vi "Test 401 Generic IO.vi"(11 "Test Case In":refnum<class "Test Profile Verification.lvclass">) -> (0 "error out":errorcluster, 3 "Test Case Out":refnum<class "Test Profile Verification.lvclass">)   [LabVIEW 2020, in "Test Profile Verification.lvclass"]
uses:
  Test Profile Verification.lvclass
  Test Profile Verification.lvclass/Test Profile Verification.ctl
  4993e8ee-a06a-463a-9684-69129f64d5ce.vi
  Profiles/401 Generic IO/CiA401 Generic IO Profile.lvclass
  Profiles/401 Generic IO/IO Capabilities.ctl
  EDS-File-Viewer/source/Electronic Datasheet/Electronic Datasheet.lvclass
  source/Typedefs/OD Entry Spec.ctl
  source/CANopen.lvlib
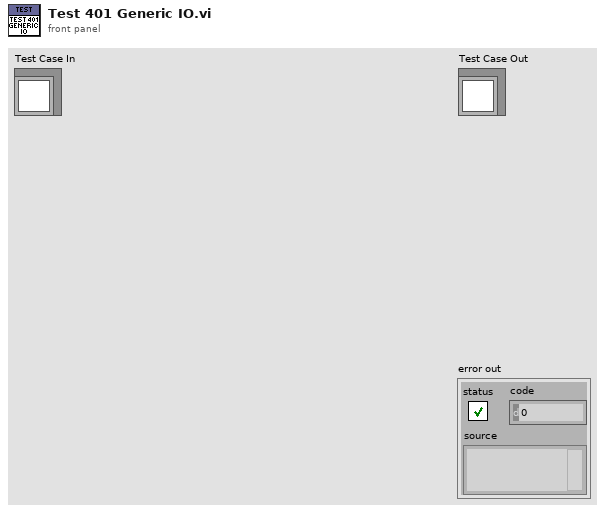
[diagram p1: front panel]
types:
  T1 = typedef "CANopen.lvlib/OD Entry Spec.ctl" = cluster{"Index":u16, "Name":string}
  T2 = typedef "CiA401 Generic IO Profile.lvclass/IO Capabilities.ctl" = cluster{"hasDigitialInputs":bool, "hasDigitalOutputs":bool, "hasAnalogInputs":bool, "hasAnalogOutputs":bool}
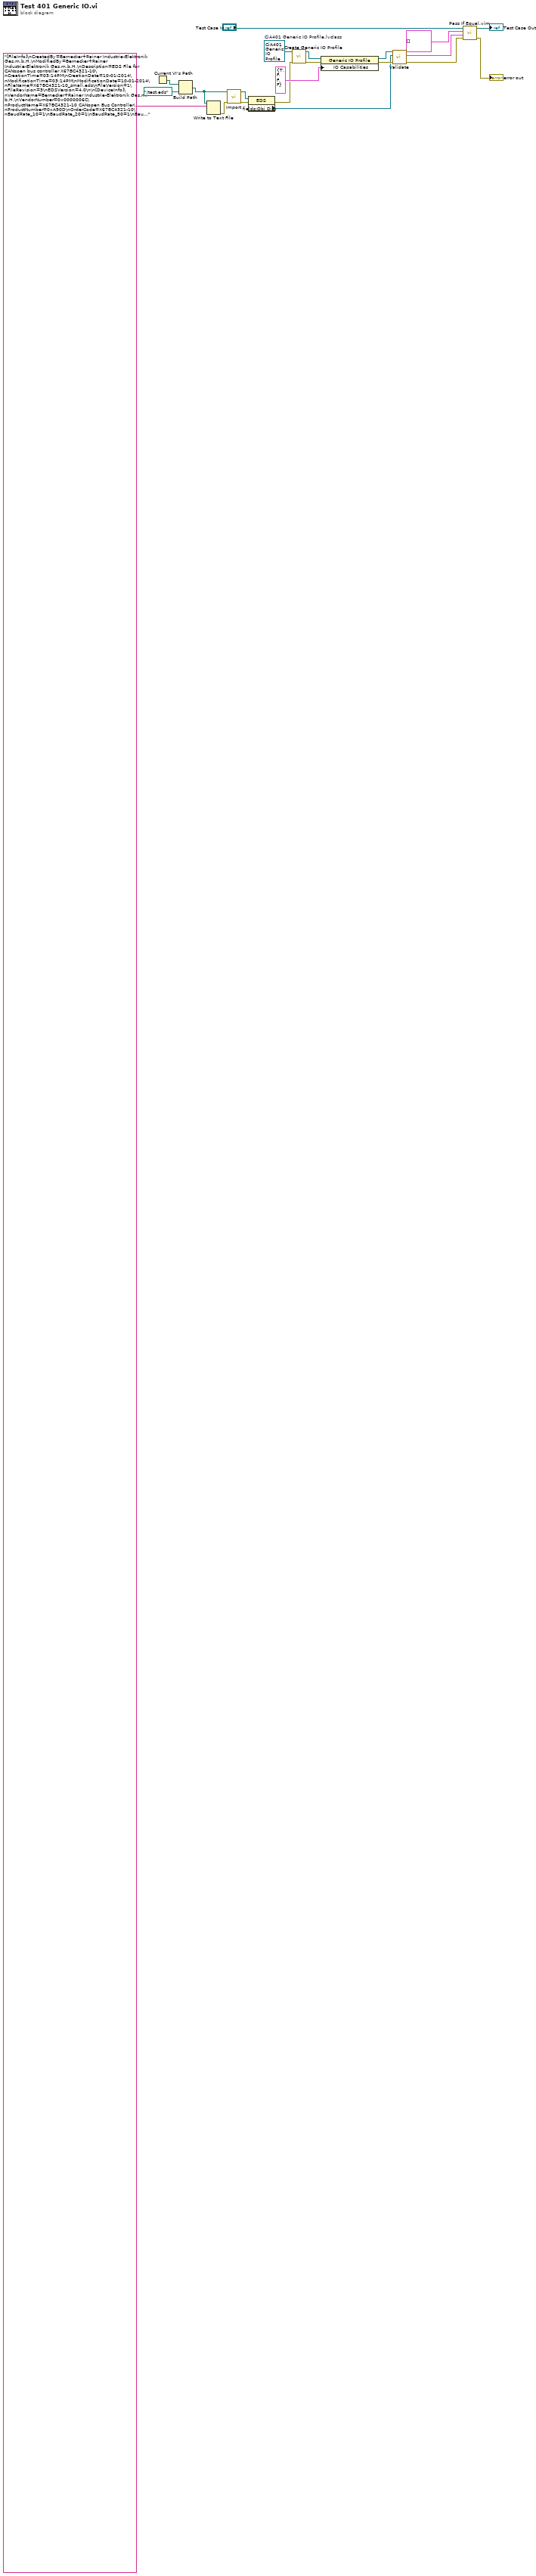
[diagram p0: block diagram]
diagram:
  w18 = refnum<class "CiA401 Generic IO Profile.lvclass"> refnum  # CiA401 Generic IO Profile.lvclass
  n1 = Current VI's Path() -> (path=w3:path)
  n2 = Build Path(base path=w3, name or relative path=path "../test.eds" ("file (use dialog)")) -> (appended path=w4:path)
  n3 = Write to Text File(file (use dialog)=w4, text="[FileInfo]\nCreatedBy=Bernecker+Rainer Industrie-Elektronik Ges.m.b.H.\nModifiedBy=Bernecker+Rainer Industrie-Elektronik Ges.m.b.H.\nDescription=EDS File for CANopen bus controller X67BC4321-10\nCreationTime=03:14PM\nCreationDate=10-01-2014\nModificationTime=03:14PM\nModificationDate=10-01-2014\nFileName=X67BC4321-10_small.eds\nFileVersion=1\nFileRevision=3\nEDSVersion=4.0\n\n[DeviceInfo]\nVendorName=Bernecker+Rainer Industrie-Elektronik Ges.m.b.H.\nVendorNumber=0x0000006C\nProductName=X67BC4321-10 CANopen Bus Controller\nProductNumber=0xA90D\nOrderCode=X67BC4321-10\nBaudRate_10=1\nBaudRate_20=1\nBaudRate_50=1\nBaudRate_125=1\nBaudRate_250=1\nBaudRate_500=1\nBaudRate_800=1\nBaudRate_1000=1\nSimpleBootUpMaster=0\nSimpleBootUpSlave=1\nGranularity=1\nDynamicChannelsSupported=0\nCompactPDO=0\nGroupMessaging=0\nNrOfRXPDO=32\nNrOfTXPDO=32\nLSS_Supported=0\n\n[DummyUsage]\nDummy0001=1\nDummy0002=1\nDummy0003=1\nDummy0004=1\nDummy0005=1\nDummy0006=1\nDummy0007=1\n\n[Comments]\nLines=0\n\n[MandatoryObjects]\nSupportedObjects=3\n1=0x1000\n2=0x1001\n3=0x1018\n\n[1000]\nParameterName=Device type\nObjectType=0x7\nDataType=0x0007\nAccessType=const\nDefaultValue=0x000F0191\nPDOMapping=0\nLowLimit=0x00000000\nHighLimit=0xFFFFFFFF\n\n[1001]\nParameterName=Error Register\nObjectType=0x7\nDataType=0x0005\nAccessType=ro\nDefaultValue=0x00\nPDOMapping=0\nLowLimit=0x00\nHighLimit=0xFF\n\n[1018]\nParameterName=Identity Object\nObjectType=0x9\nSubNumber=5\n\n[1018sub0]\nParameterName=Number of Entries\nObjectType=0x7\nDataType=0x0005\nAccessType=ro\nDefaultValue=0x4\nLowLimit=0x1\nHighLimit=0x4\n\n[1018sub1]\nParameterName=Vendor Id\nObjectType=0x7\nDataType=0x0007\nAccessType=ro\nDefaultValue=0x0000006C\nLowLimit=0x0\nHighLimit=0xFFFFFFFF\n\n[1018sub2]\nParameterName=Product Code\nObjectType=0x7\nDataType=0x0007\nAccessType=ro\nDefaultValue=0xA90D\nLowLimit=0x00000000\nHighLimit=0xFFFFFFFF\n\n[1018sub3]\nParameterName=Revision number\nObjectType=0x7\nDataType=0x0007\nAccessType=ro\nLowLimit=0x00000000\nHighLimit=0xFFFFFFFF\n\n[1018sub4]\nParameterName=Serial number\nObjectType=0x7\nDataType=0x0007\nAccessType=ro\nLowLimit=0x0\nHighLimit=0xFFFFFFFF\n\n[OptionalObjects]\nSupportedObjects=85\n1=0x1003\n2=0x1005\n3=0x1008\n4=0x1009\n5=0x100A\n6=0x100C\n7=0x100D\n8=0x1010\n9=0x1011\n10=0x1014\n11=0x1015\n12=0x1016\n13=0x1017\n14=0x1020\n15=0x1027\n16=0x1029\n17=0x1200\n18=0x1201\n19=0x1400\n20=0x1401\n21=0x1402\n22=0x1403\n23=0x1404\n24=0x1405\n25=0x1406\n26=0x1407\n27=0x1408\n28=0x1409\n29=0x1600\n30=0x1601\n31=0x1602\n32=0x1603\n33=0x1604\n34=0x1605\n35=0x1606\n36=0x1607\n37=0x1608\n38=0x1609\n39=0x1800\n40=0x1801\n41=0x1802\n42=0x1803\n43=0x1804\n44=0x1805\n45=0x1806\n46=0x1807\n47=0x1808\n48=0x1809\n49=0x1A00\n50=0x1A01\n51=0x1A02\n52=0x1A03\n53=0x1A04\n54=0x1A05\n55=0x1A06\n56=0x1A07\n57=0x1A08\n58=0x1A09\n59=0x1F50\n60=0x1F51\n61=0x1F52\n62=0x1F56\n63=0x1F57\n64=0x1F80\n65=0x6000\n66=0x6005\n67=0x6006\n68=0x6007\n69=0x6008\n70=0x6200\n71=0x6206\n72=0x6207\n73=0x6400\n74=0x6401\n75=0x6402\n76=0x6410\n77=0x6411\n78=0x6412\n79=0x6421\n80=0x6423\n81=0x6424\n82=0x6425\n83=0x6426\n84=0x6443\n85=0x6444\n\n[1003]\nParameterName=Pre-defined Error Field\nObjectType=0x8\nSubNumber=33\n\n[1003sub0]\nParameterName=Number of Errors\nObjectType=0x7\nDataType=0x0005\nAccessType=rw\nDefaultValue=0x0\nLowLimit=0x0\nHighLimit=0x20\n\n[1003sub1]\nParameterName=Standard Error Field 1\nObjectType=0x7\nDataType=0x0007\nAccessType=ro\nDefaultValue=0x0\nLowLimit=0x0\nHighLimit=0xFFFFFFFF\n\n[1003sub2]\nParameterName=Standard Error Field 2\nObjectType=0x7\nDataType=0x0007\nAccessType=ro\nDefaultValue=0x0\nLowLimit=0x0\nHighLimit=0xFFFFFFFF\n\n[1003sub3]\nParameterName=Standard Error Field 3\nObjectType=0x7\nDataType=0x0007\nAccessType=ro\nDefaultValue=0x0\nLowLimit=0x0\nHighLimit=0xFFFFFFFF\n\n[1003sub4]\nParameterName=Standard Error Field 4\nObjectType=0x7\nDataType=0x0007\nAccessType=ro\nDefaultValue=0x0\nLowLimit=0x0\nHighLimit=0xFFFFFFFF\n\n[1003sub5]\nParameterName=Standard Error Field 5\nObjectType=0x7\nDataType=0x0007\nAccessType=ro\nDefaultValue=0x0\nLowLimit=0x0\nHighLimit=0xFFFFFFFF\n\n[1003sub6]\nParameterName=Standard Error Field 6\nObjectType=0x7\nDataType=0x0007\nAccessType=ro\nDefaultValue=0x0\nLowLimit=0x0\nHighLimit=0xFFFFFFFF\n\n[1003sub7]\nParameterName=Standard Error Field 7\nObjectType=0x7\nDataType=0x0007\nAccessType=ro\nDefaultValue=0x0\nLowLimit=0x0\nHighLimit=0xFFFFFFFF\n\n[1003sub8]\nParameterName=Standard Error Field 8\nObjectType=0x7\nDataType=0x0007\nAccessType=ro\nDefaultValue=0x0\nLowLimit=0x0\nHighLimit=0xFFFFFFFF\n\n[1003sub9]\nParameterName=Standard Error Field 9\nObjectType=0x7\nDataType=0x0007\nAccessType=ro\nDefaultValue=0x0\nLowLimit=0x0\nHighLimit=0xFFFFFFFF\n\n[1003subA]\nParameterName=Standard Error Field 10\nObjectType=0x7\nDataType=0x0007\nAccessType=ro\nDefaultValue=0x0\nLowLimit=0x0\nHighLimit=0xFFFFFFFF\n\n[1003subB]\nParameterName=Standard Error Field 11\nObjectType=0x7\nDataType=0x0007\nAccessType=ro\nDefaultValue=0x0\nLowLimit=0x0\nHighLimit=0xFFFFFFFF\n\n[1003subC]\nParameterName=Standard Error Field 12\nObjectType=0x7\nDataType=0x0007\nAccessType=ro\nDefaultValue=0x0\nLowLimit=0x0\nHighLimit=0xFFFFFFFF\n\n[1003subD]\nParameterName=Standard Error Field 13\nObjectType=0x7\nDataType=0x0007\nAccessType=ro\nDefaultValue=0x0\nLowLimit=0x0\nHighLimit=0xFFFFFFFF\n\n[1003subE]\nParameterName=Standard Error Field 14\nObjectType=0x7\nDataType=0x0007\nAccessType=ro\nDefaultValue=0x0\nLowLimit=0x0\nHighLimit=0xFFFFFFFF\n\n[1003subF]\nParameterName=Standard Error Field 15\nObjectType=0x7\nDataType=0x0007\nAccessType=ro\nDefaultValue=0x0\nLowLimit=0x0\nHighLimit=0xFFFFFFFF\n\n[1003sub10]\nParameterName=Standard Error Field 16\nObjectType=0x7\nDataType=0x0007\nAccessType=ro\nDefaultValue=0x0\nLowLimit=0x0\nHighLimit=0xFFFFFFFF\n\n[1003sub11]\nParameterName=Standard Error Field 17\nObjectType=0x7\nDataType=0x0007\nAccessType=ro\nDefaultValue=0x0\nLowLimit=0x0\nHighLimit=0xFFFFFFFF\n\n[1003sub12]\nParameterName=Standard Error Field 18\nObjectType=0x7\nDataType=0x0007\nAccessType=ro\nDefaultValue=0x0\nLowLimit=0x0\nHighLimit=0xFFFFFFFF\n\n[1003sub13]\nParameterName=Standard Error Field 19\nObjectType=0x7\nDataType=0x0007\nAccessType=ro\nDefaultValue=0x0\nLowLimit=0x0\nHighLimit=0xFFFFFFFF\n\n[1003sub14]\nParameterName=Standard Error Field 20\nObjectType=0x7\nDataType=0x0007\nAccessType=ro\nDefaultValue=0x0\nLowLimit=0x0\nHighLimit=0xFFFFFFFF\n\n[1003sub15]\nParameterName=Standard Error Field 21\nObjectType=0x7\nDataType=0x0007\nAccessType=ro\nDefaultValue=0x0\nLowLimit=0x0\nHighLimit=0xFFFFFFFF\n\n[1003sub16]\nParameterName=Standard Error Field 22\nObjectType=0x7\nDataType=0x0007\nAccessType=ro\nDefaultValue=0x0\nLowLimit=0x0\nHighLimit=0xFFFFFFFF\n\n[1003sub17]\nParameterName=Standard Error Field 23\nObjectType=0x7\nDataType=0x0007\nAccessType=ro\nDefaultValue=0x0\nLowLimit=0x0\nHighLimit=0xFFFFFFFF\n\n[1003sub18]\nParameterName=Standard Error Field 24\nObjectType=0x7\nDataType=0x0007\nAccessType=ro\nDefaultValue=0x0\nLowLimit=0x0\nHighLimit=0xFFFFFFFF\n\n[1003sub19]\nParameterName=Standard Error Field 25\nObjectType=0x7\nDataType=0x0007\nAccessType=ro\nDefaultValue=0x0\nLowLimit=0x0\nHighLimit=0xFFFFFFFF\n\n[1003sub1A]\nParameterName=Standard Error Field 26\nObjectType=0x7\nDataType=0x0007\nAccessType=ro\nDefaultValue=0x0\nLowLimit=0x0\nHighLimit=0xFFFFFFFF\n\n[1003sub1B]\nParameterName=Standard Error Field 27\nObjectType=0x7\nDataType=0x0007\nAccessType=ro\nDefaultValue=0x0\nLowLimit=0x0\nHighLimit=0xFFFFFFFF\n\n[1003sub1C]\nParameterName=Standard Error Field 28\nObjectType=0x7\nDataType=0x0007\nAccessType=ro\nDefaultValue=0x0\nLowLimit=0x0\nHighLimit=0xFFFFFFFF\n\n[1003sub1D]\nParameterName=Standard Error Field 29\nObjectType=0x7\nDataType=0x0007\nAccessType=ro\nDefaultValue=0x0\nLowLimit=0x0\nHighLimit=0xFFFFFFFF\n\n[1003sub1E]\nParameterName=Standard Error Field 30\nObjectType=0x7\nDataType=0x0007\nAccessType=ro\nDefaultValue=0x0\nLowLimit=0x0\nHighLimit=0xFFFFFFFF\n\n[1003sub1F]\nParameterName=Standard Error Field 31\nObjectType=0x7\nDataType=0x0007\nAccessType=ro\nDefaultValue=0x0\nLowLimit=0x0\nHighLimit=0xFFFFFFFF\n\n[1003sub20]\nParameterName=Standard Error Field 32\nObjectType=0x7\nDataType=0x0007\nAccessType=ro\nDefaultValue=0x0\nLowLimit=0x0\nHighLimit=0xFFFFFFFF\n\n[1005]\nParameterName=COB-ID SYNC\nObjectType=0x7\nDataType=0x0007\nAccessType=rw\nDefaultValue=0x00000080\nPDOMapping=0\nLowLimit=0x00000001\nHighLimit=0xFFFFFFFF\n\n[1008]\nParameterName=Manufacturer Device Name\nObjectType=0x7\nDataType=0x0009\nAccessType=const\nDefaultValue=X67BC4321-10\nPDOMapping=0\n\n[1009]\nParameterName=Manufacturer Hardware Version\nObjectType=0x7\nDataType=0x0009\nAccessType=const\nPDOMapping=0\n\n[100A]\nParameterName=Manufacturer Software Version\nObjectType=0x7\nDataType=0x0009\nAccessType=const\nPDOMapping=0\n\n[100C]\nParameterName=Guard Time\nObjectType=0x7\nDataType=0x0006\nAccessType=rw\nDefaultValue=0\nPDOMapping=0\nLowLimit=0\nHighLimit=65535\n\n[100D]\nParameterName=Life Time Factor\nObjectType=0x7\nDataType=0x0005\nAccessType=rw\nDefaultValue=0x00\nPDOMapping=0\nLowLimit=0x0\nHighLimit=0xFF\n\n[1010]\nParameterName=Store Parameter Field\nObjectType=0x8\nSubNumber=5\n\n[1010sub0]\nParameterName=Number of Entries\nObjectType=0x7\nDataType=0x0005\nAccessType=ro\nDefaultValue=0x04\nLowLimit=0x0\nHighLimit=0x7F\n\n[1010sub1]\nParameterName=Save all Parameters\nObjectType=0x7\nDataType=0x0007\nAccessType=rw\n\n[1010sub2]\nParameterName=Save Communication Parameters\nObjectType=0x7\nDataType=0x0007\nAccessType=rw\n\n[1010sub3]\nParameterName=Save Application Parameters\nObjectType=0x7\nDataType=0x0007\nAccessType=rw\n\n[1010sub4]\nParameterName=Save Manufacturer Parameters\nObjectType=0x7\nDataType=0x0007\nAccessType=rw\n\n[1011]\nParameterName=Restore Default Parameters\nObjectType=0x8\nSubNumber=5\n\n[1011sub0]\nParameterName=Number of Entries\nObjectType=0x7\nDataType=0x0005\nAccessType=ro\nDefaultValue=0x04\nLowLimit=0x0\nHighLimit=0x7F\n\n[1011sub1]\nParameterName=Restore all Default Parameters\nObjectType=0x7\nDataType=0x0007\nAccessType=rw\n\n[1011sub2]\nParameterName=Restore Communication Default Parameters\nObjectType=0x7\nDataType=0x0007\nAccessType=rw\n\n[1011sub3]\nParameterName=Restore Application Default Parameters\nObjectType=0x7\nDataType=0x0007\nAccessType=rw\n\n[1011sub4]\nParameterName=Restore Manufacturer Default Parameters\nObjectType=0x7\nDataType=0x0007\nAccessType=rw\n\n[1014]\nParameterName=COB-ID EMCY\nObjectType=0x7\nDataType=0x0007\nAccessType=rw\nDefaultValue=$NODEID+0x080\nPDOMapping=0\nLowLimit=0x00000001\nHighLimit=0xFFFFFFFF\n\n[1015]\nParameterName=Inhibit Time Emergency\nObjectType=0x7\nDataType=0x0006\nAccessType=rw\nDefaultValue=0x0\nPDOMapping=0\nLowLimit=0x0\nHighLimit=0xFFFF\n\n[1016]\nParameterName=Consumer Heartbeat Time\nObjectType=0x8\nSubNumber=2\n\n[1016sub0]\nParameterName=Number of Entries\nObjectType=0x7\nDataType=0x0005\nAccessType=ro\nDefaultValue=0x1\nLowLimit=0x1\nHighLimit=0x7F\n\n[1016sub1]\nParameterName=Consumer Heartbeat Time\nObjectType=0x7\nDataType=0x0007\nAccessType=rw\nDefaultValue=0\nLowLimit=0x00000000\nHighLimit=0x007FFFFF\n\n[1017]\nParameterName=Producer Heartbeat Time\nObjectType=0x7\nDataType=0x0006\nAccessType=rw\nDefaultValue=0\nPDOMapping=0\nLowLimit=0\nHighLimit=65535\n\n[1020]\nParameterName=Verify Configuration\nObjectType=0x8\nSubNumber=3\n\n[1020sub0]\nParameterName=Number of entries\nObjectType=0x7\nDataType=0x0005\nAccessType=ro\nDefaultValue=2\n\n[1020sub1]\nParameterName=Configuration date\nObjectType=0x7\nDataType=0x0007\nAccessType=rw\n\n[1020sub2]\nParameterName=Configuration time\nObjectType=0x7\nDataType=0x0007\nAccessType=rw\n\n[1027]\nParameterName=Module List\nObjectType=0x8\nSubNumber=65\n\n[1027sub0]\nParameterName=Nr of connected modules\nObjectType=0x7\nDataType=0x0005\nAccessType=ro\nLowLimit=0x00\nHighLimit=0x40\n\n[1027sub1]\nParameterName=Module 1\nObjectType=0x7\nDataType=0x0006\nAccessType=ro\nDefaultValue=0xB528\nLowLimit=0x0000\nHighLimit=0xFFFF\n\n[1027sub2]\nParameterName=Module 2\nObjectType=0x7\nDataType=0x0006\nAccessType=ro\nDefaultValue=0x0000\nLowLimit=0x0000\nHighLimit=0xFFFF\n\n[1027sub3]\nParameterName=Module 3\nObjectType=0x7\nDataType=0x0006\nAccessType=ro\nDefaultValue=0x0000\nLowLimit=0x0000\nHighLimit=0xFFFF\n\n[1027sub4]\nParameterName=Module 4\nObjectType=0x7\nDataType=0x0006\nAccessType=ro\nDefaultValue=0x0000\nLowLimit=0x0000\nHighLimit=0xFFFF\n\n[1027sub5]\nParameterName=Module 5\nObjectType=0x7\nDataType=0x0006\nAccessType=ro\nDefaultValue=0x0000\nLowLimit=0x0000\nHighLimit=0xFFFF\n\n[1027sub6]\nParameterName=Module 6\nObjectType=0x7\nDataType=0x0006\nAccessType=ro\nDefaultValue=0x0000\nLowLimit=0x0000\nHighLimit=0xFFFF\n\n[1027sub7]\nParameterName=Module 7\nObjectType=0x7\nDataType=0x0006\nAccessType=ro\nDefaultValue=0x0000\nLowLimit=0x0000\nHighLimit=0xFFFF\n\n[1027sub8]\nParameterName=Module 8\nObjectType=0x7\nDataType=0x0006\nAccessType=ro\nDefaultValue=0x0000\nLowLimit=0x0000\nHighLimit=0xFFFF\n\n[1027sub9]\nParameterName=Module 9\nObjectType=0x7\nDataType=0x0006\nAccessType=ro\nDefaultValue=0x0000\nLowLimit=0x0000\nHighLimit=0xFFFF\n\n[1027subA]\nParameterName=Module 10\nObjectType=0x7\nDataType=0x0006\nAccessType=ro\nDefaultValue=0x0000\nLowLimit=0x0000\nHighLimit=0xFFFF\n\n[1027subB]\nParameterName=Module 11\nObjectType=0x7\nDataType=0x0006\nAccessType=ro\nDefaultValue=0x0000\nLowLimit=0x0000\nHighLimit=0xFFFF\n\n[1027subC]\nParameterName=Module 12\nObjectType=0x7\nDataType=0x0006\nAccessType=ro\nDefaultValue=0x0000\nLowLimit=0x0000\nHighLimit=0xFFFF\n\n[1027subD]\nParameterName=Module 13\nObjectType=0x7\nDataType=0x0006\nAccessType=ro\nDefaultValue=0x0000\nLowLimit=0x0000\nHighLimit=0xFFFF\n\n[1027subE]\nParameterName=Module 14\nObjectType=0x7\nDataType=0x0006\nAccessType=ro\nDefaultValue=0x0000\nLowLimit=0x0000\nHighLimit=0xFFFF\n\n[1027subF]\nParameterName=Module 15\nObjectType=0x7\nDataType=0x0006\nAccessType=ro\nDefaultValue=0x0000\nLowLimit=0x0000\nHighLimit=0xFFFF\n\n[1027sub10]\nParameterName=Module 16\nObjectType=0x7\nDataType=0x0006\nAccessType=ro\nDefaultValue=0x0000\nLowLimit=0x0000\nHighLimit=0xFFFF\n\n[1027sub11]\nParameterName=Module 17\nObjectType=0x7\nDataType=0x0006\nAccessType=ro\nDefaultValue=0x0000\nLowLimit=0x0000\nHighLimit=0xFFFF\n\n[1027sub12]\nParameterName=Module 18\nObjectType=0x7\nDataType=0x0006\nAccessType=ro\nDefaultValue=0x0000\nLowLimit=0x0000\nHighLimit=0xFFFF\n\n[1027sub13]\nParameterName=Module 19\nObjectType=0x7\nDataType=0x0006\nAccessType=ro\nDefaultValue=0x0000\nLowLimit=0x0000\nHighLimit=0xFFFF\n\n[1027sub14]\nParameterName=Module 20\nObjectType=0x7\nDataType=0x0006\nAccessType=ro\nDefaultValue=0x0000\nLowLimit=0x0000\nHighLimit=0xFFFF\n\n[1027sub15]\nParameterName=Module 21\nObjectType=0x7\nDataType=0x0006\nAccessType=ro\nDefaultValue=0x0000\nLowLimit=0x0000\nHighLimit=0xFFFF\n\n[1027sub16]\nParameterName=Module 22\nObjectType=0x7\nDataType=0x0006\nAccessType=ro\nDefaultValue=0x0000\nLowLimit=0x0000\nHighLimit=0xFFFF\n\n[1027sub17]\nParameterName=Module 23\nObjectType=0x7\nDataType=0x0006\nAccessType=ro\nDefaultValue=0x0000\nLowLimit=0x0000\nHighLimit=0xFFFF\n\n[1027sub18]\nParameterName=Module 24\nObjectType=0x7\nDataType=0x0006\nAccessType=ro\nDefaultValue=0x0000\nLowLimit=0x0000\nHighLimit=0xFFFF\n\n[1027sub19]\nParameterName=Module 25\nObjectType=0x7\nDataType=0x0006\nAccessType=ro\nDefaultValue=0x0000\nLowLimit=0x0000\nHighLimit=0xFFFF\n\n[1027sub1A]\nParameterName=Module 26\nObjectType=0x7\nDataType=0x0006\nAccessType=ro\nDefaultValue=0x0000\nLowLimit=0x0000\nHighLimit=0xFFFF\n\n[1027sub1B]\nParameterName=Module 27\nObjectType=0x7\nDataType=0x0006\nAccessType=ro\nDefaultValue=0x0000\nLowLimit=0x0000\nHighLimit=0xFFFF\n\n[1027sub1C]\nParameterName=Module 28\nObjectType=0x7\nDataType=0x0006\nAccessType=ro\nDefaultValue=0x0000\nLowLimit=0x0000\nHighLimit=0xFFFF\n\n[1027sub1D]\nParameterName=Module 29\nObjectType=0x7\nDataType=0x0006\nAccessType=ro\nDefaultValue=0x0000\nLowLimit=0x0000\nHighLimit=0xFFFF\n\n[1027sub1E]\nParameterName=Module 30\nObjectType=0x7\nDataType=0x0006\nAccessType=ro\nDefaultValue=0x0000\nLowLimit=0x0000\nHighLimit=0xFFFF\n\n[1027sub1F]\nParameterName=Module 31\nObjectType=0x7\nDataType=0x0006\nAccessType=ro\nDefaultValue=0x0000\nLowLimit=0x0000\nHighLimit=0xFFFF\n\n[1027sub20]\nParameterName=Module 32\nObjectType=0x7\nDataType=0x0006\nAccessType=ro\nDefaultValue=0x0000\nLowLimit=0x0000\nHighLimit=0xFFFF\n\n[1027sub21]\nParameterName=Module 33\nObjectType=0x7\nDataType=0x0006\nAccessType=ro\nDefaultValue=0x0000\nLowLimit=0x0000\nHighLimit=0xFFFF\n\n[1027sub22]\nParameterName=Module 34\nObjectType=0x7\nDataType=0x0006\nAccessType=ro\nDefaultValue=0x0000\nLowLimit=0x0000\nHighLimit=0xFFFF\n\n[1027sub23]\nParameterName=Module 35\nObjectType=0x7\nDataType=0x0006\nAccessType=ro\nDefaultValue=0x0000\nLowLimit=0x0000\nHighLimit=0xFFFF\n\n[1027sub24]\nParameterName=Module 36\nObjectType=0x7\nDataType=0x0006\nAccessType=ro\nDefaultValue=0x0000\nLowLimit=0x0000\nHighLimit=0xFFFF\n\n[1027sub25]\nParameterName=Module 37\nObjectType=0x7\nDataType=0x0006\nAccessType=ro\nDefaultValue=0x0000\nLowLimit=0x0000\nHighLimit=0xFFFF\n\n[1027sub26]\nParameterName=Module 38\nObjectType=0x7\nDataType=0x0006\nAccessType=ro\nDefaultValue=0x0000\nLowLimit=0x0000\nHighLimit=0xFFFF\n\n[1027sub27]\nParameterName=Module 39\nObjectType=0x7\nDataType=0x0006\nAccessType=ro\nDefaultValue=0x0000\nLowLimit=0x0000\nHighLimit=0xFFFF\n\n[1027sub28]\nParameterName=Module 40\nObjectType=0x7\nDataType=0x0006\nAccessType=ro\nDefaultValue=0x0000\nLowLimit=0x0000\nHighLimit=0xFFFF\n\n[1027sub29]\nParameterName=Module 41\nObjectType=0x7\nDataType=0x0006\nAccessType=ro\nDefaultValue=0x0000\nLowLimit=0x0000\nHighLimit=0xFFFF\n\n[1027sub2A]\nParameterName=Module 42\nObjectType=0x7\nDataType=0x0006\nAccessType=ro\nDefaultValue=0x0000\nLowLimit=0x0000\nHighLimit=0xFFFF\n\n[1027sub2B]\nParameterName=Module 43\nObjectType=0x7\nDataType=0x0006\nAccessType=ro\nDefaultValue=0x0000\nLowLimit=0x0000\nHighLimit=0xFFFF\n\n[1027sub2C]\nParameterName=Module 44\nObjectType=0x7\nDataType=0x0006\nAccessType=ro\nDefaultValue=0x0000\nLowLimit=0x0000\nHighLimit=0xFFFF\n\n[1027sub2D]\nParameterName=Module 45\nObjectType=0x7\nDataType=0x0006\nAccessType=ro\nDefaultValue=0x0000\nLowLimit=0x0000\nHighLimit=0xFFFF\n\n[1027sub2E]\nParameterName=Module 46\nObjectType=0x7\nDataType=0x0006\nAccessType=ro\nDefaultValue=0x0000\nLowLimit=0x0000\nHighLimit=0xFFFF\n\n[1027sub2F]\nParameterName=Module 47\nObjectType=0x7\nDataType=0x0006\nAccessType=ro\nDefaultValue=0x0000\nLowLimit=0x0000\nHighLimit=0xFFFF\n\n[1027sub30]\nParameterName=Module 48\nObjectType=0x7\nDataType=0x0006\nAccessType=ro\nDefaultValue=0x0000\nLowLimit=0x0000\nHighLimit=0xFFFF\n\n[1027sub31]\nParameterName=Module 49\nObjectType=0x7\nDataType=0x0006\nAccessType=ro\nDefaultValue=0x0000\nLowLimit=0x0000\nHighLimit=0xFFFF\n\n[1027sub32]\nParameterName=Module 50\nObjectType=0x7\nDataType=0x0006\nAccessType=ro\nDefaultValue=0x0000\nLowLimit=0x0000\nHighLimit=0xFFFF\n\n[1027sub33]\nParameterName=Module 51\nObjectType=0x7\nDataType=0x0006\nAccessType=ro\nDefaultValue=0x0000\nLowLimit=0x0000\nHighLimit=0xFFFF\n\n[1027sub34]\nParameterName=Module 52\nObjectType=0x7\nDataType=0x0006\nAccessType=ro\nDefaultValue=0x0000\nLowLimit=0x0000\nHighLimit=0xFFFF\n\n[1027sub35]\nParameterName=Module 53\nObjectType=0x7\nDataType=0x0006\nAccessType=ro\nDefaultValue=0x0000\nLowLimit=0x0000\nHighLimit=0xFFFF\n\n[1027sub36]\nParameterName=Module 54\nObjectType=0x7\nDataType=0x0006\nAccessType=ro\nDefaultValue=0x0000\nLowLimit=0x0000\nHighLimit=0xFFFF\n\n[1027sub37]\nParameterName=Module 55\nObjectType=0x7\nDataType=0x0006\nAccessType=ro\nDefaultValue=0x0000\nLowLimit=0x0000\nHighLimit=0xFFFF\n\n[1027sub38]\nParameterName=Module 56\nObjectType=0x7\nDataType=0x0006\nAccessType=ro\nDefaultValue=0x0000\nLowLimit=0x0000\nHighLimit=0xFFFF\n\n[1027sub39]\nParameterName=Module 57\nObjectType=0x7\nDataType=0x0006\nAccessType=ro\nDefaultValue=0x0000\nLowLimit=0x0000\nHighLimit=0xFFFF\n\n[1027sub3A]\nParameterName=Module 58\nObjectType=0x7\nDataType=0x0006\nAccessType=ro\nDefaultValue=0x0000\nLowLimit=0x0000\nHighLimit=0xFFFF\n\n[1027sub3B]\nParameterName=Module 59\nObjectType=0x7\nDataType=0x0006\nAccessType=ro\nDefaultValue=0x0000\nLowLimit=0x0000\nHighLimit=0xFFFF\n\n[1027sub3C]\nParameterName=Module 60\nObjectType=0x7\nDataType=0x0006\nAccessType=ro\nDefaultValue=0x0000\nLowLimit=0x0000\nHighLimit=0xFFFF\n\n[1027sub3D]\nParameterName=Module 61\nObjectType=0x7\nDataType=0x0006\nAccessType=ro\nDefaultValue=0x0000\nLowLimit=0x0000\nHighLimit=0xFFFF\n\n[1027sub3E]\nParameterName=Module 62\nObjectType=0x7\nDataType=0x0006\nAccessType=ro\nDefaultValue=0x0000\nLowLimit=0x0000\nHighLimit=0xFFFF\n\n[1027sub3F]\nParameterName=Module 63\nObjectType=0x7\nDataType=0x0006\nAccessType=ro\nDefaultValue=0x0000\nLowLimit=0x0000\nHighLimit=0xFFFF\n\n[1027sub40]\nParameterName=Module 64\nObjectType=0x7\nDataType=0x0006\nAccessType=ro\nDefaultValue=0x0000\nLowLimit=0x0000\nHighLimit=0xFFFF\n\n[1029]\nParameterName=Error behaviour\nObjectType=0x8\nSubNumber=3\n\n[1029sub0]\nParameterName=Nr of Error Classes\nObjectType=0x7\nDataType=0x0005\nAccessType=ro\nDefaultValue=128\n\n[1029sub1]\nParameterName=Communication Error\nObjectType=0x7\nDataType=0x0005\nAccessType=rw\nDefaultValue=0\n\n[1029sub80]\nParameterName=Advanced mapping\nObjectType=0x7\nDataType=0x0005\nAccessType=rw\nDefaultValue=0x81\n\n[1200]\nParameterName=Server SDO Parameter\nObjectType=0x9\nSubNumber=3\n\n[1200sub0]\nParameterName=Number of Entries\nObjectType=0x7\nDataType=0x0005\nAccessType=ro\nDefaultValue=0x02\nLowLimit=0x02\nHighLimit=0x02\n\n[1200sub1]\nParameterName=COB-ID Client -> Server\nObjectType=0x7\nDataType=0x0007\nAccessType=ro\nDefaultValue=$NODEID+0x600\nLowLimit=$NODEID+0x600\nHighLimit=$NODEID+0x600\n\n[1200sub2]\nParameterName=COB-ID Server -> Client\nObjectType=0x7\nDataType=0x0007\nAccessType=ro\nDefaultValue=$NODEID+0x580\nLowLimit=$NODEID+0x580\nHighLimit=$NODEID+0x580\n\n[1201]\nParameterName=Server SDO Parameter\nObjectType=0x9\nSubNumber=4\n\n[1201sub0]\nParameterName=Number of Entries\nObjectType=0x7\nDataType=0x0005\nAccessType=ro\nDefaultValue=0x3\nLowLimit=0x2\nHighLimit=0x3\n\n[1201sub1]\nParameterName=COB-ID Client -> Server\nObjectType=0x7\nDataType=0x0007\nAccessType=rw\nDefaultValue=0x80000000\nPDOMapping=0\nLowLimit=0x01\nHighLimit=0xFFFFFFFF\n\n[1201sub2]\nParameterName=COB-ID Server -> Client\nObjectType=0x7\nDataType=0x0007\nAccessType=rw\nDefaultValue=0x80000000\nPDOMapping=0\nLowLimit=0x01\nHighLimit=0xFFFFFFFF\n\n[1201sub3]\nParameterName=Node ID of the SDO Client\nObjectType=0x7\nDataType=0x0005\nAccessType=rw\nPDOMapping=0\nLowLimit=1\nHighLimit=127\n\n[1400]\nParameterName=Receive PDO 1 Communication Parameter\nObjectType=0x9\nSubNumber=5\n\n[1400sub0]\nParameterName=Number of Entries\nObjectType=0x7\nDataType=0x0005\nAccessType=ro\nDefaultValue=0x05\nLowLimit=0x02\nHighLimit=0x05\n\n[1400sub1]\nParameterName=COB-ID\nObjectType=0x7\nDataType=0x0007\nAccessType=rw\nDefaultValue=$NODEID+0x00000200\nLowLimit=0x00000001\nHighLimit=0xFFFFFFFF\n\n[1400sub2]\nParameterName=Transmission Type\nObjectType=0x7\nDataType=0x0005\nAccessType=rw\nDefaultValue=0xFF\nLowLimit=0x00\nHighLimit=0xFF\n\n[1400sub3]\nParameterName=Inhibit Time\nObjectType=0x7\nDataType=0x0006\nAccessType=rw\nDefaultValue=0x0000\nLowLimit=0x0000\nHighLimit=0xFFFF\n\n[1400sub5]\nParameterName=Event Timer\nObjectType=0x7\nDataType=0x0006\nAccessType=rw\nDefaultValue=0x0\nLowLimit=0x0\nHighLimit=0xFFFF\n\n[1401]\nParameterName=Receive PDO 2 Communication Parameter\nObjectType=0x9\nSubNumber=5\n\n[1401sub0]\nParameterName=Number of Entries\nObjectType=0x7\nDataType=0x0005\nAccessType=ro\nDefaultValue=0x05\nLowLimit=0x02\nHighLimit=0x05\n\n[1401sub1]\nParameterName=COB-ID\nObjectType=0x7\nDataType=0x0007\nAccessType=rw\nDefaultValue=$NODEID+0x00000300\nLowLimit=0x00000001\nHighLimit=0xFFFFFFFF\n\n[1401sub2]\nParameterName=Transmission Type\nObjectType=0x7\nDataType=0x0005\nAccessType=rw\nDefaultValue=0xFF\nLowLimit=0x00\nHighLimit=0xFF\n\n[1401sub3]\nParameterName=Inhibit Time\nObjectType=0x7\nDataType=0x0006\nAccessType=rw\nDefaultValue=0x0000\nLowLimit=0x0000\nHighLimit=0xFFFF\n\n[1401sub5]\nParameterName=Event Timer\nObjectType=0x7\nDataType=0x0006\nAccessType=rw\nDefaultValue=0x0\nLowLimit=0x0\nHighLimit=0xFFFF\n\n[1402]\nParameterName=Receive PDO 3 Communication Parameter\nObjectType=0x9\nSubNumber=5\n\n[1402sub0]\nParameterName=Number of Entries\nObjectType=0x7\nDataType=0x0005\nAccessType=ro\nDefaultValue=0x05\nLowLimit=0x02\nHighLimit=0x05\n\n[1402sub1]\nParameterName=COB-ID\nObjectType=0x7\nDataType=0x0007\nAccessType=rw\nDefaultValue=$NODEID+0x00000400\nLowLimit=0x00000001\nHighLimit=0xFFFFFFFF\n\n[1402sub2]\nParameterName=Transmission Type\nObjectType=0x7\nDataType=0x0005\nAccessType=rw\nDefaultValue=0xFF\nLowLimit=0x00\nHighLimit=0xFF\n\n[1402sub3]\nParameterName=Inhibit Time\nObjectType=0x7\nDataType=0x0006\nAccessType=rw\nDefaultValue=0x0000\nLowLimit=0x0000\nHighLimit=0xFFFF\n\n[1402sub5]\nParameterName=Event Timer\nObjectType=0x7\nDataType=0x0006\nAccessType=rw\nDefaultValue=0x0\nLowLimit=0x0\nHighLimit=0xFFFF\n\n[1403]\nParameterName=Receive PDO 4 Communication Parameter\nObjectType=0x9\nSubNumber=5\n\n[1403sub0]\nParameterName=Number of Entries\nObjectType=0x7\nDataType=0x0005\nAccessType=ro\nDefaultValue=0x05\nLowLimit=0x02\nHighLimit=0x05\n\n[1403sub1]\nParameterName=COB-ID\nObjectType=0x7\nDataType=0x0007\nAccessType=rw\nDefaultValue=$NODEID+0x00000500\nLowLimit=0x00000001\nHighLimit=0xFFFFFFFF\n\n[1403sub2]\nParameterName=Transmission Type\nObjectType=0x7\nDataType=0x0005\nAccessType=rw\nDefaultValue=0xFF\nLowLimit=0x00\nHighLimit=0xFF\n\n[1403sub3]\nParameterName=Inhibit Time\nObjectType=0x7\nDataType=0x0006\nAccessType=rw\nDefaultValue=0x0000\nLowLimit=0x0000\nHighLimit=0xFFFF\n\n[1403sub5]\nParameterName=Event Timer\nObjectType=0x7\nDataType=0x0006\nAccessType=rw\nDefaultValue=0x0\nLowLimit=0x0\nHighLimit=0xFFFF\n\n[1404]\nParameterName=Receive PDO 5 Communication Parameter\nObjectType=0x9\nSubNumber=5\n\n[1404sub0]\nParameterName=Number of Entries\nObjectType=0x7\nDataType=0x0005\nAccessType=ro\nDefaultValue=0x05\nLowLimit=0x02\nHighLimit=0x05\n\n[1404sub1]\nParameterName=COB-ID\nObjectType=0x7\nDataType=0x0007\nAccessType=rw\nDefaultValue=$NODEID+0x80000240\nLowLimit=0x00000001\nHighLimit=0xFFFFFFFF\n\n[1404sub2]\nParameterName=Transmission Type\nObjectType=0x7\nDataType=0x0005\nAccessType=rw\nDefaultValue=255\nLowLimit=0\nHighLimit=255\n\n[1404sub3]\nParameterName=Inhibit Time\nObjectType=0x7\nDataType=0x0006\nAccessType=rw\nDefaultValue=0x0000\nLowLimit=0x0000\nHighLimit=0xFFFF\n\n[1404sub5]\nParameterName=Event Timer\nObjectType=0x7\nDataType=0x0006\nAccessType=rw\nDefaultValue=0x0\nLowLimit=0x0\nHighLimit=0xFFFF\n\n[1405]\nParameterName=Receive PDO 6 Communication Parameter\nObjectType=0x9\nSubNumber=5\n\n[1405sub0]\nParameterName=Number of Entries\nObjectType=0x7\nDataType=0x0005\nAccessType=ro\nDefaultValue=0x05\nLowLimit=0x02\nHighLimit=0x05\n\n[1405sub1]\nParameterName=COB-ID\nObjectType=0x7\nDataType=0x0007\nAccessType=rw\nDefaultValue=$NODEID+0x80000340\nLowLimit=0x00000001\nHighLimit=0xFFFFFFFF\n\n[1405sub2]\nParameterName=Transmission Type\nObjectType=0x7\nDataType=0x0005\nAccessType=rw\nDefaultValue=255\nLowLimit=0\nHighLimit=255\n\n[1405sub3]\nParameterName=Inhibit Time\nObjectType=0x7\nDataType=0x0006\nAccessType=rw\nDefaultValue=0x0000\nLowLimit=0x0000\nHighLimit=0xFFFF\n\n[1405sub5]\nParameterName=Event Timer\nObjectType=0x7\nDataType=0x0006\nAccessType=rw\nDefaultValue=0x0\nLowLimit=0x0\nHighLimit=0xFFFF\n\n[1406]\nParameterName=Receive PDO 7 Communication Parameter\nObjectType=0x9\nSubNumber=5\n\n[1406sub0]\nParameterName=Number of Entries\nObjectType=0x7\nDataType=0x0005\nAccessType=ro\nDefaultValue=0x05\nLowLimit=0x02\nHighLimit=0x05\n\n[1406sub1]\nParameterName=COB-ID\nObjectType=0x7\nDataType=0x0007\nAccessType=rw\nDefaultValue=$NODEID+0x80000440\nLowLimit=0x00000001\nHighLimit=0xFFFFFFFF\n\n[1406sub2]\nParameterName=Transmission Type\nObjectType=0x7\nDataType=0x0005\nAccessType=rw\nDefaultValue=0xFF\nLowLimit=0x00\nHighLimit=0xFF\n\n[1406sub3]\nParameterName=Inhibit Time\nObjectType=0x7\nDataType=0x0006\nAccessType=rw\nDefaultValue=0x0000\nLowLimit=0x0000\nHighLimit=0xFFFF\n\n[1406sub5]\nParameterName=Event Timer\nObjectType=0x7\nDataType=0x0006\nAccessType=rw\nDefaultValue=0x0\nLowLimit=0x0\nHighLimit=0xFFFF\n\n[1407]\nParameterName=Receive PDO 8 Communication Parameter\nObjectType=0x9\nSubNumber=5\n\n[1407sub0]\nParameterName=Number of Entries\nObjectType=0x7\nDataType=0x0005\nAccessType=ro\nDefaultValue=0x05\nLowLimit=0x02\nHighLimit=0x05\n\n[1407sub1]\nParameterName=COB-ID\nObjectType=0x7\nDataType=0x0007\nAccessType=rw\nDefaultValue=$NODEID+0x80000540\nLowLimit=0x00000001\nHighLimit=0xFFFFFFFF\n\n[1407sub2]\nParameterName=Transmission Type\nObjectType=0x7\nDataType=0x0005\nAccessType=rw\nDefaultValue=0xFF\nLowLimit=0x00\nHighLimit=0xFF\n\n[1407sub3]\nParameterName=Inhibit Time\nObjectType=0x7\nDataType=0x0006\nAccessType=rw\nDefaultValue=0x0000\nLowLimit=0x0000\nHighLimit=0xFFFF\n\n[1407sub5]\nParameterName=Event Timer\nObjectType=0x7\nDataType=0x0006\nAccessType=rw\nDefaultValue=0x0\nLowLimit=0x0\nHighLimit=0xFFFF\n\n[1408]\nParameterName=Receive PDO 9 Communication Parameter\nObjectType=0x9\nSubNumber=5\n\n[1408sub0]\nParameterName=Number of Entries\nObjectType=0x7\nDataType=0x0005\nAccessType=ro\nDefaultValue=0x05\nLowLimit=0x02\nHighLimit=0x05\n\n[1408sub1]\nParameterName=COB-ID\nObjectType=0x7\nDataType=0x0007\nAccessType=rw\nDefaultValue=$NODEID+0x80000220\nLowLimit=0x00000001\nHighLimit=0xFFFFFFFF\n\n[1408sub2]\nParameterName=Transmission Type\nObjectType=0x7\nDataType=0x0005\nAccessType=rw\nDefaultValue=0xFF\nLowLimit=0x00\nHighLimit=0xFF\n\n[1408sub3]\nParameterName=Inhibit Time\nObjectType=0x7\nDataType=0x0006\nAccessType=rw\nDefaultValue=0x0000\nLowLimit=0x0000\nHighLimit=0xFFFF\n\n[1408sub5]\nParameterName=Event Timer\nObjectType=0x7\nDataType=0x0006\nAccessType=rw\nDefaultValue=0x0\nLowLimit=0x0\nHighLimit=0xFFFF\n\n[1409]\nParameterName=Receive PDO 10 Communication Parameter\nObjectType=0x9\nSubNumber=5\n\n[1409sub0]\nParameterName=Number of Entries\nObjectType=0x7\nDataType=0x0005\nAccessType=ro\nDefaultValue=0x05\nLowLimit=0x02\nHighLimit=0x05\n\n[1409sub1]\nParameterName=COB-ID\nObjectType=0x7\nDataType=0x0007\nAccessType=rw\nDefaultValue=$NODEID+0x80000320\nLowLimit=0x00000001\nHighLimit=0xFFFFFFFF\n\n[1409sub2]\nParameterName=Transmission Type\nObjectType=0x7\nDataType=0x0005\nAccessType=rw\nDefaultValue=0xFF\nLowLimit=0x00\nHighLimit=0xFF\n\n[1409sub3]\nParameterName=Inhibit Time\nObjectType=0x7\nDataType=0x0006\nAccessType=rw\nDefaultValue=0x0000\nLowLimit=0x0000\nHighLimit=0xFFFF\n\n[1409sub5]\nParameterName=Event Timer\nObjectType=0x7\nDataType=0x0006\nAccessType=rw\nDefaultValue=0x0\nLowLimit=0x0\nHighLimit=0xFFFF\n\n[1600]\nParameterName=Receive PDO 1 Mapping Parameter\nObjectType=0x9\nSubNumber=9\n\n[1600sub0]\nParameterName=Number of Entries\nObjectType=0x7\nDataType=0x0005\nAccessType=rw\nDefaultValue=8\nLowLimit=0\nHighLimit=64\n\n[1600sub1]\nParameterName=PDO Mapping Entry\nObjectType=0x7\nDataType=0x0007\nAccessType=rw\nDefaultValue=0x62000108\nLowLimit=0x00000000\nHighLimit=0xFFFFFFFF\n\n[1600sub2]\nParameterName=PDO Mapping Entry\nObjectType=0x7\nDataType=0x0007\nAccessType=rw\nDefaultValue=0x62000208\nLowLimit=0x00000000\nHighLimit=0xFFFFFFFF\n\n[1600sub3]\nParameterName=PDO Mapping Entry\nObjectType=0x7\nDataType=0x0007\nAccessType=rw\nDefaultValue=0x62000308\nLowLimit=0x00000000\nHighLimit=0xFFFFFFFF\n\n[1600sub4]\nParameterName=PDO Mapping Entry\nObjectType=0x7\nDataType=0x0007\nAccessType=rw\nDefaultValue=0x62000408\nLowLimit=0x00000000\nHighLimit=0xFFFFFFFF\n\n[1600sub5]\nParameterName=PDO Mapping Entry\nObjectType=0x7\nDataType=0x0007\nAccessType=rw\nDefaultValue=0x62000508\nLowLimit=0x00000000\nHighLimit=0xFFFFFFFF\n\n[1600sub6]\nParameterName=PDO Mapping Entry\nObjectType=0x7\nDataType=0x0007\nAccessType=rw\nDefaultValue=0x62000608\nLowLimit=0x00000000\nHighLimit=0xFFFFFFFF\n\n[1600sub7]\nParameterName=PDO Mapping Entry\nObjectType=0x7\nDataType=0x0007\nAccessType=rw\nDefaultValue=0x62000708\nLowLimit=0x00000000\nHighLimit=0xFFFFFFFF\n\n[1600sub8]\nParameterName=PDO Mapping Entry\nObjectType=0x7\nDataType=0x0007\nAccessType=rw\nDefaultValue=0x62000808\nLowLimit=0x00000000\nHighLimit=0xFFFFFFFF\n\n[1601]\nParameterName=Receive PDO 2 Mapping Parameter\nObjectType=0x9\nSubNumber=9\n\n[1601sub0]\nParameterName=Number of Entries\nObjectType=0x7\nDataType=0x0005\nAccessType=rw\nDefaultValue=4\nLowLimit=0\nHighLimit=64\n\n[1601sub1]\nParameterName=PDO Mapping Entry\nObjectType=0x7\nDataType=0x0007\nAccessType=rw\nDefaultValue=0x64110110\nLowLimit=0x00000000\nHighLimit=0xFFFFFFFF\n\n[1601sub2]\nParameterName=PDO Mapping Entry\nObjectType=0x7\nDataType=0x0007\nAccessType=rw\nDefaultValue=0x64110210\nLowLimit=0x00000000\nHighLimit=0xFFFFFFFF\n\n[1601sub3]\nParameterName=PDO Mapping Entry\nObjectType=0x7\nDataType=0x0007\nAccessType=rw\nDefaultValue=0x64110310\nLowLimit=0x00000000\nHighLimit=0xFFFFFFFF\n\n[1601sub4]\nParameterName=PDO Mapping Entry\nObjectType=0x7\nDataType=0x0007\nAccessType=rw\nDefaultValue=0x64110410\nLowLimit=0x00000000\nHighLimit=0xFFFFFFFF\n\n[1601sub5]\nParameterName=PDO Mapping Entry\nObjectType=0x7\nDataType=0x0007\nAccessType=rw\nDefaultValue=0x00000000\nLowLimit=0x00000000\nHighLimit=0xFFFFFFFF\n\n[1601sub6]\nParameterName=PDO Mapping Entry\nObjectType=0x7\nDataType=0x0007\nAccessType=rw\nDefaultValue=0x00000000\nLowLimit=0x00000000\nHighLimit=0xFFFFFFFF\n\n[1601sub7]\nParameterName=PDO Mapping Entry\nObjectType=0x7\nDataType=0x0007\nAccessType=rw\nDefaultValue=0x00000000\nLowLimit=0x00000000\nHighLimit=0xFFFFFFFF\n\n[1601sub8]\nParameterName=PDO Mapping Entry\nObjectType=0x7\nDataType=0x0007\nAccessType=rw\nDefaultValue=0x00000000\nLowLimit=0x00000000\nHighLimit=0xFFFFFFFF\n\n[1602]\nParameterName=Receive PDO 3 Mapping Parameter\nObjectType=0x9\nSubNumber=9\n\n[1602sub0]\nParameterName=Number of Entries\nObjectType=0x7\nDataType=0x0005\nAccessType=rw\nDefaultValue=4\nLowLimit=0\nHighLimit=64\n\n[1602sub1]\nParameterName=PDO Mapping Entry\nObjectType=0x7\nDataType=0x0007\nAccessType=rw\nDefaultValue=0x64110510\nLowLimit=0x00000000\nHighLimit=0xFFFFFFFF\n\n[1602sub2]\nParameterName=PDO Mapping Entry\nObjectType=0x7\nDataType=0x0007\nAccessType=rw\nDefaultValue=0x64110610\nLowLimit=0x00000000\nHighLimit=0xFFFFFFFF\n\n[1602sub3]\nParameterName=PDO Mapping Entry\nObjectType=0x7\nDataType=0x0007\nAccessType=rw\nDefaultValue=0x64110710\nLowLimit=0x00000000\nHighLimit=0xFFFFFFFF\n\n[1602sub4]\nParameterName=PDO Mapping Entry\nObjectType=0x7\nDataType=0x0007\nAccessType=rw\nDefaultValue=0x64110810\nLowLimit=0x00000000\nHighLimit=0xFFFFFFFF\n\n[1602sub5]\nParameterName=PDO Mapping Entry\nObjectType=0x7\nDataType=0x0007\nAccessType=rw\nDefaultValue=0x00000000\nLowLimit=0x00000000\nHighLimit=0xFFFFFFFF\n\n[1602sub6]\nParameterName=PDO Mapping Entry\nObjectType=0x7\nDataType=0x0007\nAccessType=rw\nDefaultValue=0x00000000\nLowLimit=0x00000000\nHighLimit=0xFFFFFFFF\n\n[1602sub7]\nParameterName=PDO Mapping Entry\nObjectType=0x7\nDataType=0x0007\nAccessType=rw\nDefaultValue=0x00000000\nLowLimit=0x00000000\nHighLimit=0xFFFFFFFF\n\n[1602sub8]\nParameterName=PDO Mapping Entry\nObjectType=0x7\nDataType=0x0007\nAccessType=rw\nDefaultValue=0x00000000\nLowLimit=0x00000000\nHighLimit=0xFFFFFFFF\n\n[1603]\nParameterName=Receive PDO 4 Mapping Parameter\nObjectType=0x9\nSubNumber=9\n\n[1603sub0]\nParameterName=Number of Entries\nObjectType=0x7\nDataType=0x0005\nAccessType=rw\nDefaultValue=4\nLowLimit=0\nHighLimit=64\n\n[1603sub1]\nParameterName=PDO Mapping Entry\nObjectType=0x7\nDataType=0x0007\nAccessType=rw\nDefaultValue=0x64110910\nLowLimit=0x00000000\nHighLimit=0xFFFFFFFF\n\n[1603sub2]\nParameterName=PDO Mapping Entry\nObjectType=0x7\nDataType=0x0007\nAccessType=rw\nDefaultValue=0x64110a10\nLowLimit=0x00000000\nHighLimit=0xFFFFFFFF\n\n[1603sub3]\nParameterName=PDO Mapping Entry\nObjectType=0x7\nDataType=0x0007\nAccessType=rw\nDefaultValue=0x64110b10\nLowLimit=0x00000000\nHighLimit=0xFFFFFFFF\n\n[1603sub4]\nParameterName=PDO Mapping Entry\nObjectType=0x7\nDataType=0x0007\nAccessType=rw\nDefaultValue=0x64110c10\nLowLimit=0x00000000\nHighLimit=0xFFFFFFFF\n\n[1603sub5]\nParameterName=PDO Mapping Entry\nObjectType=0x7\nDataType=0x0007\nAccessType=rw\nDefaultValue=0x00000000\nLowLimit=0x00000000\nHighLimit=0xFFFFFFFF\n\n[1603sub6]\nParameterName=PDO Mapping Entry\nObjectType=0x7\nDataType=0x0007\nAccessType=rw\nDefaultValue=0x00000000\nLowLimit=0x00000000\nHighLimit=0xFFFFFFFF\n\n[1603sub7]\nParameterName=PDO Mapping Entry\nObjectType=0x7\nDataType=0x0007\nAccessType=rw\nDefaultValue=0x00000000\nLowLimit=0x00000000\nHighLimit=0xFFFFFFFF\n\n[1603sub8]\nParameterName=PDO Mapping Entry\nObjectType=0x7\nDataType=0x0007\nAccessType=rw\nDefaultValue=0x00000000\nLowLimit=0x00000000\nHighLimit=0xFFFFFFFF\n\n[1604]\nParameterName=Receive PDO 5 Mapping Parameter\nObjectType=0x9\nSubNumber=9\n\n[1604sub0]\nParameterName=Number of Entries\nObjectType=0x7\nDataType=0x0005\nAccessType=rw\nDefaultValue=0\nLowLimit=0\nHighLimit=64\n\n[1604sub1]\nParameterName=PDO Mapping Entry\nObjectType=0x7\nDataType=0x0007\nAccessType=rw\nDefaultValue=0x00000000\nLowLimit=0x00000000\nHighLimit=0xFFFFFFFF\n\n[1604sub2]\nParameterName=PDO Mapping Entry\nObjectType=0x7\nDataType=0x0007\nAccessType=rw\nDefaultValue=0x00000000\nLowLimit=0x00000000\nHighLimit=0xFFFFFFFF\n\n[1604sub3]\nParameterName=PDO Mapping Entry\nObjectType=0x7\nDataType=0x0007\nAccessType=rw\nDefaultValue=0x00000000\nLowLimit=0x00000000\nHighLimit=0xFFFFFFFF\n\n[1604sub4]\nParameterName=PDO Mapping Entry\nObjectType=0x7\nDataType=0x0007\nAccessType=rw\nDefaultValue=0x00000000\nLowLimit=0x00000000\nHighLimit=0xFFFFFFFF\n\n[1604sub5]\nParameterName=PDO Mapping Entry\nObjectType=0x7\nDataType=0x0007\nAccessType=rw\nDefaultValue=0x00000000\nLowLimit=0x00000000\nHighLimit=0xFFFFFFFF\n\n[1604sub6]\nParameterName=PDO Mapping Entry\nObjectType=0x7\nDataType=0x0007\nAccessType=rw\nDefaultValue=0x00000000\nLowLimit=0x00000000\nHighLimit=0xFFFFFFFF\n\n[1604sub7]\nParameterName=PDO Mapping Entry\nObjectType=0x7\nDataType=0x0007\nAccessType=rw\nDefaultValue=0x00000000\nLowLimit=0x00000000\nHighLimit=0xFFFFFFFF\n\n[1604sub8]\nParameterName=PDO Mapping Entry\nObjectType=0x7\nDataType=0x0007\nAccessType=rw\nDefaultValue=0x00000000\nLowLimit=0x00000000\nHighLimit=0xFFFFFFFF\n\n[1605]\nParameterName=Receive PDO 6 Mapping Parameter\nObjectType=0x9\nSubNumber=9\n\n[1605sub0]\nParameterName=Number of Entries\nObjectType=0x7\nDataType=0x0005\nAccessType=rw\nDefaultValue=0\nLowLimit=0\nHighLimit=64\n\n[1605sub1]\nParameterName=PDO Mapping Entry\nObjectType=0x7\nDataType=0x0007\nAccessType=rw\nDefaultValue=0x00000000\nLowLimit=0x00000000\nHighLimit=0xFFFFFFFF\n\n[1605sub2]\nParameterName=PDO Mapping Entry\nObjectType=0x7\nDataType=0x0007\nAccessType=rw\nDefaultValue=0x00000000\nLowLimit=0x00000000\nHighLimit=0xFFFFFFFF\n\n[1605sub3]\nParameterName=PDO Mapping Entry\nObjectType=0x7\nDataType=0x0007\nAccessType=rw\nDefaultValue=0x00000000\nLowLimit=0x00000000\nHighLimit=0xFFFFFFFF\n\n[1605sub4]\nParameterName=PDO Mapping Entry\nObjectType=0x7\nDataType=0x0007\nAccessType=rw\nDefaultValue=0x00000000\nLowLimit=0x00000000\nHighLimit=0xFFFFFFFF\n\n[1605sub5]\nParameterName=PDO Mapping Entry\nObjectType=0x7\nDataType=0x0007\nAccessType=rw\nDefaultValue=0x00000000\nLowLimit=0x00000000\nHighLimit=0xFFFFFFFF\n\n[1605sub6]\nParameterName=PDO Mapping Entry\nObjectType=0x7\nDataType=0x0007\nAccessType=rw\nDefaultValue=0x00000000\nLowLimit=0x00000000\nHighLimit=0xFFFFFFFF\n\n[1605sub7]\nParameterName=PDO Mapping Entry\nObjectType=0x7\nDataType=0x0007\nAccessType=rw\nDefaultValue=0x00000000\nLowLimit=0x00000000\nHighLimit=0xFFFFFFFF\n\n[1605sub8]\nParameterName=PDO Mapping Entry\nObjectType=0x7\nDataType=0x0007\nAccessType=rw\nDefaultValue=0x00000000\nLowLimit=0x00000000\nHighLimit=0xFFFFFFFF\n\n[1606]\nParameterName=Receive PDO 7 Mapping Parameter\nObjectType=0x9\nSubNumber=9\n\n[1606sub0]\nParameterName=Number of Entries\nObjectType=0x7\nDataType=0x0005\nAccessType=rw\nDefaultValue=0\nLowLimit=0\nHighLimit=64\n\n[1606sub1]\nParameterName=PDO Mapping Entry\nObjectType=0x7\nDataType=0x0007\nAccessType=rw\nDefaultValue=0x00000000\nLowLimit=0x00000000\nHighLimit=0xFFFFFFFF\n\n[1606sub2]\nParameterName=PDO Mapping Entry\nObjectType=0x7\nDataType=0x0007\nAccessType=rw\nDefaultValue=0x00000000\nLowLimit=0x00000000\nHighLimit=0xFFFFFFFF\n\n[1606sub3]\nParameterName=PDO Mapping Entry\nObjectType=0x7\nDataType=0x0007\nAccessType=rw\nDefaultValue=0x00000000\nLowLimit=0x00000000\nHighLimit=0xFFFFFFFF\n\n[1606sub4]\nParameterName=PDO Mapping Entry\nObjectType=0x7\nDataType=0x0007\nAccessType=rw\nDefaultValue=0x00000000\nLowLimit=0x00000000\nHighLimit=0xFFFFFFFF\n\n[1606sub5]\nParameterName=PDO Mapping Entry\nObjectType=0x7\nDataType=0x0007\nAccessType=rw\nDefaultValue=0x00000000\nLowLimit=0x00000000\nHighLimit=0xFFFFFFFF\n\n[1606sub6]\nParameterName=PDO Mapping Entry\nObjectType=0x7\nDataType=0x0007\nAccessType=rw\nDefaultValue=0x00000000\nLowLimit=0x00000000\nHighLimit=0xFFFFFFFF\n\n[1606sub7]\nParameterName=PDO Mapping Entry\nObjectType=0x7\nDataType=0x0007\nAccessType=rw\nDefaultValue=0x00000000\nLowLimit=0x00000000\nHighLimit=0xFFFFFFFF\n\n[1606sub8]\nParameterName=PDO Mapping Entry\nObjectType=0x7\nDataType=0x0007\nAccessType=rw\nDefaultValue=0x00000000\nLowLimit=0x00000000\nHighLimit=0xFFFFFFFF\n\n[1607]\nParameterName=Receive PDO 8 Mapping Parameter\nObjectType=0x9\nSubNumber=9\n\n[1607sub0]\nParameterName=Number of Entries\nObjectType=0x7\nDataType=0x0005\nAccessType=rw\nDefaultValue=0\nLowLimit=0\nHighLimit=64\n\n[1607sub1]\nParameterName=PDO Mapping Entry\nObjectType=0x7\nDataType=0x0007\nAccessType=rw\nDefaultValue=0x00000000\nLowLimit=0x00000000\nHighLimit=0xFFFFFFFF\n\n[1607sub2]\nParameterName=PDO Mapping Entry\nObjectType=0x7\nDataType=0x0007\nAccessType=rw\nDefaultValue=0x00000000\nLowLimit=0x00000000\nHighLimit=0xFFFFFFFF\n\n[1607sub3]\nParameterName=PDO Mapping Entry\nObjectType=0x7\nDataType=0x0007\nAccessType=rw\nDefaultValue=0x00000000\nLowLimit=0x00000000\nHighLimit=0xFFFFFFFF\n\n[1607sub4]\nParameterName=PDO Mapping Entry\nObjectType=0x7\nDataType=0x0007\nAccessType=rw\nDefaultValue=0x00000000\nLowLimit=0x00000000\nHighLimit=0xFFFFFFFF\n\n[1607sub5]\nParameterName=PDO Mapping Entry\nObjectType=0x7\nDataType=0x0007\nAccessType=rw\nDefaultValue=0x00000000\nLowLimit=0x00000000\nHighLimit=0xFFFFFFFF\n\n[1607sub6]\nParameterName=PDO Mapping Entry\nObjectType=0x7\nDataType=0x0007\nAccessType=rw\nDefaultValue=0x00000000\nLowLimit=0x00000000\nHighLimit=0xFFFFFFFF\n\n[1607sub7]\nParameterName=PDO Mapping Entry\nObjectType=0x7\nDataType=0x0007\nAccessType=rw\nDefaultValue=0x00000000\nLowLimit=0x00000000\nHighLimit=0xFFFFFFFF\n\n[1607sub8]\nParameterName=PDO Mapping Entry\nObjectType=0x7\nDataType=0x0007\nAccessType=rw\nDefaultValue=0x00000000\nLowLimit=0x00000000\nHighLimit=0xFFFFFFFF\n\n[1608]\nParameterName=Receive PDO 9 Mapping Parameter\nObjectType=0x9\nSubNumber=9\n\n[1608sub0]\nParameterName=Number of Entries\nObjectType=0x7\nDataType=0x0005\nAccessType=rw\nDefaultValue=0\nLowLimit=0\nHighLimit=64\n\n[1608sub1]\nParameterName=PDO Mapping Entry\nObjectType=0x7\nDataType=0x0007\nAccessType=rw\nDefaultValue=0x00000000\nLowLimit=0x00000000\nHighLimit=0xFFFFFFFF\n\n[1608sub2]\nParameterName=PDO Mapping Entry\nObjectType=0x7\nDataType=0x0007\nAccessType=rw\nDefaultValue=0x00000000\nLowLimit=0x00000000\nHighLimit=0xFFFFFFFF\n\n[1608sub3]\nParameterName=PDO Mapping Entry\nObjectType=0x7\nDataType=0x0007\nAccessType=rw\nDefaultValue=0x00000000\nLowLimit=0x00000000\nHighLimit=0xFFFFFFFF\n\n[1608sub4]\nParameterName=PDO Mapping Entry\nObjectType=0x7\nDataType=0x0007\nAccessType=rw\nDefaultValue=0x00000000\nLowLimit=0x00000000\nHighLimit=0xFFFFFFFF\n\n[1608sub5]\nParameterName=PDO Mapping Entry\nObjectType=0x7\nDataType=0x0007\nAccessType=rw\nDefaultValue=0x00000000\nLowLimit=0x00000000\nHighLimit=0xFFFFFFFF\n\n[1608sub6]\nParameterName=PDO Mapping Entry\nObjectType=0x7\nDataType=0x0007\nAccessType=rw\nDefaultValue=0x00000000\nLowLimit=0x00000000\nHighLimit=0xFFFFFFFF\n\n[1608sub7]\nParameterName=PDO Mapping Entry\nObjectType=0x7\nDataType=0x0007\nAccessType=rw\nDefaultValue=0x00000000\nLowLimit=0x00000000\nHighLimit=0xFFFFFFFF\n\n[1608sub8]\nParameterName=PDO Mapping Entry\nObjectType=0x7\nDataType=0x0007\nAccessType=rw\nDefaultValue=0x00000000\nLowLimit=0x00000000\nHighLimit=0xFFFFFFFF\n\n[1609]\nParameterName=Receive PDO 10 Mapping Parameter\nObjectType=0x9\nSubNumber=9\n\n[1609sub0]\nParameterName=Number of Entries\nObjectType=0x7\nDataType=0x0005\nAccessType=rw\nDefaultValue=0\nLowLimit=0\nHighLimit=64\n\n[1609sub1]\nParameterName=PDO Mapping Entry\nObjectType=0x7\nDataType=0x0007\nAccessType=rw\nDefaultValue=0x00000000\nLowLimit=0x00000000\nHighLimit=0xFFFFFFFF\n\n[1609sub2]\nParameterName=PDO Mapping Entry\nObjectType=0x7\nDataType=0x0007\nAccessType=rw\nDefaultValue=0x00000000\nLowLimit=0x00000000\nHighLimit=0xFFFFFFFF\n\n[1609sub3]\nParameterName=PDO Mapping Entry\nObjectType=0x7\nDataType=0x0007\nAccessType=rw\nDefaultValue=0x00000000\nLowLimit=0x00000000\nHighLimit=0xFFFFFFFF\n\n[1609sub4]\nParameterName=PDO Mapping Entry\nObjectType=0x7\nDataType=0x0007\nAccessType=rw\nDefaultValue=0x00000000\nLowLimit=0x00000000\nHighLimit=0xFFFFFFFF\n\n[1609sub5]\nParameterName=PDO Mapping Entry\nObjectType=0x7\nDataType=0x0007\nAccessType=rw\nDefaultValue=0x00000000\nLowLimit=0x00000000\nHighLimit=0xFFFFFFFF\n\n[1609sub6]\nParameterName=PDO Mapping Entry\nObjectType=0x7\nDataType=0x0007\nAccessType=rw\nDefaultValue=0x00000000\nLowLimit=0x00000000\nHighLimit=0xFFFFFFFF\n\n[1609sub7]\nParameterName=PDO Mapping Entry\nObjectType=0x7\nDataType=0x0007\nAccessType=rw\nDefaultValue=0x00000000\nLowLimit=0x00000000\nHighLimit=0xFFFFFFFF\n\n[1609sub8]\nParameterName=PDO Mapping Entry\nObjectType=0x7\nDataType=0x0007\nAccessType=rw\nDefaultValue=0x00000000\nLowLimit=0x00000000\nHighLimit=0xFFFFFFFF\n\n[1800]\nParameterName=Transmit PDO 1 Communication Parameter\nObjectType=0x9\nSubNumber=5\n\n[1800sub0]\nParameterName=Number of Entries\nObjectType=0x7\nDataType=0x0005\nAccessType=ro\nDefaultValue=0x05\nLowLimit=0x02\nHighLimit=0x05\n\n[1800sub1]\nParameterName=COB-ID\nObjectType=0x7\nDataType=0x0007\nAccessType=rw\nDefaultValue=$NODEID+0x00000180\nLowLimit=0x00000001\nHighLimit=0xFFFFFFFF\n\n[1800sub2]\nParameterName=Transmission Type\nObjectType=0x7\nDataType=0x0005\nAccessType=rw\nDefaultValue=0xFF\nLowLimit=0x00\nHighLimit=0xFF\n\n[1800sub3]\nParameterName=Inhibit Time\nObjectType=0x7\nDataType=0x0006\nAccessType=rw\nDefaultValue=0x0000\nLowLimit=0x0000\nHighLimit=0xFFFF\n\n[1800sub5]\nParameterName=Event Timer\nObjectType=0x7\nDataType=0x0006\nAccessType=rw\nDefaultValue=0x0\nLowLimit=0x0\nHighLimit=0xFFFF\n\n[1801]\nParameterName=Transmit PDO 2 Communication Parameter\nObjectType=0x9\nSubNumber=5\n\n[1801sub0]\nParameterName=Number of Entries\nObjectType=0x7\nDataType=0x0005\nAccessType=ro\nDefaultValue=0x05\nLowLimit=0x02\nHighLimit=0x05\n\n[1801sub1]\nParameterName=COB-ID\nObjectType=0x7\nDataType=0x0007\nAccessType=rw\nDefaultValue=$NODEID+0x00000280\nLowLimit=0x00000001\nHighLimit=0xFFFFFFFF\n\n[1801sub2]\nParameterName=Transmission Type\nObjectType=0x7\nDataType=0x0005\nAccessType=rw\nDefaultValue=0xFF\nLowLimit=0x00\nHighLimit=0xFF\n\n[1801sub3]\nParameterName=Inhibit Time\nObjectType=0x7\nDataType=0x0006\nAccessType=rw\nDefaultValue=0x0000\nLowLimit=0x0000\nHighLimit=0xFFFF\n\n[1801sub5]\nParameterName=Event Timer\nObjectType=0x7\nDataType=0x0006\nAccessType=rw\nDefaultValue=0x0\nLowLimit=0x0000\nHighLimit=0xFFFF\n\n[1802]\nParameterName=Transmit PDO 3 Communication Parameter\nObjectType=0x9\nSubNumber=5\n\n[1802sub0]\nParameterName=Number of Entries\nObjectType=0x7\nDataType=0x0005\nAccessType=ro\nDefaultValue=0x05\nLowLimit=0x02\nHighLimit=0x05\n\n[1802sub1]\nParameterName=COB-ID\nObjectType=0x7\nDataType=0x0007\nAccessType=rw\nDefaultValue=$NODEID+0x00000380\nLowLimit=0x00000001\nHighLimit=0xFFFFFFFF\n\n[1802sub2]\nParameterName=Transmission Type\nObjectType=0x7\nDataType=0x0005\nAccessType=rw\nDefaultValue=0xFF\nLowLimit=0x00\nHighLimit=0xFF\n\n[1802sub3]\nParameterName=Inhibit Time\nObjectType=0x7\nDataType=0x0006\nAccessType=rw\nDefaultValue=0x0000\nLowLimit=0x0000\nHighLimit=0xFFFF\n\n[1802sub5]\nParameterName=Event Timer\nObjectType=0x7\nDataType=0x0006\nAccessType=rw\nDefaultValue=0x0\nLowLimit=0x0000\nHighLimit=0xFFFF\n\n[1803]\nParameterName=Transmit PDO 4 Communication Parameter\nObjectType=0x9\nSubNumber=5\n\n[1803sub0]\nParameterName=Number of Entries\nObjectType=0x7\nDataType=0x0005\nAccessType=ro\nDefaultValue=0x05\nLowLimit=0x02\nHighLimit=0x05\n\n[1803sub1]\nParameterName=COB-ID\nObjectType=0x7\nDataType=0x0007\nAccessType=rw\nDefaultValue=$NODEID+0x00000480\nLowLimit=0x00000001\nHighLimit=0xFFFFFFFF\n\n[1803sub2]\nParameterName=Transmission Type\nObjectType=0x7\nDataType=0x0005\nAccessType=rw\nDefaultValue=0xFF\nLowLimit=0x00\nHighLimit=0xFF\n\n[1803sub3]\nParameterName=Inhibit Time\nObjectType=0x7\nDataType=0x0006\nAccessType=rw\nDefaultValue=0x0000\nLowLimit=0x0000\nHighLimit=0xFFFF\n\n[1803sub5]\nParameterName=Event Timer\nObjectType=0x7\nDataType=0x0006\nAccessType=rw\nDefaultValue=0x0\nLowLimit=0x0000\nHighLimit=0xFFFF\n\n[1804]\nParameterName=Transmit PDO 5 Communication Parameter\nObjectType=0x9\nSubNumber=5\n\n[1804sub0]\nParameterName=Number of Entries\nObjectType=0x7\nDataType=0x0005\nAccessType=ro\nDefaultValue=0x05\nLowLimit=0x02\nHighLimit=0x05\n\n[1804sub1]\nParameterName=COB-ID\nObjectType=0x7\nDataType=0x0007\nAccessType=rw\nDefaultValue=$NODEID+0x800001c0\nLowLimit=0x00000001\nHighLimit=0xFFFFFFFF\n\n[1804sub2]\nParameterName=Transmission Type\nObjectType=0x7\nDataType=0x0005\nAccessType=rw\nDefaultValue=255\nLowLimit=0\nHighLimit=255\n\n[1804sub3]\nParameterName=Inhibit Time\nObjectType=0x7\nDataType=0x0006\nAccessType=rw\nDefaultValue=0x0000\nLowLimit=0x0000\nHighLimit=0xFFFF\n\n[1804sub5]\nParameterName=Event Timer\nObjectType=0x7\nDataType=0x0006\nAccessType=rw\nDefaultValue=0x0\nLowLimit=0x0000\nHighLimit=0xFFFF\n\n[1805]\nParameterName=Transmit PDO 6 Communication Parameter\nObjectType=0x9\nSubNumber=5\n\n[1805sub0]\nParameterName=Number of Entries\nObjectType=0x7\nDataType=0x0005\nAccessType=ro\nDefaultValue=0x05\nLowLimit=0x02\nHighLimit=0x05\n\n[1805sub1]\nParameterName=COB-ID\nObjectType=0x7\nDataType=0x0007\nAccessType=rw\nDefaultValue=$NODEID+0x800002C0\nLowLimit=0x00000001\nHighLimit=0xFFFFFFFF\n\n[1805sub2]\nParameterName=Transmission Type\nObjectType=0x7\nDataType=0x0005\nAccessType=rw\nDefaultValue=0xFF\nLowLimit=0x00\nHighLimit=0xFF\n\n[1805sub3]\nParameterName=Inhibit Time\nObjectType=0x7\nDataType=0x0006\nAccessType=rw\nDefaultValue=0x0000\nLowLimit=0x0000\nHighLimit=0xFFFF\n\n[1805sub5]\nParameterName=Event Timer\nObjectType=0x7\nDataType=0x0006\nAccessType=rw\nDefaultValue=0x0\nLowLimit=0x0000\nHighLimit=0xFFFF\n\n[1806]\nParameterName=Transmit PDO 7 Communication Parameter\nObjectType=0x9\nSubNumber=5\n\n[1806sub0]\nParameterName=Number of Entries\nObjectType=0x7\nDataType=0x0005\nAccessType=ro\nDefaultValue=0x05\nLowLimit=0x02\nHighLimit=0x05\n\n[1806sub1]\nParameterName=COB-ID\nObjectType=0x7\nDataType=0x0007\nAccessType=rw\nDefaultValue=$NODEID+0x800003C0\nLowLimit=0x00000001\nHighLimit=0xFFFFFFFF\n\n[1806sub2]\nParameterName=Transmission Type\nObjectType=0x7\nDataType=0x0005\nAccessType=rw\nDefaultValue=0xFF\nLowLimit=0x00\nHighLimit=0xFF\n\n[1806sub3]\nParameterName=Inhibit Time\nObjectType=0x7\nDataType=0x0006\nAccessType=rw\nDefaultValue=0x0000\nLowLimit=0x0000\nHighLimit=0xFFFF\n\n[1806sub5]\nParameterName=Event Timer\nObjectType=0x7\nDataType=0x0006\nAccessType=rw\nDefaultValue=0x0\nLowLimit=0x0000\nHighLimit=0xFFFF\n\n[1807]\nParameterName=Transmit PDO 8 Communication Parameter\nObjectType=0x9\nSubNumber=5\n\n[1807sub0]\nParameterName=Number of Entries\nObjectType=0x7\nDataType=0x0005\nAccessType=ro\nDefaultValue=0x05\nLowLimit=0x02\nHighLimit=0x05\n\n[1807sub1]\nParameterName=COB-ID\nObjectType=0x7\nDataType=0x0007\nAccessType=rw\nDefaultValue=$NODEID+0x800004C0\nLowLimit=0x00000001\nHighLimit=0xFFFFFFFF\n\n[1807sub2]\nParameterName=Transmission Type\nObjectType=0x7\nDataType=0x0005\nAccessType=rw\nDefaultValue=0xFF\nLowLimit=0x00\nHighLimit=0xFF\n\n[1807sub3]\nParameterName=Inhibit Time\nObjectType=0x7\nDataType=0x0006\nAccessType=rw\nDefaultValue=0x0000\nLowLimit=0x0000\nHighLimit=0xFFFF\n\n[1807sub5]\nParameterName=Event Timer\nObjectType=0x7\nDataType=0x0006\nAccessType=rw\nDefaultValue=0x0\nLowLimit=0x0000\nHighLimit=0xFFFF\n\n[1808]\nParameterName=Transmit PDO 9 Communication Parameter\nObjectType=0x9\nSubNumber=5\n\n[1808sub0]\nParameterName=Number of Entries\nObjectType=0x7\nDataType=0x0005\nAccessType=ro\nDefaultValue=0x05\nLowLimit=0x02\nHighLimit=0x05\n\n[1808sub1]\nParameterName=COB-ID\nObjectType=0x7\nDataType=0x0007\nAccessType=rw\nDefaultValue=$NODEID+0x800001A0\nLowLimit=0x00000001\nHighLimit=0xFFFFFFFF\n\n[1808sub2]\nParameterName=Transmission Type\nObjectType=0x7\nDataType=0x0005\nAccessType=rw\nDefaultValue=0xFF\nLowLimit=0x00\nHighLimit=0xFF\n\n[1808sub3]\nParameterName=Inhibit Time\nObjectType=0x7\nDataType=0x0006\nAccessType=rw\nDefaultValue=0x0000\nLowLimit=0x0000\nHighLimit=0xFFFF\n\n[1808sub5]\nParameterName=Event Timer\nObjectType=0x7\nDataType=0x0006\nAccessType=rw\nDefaultValue=0x0\nLowLimit=0x0000\nHighLimit=0xFFFF\n\n[1809]\nParameterName=Transmit PDO 10 Communication Parameter\nObjectType=0x9\nSubNumber=5\n\n[1809sub0]\nParameterName=Number of Entries\nObjectType=0x7\nDataType=0x0005\nAccessType=ro\nDefaultValue=0x05\nLowLimit=0x02\nHighLimit=0x05\n\n[1809sub1]\nParameterName=COB-ID\nObjectType=0x7\nDataType=0x0007\nAccessType=rw\nDefaultValue=$NODEID+0x800002A0\nLowLimit=0x00000001\nHighLimit=0xFFFFFFFF\n\n[1809sub2]\nParameterName=Transmission Type\nObjectType=0x7\nDataType=0x0005\nAccessType=rw\nDefaultValue=0xFF\nLowLimit=0x00\nHighLimit=0xFF\n\n[1809sub3]\nParameterName=Inhibit Time\nObjectType=0x7\nDataType=0x0006\nAccessType=rw\nDefaultValue=0x0000\nLowLimit=0x0000\nHighLimit=0xFFFF\n\n[1809sub5]\nParameterName=Event Timer\nObjectType=0x7\nDataType=0x0006\nAccessType=rw\nDefaultValue=0x0\nLowLimit=0x0000\nHighLimit=0xFFFF\n\n[1A00]\nParameterName=Transmit PDO 1 Mapping Parameter\nObjectType=0x9\nSubNumber=9\n\n[1A00sub0]\nParameterName=Number of Entries\nObjectType=0x7\nDataType=0x0005\nAccessType=rw\nDefaultValue=8\nLowLimit=0\nHighLimit=64\n\n[1A00sub1]\nParameterName=PDO Mapping Entry\nObjectType=0x7\nDataType=0x0007\nAccessType=rw\nDefaultValue=0x60000108\nLowLimit=0x00000000\nHighLimit=0xFFFFFFFF\n\n[1A00sub2]\nParameterName=PDO Mapping Entry\nObjectType=0x7\nDataType=0x0007\nAccessType=rw\nDefaultValue=0x60000208\nLowLimit=0x00000000\nHighLimit=0xFFFFFFFF\n\n[1A00sub3]\nParameterName=PDO Mapping Entry\nObjectType=0x7\nDataType=0x0007\nAccessType=rw\nDefaultValue=0x60000308\nLowLimit=0x00000000\nHighLimit=0xFFFFFFFF\n\n[1A00sub4]\nParameterName=PDO Mapping Entry\nObjectType=0x7\nDataType=0x0007\nAccessType=rw\nDefaultValue=0x60000408\nLowLimit=0x00000000\nHighLimit=0xFFFFFFFF\n\n[1A00sub5]\nParameterName=PDO Mapping Entry\nObjectType=0x7\nDataType=0x0007\nAccessType=rw\nDefaultValue=0x60000508\nLowLimit=0x00000000\nHighLimit=0xFFFFFFFF\n\n[1A00sub6]\nParameterName=PDO Mapping Entry\nObjectType=0x7\nDataType=0x0007\nAccessType=rw\nDefaultValue=0x60000608\nLowLimit=0x00000000\nHighLimit=0xFFFFFFFF\n\n[1A00sub7]\nParameterName=PDO Mapping Entry\nObjectType=0x7\nDataType=0x0007\nAccessType=rw\nDefaultValue=0x60000708\nLowLimit=0x00000000\nHighLimit=0xFFFFFFFF\n\n[1A00sub8]\nParameterName=PDO Mapping Entry\nObjectType=0x7\nDataType=0x0007\nAccessType=rw\nDefaultValue=0x60000808\nLowLimit=0x00000000\nHighLimit=0xFFFFFFFF\n\n[1A01]\nParameterName=Transmit PDO 2 Mapping Parameter\nObjectType=0x9\nSubNumber=9\n\n[1A01sub0]\nParameterName=Number of Entries\nObjectType=0x7\nDataType=0x0005\nAccessType=rw\nDefaultValue=4\nLowLimit=0\nHighLimit=64\n\n[1A01sub1]\nParameterName=PDO Mapping Entry\nObjectType=0x7\nDataType=0x0007\nAccessType=rw\nDefaultValue=0x64010110\nLowLimit=0x00000000\nHighLimit=0xFFFFFFFF\n\n[1A01sub2]\nParameterName=PDO Mapping Entry\nObjectType=0x7\nDataType=0x0007\nAccessType=rw\nDefaultValue=0x64010210\nLowLimit=0x00000000\nHighLimit=0xFFFFFFFF\n\n[1A01sub3]\nParameterName=PDO Mapping Entry\nObjectType=0x7\nDataType=0x0007\nAccessType=rw\nDefaultValue=0x64010310\nLowLimit=0x00000000\nHighLimit=0xFFFFFFFF\n\n[1A01sub4]\nParameterName=PDO Mapping Entry\nObjectType=0x7\nDataType=0x0007\nAccessType=rw\nDefaultValue=0x64010410\nLowLimit=0x00000000\nHighLimit=0xFFFFFFFF\n\n[1A01sub5]\nParameterName=PDO Mapping Entry\nObjectType=0x7\nDataType=0x0007\nAccessType=rw\nDefaultValue=0x00000000\nLowLimit=0x00000000\nHighLimit=0xFFFFFFFF\n\n[1A01sub6]\nParameterName=PDO Mapping Entry\nObjectType=0x7\nDataType=0x0007\nAccessType=rw\nDefaultValue=0x00000000\nLowLimit=0x00000000\nHighLimit=0xFFFFFFFF\n\n[1A01sub7]\nParameterName=PDO Mapping Entry\nObjectType=0x7\nDataType=0x0007\nAccessType=rw\nDefaultValue=0x00000000\nLowLimit=0x00000000\nHighLimit=0xFFFFFFFF\n\n[1A01sub8]\nParameterName=PDO Mapping Entry\nObjectType=0x7\nDataType=0x0007\nAccessType=rw\nDefaultValue=0x00000000\nLowLimit=0x00000000\nHighLimit=0xFFFFFFFF\n\n[1A02]\nParameterName=Transmit PDO 3 Mapping Parameter\nObjectType=0x9\nSubNumber=9\n\n[1A02sub0]\nParameterName=Number of Entries\nObjectType=0x7\nDataType=0x0005\nAccessType=rw\nDefaultValue=4\nLowLimit=0\nHighLimit=64\n\n[1A02sub1]\nParameterName=PDO Mapping Entry\nObjectType=0x7\nDataType=0x0007\nAccessType=rw\nDefaultValue=0x64010510\nLowLimit=0x00000000\nHighLimit=0xFFFFFFFF\n\n[1A02sub2]\nParameterName=PDO Mapping Entry\nObjectType=0x7\nDataType=0x0007\nAccessType=rw\nDefaultValue=0x64010610\nLowLimit=0x00000000\nHighLimit=0xFFFFFFFF\n\n[1A02sub3]\nParameterName=PDO Mapping Entry\nObjectType=0x7\nDataType=0x0007\nAccessType=rw\nDefaultValue=0x64010710\nLowLimit=0x00000000\nHighLimit=0xFFFFFFFF\n\n[1A02sub4]\nParameterName=PDO Mapping Entry\nObjectType=0x7\nDataType=0x0007\nAccessType=rw\nDefaultValue=0x64010810\nLowLimit=0x00000000\nHighLimit=0xFFFFFFFF\n\n[1A02sub5]\nParameterName=PDO Mapping Entry\nObjectType=0x7\nDataType=0x0007\nAccessType=rw\nDefaultValue=0x00000000\nLowLimit=0x00000000\nHighLimit=0xFFFFFFFF\n\n[1A02sub6]\nParameterName=PDO Mapping Entry\nObjectType=0x7\nDataType=0x0007\nAccessType=rw\nDefaultValue=0x00000000\nLowLimit=0x00000000\nHighLimit=0xFFFFFFFF\n\n[1A02sub7]\nParameterName=PDO Mapping Entry\nObjectType=0x7\nDataType=0x0007\nAccessType=rw\nDefaultValue=0x00000000\nLowLimit=0x00000000\nHighLimit=0xFFFFFFFF\n\n[1A02sub8]\nParameterName=PDO Mapping Entry\nObjectType=0x7\nDataType=0x0007\nAccessType=rw\nDefaultValue=0x00000000\nLowLimit=0x00000000\nHighLimit=0xFFFFFFFF\n\n[1A03]\nParameterName=Transmit PDO 4 Mapping Parameter\nObjectType=0x9\nSubNumber=9\n\n[1A03sub0]\nParameterName=Number of Entries\nObjectType=0x7\nDataType=0x0005\nAccessType=rw\nDefaultValue=4\nLowLimit=0\nHighLimit=64\n\n[1A03sub1]\nParameterName=PDO Mapping Entry\nObjectType=0x7\nDataType=0x0007\nAccessType=rw\nDefaultValue=0x64010910\nLowLimit=0x00000000\nHighLimit=0xFFFFFFFF\n\n[1A03sub2]\nParameterName=PDO Mapping Entry\nObjectType=0x7\nDataType=0x0007\nAccessType=rw\nDefaultValue=0x64010a10\nLowLimit=0x00000000\nHighLimit=0xFFFFFFFF\n\n[1A03sub3]\nParameterName=PDO Mapping Entry\nObjectType=0x7\nDataType=0x0007\nAccessType=rw\nDefaultValue=0x64010b10\nLowLimit=0x00000000\nHighLimit=0xFFFFFFFF\n\n[1A03sub4]\nParameterName=PDO Mapping Entry\nObjectType=0x7\nDataType=0x0007\nAccessType=rw\nDefaultValue=0x64010c10\nLowLimit=0x00000000\nHighLimit=0xFFFFFFFF\n\n[1A03sub5]\nParameterName=PDO Mapping Entry\nObjectType=0x7\nDataType=0x0007\nAccessType=rw\nDefaultValue=0x00000000\nLowLimit=0x00000000\nHighLimit=0xFFFFFFFF\n\n[1A03sub6]\nParameterName=PDO Mapping Entry\nObjectType=0x7\nDataType=0x0007\nAccessType=rw\nDefaultValue=0x00000000\nLowLimit=0x00000000\nHighLimit=0xFFFFFFFF\n\n[1A03sub7]\nParameterName=PDO Mapping Entry\nObjectType=0x7\nDataType=0x0007\nAccessType=rw\nDefaultValue=0x00000000\nLowLimit=0x00000000\nHighLimit=0xFFFFFFFF\n\n[1A03sub8]\nParameterName=PDO Mapping Entry\nObjectType=0x7\nDataType=0x0007\nAccessType=rw\nDefaultValue=0x00000000\nLowLimit=0x00000000\nHighLimit=0xFFFFFFFF\n\n[1A04]\nParameterName=Transmit PDO 5 Mapping Parameter\nObjectType=0x9\nSubNumber=9\n\n[1A04sub0]\nParameterName=Number of Entries\nObjectType=0x7\nDataType=0x0005\nAccessType=rw\nDefaultValue=0\nLowLimit=0\nHighLimit=64\n\n[1A04sub1]\nParameterName=PDO Mapping Entry\nObjectType=0x7\nDataType=0x0007\nAccessType=rw\nDefaultValue=0x00000000\nLowLimit=0x00000000\nHighLimit=0xFFFFFFFF\n\n[1A04sub2]\nParameterName=PDO Mapping Entry\nObjectType=0x7\nDataType=0x0007\nAccessType=rw\nDefaultValue=0x00000000\nLowLimit=0x00000000\nHighLimit=0xFFFFFFFF\n\n[1A04sub3]\nParameterName=PDO Mapping Entry\nObjectType=0x7\nDataType=0x0007\nAccessType=rw\nDefaultValue=0x00000000\nLowLimit=0x00000000\nHighLimit=0xFFFFFFFF\n\n[1A04sub4]\nParameterName=PDO Mapping Entry\nObjectType=0x7\nDataType=0x0007\nAccessType=rw\nDefaultValue=0x00000000\nLowLimit=0x00000000\nHighLimit=0xFFFFFFFF\n\n[1A04sub5]\nParameterName=PDO Mapping Entry\nObjectType=0x7\nDataType=0x0007\nAccessType=rw\nDefaultValue=0x00000000\nLowLimit=0x00000000\nHighLimit=0xFFFFFFFF\n\n[1A04sub6]\nParameterName=PDO Mapping Entry\nObjectType=0x7\nDataType=0x0007\nAccessType=rw\nDefaultValue=0x00000000\nLowLimit=0x00000000\nHighLimit=0xFFFFFFFF\n\n[1A04sub7]\nParameterName=PDO Mapping Entry\nObjectType=0x7\nDataType=0x0007\nAccessType=rw\nDefaultValue=0x00000000\nLowLimit=0x00000000\nHighLimit=0xFFFFFFFF\n\n[1A04sub8]\nParameterName=PDO Mapping Entry\nObjectType=0x7\nDataType=0x0007\nAccessType=rw\nDefaultValue=0x00000000\nLowLimit=0x00000000\nHighLimit=0xFFFFFFFF\n\n[1A05]\nParameterName=Transmit PDO 6 Mapping Parameter\nObjectType=0x9\nSubNumber=9\n\n[1A05sub0]\nParameterName=Number of Entries\nObjectType=0x7\nDataType=0x0005\nAccessType=rw\nDefaultValue=0\nLowLimit=0\nHighLimit=64\n\n[1A05sub1]\nParameterName=PDO Mapping Entry\nObjectType=0x7\nDataType=0x0007\nAccessType=rw\nDefaultValue=0x00000000\nLowLimit=0x00000000\nHighLimit=0xFFFFFFFF\n\n[1A05sub2]\nParameterName=PDO Mapping Entry\nObjectType=0x7\nDataType=0x0007\nAccessType=rw\nDefaultValue=0x00000000\nLowLimit=0x00000000\nHighLimit=0xFFFFFFFF\n\n[1A05sub3]\nParameterName=PDO Mapping Entry\nObjectType=0x7\nDataType=0x0007\nAccessType=rw\nDefaultValue=0x00000000\nLowLimit=0x00000000\nHighLimit=0xFFFFFFFF\n\n[1A05sub4]\nParameterName=PDO Mapping Entry\nObjectType=0x7\nDataType=0x0007\nAccessType=rw\nDefaultValue=0x00000000\nLowLimit=0x00000000\nHighLimit=0xFFFFFFFF\n\n[1A05sub5]\nParameterName=PDO Mapping Entry\nObjectType=0x7\nDataType=0x0007\nAccessType=rw\nDefaultValue=0x00000000\nLowLimit=0x00000000\nHighLimit=0xFFFFFFFF\n\n[1A05sub6]\nParameterName=PDO Mapping Entry\nObjectType=0x7\nDataType=0x0007\nAccessType=rw\nDefaultValue=0x00000000\nLowLimit=0x00000000\nHighLimit=0xFFFFFFFF\n\n[1A05sub7]\nParameterName=PDO Mapping Entry\nObjectType=0x7\nDataType=0x0007\nAccessType=rw\nDefaultValue=0x00000000\nLowLimit=0x00000000\nHighLimit=0xFFFFFFFF\n\n[1A05sub8]\nParameterName=PDO Mapping Entry\nObjectType=0x7\nDataType=0x0007\nAccessType=rw\nDefaultValue=0x00000000\nLowLimit=0x00000000\nHighLimit=0xFFFFFFFF\n\n[1A06]\nParameterName=Transmit PDO 7 Mapping Parameter\nObjectType=0x9\nSubNumber=9\n\n[1A06sub0]\nParameterName=Number of Entries\nObjectType=0x7\nDataType=0x0005\nAccessType=rw\nDefaultValue=0\nLowLimit=0\nHighLimit=64\n\n[1A06sub1]\nParameterName=PDO Mapping Entry\nObjectType=0x7\nDataType=0x0007\nAccessType=rw\nDefaultValue=0x00000000\nLowLimit=0x00000000\nHighLimit=0xFFFFFFFF\n\n[1A06sub2]\nParameterName=PDO Mapping Entry\nObjectType=0x7\nDataType=0x0007\nAccessType=rw\nDefaultValue=0x00000000\nLowLimit=0x00000000\nHighLimit=0xFFFFFFFF\n\n[1A06sub3]\nParameterName=PDO Mapping Entry\nObjectType=0x7\nDataType=0x0007\nAccessType=rw\nDefaultValue=0x00000000\nLowLimit=0x00000000\nHighLimit=0xFFFFFFFF\n\n[1A06sub4]\nParameterName=PDO Mapping Entry\nObjectType=0x7\nDataType=0x0007\nAccessType=rw\nDefaultValue=0x00000000\nLowLimit=0x00000000\nHighLimit=0xFFFFFFFF\n\n[1A06sub5]\nParameterName=PDO Mapping Entry\nObjectType=0x7\nDataType=0x0007\nAccessType=rw\nDefaultValue=0x00000000\nLowLimit=0x00000000\nHighLimit=0xFFFFFFFF\n\n[1A06sub6]\nParameterName=PDO Mapping Entry\nObjectType=0x7\nDataType=0x0007\nAccessType=rw\nDefaultValue=0x00000000\nLowLimit=0x00000000\nHighLimit=0xFFFFFFFF\n\n[1A06sub7]\nParameterName=PDO Mapping Entry\nObjectType=0x7\nDataType=0x0007\nAccessType=rw\nDefaultValue=0x00000000\nLowLimit=0x00000000\nHighLimit=0xFFFFFFFF\n\n[1A06sub8]\nParameterName=PDO Mapping Entry\nObjectType=0x7\nDataType=0x0007\nAccessType=rw\nDefaultValue=0x00000000\nLowLimit=0x00000000\nHighLimit=0xFFFFFFFF\n\n[1A07]\nParameterName=Transmit PDO 8 Mapping Parameter\nObjectType=0x9\nSubNumber=9\n\n[1A07sub0]\nParameterName=Number of Entries\nObjectType=0x7\nDataType=0x0005\nAccessType=rw\nDefaultValue=0\nLowLimit=0\nHighLimit=64\n\n[1A07sub1]\nParameterName=PDO Mapping Entry\nObjectType=0x7\nDataType=0x0007\nAccessType=rw\nDefaultValue=0x00000000\nLowLimit=0x00000000\nHighLimit=0xFFFFFFFF\n\n[1A07sub2]\nParameterName=PDO Mapping Entry\nObjectType=0x7\nDataType=0x0007\nAccessType=rw\nDefaultValue=0x00000000\nLowLimit=0x00000000\nHighLimit=0xFFFFFFFF\n\n[1A07sub3]\nParameterName=PDO Mapping Entry\nObjectType=0x7\nDataType=0x0007\nAccessType=rw\nDefaultValue=0x00000000\nLowLimit=0x00000000\nHighLimit=0xFFFFFFFF\n\n[1A07sub4]\nParameterName=PDO Mapping Entry\nObjectType=0x7\nDataType=0x0007\nAccessType=rw\nDefaultValue=0x00000000\nLowLimit=0x00000000\nHighLimit=0xFFFFFFFF\n\n[1A07sub5]\nParameterName=PDO Mapping Entry\nObjectType=0x7\nDataType=0x0007\nAccessType=rw\nDefaultValue=0x00000000\nLowLimit=0x00000000\nHighLimit=0xFFFFFFFF\n\n[1A07sub6]\nParameterName=PDO Mapping Entry\nObjectType=0x7\nDataType=0x0007\nAccessType=rw\nDefaultValue=0x00000000\nLowLimit=0x00000000\nHighLimit=0xFFFFFFFF\n\n[1A07sub7]\nParameterName=PDO Mapping Entry\nObjectType=0x7\nDataType=0x0007\nAccessType=rw\nDefaultValue=0x00000000\nLowLimit=0x00000000\nHighLimit=0xFFFFFFFF\n\n[1A07sub8]\nParameterName=PDO Mapping Entry\nObjectType=0x7\nDataType=0x0007\nAccessType=rw\nDefaultValue=0x00000000\nLowLimit=0x00000000\nHighLimit=0xFFFFFFFF\n\n[1A08]\nParameterName=Transmit PDO 9 Mapping Parameter\nObjectType=0x9\nSubNumber=9\n\n[1A08sub0]\nParameterName=Number of Entries\nObjectType=0x7\nDataType=0x0005\nAccessType=rw\nDefaultValue=0\nLowLimit=0\nHighLimit=64\n\n[1A08sub1]\nParameterName=PDO Mapping Entry\nObjectType=0x7\nDataType=0x0007\nAccessType=rw\nDefaultValue=0x00000000\nLowLimit=0x00000000\nHighLimit=0xFFFFFFFF\n\n[1A08sub2]\nParameterName=PDO Mapping Entry\nObjectType=0x7\nDataType=0x0007\nAccessType=rw\nDefaultValue=0x00000000\nLowLimit=0x00000000\nHighLimit=0xFFFFFFFF\n\n[1A08sub3]\nParameterName=PDO Mapping Entry\nObjectType=0x7\nDataType=0x0007\nAccessType=rw\nDefaultValue=0x00000000\nLowLimit=0x00000000\nHighLimit=0xFFFFFFFF\n\n[1A08sub4]\nParameterName=PDO Mapping Entry\nObjectType=0x7\nDataType=0x0007\nAccessType=rw\nDefaultValue=0x00000000\nLowLimit=0x00000000\nHighLimit=0xFFFFFFFF\n\n[1A08sub5]\nParameterName=PDO Mapping Entry\nObjectType=0x7\nDataType=0x0007\nAccessType=rw\nDefaultValue=0x00000000\nLowLimit=0x00000000\nHighLimit=0xFFFFFFFF\n\n[1A08sub6]\nParameterName=PDO Mapping Entry\nObjectType=0x7\nDataType=0x0007\nAccessType=rw\nDefaultValue=0x00000000\nLowLimit=0x00000000\nHighLimit=0xFFFFFFFF\n\n[1A08sub7]\nParameterName=PDO Mapping Entry\nObjectType=0x7\nDataType=0x0007\nAccessType=rw\nDefaultValue=0x00000000\nLowLimit=0x00000000\nHighLimit=0xFFFFFFFF\n\n[1A08sub8]\nParameterName=PDO Mapping Entry\nObjectType=0x7\nDataType=0x0007\nAccessType=rw\nDefaultValue=0x00000000\nLowLimit=0x00000000\nHighLimit=0xFFFFFFFF\n\n[1A09]\nParameterName=Transmit PDO 10 Mapping Parameter\nObjectType=0x9\nSubNumber=9\n\n[1A09sub0]\nParameterName=Number of Entries\nObjectType=0x7\nDataType=0x0005\nAccessType=rw\nDefaultValue=0\nLowLimit=0\nHighLimit=64\n\n[1A09sub1]\nParameterName=PDO Mapping Entry\nObjectType=0x7\nDataType=0x0007\nAccessType=rw\nDefaultValue=0x00000000\nLowLimit=0x00000000\nHighLimit=0xFFFFFFFF\n\n[1A09sub2]\nParameterName=PDO Mapping Entry\nObjectType=0x7\nDataType=0x0007\nAccessType=rw\nDefaultValue=0x00000000\nLowLimit=0x00000000\nHighLimit=0xFFFFFFFF\n\n[1A09sub3]\nParameterName=PDO Mapping Entry\nObjectType=0x7\nDataType=0x0007\nAccessType=rw\nDefaultValue=0x00000000\nLowLimit=0x00000000\nHighLimit=0xFFFFFFFF\n\n[1A09sub4]\nParameterName=PDO Mapping Entry\nObjectType=0x7\nDataType=0x0007\nAccessType=rw\nDefaultValue=0x00000000\nLowLimit=0x00000000\nHighLimit=0xFFFFFFFF\n\n[1A09sub5]\nParameterName=PDO Mapping Entry\nObjectType=0x7\nDataType=0x0007\nAccessType=rw\nDefaultValue=0x00000000\nLowLimit=0x00000000\nHighLimit=0xFFFFFFFF\n\n[1A09sub6]\nParameterName=PDO Mapping Entry\nObjectType=0x7\nDataType=0x0007\nAccessType=rw\nDefaultValue=0x00000000\nLowLimit=0x00000000\nHighLimit=0xFFFFFFFF\n\n[1A09sub7]\nParameterName=PDO Mapping Entry\nObjectType=0x7\nDataType=0x0007\nAccessType=rw\nDefaultValue=0x00000000\nLowLimit=0x00000000\nHighLimit=0xFFFFFFFF\n\n[1A09sub8]\nParameterName=PDO Mapping Entry\nObjectType=0x7\nDataType=0x0007\nAccessType=rw\nDefaultValue=0x00000000\nLowLimit=0x00000000\nHighLimit=0xFFFFFFFF\n\n[1F50]\nParameterName=Download Program Data\nObjectType=0x8\nSubNumber=3\n\n[1F50sub0]\nParameterName=Number of Entries\nObjectType=0x7\nDataType=0x0005\nAccessType=ro\nDefaultValue=0x02\nLowLimit=0x0\nHighLimit=0xFF\n\n[1F50sub1]\nParameterName=Firmware Area for BC\nObjectType=0x7\nDataType=0x000f\nAccessType=wo\n\n[1F50sub2]\nParameterName=Configuration\nObjectType=0x7\nDataType=0x000f\nAccessType=wo\n\n[1F51]\nParameterName=Program Control\nObjectType=0x8\nSubNumber=3\n\n[1F51sub0]\nParameterName=Number of Entries\nObjectType=0x7\nDataType=0x0005\nAccessType=ro\nDefaultValue=0x02\nLowLimit=0x0\nHighLimit=0xFF\n\n[1F51sub1]\nParameterName=Control BC Firmware\nObjectType=0x7\nDataType=0x0005\nAccessType=rw\n\n[1F51sub2]\nParameterName=Control Configuration\nObjectType=0x7\nDataType=0x0005\nAccessType=rw\n\n[1F52]\nParameterName=Verify Application Software\nObjectType=0x8\nSubNumber=3\n\n[1F52sub0]\nParameterName=Number of entries\nObjectType=0x7\nDataType=0x0005\nAccessType=ro\nDefaultValue=2\n\n[1F52sub1]\nParameterName=Application software date\nObjectType=0x7\nDataType=0x0007\nAccessType=ro\n\n[1F52sub2]\nParameterName=Application software time\nObjectType=0x7\nDataType=0x0007\nAccessType=ro\n\n[1F56]\nParameterName=Application software identification\nObjectType=0x8\nSubNumber=2\n\n[1F56sub0]\nParameterName=Number of Entries\nObjectType=0x7\nDataType=0x0005\nAccessType=ro\nDefaultValue=0x01\nLowLimit=0x0\nHighLimit=0xFF\n\n[1F56sub1]\nParameterName=BC Firmware\nObjectType=0x7\nDataType=0x0007\nAccessType=ro\n\n[1F57]\nParameterName=Flash Status Indication\nObjectType=0x8\nSubNumber=2\n\n[1F57sub0]\nParameterName=Number of entries\nObjectType=0x7\nDataType=0x0005\nAccessType=ro\nDefaultValue=1\n\n[1F57sub1]\nParameterName=Firmware Flash Status Indication\nObjectType=0x7\nDataType=0x0007\nAccessType=ro\n\n[1F80]\nParameterName=NMTStartup\nObjectType=0x7\nDataType=0x0007\nAccessType=rw\nPDOMapping=0\n\n[6000]\nParameterName=Read State 8 Input Lines\nObjectType=0x8\nSubNumber=21\n\n[6000sub0]\nParameterName=Number of Elements\nObjectType=0x7\nDataType=0x0005\nAccessType=ro\nDefaultValue=20\n\n[6000sub1]\nParameterName=DigInput8[1]\nObjectType=0x7\nDataType=0x0005\nAccessType=rwr\nDefaultValue=0x00\nPDOMapping=1\nLowLimit=0x00\nHighLimit=0xFF\n\n[6000sub2]\nParameterName=DigInput8[2]\nObjectType=0x7\nDataType=0x0005\nAccessType=rwr\nDefaultValue=0x00\nPDOMapping=1\nLowLimit=0x00\nHighLimit=0xFF\n\n[6000sub3]\nParameterName=DigInput8[3]\nObjectType=0x7\nDataType=0x0005\nAccessType=rwr\nDefaultValue=0x00\nPDOMapping=1\nLowLimit=0x00\nHighLimit=0xFF\n\n[6000sub4]\nParameterName=DigInput8[4]\nObjectType=0x7\nDataType=0x0005\nAccessType=rwr\nDefaultValue=0x00\nPDOMapping=1\nLowLimit=0x00\nHighLimit=0xFF\n\n[6000sub5]\nParameterName=DigInput8[5]\nObjectType=0x7\nDataType=0x0005\nAccessType=rwr\nDefaultValue=0x00\nPDOMapping=1\nLowLimit=0x00\nHighLimit=0xFF\n\n[6000sub6]\nParameterName=DigInput8[6]\nObjectType=0x7\nDataType=0x0005\nAccessType=rwr\nDefaultValue=0x00\nPDOMapping=1\nLowLimit=0x00\nHighLimit=0xFF\n\n[6000sub7]\nParameterName=DigInput8[7]\nObjectType=0x7\nDataType=0x0005\nAccessType=rwr\nDefaultValue=0x00\nPDOMapping=1\nLowLimit=0x00\nHighLimit=0xFF\n\n[6000sub8]\nParameterName=DigInput8[8]\nObjectType=0x7\nDataType=0x0005\nAccessType=rwr\nDefaultValue=0x00\nPDOMapping=1\nLowLimit=0x00\nHighLimit=0xFF\n\n[6000sub9]\nParameterName=DigInput8[9]\nObjectType=0x7\nDataType=0x0005\nAccessType=rwr\nDefaultValue=0x00\nPDOMapping=1\nLowLimit=0x00\nHighLimit=0xFF\n\n[6000subA]\nParameterName=DigInput8[10]\nObjectType=0x7\nDataType=0x0005\nAccessType=rwr\nDefaultValue=0x00\nPDOMapping=1\nLowLimit=0x00\nHighLimit=0xFF\n\n[6000subB]\nParameterName=DigInput8[11]\nObjectType=0x7\nDataType=0x0005\nAccessType=rwr\nDefaultValue=0x00\nPDOMapping=1\nLowLimit=0x00\nHighLimit=0xFF\n\n[6000subC]\nParameterName=DigInput8[12]\nObjectType=0x7\nDataType=0x0005\nAccessType=rwr\nDefaultValue=0x00\nPDOMapping=1\nLowLimit=0x00\nHighLimit=0xFF\n\n[6000subD]\nParameterName=DigInput8[13]\nObjectType=0x7\nDataType=0x0005\nAccessType=rwr\nDefaultValue=0x00\nPDOMapping=1\nLowLimit=0x00\nHighLimit=0xFF\n\n[6000subE]\nParameterName=DigInput8[14]\nObjectType=0x7\nDataType=0x0005\nAccessType=rwr\nDefaultValue=0x00\nPDOMapping=1\nLowLimit=0x00\nHighLimit=0xFF\n\n[6000subF]\nParameterName=DigInput8[15]\nObjectType=0x7\nDataType=0x0005\nAccessType=rwr\nDefaultValue=0x00\nPDOMapping=1\nLowLimit=0x00\nHighLimit=0xFF\n\n[6000sub10]\nParameterName=DigInput8[16]\nObjectType=0x7\nDataType=0x0005\nAccessType=rwr\nDefaultValue=0x00\nPDOMapping=1\nLowLimit=0x00\nHighLimit=0xFF\n\n[6000sub11]\nParameterName=DigInput8[17]\nObjectType=0x7\nDataType=0x0005\nAccessType=rwr\nDefaultValue=0x00\nPDOMapping=1\nLowLimit=0x00\nHighLimit=0xFF\n\n[6000sub12]\nParameterName=DigInput8[18]\nObjectType=0x7\nDataType=0x0005\nAccessType=rwr\nDefaultValue=0x00\nPDOMapping=1\nLowLimit=0x00\nHighLimit=0xFF\n\n[6000sub13]\nParameterName=DigInput8[19]\nObjectType=0x7\nDataType=0x0005\nAccessType=rwr\nDefaultValue=0x00\nPDOMapping=1\nLowLimit=0x00\nHighLimit=0xFF\n\n[6000sub14]\nParameterName=DigInput8[20]\nObjectType=0x7\nDataType=0x0005\nAccessType=rwr\nDefaultValue=0x00\nPDOMapping=1\nLowLimit=0x00\nHighLimit=0xFF\n\n[6005]\nParameterName=Global Interrupt Enable Digital 8-Bit\nObjectType=0x7\nDataType=0x0001\nAccessType=rw\nDefaultValue=1\nPDOMapping=0\n\n[6006]\nParameterName=Interrupt Mask Any Change 8-Bit\nObjectType=0x8\nSubNumber=21\n\n[6006sub0]\nParameterName=Number of Elements\nObjectType=0x7\nDataType=0x0005\nAccessType=ro\nDefaultValue=20\n\n[6006sub1]\nParameterName=InterruptAnyChange[1]\nObjectType=0x7\nDataType=0x0005\nAccessType=rw\nDefaultValue=255\n\n[6006sub2]\nParameterName=InterruptAnyChange[2]\nObjectType=0x7\nDataType=0x0005\nAccessType=rw\nDefaultValue=255\n\n[6006sub3]\nParameterName=InterruptAnyChange[3]\nObjectType=0x7\nDataType=0x0005\nAccessType=rw\nDefaultValue=255\n\n[6006sub4]\nParameterName=InterruptAnyChange[4]\nObjectType=0x7\nDataType=0x0005\nAccessType=rw\nDefaultValue=255\n\n[6006sub5]\nParameterName=InterruptAnyChange[5]\nObjectType=0x7\nDataType=0x0005\nAccessType=rw\nDefaultValue=255\n\n[6006sub6]\nParameterName=InterruptAnyChange[6]\nObjectType=0x7\nDataType=0x0005\nAccessType=rw\nDefaultValue=255\n\n[6006sub7]\nParameterName=InterruptAnyChange[7]\nObjectType=0x7\nDataType=0x0005\nAccessType=rw\nDefaultValue=255\n\n[6006sub8]\nParameterName=InterruptAnyChange[8]\nObjectType=0x7\nDataType=0x0005\nAccessType=rw\nDefaultValue=255\n\n[6006sub9]\nParameterName=InterruptAnyChange[9]\nObjectType=0x7\nDataType=0x0005\nAccessType=rw\nDefaultValue=255\n\n[6006subA]\nParameterName=InterruptAnyChange[10]\nObjectType=0x7\nDataType=0x0005\nAccessType=rw\nDefaultValue=255\n\n[6006subB]\nParameterName=InterruptAnyChange[11]\nObjectType=0x7\nDataType=0x0005\nAccessType=rw\nDefaultValue=255\n\n[6006subC]\nParameterName=InterruptAnyChange[12]\nObjectType=0x7\nDataType=0x0005\nAccessType=rw\nDefaultValue=255\n\n[6006subD]\nParameterName=InterruptAnyChange[13]\nObjectType=0x7\nDataType=0x0005\nAccessType=rw\nDefaultValue=255\n\n[6006subE]\nParameterName=InterruptAnyChange[14]\nObjectType=0x7\nDataType=0x0005\nAccessType=rw\nDefaultValue=255\n\n[6006subF]\nParameterName=InterruptAnyChange[15]\nObjectType=0x7\nDataType=0x0005\nAccessType=rw\nDefaultValue=255\n\n[6006sub10]\nParameterName=InterruptAnyChange[16]\nObjectType=0x7\nDataType=0x0005\nAccessType=rw\nDefaultValue=255\n\n[6006sub11]\nParameterName=InterruptAnyChange[17]\nObjectType=0x7\nDataType=0x0005\nAccessType=rw\nDefaultValue=255\n\n[6006sub12]\nParameterName=InterruptAnyChange[18]\nObjectType=0x7\nDataType=0x0005\nAccessType=rw\nDefaultValue=255\n\n[6006sub13]\nParameterName=InterruptAnyChange[19]\nObjectType=0x7\nDataType=0x0005\nAccessType=rw\nDefaultValue=255\n\n[6006sub14]\nParameterName=InterruptAnyChange[20]\nObjectType=0x7\nDataType=0x0005\nAccessType=rw\nDefaultValue=255\n\n[6007]\nParameterName=Interrupt Mask Low to High 8-Bit\nObjectType=0x8\nSubNumber=21\n\n[6007sub0]\nParameterName=Number of Elements\nObjectType=0x7\nDataType=0x0005\nAccessType=ro\nDefaultValue=20\n\n[6007sub1]\nParameterName=InterruptLowToHigh8[1]\nObjectType=0x7\nDataType=0x0005\nAccessType=rw\nDefaultValue=0\n\n[6007sub2]\nParameterName=InterruptLowToHigh8[2]\nObjectType=0x7\nDataType=0x0005\nAccessType=rw\nDefaultValue=0\n\n[6007sub3]\nParameterName=InterruptLowToHigh8[3]\nObjectType=0x7\nDataType=0x0005\nAccessType=rw\nDefaultValue=0\n\n[6007sub4]\nParameterName=InterruptLowToHigh8[4]\nObjectType=0x7\nDataType=0x0005\nAccessType=rw\nDefaultValue=0\n\n[6007sub5]\nParameterName=InterruptLowToHigh8[5]\nObjectType=0x7\nDataType=0x0005\nAccessType=rw\nDefaultValue=0\n\n[6007sub6]\nParameterName=InterruptLowToHigh8[6]\nObjectType=0x7\nDataType=0x0005\nAccessType=rw\nDefaultValue=0\n\n[6007sub7]\nParameterName=InterruptLowToHigh8[7]\nObjectType=0x7\nDataType=0x0005\nAccessType=rw\nDefaultValue=0\n\n[6007sub8]\nParameterName=InterruptLowToHigh8[8]\nObjectType=0x7\nDataType=0x0005\nAccessType=rw\nDefaultValue=0\n\n[6007sub9]\nParameterName=InterruptLowToHigh8[9]\nObjectType=0x7\nDataType=0x0005\nAccessType=rw\nDefaultValue=0\n\n[6007subA]\nParameterName=InterruptLowToHigh8[10]\nObjectType=0x7\nDataType=0x0005\nAccessType=rw\nDefaultValue=0\n\n[6007subB]\nParameterName=InterruptLowToHigh8[11]\nObjectType=0x7\nDataType=0x0005\nAccessType=rw\nDefaultValue=0\n\n[6007subC]\nParameterName=InterruptLowToHigh8[12]\nObjectType=0x7\nDataType=0x0005\nAccessType=rw\nDefaultValue=0\n\n[6007subD]\nParameterName=InterruptLowToHigh8[13]\nObjectType=0x7\nDataType=0x0005\nAccessType=rw\nDefaultValue=0\n\n[6007subE]\nParameterName=InterruptLowToHigh8[14]\nObjectType=0x7\nDataType=0x0005\nAccessType=rw\nDefaultValue=0\n\n[6007subF]\nParameterName=InterruptLowToHigh8[15]\nObjectType=0x7\nDataType=0x0005\nAccessType=rw\nDefaultValue=0\n\n[6007sub10]\nParameterName=InterruptLowToHigh8[16]\nObjectType=0x7\nDataType=0x0005\nAccessType=rw\nDefaultValue=0\n\n[6007sub11]\nParameterName=InterruptLowToHigh8[17]\nObjectType=0x7\nDataType=0x0005\nAccessType=rw\nDefaultValue=0\n\n[6007sub12]\nParameterName=InterruptLowToHigh8[18]\nObjectType=0x7\nDataType=0x0005\nAccessType=rw\nDefaultValue=0\n\n[6007sub13]\nParameterName=InterruptLowToHigh8[19]\nObjectType=0x7\nDataType=0x0005\nAccessType=rw\nDefaultValue=0\n\n[6007sub14]\nParameterName=InterruptLowToHigh8[20]\nObjectType=0x7\nDataType=0x0005\nAccessType=rw\nDefaultValue=0\n\n[6008]\nParameterName=Interrupt Mask High to Low 8-Bit\nObjectType=0x8\nSubNumber=21\n\n[6008sub0]\nParameterName=Number of Elements\nObjectType=0x7\nDataType=0x0005\nAccessType=ro\nDefaultValue=20\n\n[6008sub1]\nParameterName=InterruptHighToLow8[1]\nObjectType=0x7\nDataType=0x0005\nAccessType=rw\nDefaultValue=0\n\n[6008sub2]\nParameterName=InterruptHighToLow8[2]\nObjectType=0x7\nDataType=0x0005\nAccessType=rw\nDefaultValue=0\n\n[6008sub3]\nParameterName=InterruptHighToLow8[3]\nObjectType=0x7\nDataType=0x0005\nAccessType=rw\nDefaultValue=0\n\n[6008sub4]\nParameterName=InterruptHighToLow8[4]\nObjectType=0x7\nDataType=0x0005\nAccessType=rw\nDefaultValue=0\n\n[6008sub5]\nParameterName=InterruptHighToLow8[5]\nObjectType=0x7\nDataType=0x0005\nAccessType=rw\nDefaultValue=0\n\n[6008sub6]\nParameterName=InterruptHighToLow8[6]\nObjectType=0x7\nDataType=0x0005\nAccessType=rw\nDefaultValue=0\n\n[6008sub7]\nParameterName=InterruptHighToLow8[7]\nObjectType=0x7\nDataType=0x0005\nAccessType=rw\nDefaultValue=0\n\n[6008sub8]\nParameterName=InterruptHighToLow8[8]\nObjectType=0x7\nDataType=0x0005\nAccessType=rw\nDefaultValue=0\n\n[6008sub9]\nParameterName=InterruptHighToLow8[9]\nObjectType=0x7\nDataType=0x0005\nAccessType=rw\nDefaultValue=0\n\n[6008subA]\nParameterName=InterruptHighToLow8[10]\nObjectType=0x7\nDataType=0x0005\nAccessType=rw\nDefaultValue=0\n\n[6008subB]\nParameterName=InterruptHighToLow8[11]\nObjectType=0x7\nDataType=0x0005\nAccessType=rw\nDefaultValue=0\n\n[6008subC]\nParameterName=InterruptHighToLow8[12]\nObjectType=0x7\nDataType=0x0005\nAccessType=rw\nDefaultValue=0\n\n[6008subD]\nParameterName=InterruptHighToLow8[13]\nObjectType=0x7\nDataType=0x0005\nAccessType=rw\nDefaultValue=0\n\n[6008subE]\nParameterName=InterruptHighToLow8[14]\nObjectType=0x7\nDataType=0x0005\nAccessType=rw\nDefaultValue=0\n\n[6008subF]\nParameterName=InterruptHighToLow8[15]\nObjectType=0x7\nDataType=0x0005\nAccessType=rw\nDefaultValue=0\n\n[6008sub10]\nParameterName=InterruptHighToLow8[16]\nObjectType=0x7\nDataType=0x0005\nAccessType=rw\nDefaultValue=0\n\n[6008sub11]\nParameterName=InterruptHighToLow8[17]\nObjectType=0x7\nDataType=0x0005\nAccessType=rw\nDefaultValue=0\n\n[6008sub12]\nParameterName=InterruptHighToLow8[18]\nObjectType=0x7\nDataType=0x0005\nAccessType=rw\nDefaultValue=0\n\n[6008sub13]\nParameterName=InterruptHighToLow8[19]\nObjectType=0x7\nDataType=0x0005\nAccessType=rw\nDefaultValue=0\n\n[6008sub14]\nParameterName=InterruptHighToLow8[20]\nObjectType=0x7\nDataType=0x0005\nAccessType=rw\nDefaultValue=0\n\n[6200]\nParameterName=Write State 8 Output Lines\nObjectType=0x8\nSubNumber=21\n\n[6200sub0]\nParameterName=Number of Elements\nObjectType=0x7\nDataType=0x0005\nAccessType=ro\nDefaultValue=20\n\n[6200sub1]\nParameterName=DigOutU8[1]\nObjectType=0x7\nDataType=0x0005\nAccessType=rww\nDefaultValue=0x00\nPDOMapping=1\nLowLimit=0x00\nHighLimit=0xFF\n\n[6200sub2]\nParameterName=DigOutU8[2]\nObjectType=0x7\nDataType=0x0005\nAccessType=rww\nDefaultValue=0x00\nPDOMapping=1\nLowLimit=0x00\nHighLimit=0xFF\n\n[6200sub3]\nParameterName=DigOutU8[3]\nObjectType=0x7\nDataType=0x0005\nAccessType=rww\nDefaultValue=0x00\nPDOMapping=1\nLowLimit=0x00\nHighLimit=0xFF\n\n[6200sub4]\nParameterName=DigOutU8[4]\nObjectType=0x7\nDataType=0x0005\nAccessType=rww\nDefaultValue=0x00\nPDOMapping=1\nLowLimit=0x00\nHighLimit=0xFF\n\n[6200sub5]\nParameterName=DigOutU8[5]\nObjectType=0x7\nDataType=0x0005\nAccessType=rww\nDefaultValue=0x00\nPDOMapping=1\nLowLimit=0x00\nHighLimit=0xFF\n\n[6200sub6]\nParameterName=DigOutU8[6]\nObjectType=0x7\nDataType=0x0005\nAccessType=rww\nDefaultValue=0x00\nPDOMapping=1\nLowLimit=0x00\nHighLimit=0xFF\n\n[6200sub7]\nParameterName=DigOutU8[7]\nObjectType=0x7\nDataType=0x0005\nAccessType=rww\nDefaultValue=0x00\nPDOMapping=1\nLowLimit=0x00\nHighLimit=0xFF\n\n[6200sub8]\nParameterName=DigOutU8[8]\nObjectType=0x7\nDataType=0x0005\nAccessType=rww\nDefaultValue=0x00\nPDOMapping=1\nLowLimit=0x00\nHighLimit=0xFF\n\n[6200sub9]\nParameterName=DigOutU8[9]\nObjectType=0x7\nDataType=0x0005\nAccessType=rww\nDefaultValue=0x00\nPDOMapping=1\nLowLimit=0x00\nHighLimit=0xFF\n\n[6200subA]\nParameterName=DigOutU8[10]\nObjectType=0x7\nDataType=0x0005\nAccessType=rww\nDefaultValue=0x00\nPDOMapping=1\nLowLimit=0x00\nHighLimit=0xFF\n\n[6200subB]\nParameterName=DigOutU8[11]\nObjectType=0x7\nDataType=0x0005\nAccessType=rww\nDefaultValue=0x00\nPDOMapping=1\nLowLimit=0x00\nHighLimit=0xFF\n\n[6200subC]\nParameterName=DigOutU8[12]\nObjectType=0x7\nDataType=0x0005\nAccessType=rww\nDefaultValue=0x00\nPDOMapping=1\nLowLimit=0x00\nHighLimit=0xFF\n\n[6200subD]\nParameterName=DigOutU8[13]\nObjectType=0x7\nDataType=0x0005\nAccessType=rww\nDefaultValue=0x00\nPDOMapping=1\nLowLimit=0x00\nHighLimit=0xFF\n\n[6200subE]\nParameterName=DigOutU8[14]\nObjectType=0x7\nDataType=0x0005\nAccessType=rww\nDefaultValue=0x00\nPDOMapping=1\nLowLimit=0x00\nHighLimit=0xFF\n\n[6200subF]\nParameterName=DigOutU8[15]\nObjectType=0x7\nDataType=0x0005\nAccessType=rww\nDefaultValue=0x00\nPDOMapping=1\nLowLimit=0x00\nHighLimit=0xFF\n\n[6200sub10]\nParameterName=DigOutU8[16]\nObjectType=0x7\nDataType=0x0005\nAccessType=rww\nDefaultValue=0x00\nPDOMapping=1\nLowLimit=0x00\nHighLimit=0xFF\n\n[6200sub11]\nParameterName=DigOutU8[17]\nObjectType=0x7\nDataType=0x0005\nAccessType=rww\nDefaultValue=0x00\nPDOMapping=1\nLowLimit=0x00\nHighLimit=0xFF\n\n[6200sub12]\nParameterName=DigOutU8[18]\nObjectType=0x7\nDataType=0x0005\nAccessType=rww\nDefaultValue=0x00\nPDOMapping=1\nLowLimit=0x00\nHighLimit=0xFF\n\n[6200sub13]\nParameterName=DigOutU8[19]\nObjectType=0x7\nDataType=0x0005\nAccessType=rww\nDefaultValue=0x00\nPDOMapping=1\nLowLimit=0x00\nHighLimit=0xFF\n\n[6200sub14]\nParameterName=DigOutU8[20]\nObjectType=0x7\nDataType=0x0005\nAccessType=rww\nDefaultValue=0x00\nPDOMapping=1\nLowLimit=0x00\nHighLimit=0xFF\n\n[6206]\nParameterName=Error Mode Output 8-Bit\nObjectType=0x8\nSubNumber=21\n\n[6206sub0]\nParameterName=Number of Elements\nObjectType=0x7\nDataType=0x0005\nAccessType=ro\nDefaultValue=20\n\n[6206sub1]\nParameterName=ErrorMode8[1]\nObjectType=0x7\nDataType=0x0005\nAccessType=rw\nDefaultValue=255\n\n[6206sub2]\nParameterName=ErrorMode8[2]\nObjectType=0x7\nDataType=0x0005\nAccessType=rw\nDefaultValue=255\n\n[6206sub3]\nParameterName=ErrorMode8[3]\nObjectType=0x7\nDataType=0x0005\nAccessType=rw\nDefaultValue=255\n\n[6206sub4]\nParameterName=ErrorMode8[4]\nObjectType=0x7\nDataType=0x0005\nAccessType=rw\nDefaultValue=255\n\n[6206sub5]\nParameterName=ErrorMode8[5]\nObjectType=0x7\nDataType=0x0005\nAccessType=rw\nDefaultValue=255\n\n[6206sub6]\nParameterName=ErrorMode8[6]\nObjectType=0x7\nDataType=0x0005\nAccessType=rw\nDefaultValue=255\n\n[6206sub7]\nParameterName=ErrorMode8[7]\nObjectType=0x7\nDataType=0x0005\nAccessType=rw\nDefaultValue=255\n\n[6206sub8]\nParameterName=ErrorMode8[8]\nObjectType=0x7\nDataType=0x0005\nAccessType=rw\nDefaultValue=255\n\n[6206sub9]\nParameterName=ErrorMode8[9]\nObjectType=0x7\nDataType=0x0005\nAccessType=rw\nDefaultValue=255\n\n[6206subA]\nParameterName=ErrorMode8[10]\nObjectType=0x7\nDataType=0x0005\nAccessType=rw\nDefaultValue=255\n\n[6206subB]\nParameterName=ErrorMode8[11]\nObjectType=0x7\nDataType=0x0005\nAccessType=rw\nDefaultValue=255\n\n[6206subC]\nParameterName=ErrorMode8[12]\nObjectType=0x7\nDataType=0x0005\nAccessType=rw\nDefaultValue=255\n\n[6206subD]\nParameterName=ErrorMode8[13]\nObjectType=0x7\nDataType=0x0005\nAccessType=rw\nDefaultValue=255\n\n[6206subE]\nParameterName=ErrorMode8[14]\nObjectType=0x7\nDataType=0x0005\nAccessType=rw\nDefaultValue=255\n\n[6206subF]\nParameterName=ErrorMode8[15]\nObjectType=0x7\nDataType=0x0005\nAccessType=rw\nDefaultValue=255\n\n[6206sub10]\nParameterName=ErrorMode8[16]\nObjectType=0x7\nDataType=0x0005\nAccessType=rw\nDefaultValue=255\n\n[6206sub11]\nParameterName=ErrorMode8[17]\nObjectType=0x7\nDataType=0x0005\nAccessType=rw\nDefaultValue=255\n\n[6206sub12]\nParameterName=ErrorMode8[18]\nObjectType=0x7\nDataType=0x0005\nAccessType=rw\nDefaultValue=255\n\n[6206sub13]\nParameterName=ErrorMode8[19]\nObjectType=0x7\nDataType=0x0005\nAccessType=rw\nDefaultValue=255\n\n[6206sub14]\nParameterName=ErrorMode8[20]\nObjectType=0x7\nDataType=0x0005\nAccessType=rw\nDefaultValue=255\n\n[6207]\nParameterName=Error Value Output 8-Bit\nObjectType=0x8\nSubNumber=21\n\n[6207sub0]\nParameterName=Number of Elements\nObjectType=0x7\nDataType=0x0005\nAccessType=ro\nDefaultValue=20\n\n[6207sub1]\nParameterName=ErrorValue8[1]\nObjectType=0x7\nDataType=0x0005\nAccessType=rw\nDefaultValue=0\n\n[6207sub2]\nParameterName=ErrorValue8[2]\nObjectType=0x7\nDataType=0x0005\nAccessType=rw\nDefaultValue=0\n\n[6207sub3]\nParameterName=ErrorValue8[3]\nObjectType=0x7\nDataType=0x0005\nAccessType=rw\nDefaultValue=0\n\n[6207sub4]\nParameterName=ErrorValue8[4]\nObjectType=0x7\nDataType=0x0005\nAccessType=rw\nDefaultValue=0\n\n[6207sub5]\nParameterName=ErrorValue8[5]\nObjectType=0x7\nDataType=0x0005\nAccessType=rw\nDefaultValue=0\n\n[6207sub6]\nParameterName=ErrorValue8[6]\nObjectType=0x7\nDataType=0x0005\nAccessType=rw\nDefaultValue=0\n\n[6207sub7]\nParameterName=ErrorValue8[7]\nObjectType=0x7\nDataType=0x0005\nAccessType=rw\nDefaultValue=0\n\n[6207sub8]\nParameterName=ErrorValue8[8]\nObjectType=0x7\nDataType=0x0005\nAccessType=rw\nDefaultValue=0\n\n[6207sub9]\nParameterName=ErrorValue8[9]\nObjectType=0x7\nDataType=0x0005\nAccessType=rw\nDefaultValue=0\n\n[6207subA]\nParameterName=ErrorValue8[10]\nObjectType=0x7\nDataType=0x0005\nAccessType=rw\nDefaultValue=0\n\n[6207subB]\nParameterName=ErrorValue8[11]\nObjectType=0x7\nDataType=0x0005\nAccessType=rw\nDefaultValue=0\n\n[6207subC]\nParameterName=ErrorValue8[12]\nObjectType=0x7\nDataType=0x0005\nAccessType=rw\nDefaultValue=0\n\n[6207subD]\nParameterName=ErrorValue8[13]\nObjectType=0x7\nDataType=0x0005\nAccessType=rw\nDefaultValue=0\n\n[6207subE]\nParameterName=ErrorValue8[14]\nObjectType=0x7\nDataType=0x0005\nAccessType=rw\nDefaultValue=0\n\n[6207subF]\nParameterName=ErrorValue8[15]\nObjectType=0x7\nDataType=0x0005\nAccessType=rw\nDefaultValue=0\n\n[6207sub10]\nParameterName=ErrorValue8[16]\nObjectType=0x7\nDataType=0x0005\nAccessType=rw\nDefaultValue=0\n\n[6207sub11]\nParameterName=ErrorValue8[17]\nObjectType=0x7\nDataType=0x0005\nAccessType=rw\nDefaultValue=0\n\n[6207sub12]\nParameterName=ErrorValue8[18]\nObjectType=0x7\nDataType=0x0005\nAccessType=rw\nDefaultValue=0\n\n[6207sub13]\nParameterName=ErrorValue8[19]\nObjectType=0x7\nDataType=0x0005\nAccessType=rw\nDefaultValue=0\n\n[6207sub14]\nParameterName=ErrorValue8[20]\nObjectType=0x7\nDataType=0x0005\nAccessType=rw\nDefaultValue=0\n\n[6400]\nParameterName=Read Analogue Input 8-Bit\nObjectType=0x8\nSubNumber=21\n\n[6400sub0]\nParameterName=Number of Elements\nObjectType=0x7\nDataType=0x0005\nAccessType=ro\nDefaultValue=20\n\n[6400sub1]\nParameterName=AnalogueInput8[1]\nObjectType=0x7\nDataType=0x0002\nAccessType=rwr\nPDOMapping=1\n\n[6400sub2]\nParameterName=AnalogueInput8[2]\nObjectType=0x7\nDataType=0x0002\nAccessType=rwr\nPDOMapping=1\n\n[6400sub3]\nParameterName=AnalogueInput8[3]\nObjectType=0x7\nDataType=0x0002\nAccessType=rwr\nPDOMapping=1\n\n[6400sub4]\nParameterName=AnalogueInput8[4]\nObjectType=0x7\nDataType=0x0002\nAccessType=rwr\nPDOMapping=1\n\n[6400sub5]\nParameterName=AnalogueInput8[5]\nObjectType=0x7\nDataType=0x0002\nAccessType=rwr\nPDOMapping=1\n\n[6400sub6]\nParameterName=AnalogueInput8[6]\nObjectType=0x7\nDataType=0x0002\nAccessType=rwr\nPDOMapping=1\n\n[6400sub7]\nParameterName=AnalogueInput8[7]\nObjectType=0x7\nDataType=0x0002\nAccessType=rwr\nPDOMapping=1\n\n[6400sub8]\nParameterName=AnalogueInput8[8]\nObjectType=0x7\nDataType=0x0002\nAccessType=rwr\nPDOMapping=1\n\n[6400sub9]\nParameterName=AnalogueInput8[9]\nObjectType=0x7\nDataType=0x0002\nAccessType=rwr\nPDOMapping=1\n\n[6400subA]\nParameterName=AnalogueInput8[10]\nObjectType=0x7\nDataType=0x0002\nAccessType=rwr\nPDOMapping=1\n\n[6400subB]\nParameterName=AnalogueInput8[11]\nObjectType=0x7\nDataType=0x0002\nAccessType=rwr\nPDOMapping=1\n\n[6400subC]\nParameterName=AnalogueInput8[12]\nObjectType=0x7\nDataType=0x0002\nAccessType=rwr\nPDOMapping=1\n\n[6400subD]\nParameterName=AnalogueInput8[13]\nObjectType=0x7\nDataType=0x0002\nAccessType=rwr\nPDOMapping=1\n\n[6400subE]\nParameterName=AnalogueInput8[14]\nObjectType=0x7\nDataType=0x0002\nAccessType=rwr\nPDOMapping=1\n\n[6400subF]\nParameterName=AnalogueInput8[15]\nObjectType=0x7\nDataType=0x0002\nAccessType=rwr\nPDOMapping=1\n\n[6400sub10]\nParameterName=AnalogueInput8[16]\nObjectType=0x7\nDataType=0x0002\nAccessType=rwr\nPDOMapping=1\n\n[6400sub11]\nParameterName=AnalogueInput8[17]\nObjectType=0x7\nDataType=0x0002\nAccessType=rwr\nPDOMapping=1\n\n[6400sub12]\nParameterName=AnalogueInput8[18]\nObjectType=0x7\nDataType=0x0002\nAccessType=rwr\nPDOMapping=1\n\n[6400sub13]\nParameterName=AnalogueInput8[19]\nObjectType=0x7\nDataType=0x0002\nAccessType=rwr\nPDOMapping=1\n\n[6400sub14]\nParameterName=AnalogueInput8[20]\nObjectType=0x7\nDataType=0x0002\nAccessType=rwr\nPDOMapping=1\n\n[6401]\nParameterName=Read Analog Input 16 Bit\nObjectType=0x8\nSubNumber=21\n\n[6401sub0]\nParameterName=Number of Elements\nObjectType=0x7\nDataType=0x0005\nAccessType=ro\nDefaultValue=20\n\n[6401sub1]\nParameterName=AnalogueInput16[1]\nObjectType=0x7\nDataType=0x0003\nAccessType=rwr\nPDOMapping=1\n\n[6401sub2]\nParameterName=AnalogueInput16[2]\nObjectType=0x7\nDataType=0x0003\nAccessType=rwr\nPDOMapping=1\n\n[6401sub3]\nParameterName=AnalogueInput16[3]\nObjectType=0x7\nDataType=0x0003\nAccessType=rwr\nPDOMapping=1\n\n[6401sub4]\nParameterName=AnalogueInput16[4]\nObjectType=0x7\nDataType=0x0003\nAccessType=rwr\nPDOMapping=1\n\n[6401sub5]\nParameterName=AnalogueInput16[5]\nObjectType=0x7\nDataType=0x0003\nAccessType=rwr\nPDOMapping=1\n\n[6401sub6]\nParameterName=AnalogueInput16[6]\nObjectType=0x7\nDataType=0x0003\nAccessType=rwr\nPDOMapping=1\n\n[6401sub7]\nParameterName=AnalogueInput16[7]\nObjectType=0x7\nDataType=0x0003\nAccessType=rwr\nPDOMapping=1\n\n[6401sub8]\nParameterName=AnalogueInput16[8]\nObjectType=0x7\nDataType=0x0003\nAccessType=rwr\nPDOMapping=1\n\n[6401sub9]\nParameterName=AnalogueInput16[9]\nObjectType=0x7\nDataType=0x0003\nAccessType=rwr\nPDOMapping=1\n\n[6401subA]\nParameterName=AnalogueInput16[10]\nObjectType=0x7\nDataType=0x0003\nAccessType=rwr\nPDOMapping=1\n\n[6401subB]\nParameterName=AnalogueInput16[11]\nObjectType=0x7\nDataType=0x0003\nAccessType=rwr\nPDOMapping=1\n\n[6401subC]\nParameterName=AnalogueInput16[12]\nObjectType=0x7\nDataType=0x0003\nAccessType=rwr\nPDOMapping=1\n\n[6401subD]\nParameterName=AnalogueInput16[13]\nObjectType=0x7\nDataType=0x0003\nAccessType=rwr\nPDOMapping=1\n\n[6401subE]\nParameterName=AnalogueInput16[14]\nObjectType=0x7\nDataType=0x0003\nAccessType=rwr\nPDOMapping=1\n\n[6401subF]\nParameterName=AnalogueInput16[15]\nObjectType=0x7\nDataType=0x0003\nAccessType=rwr\nPDOMapping=1\n\n[6401sub10]\nParameterName=AnalogueInput16[16]\nObjectType=0x7\nDataType=0x0003\nAccessType=rwr\nPDOMapping=1\n\n[6401sub11]\nParameterName=AnalogueInput16[17]\nObjectType=0x7\nDataType=0x0003\nAccessType=rwr\nPDOMapping=1\n\n[6401sub12]\nParameterName=AnalogueInput16[18]\nObjectType=0x7\nDataType=0x0003\nAccessType=rwr\nPDOMapping=1\n\n[6401sub13]\nParameterName=AnalogueInput16[19]\nObjectType=0x7\nDataType=0x0003\nAccessType=rwr\nPDOMapping=1\n\n[6401sub14]\nParameterName=AnalogueInput16[20]\nObjectType=0x7\nDataType=0x0003\nAccessType=rwr\nPDOMapping=1\n\n[6402]\nParameterName=Read Analogue Input 32-Bit\nObjectType=0x8\nSubNumber=21\n\n[6402sub0]\nParameterName=Number of Elements\nObjectType=0x7\nDataType=0x0005\nAccessType=ro\nDefaultValue=20\n\n[6402sub1]\nParameterName=AnalogueInput32[1]\nObjectType=0x7\nDataType=0x0004\nAccessType=rwr\nPDOMapping=1\n\n[6402sub2]\nParameterName=AnalogueInput32[2]\nObjectType=0x7\nDataType=0x0004\nAccessType=rwr\nPDOMapping=1\n\n[6402sub3]\nParameterName=AnalogueInput32[3]\nObjectType=0x7\nDataType=0x0004\nAccessType=rwr\nPDOMapping=1\n\n[6402sub4]\nParameterName=AnalogueInput32[4]\nObjectType=0x7\nDataType=0x0004\nAccessType=rwr\nPDOMapping=1\n\n[6402sub5]\nParameterName=AnalogueInput32[5]\nObjectType=0x7\nDataType=0x0004\nAccessType=rwr\nPDOMapping=1\n\n[6402sub6]\nParameterName=AnalogueInput32[6]\nObjectType=0x7\nDataType=0x0004\nAccessType=rwr\nPDOMapping=1\n\n[6402sub7]\nParameterName=AnalogueInput32[7]\nObjectType=0x7\nDataType=0x0004\nAccessType=rwr\nPDOMapping=1\n\n[6402sub8]\nParameterName=AnalogueInput32[8]\nObjectType=0x7\nDataType=0x0004\nAccessType=rwr\nPDOMapping=1\n\n[6402sub9]\nParameterName=AnalogueInput32[9]\nObjectType=0x7\nDataType=0x0004\nAccessType=rwr\nPDOMapping=1\n\n[6402subA]\nParameterName=AnalogueInput32[10]\nObjectType=0x7\nDataType=0x0004\nAccessType=rwr\nPDOMapping=1\n\n[6402subB]\nParameterName=AnalogueInput32[11]\nObjectType=0x7\nDataType=0x0004\nAccessType=rwr\nPDOMapping=1\n\n[6402subC]\nParameterName=AnalogueInput32[12]\nObjectType=0x7\nDataType=0x0004\nAccessType=rwr\nPDOMapping=1\n\n[6402subD]\nParameterName=AnalogueInput32[13]\nObjectType=0x7\nDataType=0x0004\nAccessType=rwr\nPDOMapping=1\n\n[6402subE]\nParameterName=AnalogueInput32[14]\nObjectType=0x7\nDataType=0x0004\nAccessType=rwr\nPDOMapping=1\n\n[6402subF]\nParameterName=AnalogueInput32[15]\nObjectType=0x7\nDataType=0x0004\nAccessType=rwr\nPDOMapping=1\n\n[6402sub10]\nParameterName=AnalogueInput32[16]\nObjectType=0x7\nDataType=0x0004\nAccessType=rwr\nPDOMapping=1\n\n[6402sub11]\nParameterName=AnalogueInput32[17]\nObjectType=0x7\nDataType=0x0004\nAccessType=rwr\nPDOMapping=1\n\n[6402sub12]\nParameterName=AnalogueInput32[18]\nObjectType=0x7\nDataType=0x0004\nAccessType=rwr\nPDOMapping=1\n\n[6402sub13]\nParameterName=AnalogueInput32[19]\nObjectType=0x7\nDataType=0x0004\nAccessType=rwr\nPDOMapping=1\n\n[6402sub14]\nParameterName=AnalogueInput32[20]\nObjectType=0x7\nDataType=0x0004\nAccessType=rwr\nPDOMapping=1\n\n[6410]\nParameterName=Write Analogue Output 8-Bit\nObjectType=0x8\nSubNumber=21\n\n[6410sub0]\nParameterName=Number of Elements\nObjectType=0x7\nDataType=0x0005\nAccessType=ro\nDefaultValue=20\n\n[6410sub1]\nParameterName=AnalogueOutput8[1]\nObjectType=0x7\nDataType=0x0002\nAccessType=rww\nPDOMapping=1\n\n[6410sub2]\nParameterName=AnalogueOutput8[2]\nObjectType=0x7\nDataType=0x0002\nAccessType=rww\nPDOMapping=1\n\n[6410sub3]\nParameterName=AnalogueOutput8[3]\nObjectType=0x7\nDataType=0x0002\nAccessType=rww\nPDOMapping=1\n\n[6410sub4]\nParameterName=AnalogueOutput8[4]\nObjectType=0x7\nDataType=0x0002\nAccessType=rww\nPDOMapping=1\n\n[6410sub5]\nParameterName=AnalogueOutput8[5]\nObjectType=0x7\nDataType=0x0002\nAccessType=rww\nPDOMapping=1\n\n[6410sub6]\nParameterName=AnalogueOutput8[6]\nObjectType=0x7\nDataType=0x0002\nAccessType=rww\nPDOMapping=1\n\n[6410sub7]\nParameterName=AnalogueOutput8[7]\nObjectType=0x7\nDataType=0x0002\nAccessType=rww\nPDOMapping=1\n\n[6410sub8]\nParameterName=AnalogueOutput8[8]\nObjectType=0x7\nDataType=0x0002\nAccessType=rww\nPDOMapping=1\n\n[6410sub9]\nParameterName=AnalogueOutput8[9]\nObjectType=0x7\nDataType=0x0002\nAccessType=rww\nPDOMapping=1\n\n[6410subA]\nParameterName=AnalogueOutput8[10]\nObjectType=0x7\nDataType=0x0002\nAccessType=rww\nPDOMapping=1\n\n[6410subB]\nParameterName=AnalogueOutput8[11]\nObjectType=0x7\nDataType=0x0002\nAccessType=rww\nPDOMapping=1\n\n[6410subC]\nParameterName=AnalogueOutput8[12]\nObjectType=0x7\nDataType=0x0002\nAccessType=rww\nPDOMapping=1\n\n[6410subD]\nParameterName=AnalogueOutput8[13]\nObjectType=0x7\nDataType=0x0002\nAccessType=rww\nPDOMapping=1\n\n[6410subE]\nParameterName=AnalogueOutput8[14]\nObjectType=0x7\nDataType=0x0002\nAccessType=rww\nPDOMapping=1\n\n[6410subF]\nParameterName=AnalogueOutput8[15]\nObjectType=0x7\nDataType=0x0002\nAccessType=rww\nPDOMapping=1\n\n[6410sub10]\nParameterName=AnalogueOutput8[16]\nObjectType=0x7\nDataType=0x0002\nAccessType=rww\nPDOMapping=1\n\n[6410sub11]\nParameterName=AnalogueOutput8[17]\nObjectType=0x7\nDataType=0x0002\nAccessType=rww\nPDOMapping=1\n\n[6410sub12]\nParameterName=AnalogueOutput8[18]\nObjectType=0x7\nDataType=0x0002\nAccessType=rww\nPDOMapping=1\n\n[6410sub13]\nParameterName=AnalogueOutput8[19]\nObjectType=0x7\nDataType=0x0002\nAccessType=rww\nPDOMapping=1\n\n[6410sub14]\nParameterName=AnalogueOutput8[20]\nObjectType=0x7\nDataType=0x0002\nAccessType=rww\nPDOMapping=1\n\n[6411]\nParameterName=Write Analog Output 16 Bit\nObjectType=0x8\nSubNumber=21\n\n[6411sub0]\nParameterName=Number of Elements\nObjectType=0x7\nDataType=0x0005\nAccessType=ro\nDefaultValue=20\n\n[6411sub1]\nParameterName=AnalogueOutput16[1]\nObjectType=0x7\nDataType=0x0003\nAccessType=rww\nPDOMapping=1\n\n[6411sub2]\nParameterName=AnalogueOutput16[2]\nObjectType=0x7\nDataType=0x0003\nAccessType=rww\nPDOMapping=1\n\n[6411sub3]\nParameterName=AnalogueOutput16[3]\nObjectType=0x7\nDataType=0x0003\nAccessType=rww\nPDOMapping=1\n\n[6411sub4]\nParameterName=AnalogueOutput16[4]\nObjectType=0x7\nDataType=0x0003\nAccessType=rww\nPDOMapping=1\n\n[6411sub5]\nParameterName=AnalogueOutput16[5]\nObjectType=0x7\nDataType=0x0003\nAccessType=rww\nPDOMapping=1\n\n[6411sub6]\nParameterName=AnalogueOutput16[6]\nObjectType=0x7\nDataType=0x0003\nAccessType=rww\nPDOMapping=1\n\n[6411sub7]\nParameterName=AnalogueOutput16[7]\nObjectType=0x7\nDataType=0x0003\nAccessType=rww\nPDOMapping=1\n\n[6411sub8]\nParameterName=AnalogueOutput16[8]\nObjectType=0x7\nDataType=0x0003\nAccessType=rww\nPDOMapping=1\n\n[6411sub9]\nParameterName=AnalogueOutput16[9]\nObjectType=0x7\nDataType=0x0003\nAccessType=rww\nPDOMapping=1\n\n[6411subA]\nParameterName=AnalogueOutput16[10]\nObjectType=0x7\nDataType=0x0003\nAccessType=rww\nPDOMapping=1\n\n[6411subB]\nParameterName=AnalogueOutput16[11]\nObjectType=0x7\nDataType=0x0003\nAccessType=rww\nPDOMapping=1\n\n[6411subC]\nParameterName=AnalogueOutput16[12]\nObjectType=0x7\nDataType=0x0003\nAccessType=rww\nPDOMapping=1\n\n[6411subD]\nParameterName=AnalogueOutput16[13]\nObjectType=0x7\nDataType=0x0003\nAccessType=rww\nPDOMapping=1\n\n[6411subE]\nParameterName=AnalogueOutput16[14]\nObjectType=0x7\nDataType=0x0003\nAccessType=rww\nPDOMapping=1\n\n[6411subF]\nParameterName=AnalogueOutput16[15]\nObjectType=0x7\nDataType=0x0003\nAccessType=rww\nPDOMapping=1\n\n[6411sub10]\nParameterName=AnalogueOutput16[16]\nObjectType=0x7\nDataType=0x0003\nAccessType=rww\nPDOMapping=1\n\n[6411sub11]\nParameterName=AnalogueOutput16[17]\nObjectType=0x7\nDataType=0x0003\nAccessType=rww\nPDOMapping=1\n\n[6411sub12]\nParameterName=AnalogueOutput16[18]\nObjectType=0x7\nDataType=0x0003\nAccessType=rww\nPDOMapping=1\n\n[6411sub13]\nParameterName=AnalogueOutput16[19]\nObjectType=0x7\nDataType=0x0003\nAccessType=rww\nPDOMapping=1\n\n[6411sub14]\nParameterName=AnalogueOutput16[20]\nObjectType=0x7\nDataType=0x0003\nAccessType=rww\nPDOMapping=1\n\n[6412]\nParameterName=Write Analogue Output 32-Bit\nObjectType=0x8\nSubNumber=21\n\n[6412sub0]\nParameterName=Number of Elements\nObjectType=0x7\nDataType=0x0005\nAccessType=ro\nDefaultValue=20\n\n[6412sub1]\nParameterName=AnalogueOutput32[1]\nObjectType=0x7\nDataType=0x0004\nAccessType=rww\nPDOMapping=1\n\n[6412sub2]\nParameterName=AnalogueOutput32[2]\nObjectType=0x7\nDataType=0x0004\nAccessType=rww\nPDOMapping=1\n\n[6412sub3]\nParameterName=AnalogueOutput32[3]\nObjectType=0x7\nDataType=0x0004\nAccessType=rww\nPDOMapping=1\n\n[6412sub4]\nParameterName=AnalogueOutput32[4]\nObjectType=0x7\nDataType=0x0004\nAccessType=rww\nPDOMapping=1\n\n[6412sub5]\nParameterName=AnalogueOutput32[5]\nObjectType=0x7\nDataType=0x0004\nAccessType=rww\nPDOMapping=1\n\n[6412sub6]\nParameterName=AnalogueOutput32[6]\nObjectType=0x7\nDataType=0x0004\nAccessType=rww\nPDOMapping=1\n\n[6412sub7]\nParameterName=AnalogueOutput32[7]\nObjectType=0x7\nDataType=0x0004\nAccessType=rww\nPDOMapping=1\n\n[6412sub8]\nParameterName=AnalogueOutput32[8]\nObjectType=0x7\nDataType=0x0004\nAccessType=rww\nPDOMapping=1\n\n[6412sub9]\nParameterName=AnalogueOutput32[9]\nObjectType=0x7\nDataType=0x0004\nAccessType=rww\nPDOMapping=1\n\n[6412subA]\nParameterName=AnalogueOutput32[10]\nObjectType=0x7\nDataType=0x0004\nAccessType=rww\nPDOMapping=1\n\n[6412subB]\nParameterName=AnalogueOutput32[11]\nObjectType=0x7\nDataType=0x0004\nAccessType=rww\nPDOMapping=1\n\n[6412subC]\nParameterName=AnalogueOutput32[12]\nObjectType=0x7\nDataType=0x0004\nAccessType=rww\nPDOMapping=1\n\n[6412subD]\nParameterName=AnalogueOutput32[13]\nObjectType=0x7\nDataType=0x0004\nAccessType=rww\nPDOMapping=1\n\n[6412subE]\nParameterName=AnalogueOutput32[14]\nObjectType=0x7\nDataType=0x0004\nAccessType=rww\nPDOMapping=1\n\n[6412subF]\nParameterName=AnalogueOutput32[15]\nObjectType=0x7\nDataType=0x0004\nAccessType=rww\nPDOMapping=1\n\n[6412sub10]\nParameterName=AnalogueOutput32[16]\nObjectType=0x7\nDataType=0x0004\nAccessType=rww\nPDOMapping=1\n\n[6412sub11]\nParameterName=AnalogueOutput32[17]\nObjectType=0x7\nDataType=0x0004\nAccessType=rww\nPDOMapping=1\n\n[6412sub12]\nParameterName=AnalogueOutput32[18]\nObjectType=0x7\nDataType=0x0004\nAccessType=rww\nPDOMapping=1\n\n[6412sub13]\nParameterName=AnalogueOutput32[19]\nObjectType=0x7\nDataType=0x0004\nAccessType=rww\nPDOMapping=1\n\n[6412sub14]\nParameterName=AnalogueOutput32[20]\nObjectType=0x7\nDataType=0x0004\nAccessType=rww\nPDOMapping=1\n\n[6421]\nParameterName=Interrupt Trigger Selection\nObjectType=0x8\nSubNumber=21\n\n[6421sub0]\nParameterName=Number of Elements\nObjectType=0x7\nDataType=0x0005\nAccessType=ro\nDefaultValue=20\n\n[6421sub1]\nParameterName=InterruptTriggerSelection\nObjectType=0x7\nDataType=0x0005\nAccessType=rw\nDefaultValue=7\nLowLimit=0\nHighLimit=7\n\n[6421sub2]\nParameterName=InterruptTriggerSelection\nObjectType=0x7\nDataType=0x0005\nAccessType=rw\nDefaultValue=7\nLowLimit=0\nHighLimit=7\n\n[6421sub3]\nParameterName=InterruptTriggerSelection\nObjectType=0x7\nDataType=0x0005\nAccessType=rw\nDefaultValue=7\nLowLimit=0\nHighLimit=7\n\n[6421sub4]\nParameterName=InterruptTriggerSelection\nObjectType=0x7\nDataType=0x0005\nAccessType=rw\nDefaultValue=7\nLowLimit=0\nHighLimit=7\n\n[6421sub5]\nParameterName=InterruptTriggerSelection\nObjectType=0x7\nDataType=0x0005\nAccessType=rw\nDefaultValue=7\nLowLimit=0\nHighLimit=7\n\n[6421sub6]\nParameterName=InterruptTriggerSelection\nObjectType=0x7\nDataType=0x0005\nAccessType=rw\nDefaultValue=7\nLowLimit=0\nHighLimit=7\n\n[6421sub7]\nParameterName=InterruptTriggerSelection\nObjectType=0x7\nDataType=0x0005\nAccessType=rw\nDefaultValue=7\nLowLimit=0\nHighLimit=7\n\n[6421sub8]\nParameterName=InterruptTriggerSelection\nObjectType=0x7\nDataType=0x0005\nAccessType=rw\nDefaultValue=7\nLowLimit=0\nHighLimit=7\n\n[6421sub9]\nParameterName=InterruptTriggerSelection\nObjectType=0x7\nDataType=0x0005\nAccessType=rw\nDefaultValue=7\nLowLimit=0\nHighLimit=7\n\n[6421subA]\nParameterName=InterruptTriggerSelection\nObjectType=0x7\nDataType=0x0005\nAccessType=rw\nDefaultValue=7\nLowLimit=0\nHighLimit=7\n\n[6421subB]\nParameterName=InterruptTriggerSelection\nObjectType=0x7\nDataType=0x0005\nAccessType=rw\nDefaultValue=7\nLowLimit=0\nHighLimit=7\n\n[6421subC]\nParameterName=InterruptTriggerSelection\nObjectType=0x7\nDataType=0x0005\nAccessType=rw\nDefaultValue=7\nLowLimit=0\nHighLimit=7\n\n[6421subD]\nParameterName=InterruptTriggerSelection\nObjectType=0x7\nDataType=0x0005\nAccessType=rw\nDefaultValue=7\nLowLimit=0\nHighLimit=7\n\n[6421subE]\nParameterName=InterruptTriggerSelection\nObjectType=0x7\nDataType=0x0005\nAccessType=rw\nDefaultValue=7\nLowLimit=0\nHighLimit=7\n\n[6421subF]\nParameterName=InterruptTriggerSelection\nObjectType=0x7\nDataType=0x0005\nAccessType=rw\nDefaultValue=7\nLowLimit=0\nHighLimit=7\n\n[6421sub10]\nParameterName=InterruptTriggerSelection\nObjectType=0x7\nDataType=0x0005\nAccessType=rw\nDefaultValue=7\nLowLimit=0\nHighLimit=7\n\n[6421sub11]\nParameterName=InterruptTriggerSelection\nObjectType=0x7\nDataType=0x0005\nAccessType=rw\nDefaultValue=7\nLowLimit=0\nHighLimit=7\n\n[6421sub12]\nParameterName=InterruptTriggerSelection\nObjectType=0x7\nDataType=0x0005\nAccessType=rw\nDefaultValue=7\nLowLimit=0\nHighLimit=7\n\n[6421sub13]\nParameterName=InterruptTriggerSelection\nObjectType=0x7\nDataType=0x0005\nAccessType=rw\nDefaultValue=7\nLowLimit=0\nHighLimit=7\n\n[6421sub14]\nParameterName=InterruptTriggerSelection\nObjectType=0x7\nDataType=0x0005\nAccessType=rw\nDefaultValue=7\nLowLimit=0\nHighLimit=7\n\n[6423]\nParameterName=Global Analog Interrupt Enable\nObjectType=0x7\nDataType=0x0001\nAccessType=rw\nDefaultValue=1\nPDOMapping=0\n\n[6424]\nParameterName=Analogue Input Interrupt Upper Limit Integer\nObjectType=0x8\nSubNumber=21\n\n[6424sub0]\nParameterName=Number of Elements\nObjectType=0x7\nDataType=0x0005\nAccessType=ro\nDefaultValue=20\n\n[6424sub1]\nParameterName=InterruptUpperLimInt\nObjectType=0x7\nDataType=0x0004\nAccessType=rw\nDefaultValue=0\n\n[6424sub2]\nParameterName=InterruptUpperLimInt\nObjectType=0x7\nDataType=0x0004\nAccessType=rw\nDefaultValue=0\n\n[6424sub3]\nParameterName=InterruptUpperLimInt\nObjectType=0x7\nDataType=0x0004\nAccessType=rw\nDefaultValue=0\n\n[6424sub4]\nParameterName=InterruptUpperLimInt\nObjectType=0x7\nDataType=0x0004\nAccessType=rw\nDefaultValue=0\n\n[6424sub5]\nParameterName=InterruptUpperLimInt\nObjectType=0x7\nDataType=0x0004\nAccessType=rw\nDefaultValue=0\n\n[6424sub6]\nParameterName=InterruptUpperLimInt\nObjectType=0x7\nDataType=0x0004\nAccessType=rw\nDefaultValue=0\n\n[6424sub7]\nParameterName=InterruptUpperLimInt\nObjectType=0x7\nDataType=0x0004\nAccessType=rw\nDefaultValue=0\n\n[6424sub8]\nParameterName=InterruptUpperLimInt\nObjectType=0x7\nDataType=0x0004\nAccessType=rw\nDefaultValue=0\n\n[6424sub9]\nParameterName=InterruptUpperLimInt\nObjectType=0x7\nDataType=0x0004\nAccessType=rw\nDefaultValue=0\n\n[6424subA]\nParameterName=InterruptUpperLimInt\nObjectType=0x7\nDataType=0x0004\nAccessType=rw\nDefaultValue=0\n\n[6424subB]\nParameterName=InterruptUpperLimInt\nObjectType=0x7\nDataType=0x0004\nAccessType=rw\nDefaultValue=0\n\n[6424subC]\nParameterName=InterruptUpperLimInt\nObjectType=0x7\nDataType=0x0004\nAccessType=rw\nDefaultValue=0\n\n[6424subD]\nParameterName=InterruptUpperLimInt\nObjectType=0x7\nDataType=0x0004\nAccessType=rw\nDefaultValue=0\n\n[6424subE]\nParameterName=InterruptUpperLimInt\nObjectType=0x7\nDataType=0x0004\nAccessType=rw\nDefaultValue=0\n\n[6424subF]\nParameterName=InterruptUpperLimInt\nObjectType=0x7\nDataType=0x0004\nAccessType=rw\nDefaultValue=0\n\n[6424sub10]\nParameterName=InterruptUpperLimInt\nObjectType=0x7\nDataType=0x0004\nAccessType=rw\nDefaultValue=0\n\n[6424sub11]\nParameterName=InterruptUpperLimInt\nObjectType=0x7\nDataType=0x0004\nAccessType=rw\nDefaultValue=0\n\n[6424sub12]\nParameterName=InterruptUpperLimInt\nObjectType=0x7\nDataType=0x0004\nAccessType=rw\nDefaultValue=0\n\n[6424sub13]\nParameterName=InterruptUpperLimInt\nObjectType=0x7\nDataType=0x0004\nAccessType=rw\nDefaultValue=0\n\n[6424sub14]\nParameterName=InterruptUpperLimInt\nObjectType=0x7\nDataType=0x0004\nAccessType=rw\nDefaultValue=0\n\n[6425]\nParameterName=Analogue Input Interrupt Lower Limit Integer\nObjectType=0x8\nSubNumber=21\n\n[6425sub0]\nParameterName=Number of Elements\nObjectType=0x7\nDataType=0x0005\nAccessType=ro\nDefaultValue=20\n\n[6425sub1]\nParameterName=InterruptLowerLimInt\nObjectType=0x7\nDataType=0x0004\nAccessType=rw\nDefaultValue=0\n\n[6425sub2]\nParameterName=InterruptLowerLimInt\nObjectType=0x7\nDataType=0x0004\nAccessType=rw\nDefaultValue=0\n\n[6425sub3]\nParameterName=InterruptLowerLimInt\nObjectType=0x7\nDataType=0x0004\nAccessType=rw\nDefaultValue=0\n\n[6425sub4]\nParameterName=InterruptLowerLimInt\nObjectType=0x7\nDataType=0x0004\nAccessType=rw\nDefaultValue=0\n\n[6425sub5]\nParameterName=InterruptLowerLimInt\nObjectType=0x7\nDataType=0x0004\nAccessType=rw\nDefaultValue=0\n\n[6425sub6]\nParameterName=InterruptLowerLimInt\nObjectType=0x7\nDataType=0x0004\nAccessType=rw\nDefaultValue=0\n\n[6425sub7]\nParameterName=InterruptLowerLimInt\nObjectType=0x7\nDataType=0x0004\nAccessType=rw\nDefaultValue=0\n\n[6425sub8]\nParameterName=InterruptLowerLimInt\nObjectType=0x7\nDataType=0x0004\nAccessType=rw\nDefaultValue=0\n\n[6425sub9]\nParameterName=InterruptLowerLimInt\nObjectType=0x7\nDataType=0x0004\nAccessType=rw\nDefaultValue=0\n\n[6425subA]\nParameterName=InterruptLowerLimInt\nObjectType=0x7\nDataType=0x0004\nAccessType=rw\nDefaultValue=0\n\n[6425subB]\nParameterName=InterruptLowerLimInt\nObjectType=0x7\nDataType=0x0004\nAccessType=rw\nDefaultValue=0\n\n[6425subC]\nParameterName=InterruptLowerLimInt\nObjectType=0x7\nDataType=0x0004\nAccessType=rw\nDefaultValue=0\n\n[6425subD]\nParameterName=InterruptLowerLimInt\nObjectType=0x7\nDataType=0x0004\nAccessType=rw\nDefaultValue=0\n\n[6425subE]\nParameterName=InterruptLowerLimInt\nObjectType=0x7\nDataType=0x0004\nAccessType=rw\nDefaultValue=0\n\n[6425subF]\nParameterName=InterruptLowerLimInt\nObjectType=0x7\nDataType=0x0004\nAccessType=rw\nDefaultValue=0\n\n[6425sub10]\nParameterName=InterruptLowerLimInt\nObjectType=0x7\nDataType=0x0004\nAccessType=rw\nDefaultValue=0\n\n[6425sub11]\nParameterName=InterruptLowerLimInt\nObjectType=0x7\nDataType=0x0004\nAccessType=rw\nDefaultValue=0\n\n[6425sub12]\nParameterName=InterruptLowerLimInt\nObjectType=0x7\nDataType=0x0004\nAccessType=rw\nDefaultValue=0\n\n[6425sub13]\nParameterName=InterruptLowerLimInt\nObjectType=0x7\nDataType=0x0004\nAccessType=rw\nDefaultValue=0\n\n[6425sub14]\nParameterName=InterruptLowerLimInt\nObjectType=0x7\nDataType=0x0004\nAccessType=rw\nDefaultValue=0\n\n[6426]\nParameterName=Analogue Input Interrupt Delta Unsigned\nObjectType=0x8\nSubNumber=21\n\n[6426sub0]\nParameterName=Number of Elements\nObjectType=0x7\nDataType=0x0005\nAccessType=ro\nDefaultValue=20\n\n[6426sub1]\nParameterName=InterruptDeltaUInt\nObjectType=0x7\nDataType=0x0007\nAccessType=rw\nDefaultValue=0\n\n[6426sub2]\nParameterName=InterruptDeltaUInt\nObjectType=0x7\nDataType=0x0007\nAccessType=rw\nDefaultValue=0\n\n[6426sub3]\nParameterName=InterruptDeltaUInt\nObjectType=0x7\nDataType=0x0007\nAccessType=rw\nDefaultValue=0\n\n[6426sub4]\nParameterName=InterruptDeltaUInt\nObjectType=0x7\nDataType=0x0007\nAccessType=rw\nDefaultValue=0\n\n[6426sub5]\nParameterName=InterruptDeltaUInt\nObjectType=0x7\nDataType=0x0007\nAccessType=rw\nDefaultValue=0\n\n[6426sub6]\nParameterName=InterruptDeltaUInt\nObjectType=0x7\nDataType=0x0007\nAccessType=rw\nDefaultValue=0\n\n[6426sub7]\nParameterName=InterruptDeltaUInt\nObjectType=0x7\nDataType=0x0007\nAccessType=rw\nDefaultValue=0\n\n[6426sub8]\nParameterName=InterruptDeltaUInt\nObjectType=0x7\nDataType=0x0007\nAccessType=rw\nDefaultValue=0\n\n[6426sub9]\nParameterName=InterruptDeltaUInt\nObjectType=0x7\nDataType=0x0007\nAccessType=rw\nDefaultValue=0\n\n[6426subA]\nParameterName=InterruptDeltaUInt\nObjectType=0x7\nDataType=0x0007\nAccessType=rw\nDefaultValue=0\n\n[6426subB]\nParameterName=InterruptDeltaUInt\nObjectType=0x7\nDataType=0x0007\nAccessType=rw\nDefaultValue=0\n\n[6426subC]\nParameterName=InterruptDeltaUInt\nObjectType=0x7\nDataType=0x0007\nAccessType=rw\nDefaultValue=0\n\n[6426subD]\nParameterName=InterruptDeltaUInt\nObjectType=0x7\nDataType=0x0007\nAccessType=rw\nDefaultValue=0\n\n[6426subE]\nParameterName=InterruptDeltaUInt\nObjectType=0x7\nDataType=0x0007\nAccessType=rw\nDefaultValue=0\n\n[6426subF]\nParameterName=InterruptDeltaUInt\nObjectType=0x7\nDataType=0x0007\nAccessType=rw\nDefaultValue=0\n\n[6426sub10]\nParameterName=InterruptDeltaUInt\nObjectType=0x7\nDataType=0x0007\nAccessType=rw\nDefaultValue=0\n\n[6426sub11]\nParameterName=InterruptDeltaUInt\nObjectType=0x7\nDataType=0x0007\nAccessType=rw\nDefaultValue=0\n\n[6426sub12]\nParameterName=InterruptDeltaUInt\nObjectType=0x7\nDataType=0x0007\nAccessType=rw\nDefaultValue=0\n\n[6426sub13]\nParameterName=InterruptDeltaUInt\nObjectType=0x7\nDataType=0x0007\nAccessType=rw\nDefaultValue=0\n\n[6426sub14]\nParameterName=InterruptDeltaUInt\nObjectType=0x7\nDataType=0x0007\nAccessType=rw\nDefaultValue=0\n\n[6443]\nParameterName=Analogue Output Error Mode\nObjectType=0x8\nSubNumber=21\n\n[6443sub0]\nParameterName=Number of Elements\nObjectType=0x7\nDataType=0x0005\nAccessType=ro\nDefaultValue=20\n\n[6443sub1]\nParameterName=ErrorMode\nObjectType=0x7\nDataType=0x0005\nAccessType=rw\nDefaultValue=1\n\n[6443sub2]\nParameterName=ErrorMode\nObjectType=0x7\nDataType=0x0005\nAccessType=rw\nDefaultValue=1\n\n[6443sub3]\nParameterName=ErrorMode\nObjectType=0x7\nDataType=0x0005\nAccessType=rw\nDefaultValue=1\n\n[6443sub4]\nParameterName=ErrorMode\nObjectType=0x7\nDataType=0x0005\nAccessType=rw\nDefaultValue=1\n\n[6443sub5]\nParameterName=ErrorMode\nObjectType=0x7\nDataType=0x0005\nAccessType=rw\nDefaultValue=1\n\n[6443sub6]\nParameterName=ErrorMode\nObjectType=0x7\nDataType=0x0005\nAccessType=rw\nDefaultValue=1\n\n[6443sub7]\nParameterName=ErrorMode\nObjectType=0x7\nDataType=0x0005\nAccessType=rw\nDefaultValue=1\n\n[6443sub8]\nParameterName=ErrorMode\nObjectType=0x7\nDataType=0x0005\nAccessType=rw\nDefaultValue=1\n\n[6443sub9]\nParameterName=ErrorMode\nObjectType=0x7\nDataType=0x0005\nAccessType=rw\nDefaultValue=1\n\n[6443subA]\nParameterName=ErrorMode\nObjectType=0x7\nDataType=0x0005\nAccessType=rw\nDefaultValue=1\n\n[6443subB]\nParameterName=ErrorMode\nObjectType=0x7\nDataType=0x0005\nAccessType=rw\nDefaultValue=1\n\n[6443subC]\nParameterName=ErrorMode\nObjectType=0x7\nDataType=0x0005\nAccessType=rw\nDefaultValue=1\n\n[6443subD]\nParameterName=ErrorMode\nObjectType=0x7\nDataType=0x0005\nAccessType=rw\nDefaultValue=1\n\n[6443subE]\nParameterName=ErrorMode\nObjectType=0x7\nDataType=0x0005\nAccessType=rw\nDefaultValue=1\n\n[6443subF]\nParameterName=ErrorMode\nObjectType=0x7\nDataType=0x0005\nAccessType=rw\nDefaultValue=1\n\n[6443sub10]\nParameterName=ErrorMode\nObjectType=0x7\nDataType=0x0005\nAccessType=rw\nDefaultValue=1\n\n[6443sub11]\nParameterName=ErrorMode\nObjectType=0x7\nDataType=0x0005\nAccessType=rw\nDefaultValue=1\n\n[6443sub12]\nParameterName=ErrorMode\nObjectType=0x7\nDataType=0x0005\nAccessType=rw\nDefaultValue=1\n\n[6443sub13]\nParameterName=ErrorMode\nObjectType=0x7\nDataType=0x0005\nAccessType=rw\nDefaultValue=1\n\n[6443sub14]\nParameterName=ErrorMode\nObjectType=0x7\nDataType=0x0005\nAccessType=rw\nDefaultValue=1\n\n[6444]\nParameterName=Analogue Output Error Value Integer\nObjectType=0x8\nSubNumber=21\n\n[6444sub0]\nParameterName=Number of Elements\nObjectType=0x7\nDataType=0x0005\nAccessType=ro\nDefaultValue=20\n\n[6444sub1]\nParameterName=ErrorValueInt\nObjectType=0x7\nDataType=0x0004\nAccessType=rw\nDefaultValue=0\n\n[6444sub2]\nParameterName=ErrorValueInt\nObjectType=0x7\nDataType=0x0004\nAccessType=rw\nDefaultValue=0\n\n[6444sub3]\nParameterName=ErrorValueInt\nObjectType=0x7\nDataType=0x0004\nAccessType=rw\nDefaultValue=0\n\n[6444sub4]\nParameterName=ErrorValueInt\nObjectType=0x7\nDataType=0x0004\nAccessType=rw\nDefaultValue=0\n\n[6444sub5]\nParameterName=ErrorValueInt\nObjectType=0x7\nDataType=0x0004\nAccessType=rw\nDefaultValue=0\n\n[6444sub6]\nParameterName=ErrorValueInt\nObjectType=0x7\nDataType=0x0004\nAccessType=rw\nDefaultValue=0\n\n[6444sub7]\nParameterName=ErrorValueInt\nObjectType=0x7\nDataType=0x0004\nAccessType=rw\nDefaultValue=0\n\n[6444sub8]\nParameterName=ErrorValueInt\nObjectType=0x7\nDataType=0x0004\nAccessType=rw\nDefaultValue=0\n\n[6444sub9]\nParameterName=ErrorValueInt\nObjectType=0x7\nDataType=0x0004\nAccessType=rw\nDefaultValue=0\n\n[6444subA]\nParameterName=ErrorValueInt\nObjectType=0x7\nDataType=0x0004\nAccessType=rw\nDefaultValue=0\n\n[6444subB]\nParameterName=ErrorValueInt\nObjectType=0x7\nDataType=0x0004\nAccessType=rw\nDefaultValue=0\n\n[6444subC]\nParameterName=ErrorValueInt\nObjectType=0x7\nDataType=0x0004\nAccessType=rw\nDefaultValue=0\n\n[6444subD]\nParameterName=ErrorValueInt\nObjectType=0x7\nDataType=0x0004\nAccessType=rw\nDefaultValue=0\n\n[6444subE]\nParameterName=ErrorValueInt\nObjectType=0x7\nDataType=0x0004\nAccessType=rw\nDefaultValue=0\n\n[6444subF]\nParameterName=ErrorValueInt\nObjectType=0x7\nDataType=0x0004\nAccessType=rw\nDefaultValue=0\n\n[6444sub10]\nParameterName=ErrorValueInt\nObjectType=0x7\nDataType=0x0004\nAccessType=rw\nDefaultValue=0\n\n[6444sub11]\nParameterName=ErrorValueInt\nObjectType=0x7\nDataType=0x0004\nAccessType=rw\nDefaultValue=0\n\n[6444sub12]\nParameterName=ErrorValueInt\nObjectType=0x7\nDataType=0x0004\nAccessType=rw\nDefaultValue=0\n\n[6444sub13]\nParameterName=ErrorValueInt\nObjectType=0x7\nDataType=0x0004\nAccessType=rw\nDefaultValue=0\n\n[6444sub14]\nParameterName=ErrorValueInt\nObjectType=0x7\nDataType=0x0004\nAccessType=rw\nDefaultValue=0\n\n[ManufacturerObjects]\nSupportedObjects=193\n1=0x2010\n2=0x2041\n3=0x2100\n4=0x2200\n5=0x3000\n6=0x3001\n7=0x3011\n8=0x30A1\n9=0x30B2\n10=0x3100\n11=0x3101\n12=0x3102\n13=0x3103\n14=0x3104\n15=0x3105\n16=0x3106\n17=0x3107\n18=0x3108\n19=0x3109\n20=0x310A\n21=0x310B\n22=0x310C\n23=0x310D\n24=0x310E\n25=0x310F\n26=0x3110\n27=0x3111\n28=0x3112\n29=0x3113\n30=0x3200\n31=0x3201\n32=0x3202\n33=0x3203\n34=0x3204\n35=0x3205\n36=0x3206\n37=0x3207\n38=0x3208\n39=0x3209\n40=0x320A\n41=0x320B\n42=0x320C\n43=0x320D\n44=0x320E\n45=0x320F\n46=0x3210\n47=0x3211\n48=0x3212\n49=0x3213\n50=0x3300\n51=0x3301\n52=0x3302\n53=0x3303\n54=0x3304\n55=0x3305\n56=0x3306\n57=0x3307\n58=0x3308\n59=0x3309\n60=0x330A\n61=0x330B\n62=0x330C\n63=0x330D\n64=0x330E\n65=0x330F\n66=0x3310\n67=0x3311\n68=0x3312\n69=0x3313\n70=0x3314\n71=0x3400\n72=0x3401\n73=0x3402\n74=0x3403\n75=0x3404\n76=0x3405\n77=0x3406\n78=0x3407\n79=0x3408\n80=0x3409\n81=0x340A\n82=0x340B\n83=0x340C\n84=0x340D\n85=0x340E\n86=0x340F\n87=0x3410\n88=0x3411\n89=0x3412\n90=0x3413\n91=0x3500\n92=0x3501\n93=0x3502\n94=0x3503\n95=0x3504\n96=0x3505\n97=0x3506\n98=0x3507\n99=0x3508\n100=0x3509\n101=0x350A\n102=0x350B\n103=0x350C\n104=0x350D\n105=0x350E\n106=0x350F\n107=0x3510\n108=0x3511\n109=0x3512\n110=0x3513\n111=0x3600\n112=0x3601\n113=0x3602\n114=0x3603\n115=0x3604\n116=0x3605\n117=0x3606\n118=0x3607\n119=0x3608\n120=0x3609\n121=0x360A\n122=0x360B\n123=0x360C\n124=0x360D\n125=0x360E\n126=0x360F\n127=0x3610\n128=0x3611\n129=0x3612\n130=0x3613\n131=0x3700\n132=0x3701\n133=0x3702\n134=0x3703\n135=0x3704\n136=0x3705\n137=0x3706\n138=0x3707\n139=0x3708\n140=0x3709\n141=0x370A\n142=0x370B\n143=0x370C\n144=0x370D\n145=0x370E\n146=0x370F\n147=0x3710\n148=0x3711\n149=0x3712\n150=0x3713\n151=0x3800\n152=0x3801\n153=0x3802\n154=0x3803\n155=0x3804\n156=0x3805\n157=0x3806\n158=0x3807\n159=0x3808\n160=0x3809\n161=0x380A\n162=0x380B\n163=0x380C\n164=0x380D\n165=0x380E\n166=0x380F\n167=0x3810\n168=0x3811\n169=0x3812\n170=0x3813\n171=0x3900\n172=0x3901\n173=0x3902\n174=0x3903\n175=0x3904\n176=0x3905\n177=0x3906\n178=0x3907\n179=0x3908\n180=0x3909\n181=0x390A\n182=0x390B\n183=0x390C\n184=0x390D\n185=0x390E\n186=0x390F\n187=0x3910\n188=0x3911\n189=0x3912\n190=0x3913\n191=0x3FFD\n192=0x3FFE\n193=0x3FFF\n\n[2010]\nParameterName=Control Object\nObjectType=0x9\nSubNumber=2\n\n[2010sub0]\nParameterName=Number of Entries\nObjectType=0x7\nDataType=0x0005\nAccessType=ro\nDefaultValue=1\n\n[2010sub1]\nParameterName=Simple_Profile_BOOL\nObjectType=0x7\nDataType=0x0001\nAccessType=rw\nDefaultValue=0x0\nLowLimit=0x0\nHighLimit=0x1\n\n[2041]\nParameterName=Buscontroller settings\nObjectType=0x9\nSubNumber=2\n\n[2041sub0]\nParameterName=Number of Entries\nObjectType=0x7\nDataType=0x0005\nAccessType=ro\nDefaultValue=4\nLowLimit=0x00\nHighLimit=0xFF\n\n[2041sub4]\nParameterName=Handle bus error\nObjectType=0x7\nDataType=0x0001\nAccessType=rw\nDefaultValue=0x1\nLowLimit=0x0\nHighLimit=0x1\n\n[2100]\nParameterName=Object 2100 - IO Mask for DMxxxx Modules\nObjectType=0x8\nSubNumber=21\n\n[2100sub0]\nParameterName=Number of Elements\nObjectType=0x7\nDataType=0x0005\nAccessType=ro\nDefaultValue=0x14\n\n[2100sub1]\nParameterName=IO Mask for Channel 1-8\nObjectType=0x7\nDataType=0x0005\nAccessType=rw\nDefaultValue=0x0\nLowLimit=0x0\nHighLimit=0xFF\n\n[2100sub2]\nParameterName=IO Mask for Channel 9-16\nObjectType=0x7\nDataType=0x0005\nAccessType=rw\nDefaultValue=0x0\nLowLimit=0x0\nHighLimit=0xFF\n\n[2100sub3]\nParameterName=IO Mask for Channel 17-24\nObjectType=0x7\nDataType=0x0005\nAccessType=rw\nDefaultValue=0x0\nLowLimit=0x0\nHighLimit=0xFF\n\n[2100sub4]\nParameterName=IO Mask for Channel 25-32\nObjectType=0x7\nDataType=0x0005\nAccessType=rw\nDefaultValue=0x0\nLowLimit=0x0\nHighLimit=0xFF\n\n[2100sub5]\nParameterName=IO Mask for Channel 33-40\nObjectType=0x7\nDataType=0x0005\nAccessType=rw\nDefaultValue=0x0\nLowLimit=0x0\nHighLimit=0xFF\n\n[2100sub6]\nParameterName=IO Mask for Channel 41-48\nObjectType=0x7\nDataType=0x0005\nAccessType=rw\nDefaultValue=0x0\nLowLimit=0x0\nHighLimit=0xFF\n\n[2100sub7]\nParameterName=IO Mask for Channel 49-56\nObjectType=0x7\nDataType=0x0005\nAccessType=rw\nDefaultValue=0x0\nLowLimit=0x0\nHighLimit=0xFF\n\n[2100sub8]\nParameterName=IO Mask for Channel 57-64\nObjectType=0x7\nDataType=0x0005\nAccessType=rw\nDefaultValue=0x0\nLowLimit=0x0\nHighLimit=0xFF\n\n[2100sub9]\nParameterName=IO Mask for Channel 65-72\nObjectType=0x7\nDataType=0x0005\nAccessType=rw\nDefaultValue=0x0\nLowLimit=0x0\nHighLimit=0xFF\n\n[2100subA]\nParameterName=IO Mask for Channel 73-80\nObjectType=0x7\nDataType=0x0005\nAccessType=rw\nDefaultValue=0x0\nLowLimit=0x0\nHighLimit=0xFF\n\n[2100subB]\nParameterName=IO Mask for Channel 81-88\nObjectType=0x7\nDataType=0x0005\nAccessType=rw\nDefaultValue=0x0\nLowLimit=0x0\nHighLimit=0xFF\n\n[2100subC]\nParameterName=IO Mask for Channel 89-96\nObjectType=0x7\nDataType=0x0005\nAccessType=rw\nDefaultValue=0x0\nLowLimit=0x0\nHighLimit=0xFF\n\n[2100subD]\nParameterName=IO Mask for Channel 97-104\nObjectType=0x7\nDataType=0x0005\nAccessType=rw\nDefaultValue=0x0\nLowLimit=0x0\nHighLimit=0xFF\n\n[2100subE]\nParameterName=IO Mask for Channel 105-112\nObjectType=0x7\nDataType=0x0005\nAccessType=rw\nDefaultValue=0x0\nLowLimit=0x0\nHighLimit=0xFF\n\n[2100subF]\nParameterName=IO Mask for Channel 113-120\nObjectType=0x7\nDataType=0x0005\nAccessType=rw\nDefaultValue=0x0\nLowLimit=0x0\nHighLimit=0xFF\n\n[2100sub10]\nParameterName=IO Mask for Channel 121-128\nObjectType=0x7\nDataType=0x0005\nAccessType=rw\nDefaultValue=0x0\nLowLimit=0x0\nHighLimit=0xFF\n\n[2100sub11]\nParameterName=IO Mask for Channel 129-136\nObjectType=0x7\nDataType=0x0005\nAccessType=rw\nDefaultValue=0x0\nLowLimit=0x0\nHighLimit=0xFF\n\n[2100sub12]\nParameterName=IO Mask for Channel 137-144\nObjectType=0x7\nDataType=0x0005\nAccessType=rw\nDefaultValue=0x0\nLowLimit=0x0\nHighLimit=0xFF\n\n[2100sub13]\nParameterName=IO Mask for Channel 145-152\nObjectType=0x7\nDataType=0x0005\nAccessType=rw\nDefaultValue=0x0\nLowLimit=0x0\nHighLimit=0xFF\n\n[2100sub14]\nParameterName=IO Mask for Channel 153-160\nObjectType=0x7\nDataType=0x0005\nAccessType=rw\nDefaultValue=0x0\nLowLimit=0x0\nHighLimit=0xFF\n\n[2200]\nParameterName=Object 2200 - Digital Input Filter\nObjectType=0x8\nSubNumber=21\n\n[2200sub0]\nParameterName=Number of Elements\nObjectType=0x7\nDataType=0x0005\nAccessType=ro\nDefaultValue=0x14\nLowLimit=0x00\nHighLimit=0xFE\n\n[2200sub1]\nParameterName=Digital Input Filter for Channel 1-8\nObjectType=0x7\nDataType=0x0005\nAccessType=rw\nDefaultValue=0\nLowLimit=0x0\nHighLimit=0xFF\n\n[2200sub2]\nParameterName=Digital Input Filter for Channel 9-16\nObjectType=0x7\nDataType=0x0005\nAccessType=rw\nDefaultValue=0\nLowLimit=0x0\nHighLimit=0xFF\n\n[2200sub3]\nParameterName=Digital Input Filter for Channel 17-24\nObjectType=0x7\nDataType=0x0005\nAccessType=rw\nDefaultValue=0\nLowLimit=0x0\nHighLimit=0xFF\n\n[2200sub4]\nParameterName=Digital Input Filter for Channel 25-32\nObjectType=0x7\nDataType=0x0005\nAccessType=rw\nDefaultValue=0\nLowLimit=0x0\nHighLimit=0xFF\n\n[2200sub5]\nParameterName=Digital Input Filter for Channel 33-40\nObjectType=0x7\nDataType=0x0005\nAccessType=rw\nDefaultValue=0\nLowLimit=0x0\nHighLimit=0xFF\n\n[2200sub6]\nParameterName=Digital Input Filter for Channel 41-48\nObjectType=0x7\nDataType=0x0005\nAccessType=rw\nDefaultValue=0\nLowLimit=0x0\nHighLimit=0xFF\n\n[2200sub7]\nParameterName=Digital Input Filter for Channel 49-56\nObjectType=0x7\nDataType=0x0005\nAccessType=rw\nDefaultValue=0\nLowLimit=0x0\nHighLimit=0xFF\n\n[2200sub8]\nParameterName=Digital Input Filter for Channel 57-64\nObjectType=0x7\nDataType=0x0005\nAccessType=rw\nDefaultValue=0\nLowLimit=0x0\nHighLimit=0xFF\n\n[2200sub9]\nParameterName=Digital Input Filter for Channel 65-72\nObjectType=0x7\nDataType=0x0005\nAccessType=rw\nDefaultValue=0\nLowLimit=0x0\nHighLimit=0xFF\n\n[2200subA]\nParameterName=Digital Input Filter for Channel 73-80\nObjectType=0x7\nDataType=0x0005\nAccessType=rw\nDefaultValue=0\nLowLimit=0x0\nHighLimit=0xFF\n\n[2200subB]\nParameterName=Digital Input Filter for Channel 81-88\nObjectType=0x7\nDataType=0x0005\nAccessType=rw\nDefaultValue=0\nLowLimit=0x0\nHighLimit=0xFF\n\n[2200subC]\nParameterName=Digital Input Filter for Channel 89-96\nObjectType=0x7\nDataType=0x0005\nAccessType=rw\nDefaultValue=0\nLowLimit=0x0\nHighLimit=0xFF\n\n[2200subD]\nParameterName=Digital Input Filter for Channel 97-104\nObjectType=0x7\nDataType=0x0005\nAccessType=rw\nDefaultValue=0\nLowLimit=0x0\nHighLimit=0xFF\n\n[2200subE]\nParameterName=Digital Input Filter for Channel 105-112\nObjectType=0x7\nDataType=0x0005\nAccessType=rw\nDefaultValue=0\nLowLimit=0x0\nHighLimit=0xFF\n\n[2200subF]\nParameterName=Digital Input Filter for Channel 113-120\nObjectType=0x7\nDataType=0x0005\nAccessType=rw\nDefaultValue=0\nLowLimit=0x0\nHighLimit=0xFF\n\n[2200sub10]\nParameterName=Digital Input Filter for Channel 121-128\nObjectType=0x7\nDataType=0x0005\nAccessType=rw\nDefaultValue=0\nLowLimit=0x0\nHighLimit=0xFF\n\n[2200sub11]\nParameterName=Digital Input Filter for Channel 129-136\nObjectType=0x7\nDataType=0x0005\nAccessType=rw\nDefaultValue=0\nLowLimit=0x0\nHighLimit=0xFF\n\n[2200sub12]\nParameterName=Digital Input Filter for Channel 137-144\nObjectType=0x7\nDataType=0x0005\nAccessType=rw\nDefaultValue=0\nLowLimit=0x0\nHighLimit=0xFF\n\n[2200sub13]\nParameterName=Digital Input Filter for Channel 145-152\nObjectType=0x7\nDataType=0x0005\nAccessType=rw\nDefaultValue=0\nLowLimit=0x0\nHighLimit=0xFF\n\n[2200sub14]\nParameterName=Digital Input Filter for Channel 153-160\nObjectType=0x7\nDataType=0x0005\nAccessType=rw\nDefaultValue=0\nLowLimit=0x0\nHighLimit=0xFF\n\n[3000]\nParameterName=X2X_Config_REC\nObjectType=0x9\nSubNumber=11\n\n[3000sub0]\nParameterName=Number of Entries\nObjectType=0x7\nDataType=0x0005\nAccessType=ro\nDefaultValue=0x11\n\n[3000sub1]\nParameterName=X2X_CycleMode_U8\nObjectType=0x7\nDataType=0x0005\nAccessType=rw\n\n[3000sub2]\nParameterName=X2X_CycleSet_U8\nObjectType=0x7\nDataType=0x0005\nAccessType=rw\n\n[3000subA]\nParameterName=X2X_StartupDelayUs_U32\nObjectType=0x7\nDataType=0x0007\nAccessType=rw\n\n[3000subB]\nParameterName=X2X_CfgModeUploadDisable_BOOL\nObjectType=0x7\nDataType=0x0001\nAccessType=rw\n\n[3000subC]\nParameterName=X2X_ResponseMinUs_U16\nObjectType=0x7\nDataType=0x0006\nAccessType=rw\n\n[3000subD]\nParameterName=X2X_ResponseMaxUs_U16\nObjectType=0x7\nDataType=0x0006\nAccessType=rw\n\n[3000subE]\nParameterName=X2X_ResponseAverageUs_U16\nObjectType=0x7\nDataType=0x0006\nAccessType=rw\n\n[3000subF]\nParameterName=X2X_Map_EPL_Only_BOOL\nObjectType=0x7\nDataType=0x0001\nAccessType=rw\nDefaultValue=0\nLowLimit=0\nHighLimit=1\n\n[3000sub10]\nParameterName=Unhide_Manufacturer_Objects_BOOL\nObjectType=0x7\nDataType=0x0001\nAccessType=rw\nDefaultValue=1\nLowLimit=0\nHighLimit=1\n\n[3000sub11]\nParameterName=Autostore_Current_Config_BOOL\nObjectType=0x7\nDataType=0x0001\nAccessType=rw\nDefaultValue=0\nLowLimit=0\nHighLimit=1\n\n[3001]\nParameterName=X2X_OutputConfig_REC\nObjectType=0x9\nSubNumber=4\n\n[3001sub0]\nParameterName=Number of Entries\nObjectType=0x7\nDataType=0x0005\nAccessType=ro\nDefaultValue=0x0a\n\n[3001sub3]\nParameterName=X2X_OutputForceTimeUs_U32\nObjectType=0x7\nDataType=0x0007\nAccessType=rw\n\n[3001sub4]\nParameterName=X2X_ModuleErrorReaction_U8\nObjectType=0x7\nDataType=0x0005\nAccessType=rw\n\n[3001subA]\nParameterName=X2X_ClearModuleError_U8\nObjectType=0x7\nDataType=0x0005\nAccessType=wo\n\n[3011]\nParameterName=DIA_StatisticCount_REC\nObjectType=0x9\nSubNumber=26\n\n[3011sub0]\nParameterName=Number of Entries\nObjectType=0x7\nDataType=0x0005\nAccessType=ro\nDefaultValue=0x33\n\n[3011sub1]\nParameterName=DIA_Total_U32\nObjectType=0x7\nDataType=0x0007\nAccessType=rw\n\n[3011sub2]\nParameterName=DIA_CanArbitrationLost_U8\nObjectType=0x7\nDataType=0x0005\nAccessType=ro\n\n[3011sub3]\nParameterName=DIA_CanErrorCode_U8\nObjectType=0x7\nDataType=0x0005\nAccessType=ro\n\n[3011sub4]\nParameterName=DIA_CanErrorWarningLimit_U8\nObjectType=0x7\nDataType=0x0005\nAccessType=ro\n\n[3011sub5]\nParameterName=DIA_CanRxErr_U8\nObjectType=0x7\nDataType=0x0005\nAccessType=ro\n\n[3011sub6]\nParameterName=DIA_CanTxErr_U8\nObjectType=0x7\nDataType=0x0005\nAccessType=ro\n\n[3011sub10]\nParameterName=DIA_XlkCycleCount_U32\nObjectType=0x7\nDataType=0x0007\nAccessType=rw\n\n[3011sub11]\nParameterName=DIA_XlkBreakCount_U32\nObjectType=0x7\nDataType=0x0007\nAccessType=rw\n\n[3011sub12]\nParameterName=DIA_XlkSyncErrorCount_U32\nObjectType=0x7\nDataType=0x0007\nAccessType=rw\n\n[3011sub13]\nParameterName=DIA_XlkSyncBusyErrorCount_U32\nObjectType=0x7\nDataType=0x0007\nAccessType=rw\n\n[3011sub14]\nParameterName=DIA_XlkSyncNoRxErrorCount_U32\nObjectType=0x7\nDataType=0x0007\nAccessType=rw\n\n[3011sub15]\nParameterName=DIA_XlkSyncFormatErrorCount_U32\nObjectType=0x7\nDataType=0x0007\nAccessType=rw\n\n[3011sub16]\nParameterName=DIA_XlkSyncPendingErrorCount_U32\nObjectType=0x7\nDataType=0x0007\nAccessType=rw\n\n[3011sub17]\nParameterName=DIA_XlkAsynErrorCount_U32\nObjectType=0x7\nDataType=0x0007\nAccessType=rw\n\n[3011sub18]\nParameterName=DIA_XlkAsynBusyErrorCount_U32\nObjectType=0x7\nDataType=0x0007\nAccessType=rw\n\n[3011sub19]\nParameterName=DIA_XlkAsynNoRxErrorCount_U32\nObjectType=0x7\nDataType=0x0007\nAccessType=rw\n\n[3011sub1A]\nParameterName=DIA_XlkAsynFormatErrorCount_U32\nObjectType=0x7\nDataType=0x0007\nAccessType=rw\n\n[3011sub1B]\nParameterName=DIA_XlkAsynPendingErrorCount_U32\nObjectType=0x7\nDataType=0x0007\nAccessType=rw\n\n[3011sub1C]\nParameterName=DIA_XlkModuleLostWhileOperational_U32\nObjectType=0x7\nDataType=0x0007\nAccessType=rw\n\n[3011sub1D]\nParameterName=DIA_XlkModuleNewWhileOperational_U32\nObjectType=0x7\nDataType=0x0007\nAccessType=rw\n\n[3011sub20]\nParameterName=DIA_RamAccessViolation_U32\nObjectType=0x7\nDataType=0x0007\nAccessType=rw\n\n[3011sub30]\nParameterName=DIA_LastParamErrIdx_U16\nObjectType=0x7\nDataType=0x0006\nAccessType=ro\n\n[3011sub31]\nParameterName=DIA_LastParamErrSidx_U8\nObjectType=0x7\nDataType=0x0005\nAccessType=ro\n\n[3011sub32]\nParameterName=DIA_LastParamErrAbortCode_U32\nObjectType=0x7\nDataType=0x0007\nAccessType=ro\n\n[3011sub33]\nParameterName=DIA_LastParamErrRemEntries_U32\nObjectType=0x7\nDataType=0x0007\nAccessType=ro\n\n[30A1]\nParameterName=MOD_SlotCount_U8\nObjectType=0x7\nDataType=0x0005\nAccessType=ro\nPDOMapping=0\n\n[30B2]\nParameterName=MOD_NetworkStatusOk_AU32\nObjectType=0x8\nSubNumber=9\n\n[30B2sub0]\nParameterName=Number of Entries\nObjectType=0x7\nDataType=0x0005\nAccessType=ro\nDefaultValue=0x08\nLowLimit=0x0\nHighLimit=0xFF\n\n[30B2sub1]\nParameterName=MOD_NetworkStatusOk_AU32[n]\nObjectType=0x7\nDataType=0x0007\nAccessType=ro\n\n[30B2sub2]\nParameterName=MOD_NetworkStatusOk_AU32[n]\nObjectType=0x7\nDataType=0x0007\nAccessType=ro\n\n[30B2sub3]\nParameterName=MOD_NetworkStatusOk_AU32[n]\nObjectType=0x7\nDataType=0x0007\nAccessType=ro\n\n[30B2sub4]\nParameterName=MOD_NetworkStatusOk_AU32[n]\nObjectType=0x7\nDataType=0x0007\nAccessType=ro\n\n[30B2sub5]\nParameterName=MOD_NetworkStatusOk_AU32[n]\nObjectType=0x7\nDataType=0x0007\nAccessType=ro\n\n[30B2sub6]\nParameterName=MOD_NetworkStatusOk_AU32[n]\nObjectType=0x7\nDataType=0x0007\nAccessType=ro\n\n[30B2sub7]\nParameterName=MOD_NetworkStatusOk_AU32[n]\nObjectType=0x7\nDataType=0x0007\nAccessType=ro\n\n[30B2sub8]\nParameterName=MOD_NetworkStatusOk_AU32[n]\nObjectType=0x7\nDataType=0x0007\nAccessType=ro\n\n[3100]\nParameterName=MOD_Config_xxh_REC\nObjectType=0x9\nSubNumber=36\n\n[3100sub0]\nParameterName=Number of Entries\nObjectType=0x7\nDataType=0x0005\nAccessType=ro\nDefaultValue=0x68\nLowLimit=0x0\nHighLimit=0xFF\n\n[3100sub1]\nParameterName=MOD_ChildCfgIndex_U16\nObjectType=0x7\nDataType=0x0006\nAccessType=rw\n\n[3100sub2]\nParameterName=MOD_ChildCfgCount_U8\nObjectType=0x7\nDataType=0x0005\nAccessType=rw\n\n[3100sub3]\nParameterName=MOD_ChildActCount_U8\nObjectType=0x7\nDataType=0x0005\nAccessType=rw\n\n[3100sub4]\nParameterName=MOD_CfgMode_U8\nObjectType=0x7\nDataType=0x0005\nAccessType=rw\n\n[3100sub5]\nParameterName=MOD_RequestedHardwareId_U16\nObjectType=0x7\nDataType=0x0006\nAccessType=rw\n\n[3100sub6]\nParameterName=MOD_RequestedVendorId_U16\nObjectType=0x7\nDataType=0x0006\nAccessType=rw\n\n[3100sub7]\nParameterName=MOD_HardwareId_U16\nObjectType=0x7\nDataType=0x0006\nAccessType=ro\n\n[3100sub8]\nParameterName=MOD_VendorId_U16\nObjectType=0x7\nDataType=0x0006\nAccessType=ro\n\n[3100sub9]\nParameterName=MOD_InterfaceFlags_U8\nObjectType=0x7\nDataType=0x0005\nAccessType=ro\n\n[3100subA]\nParameterName=MOD_Status_U16\nObjectType=0x7\nDataType=0x0006\nAccessType=rw\n\n[3100subB]\nParameterName=MOD_NetworkStatus_U8\nObjectType=0x7\nDataType=0x0005\nAccessType=ro\n\n[3100subC]\nParameterName=MOD_BlockMask_U8\nObjectType=0x7\nDataType=0x0005\nAccessType=ro\n\n[3100subD]\nParameterName=MOD_BootCount_U8\nObjectType=0x7\nDataType=0x0005\nAccessType=rw\n\n[3100subE]\nParameterName=MOD_LastError_U8\nObjectType=0x7\nDataType=0x0005\nAccessType=rw\n\n[3100sub11]\nParameterName=MOD_FirmwareVersion_U16\nObjectType=0x7\nDataType=0x0006\nAccessType=ro\n\n[3100sub12]\nParameterName=MOD_HardwareVariant_U16\nObjectType=0x7\nDataType=0x0006\nAccessType=ro\n\n[3100sub13]\nParameterName=MOD_SerialNo_U32\nObjectType=0x7\nDataType=0x0007\nAccessType=ro\n\n[3100sub14]\nParameterName=MOD_PhysicalSlotNumber_U8\nObjectType=0x7\nDataType=0x0005\nAccessType=ro\n\n[3100sub15]\nParameterName=MOD_NodeSwitch_U8\nObjectType=0x7\nDataType=0x0005\nAccessType=ro\n\n[3100sub16]\nParameterName=MOD_RequestedSerialNo_U32\nObjectType=0x7\nDataType=0x0007\nAccessType=rw\n\n[3100sub17]\nParameterName=MOD_ModuleErrorReaction_U8\nObjectType=0x7\nDataType=0x0005\nAccessType=rw\n\n[3100sub21]\nParameterName=MOD_AsyncRead_U64\nObjectType=0x7\nDataType=0x001b\nAccessType=rw\n\n[3100sub22]\nParameterName=MOD_AsyncWrite_U64\nObjectType=0x7\nDataType=0x001b\nAccessType=wo\n\n[3100sub23]\nParameterName=MOD_Firmware_DOM\nObjectType=0x7\nDataType=0x000f\nAccessType=wo\n\n[3100sub24]\nParameterName=MOD_AsyncReadReg_U32\nObjectType=0x7\nDataType=0x0007\nAccessType=rw\n\n[3100sub25]\nParameterName=MOD_AsyncReadVal_U32\nObjectType=0x7\nDataType=0x0007\nAccessType=ro\n\n[3100sub26]\nParameterName=MOD_AsyncWriteReg_U32\nObjectType=0x7\nDataType=0x0007\nAccessType=rw\n\n[3100sub27]\nParameterName=MOD_AsyncWriteVal_U32\nObjectType=0x7\nDataType=0x0007\nAccessType=wo\n\n[3100sub5A]\nParameterName=MOD_CfgFunctionMode_U8\nObjectType=0x7\nDataType=0x0005\nAccessType=rw\n\n[3100sub5B]\nParameterName=MOD_CfgEntryCount_U8\nObjectType=0x7\nDataType=0x0005\nAccessType=rw\n\n[3100sub64]\nParameterName=MOD_CfgEntry_00_U64\nObjectType=0x7\nDataType=0x001b\nAccessType=rw\n\n[3100sub65]\nParameterName=MOD_CfgEntry_01_U64\nObjectType=0x7\nDataType=0x001b\nAccessType=rw\n\n[3100sub66]\nParameterName=MOD_CfgEntry_02_U64\nObjectType=0x7\nDataType=0x001b\nAccessType=rw\n\n[3100sub67]\nParameterName=MOD_CfgEntry_03_U64\nObjectType=0x7\nDataType=0x001b\nAccessType=rw\n\n[3100sub68]\nParameterName=MOD_CfgEntry_04_U64\nObjectType=0x7\nDataType=0x001b\nAccessType=rw\n\n[3101]\nParameterName=MOD_Config_xxh_REC\nObjectType=0x9\nSubNumber=36\n\n[3101sub0]\nParameterName=Number of Entries\nObjectType=0x7\nDataType=0x0005\nAccessType=ro\nDefaultValue=0x68\nLowLimit=0x0\nHighLimit=0xFF\n\n[3101sub1]\nParameterName=MOD_ChildCfgIndex_U16\nObjectType=0x7\nDataType=0x0006\nAccessType=rw\n\n[3101sub2]\nParameterName=MOD_ChildCfgCount_U8\nObjectType=0x7\nDataType=0x0005\nAccessType=rw\n\n[3101sub3]\nParameterName=MOD_ChildActCount_U8\nObjectType=0x7\nDataType=0x0005\nAccessType=rw\n\n[3101sub4]\nParameterName=MOD_CfgMode_U8\nObjectType=0x7\nDataType=0x0005\nAccessType=rw\n\n[3101sub5]\nParameterName=MOD_RequestedHardwareId_U16\nObjectType=0x7\nDataType=0x0006\nAccessType=rw\n\n[3101sub6]\nParameterName=MOD_RequestedVendorId_U16\nObjectType=0x7\nDataType=0x0006\nAccessType=rw\n\n[3101sub7]\nParameterName=MOD_HardwareId_U16\nObjectType=0x7\nDataType=0x0006\nAccessType=ro\n\n[3101sub8]\nParameterName=MOD_VendorId_U16\nObjectType=0x7\nDataType=0x0006\nAccessType=ro\n\n[3101sub9]\nParameterName=MOD_InterfaceFlags_U8\nObjectType=0x7\nDataType=0x0005\nAccessType=ro\n\n[3101subA]\nParameterName=MOD_Status_U16\nObjectType=0x7\nDataType=0x0006\nAccessType=rw\n\n[3101subB]\nParameterName=MOD_NetworkStatus_U8\nObjectType=0x7\nDataType=0x0005\nAccessType=ro\n\n[3101subC]\nParameterName=MOD_BlockMask_U8\nObjectType=0x7\nDataType=0x0005\nAccessType=ro\n\n[3101subD]\nParameterName=MOD_BootCount_U8\nObjectType=0x7\nDataType=0x0005\nAccessType=rw\n\n[3101subE]\nParameterName=MOD_LastError_U8\nObjectType=0x7\nDataType=0x0005\nAccessType=rw\n\n[3101sub11]\nParameterName=MOD_FirmwareVersion_U16\nObjectType=0x7\nDataType=0x0006\nAccessType=ro\n\n[3101sub12]\nParameterName=MOD_HardwareVariant_U16\nObjectType=0x7\nDataType=0x0006\nAccessType=ro\n\n[3101sub13]\nParameterName=MOD_SerialNo_U32\nObjectType=0x7\nDataType=0x0007\nAccessType=ro\n\n[3101sub14]\nParameterName=MOD_PhysicalSlotNumber_U8\nObjectType=0x7\nDataType=0x0005\nAccessType=ro\n\n[3101sub15]\nParameterName=MOD_NodeSwitch_U8\nObjectType=0x7\nDataType=0x0005\nAccessType=ro\n\n[3101sub16]\nParameterName=MOD_RequestedSerialNo_U32\nObjectType=0x7\nDataType=0x0007\nAccessType=rw\n\n[3101sub17]\nParameterName=MOD_ModuleErrorReaction_U8\nObjectType=0x7\nDataType=0x0005\nAccessType=rw\n\n[3101sub21]\nParameterName=MOD_AsyncRead_U64\nObjectType=0x7\nDataType=0x001b\nAccessType=rw\n\n[3101sub22]\nParameterName=MOD_AsyncWrite_U64\nObjectType=0x7\nDataType=0x001b\nAccessType=wo\n\n[3101sub23]\nParameterName=MOD_Firmware_DOM\nObjectType=0x7\nDataType=0x000f\nAccessType=wo\n\n[3101sub24]\nParameterName=MOD_AsyncReadReg_U32\nObjectType=0x7\nDataType=0x0007\nAccessType=rw\n\n[3101sub25]\nParameterName=MOD_AsyncReadVal_U32\nObjectType=0x7\nDataType=0x0007\nAccessType=ro\n\n[3101sub26]\nParameterName=MOD_AsyncWriteReg_U32\nObjectType=0x7\nDataType=0x0007\nAccessType=rw\n\n[3101sub27]\nParameterName=MOD_AsyncWriteVal_U32\nObjectType=0x7\nDataType=0x0007\nAccessType=wo\n\n[3101sub5A]\nParameterName=MOD_CfgFunctionMode_U8\nObjectType=0x7\nDataType=0x0005\nAccessType=rw\n\n[3101sub5B]\nParameterName=MOD_CfgEntryCount_U8\nObjectType=0x7\nDataType=0x0005\nAccessType=rw\n\n[3101sub64]\nParameterName=MOD_CfgEntry_00_U64\nObjectType=0x7\nDataType=0x001b\nAccessType=rw\n\n[3101sub65]\nParameterName=MOD_CfgEntry_01_U64\nObjectType=0x7\nDataType=0x001b\nAccessType=rw\n\n[3101sub66]\nParameterName=MOD_CfgEntry_02_U64\nObjectType=0x7\nDataType=0x001b\nAccessType=rw\n\n[3101sub67]\nParameterName=MOD_CfgEntry_03_U64\nObjectType=0x7\nDataType=0x001b\nAccessType=rw\n\n[3101sub68]\nParameterName=MOD_CfgEntry_04_U64\nObjectType=0x7\nDataType=0x001b\nAccessType=rw\n\n[3102]\nParameterName=MOD_Config_xxh_REC\nObjectType=0x9\nSubNumber=36\n\n[3102sub0]\nParameterName=Number of Entries\nObjectType=0x7\nDataType=0x0005\nAccessType=ro\nDefaultValue=0x68\nLowLimit=0x0\nHighLimit=0xFF\n\n[3102sub1]\nParameterName=MOD_ChildCfgIndex_U16\nObjectType=0x7\nDataType=0x0006\nAccessType=rw\n\n[3102sub2]\nParameterName=MOD_ChildCfgCount_U8\nObjectType=0x7\nDataType=0x0005\nAccessType=rw\n\n[3102sub3]\nParameterName=MOD_ChildActCount_U8\nObjectType=0x7\nDataType=0x0005\nAccessType=rw\n\n[3102sub4]\nParameterName=MOD_CfgMode_U8\nObjectType=0x7\nDataType=0x0005\nAccessType=rw\n\n[3102sub5]\nParameterName=MOD_RequestedHardwareId_U16\nObjectType=0x7\nDataType=0x0006\nAccessType=rw\n\n[3102sub6]\nParameterName=MOD_RequestedVendorId_U16\nObjectType=0x7\nDataType=0x0006\nAccessType=rw\n\n[3102sub7]\nParameterName=MOD_HardwareId_U16\nObjectType=0x7\nDataType=0x0006\nAccessType=ro\n\n[3102sub8]\nParameterName=MOD_VendorId_U16\nObjectType=0x7\nDataType=0x0006\nAccessType=ro\n\n[3102sub9]\nParameterName=MOD_InterfaceFlags_U8\nObjectType=0x7\nDataType=0x0005\nAccessType=ro\n\n[3102subA]\nParameterName=MOD_Status_U16\nObjectType=0x7\nDataType=0x0006\nAccessType=rw\n\n[3102subB]\nParameterName=MOD_NetworkStatus_U8\nObjectType=0x7\nDataType=0x0005\nAccessType=ro\n\n[3102subC]\nParameterName=MOD_BlockMask_U8\nObjectType=0x7\nDataType=0x0005\nAccessType=ro\n\n[3102subD]\nParameterName=MOD_BootCount_U8\nObjectType=0x7\nDataType=0x0005\nAccessType=rw\n\n[3102subE]\nParameterName=MOD_LastError_U8\nObjectType=0x7\nDataType=0x0005\nAccessType=rw\n\n[3102sub11]\nParameterName=MOD_FirmwareVersion_U16\nObjectType=0x7\nDataType=0x0006\nAccessType=ro\n\n[3102sub12]\nParameterName=MOD_HardwareVariant_U16\nObjectType=0x7\nDataType=0x0006\nAccessType=ro\n\n[3102sub13]\nParameterName=MOD_SerialNo_U32\nObjectType=0x7\nDataType=0x0007\nAccessType=ro\n\n[3102sub14]\nParameterName=MOD_PhysicalSlotNumber_U8\nObjectType=0x7\nDataType=0x0005\nAccessType=ro\n\n[3102sub15]\nParameterName=MOD_NodeSwitch_U8\nObjectType=0x7\nDataType=0x0005\nAccessType=ro\n\n[3102sub16]\nParameterName=MOD_RequestedSerialNo_U32\nObjectType=0x7\nDataType=0x0007\nAccessType=rw\n\n[3102sub17]\nParameterName=MOD_ModuleErrorReaction_U8\nObjectType=0x7\nDataType=0x0005\nAccessType=rw\n\n[3102sub21]\nParameterName=MOD_AsyncRead_U64\nObjectType=0x7\nDataType=0x001b\nAccessType=rw\n\n[3102sub22]\nParameterName=MOD_AsyncWrite_U64\nObjectType=0x7\nDataType=0x001b\nAccessType=wo\n\n[3102sub23]\nParameterName=MOD_Firmware_DOM\nObjectType=0x7\nDataType=0x000f\nAccessType=wo\n\n[3102sub24]\nParameterName=MOD_AsyncReadReg_U32\nObjectType=0x7\nDataType=0x0007\nAccessType=rw\n\n[3102sub25]\nParameterName=MOD_AsyncReadVal_U32\nObjectType=0x7\nDataType=0x0007\nAccessType=ro\n\n[3102sub26]\nParameterName=MOD_AsyncWriteReg_U32\nObjectType=0x7\nDataType=0x0007\nAccessType=rw\n\n[3102sub27]\nParameterName=MOD_AsyncWriteVal_U32\nObjectType=0x7\nDataType=0x0007\nAccessType=wo\n\n[3102sub5A]\nParameterName=MOD_CfgFunctionMode_U8\nObjectType=0x7\nDataType=0x0005\nAccessType=rw\n\n[3102sub5B]\nParameterName=MOD_CfgEntryCount_U8\nObjectType=0x7\nDataType=0x0005\nAccessType=rw\n\n[3102sub64]\nParameterName=MOD_CfgEntry_00_U64\nObjectType=0x7\nDataType=0x001b\nAccessType=rw\n\n[3102sub65]\nParameterName=MOD_CfgEntry_01_U64\nObjectType=0x7\nDataType=0x001b\nAccessType=rw\n\n[3102sub66]\nParameterName=MOD_CfgEntry_02_U64\nObjectType=0x7\nDataType=0x001b\nAccessType=rw\n\n[3102sub67]\nParameterName=MOD_CfgEntry_03_U64\nObjectType=0x7\nDataType=0x001b\nAccessType=rw\n\n[3102sub68]\nParameterName=MOD_CfgEntry_04_U64\nObjectType=0x7\nDataType=0x001b\nAccessType=rw\n\n[3103]\nParameterName=MOD_Config_xxh_REC\nObjectType=0x9\nSubNumber=36\n\n[3103sub0]\nParameterName=Number of Entries\nObjectType=0x7\nDataType=0x0005\nAccessType=ro\nDefaultValue=0x68\nLowLimit=0x0\nHighLimit=0xFF\n\n[3103sub1]\nParameterName=MOD_ChildCfgIndex_U16\nObjectType=0x7\nDataType=0x0006\nAccessType=rw\n\n[3103sub2]\nParameterName=MOD_ChildCfgCount_U8\nObjectType=0x7\nDataType=0x0005\nAccessType=rw\n\n[3103sub3]\nParameterName=MOD_ChildActCount_U8\nObjectType=0x7\nDataType=0x0005\nAccessType=rw\n\n[3103sub4]\nParameterName=MOD_CfgMode_U8\nObjectType=0x7\nDataType=0x0005\nAccessType=rw\n\n[3103sub5]\nParameterName=MOD_RequestedHardwareId_U16\nObjectType=0x7\nDataType=0x0006\nAccessType=rw\n\n[3103sub6]\nParameterName=MOD_RequestedVendorId_U16\nObjectType=0x7\nDataType=0x0006\nAccessType=rw\n\n[3103sub7]\nParameterName=MOD_HardwareId_U16\nObjectType=0x7\nDataType=0x0006\nAccessType=ro\n\n[3103sub8]\nParameterName=MOD_VendorId_U16\nObjectType=0x7\nDataType=0x0006\nAccessType=ro\n\n[3103sub9]\nParameterName=MOD_InterfaceFlags_U8\nObjectType=0x7\nDataType=0x0005\nAccessType=ro\n\n[3103subA]\nParameterName=MOD_Status_U16\nObjectType=0x7\nDataType=0x0006\nAccessType=rw\n\n[3103subB]\nParameterName=MOD_NetworkStatus_U8\nObjectType=0x7\nDataType=0x0005\nAccessType=ro\n\n[3103subC]\nParameterName=MOD_BlockMask_U8\nObjectType=0x7\nDataType=0x0005\nAccessType=ro\n\n[3103subD]\nParameterName=MOD_BootCount_U8\nObjectType=0x7\nDataType=0x0005\nAccessType=rw\n\n[3103subE]\nParameterName=MOD_LastError_U8\nObjectType=0x7\nDataType=0x0005\nAccessType=rw\n\n[3103sub11]\nParameterName=MOD_FirmwareVersion_U16\nObjectType=0x7\nDataType=0x0006\nAccessType=ro\n\n[3103sub12]\nParameterName=MOD_HardwareVariant_U16\nObjectType=0x7\nDataType=0x0006\nAccessType=ro\n\n[3103sub13]\nParameterName=MOD_SerialNo_U32\nObjectType=0x7\nDataType=0x0007\nAccessType=ro\n\n[3103sub14]\nParameterName=MOD_PhysicalSlotNumber_U8\nObjectType=0x7\nDataType=0x0005\nAccessType=ro\n\n[3103sub15]\nParameterName=MOD_NodeSwitch_U8\nObjectType=0x7\nDataType=0x0005\nAccessType=ro\n\n[3103sub16]\nParameterName=MOD_RequestedSerialNo_U32\nObjectType=0x7\nDataType=0x0007\nAccessType=rw\n\n[3103sub17]\nParameterName=MOD_ModuleErrorReaction_U8\nObjectType=0x7\nDataType=0x0005\nAccessType=rw\n\n[3103sub21]\nParameterName=MOD_AsyncRead_U64\nObjectType=0x7\nDataType=0x001b\nAccessType=rw\n\n[3103sub22]\nParameterName=MOD_AsyncWrite_U64\nObjectType=0x7\nDataType=0x001b\nAccessType=wo\n\n[3103sub23]\nParameterName=MOD_Firmware_DOM\nObjectType=0x7\nDataType=0x000f\nAccessType=wo\n\n[3103sub24]\nParameterName=MOD_AsyncReadReg_U32\nObjectType=0x7\nDataType=0x0007\nAccessType=rw\n\n[3103sub25]\nParameterName=MOD_AsyncReadVal_U32\nObjectType=0x7\nDataType=0x0007\nAccessType=ro\n\n[3103sub26]\nParameterName=MOD_AsyncWriteReg_U32\nObjectType=0x7\nDataType=0x0007\nAccessType=rw\n\n[3103sub27]\nParameterName=MOD_AsyncWriteVal_U32\nObjectType=0x7\nDataType=0x0007\nAccessType=wo\n\n[3103sub5A]\nParameterName=MOD_CfgFunctionMode_U8\nObjectType=0x7\nDataType=0x0005\nAccessType=rw\n\n[3103sub5B]\nParameterName=MOD_CfgEntryCount_U8\nObjectType=0x7\nDataType=0x0005\nAccessType=rw\n\n[3103sub64]\nParameterName=MOD_CfgEntry_00_U64\nObjectType=0x7\nDataType=0x001b\nAccessType=rw\n\n[3103sub65]\nParameterName=MOD_CfgEntry_01_U64\nObjectType=0x7\nDataType=0x001b\nAccessType=rw\n\n[3103sub66]\nParameterName=MOD_CfgEntry_02_U64\nObjectType=0x7\nDataType=0x001b\nAccessType=rw\n\n[3103sub67]\nParameterName=MOD_CfgEntry_03_U64\nObjectType=0x7\nDataType=0x001b\nAccessType=rw\n\n[3103sub68]\nParameterName=MOD_CfgEntry_04_U64\nObjectType=0x7\nDataType=0x001b\nAccessType=rw\n\n[3104]\nParameterName=MOD_Config_xxh_REC\nObjectType=0x9\nSubNumber=36\n\n[3104sub0]\nParameterName=Number of Entries\nObjectType=0x7\nDataType=0x0005\nAccessType=ro\nDefaultValue=0x68\nLowLimit=0x0\nHighLimit=0xFF\n\n[3104sub1]\nParameterName=MOD_ChildCfgIndex_U16\nObjectType=0x7\nDataType=0x0006\nAccessType=rw\n\n[3104sub2]\nParameterName=MOD_ChildCfgCount_U8\nObjectType=0x7\nDataType=0x0005\nAccessType=rw\n\n[3104sub3]\nParameterName=MOD_ChildActCount_U8\nObjectType=0x7\nDataType=0x0005\nAccessType=rw\n\n[3104sub4]\nParameterName=MOD_CfgMode_U8\nObjectType=0x7\nDataType=0x0005\nAccessType=rw\n\n[3104sub5]\nParameterName=MOD_RequestedHardwareId_U16\nObjectType=0x7\nDataType=0x0006\nAccessType=rw\n\n[3104sub6]\nParameterName=MOD_RequestedVendorId_U16\nObjectType=0x7\nDataType=0x0006\nAccessType=rw\n\n[3104sub7]\nParameterName=MOD_HardwareId_U16\nObjectType=0x7\nDataType=0x0006\nAccessType=ro\n\n[3104sub8]\nParameterName=MOD_VendorId_U16\nObjectType=0x7\nDataType=0x0006\nAccessType=ro\n\n[3104sub9]\nParameterName=MOD_InterfaceFlags_U8\nObjectType=0x7\nDataType=0x0005\nAccessType=ro\n\n[3104subA]\nParameterName=MOD_Status_U16\nObjectType=0x7\nDataType=0x0006\nAccessType=rw\n\n[3104subB]\nParameterName=MOD_NetworkStatus_U8\nObjectType=0x7\nDataType=0x0005\nAccessType=ro\n\n[3104subC]\nParameterName=MOD_BlockMask_U8\nObjectType=0x7\nDataType=0x0005\nAccessType=ro\n\n[3104subD]\nParameterName=MOD_BootCount_U8\nObjectType=0x7\nDataType=0x0005\nAccessType=rw\n\n[3104subE]\nParameterName=MOD_LastError_U8\nObjectType=0x7\nDataType=0x0005\nAccessType=rw\n\n[3104sub11]\nParameterName=MOD_FirmwareVersion_U16\nObjectType=0x7\nDataType=0x0006\nAccessType=ro\n\n[3104sub12]\nParameterName=MOD_HardwareVariant_U16\nObjectType=0x7\nDataType=0x0006\nAccessType=ro\n\n[3104sub13]\nParameterName=MOD_SerialNo_U32\nObjectType=0x7\nDataType=0x0007\nAccessType=ro\n\n[3104sub14]\nParameterName=MOD_PhysicalSlotNumber_U8\nObjectType=0x7\nDataType=0x0005\nAccessType=ro\n\n[3104sub15]\nParameterName=MOD_NodeSwitch_U8\nObjectType=0x7\nDataType=0x0005\nAccessType=ro\n\n[3104sub16]\nParameterName=MOD_RequestedSerialNo_U32\nObjectType=0x7\nDataType=0x0007\nAccessType=rw\n\n[3104sub17]\nParameterName=MOD_ModuleErrorReaction_U8\nObjectType=0x7\nDataType=0x0005\nAccessType=rw\n\n[3104sub21]\nParameterName=MOD_AsyncRead_U64\nObjectType=0x7\nDataType=0x001b\nAccessType=rw\n\n[3104sub22]\nParameterName=MOD_AsyncWrite_U64\nObjectType=0x7\nDataType=0x001b\nAccessType=wo\n\n[3104sub23]\nParameterName=MOD_Firmware_DOM\nObjectType=0x7\nDataType=0x000f\nAccessType=wo\n\n[3104sub24]\nParameterName=MOD_AsyncReadReg_U32\nObjectType=0x7\nDataType=0x0007\nAccessType=rw\n\n[3104sub25]\nParameterName=MOD_AsyncReadVal_U32\nObjectType=0x7\nDataType=0x0007\nAccessType=ro\n\n[3104sub26]\nParameterName=MOD_AsyncWriteReg_U32\nObjectType=0x7\nDataType=0x0007\nAccessType=rw\n\n[3104sub27]\nParameterName=MOD_AsyncWriteVal_U32\nObjectType=0x7\nDataType=0x0007\nAccessType=wo\n\n[3104sub5A]\nParameterName=MOD_CfgFunctionMode_U8\nObjectType=0x7\nDataType=0x0005\nAccessType=rw\n\n[3104sub5B]\nParameterName=MOD_CfgEntryCount_U8\nObjectType=0x7\nDataType=0x0005\nAccessType=rw\n\n[3104sub64]\nParameterName=MOD_CfgEntry_00_U64\nObjectType=0x7\nDataType=0x001b\nAccessType=rw\n\n[3104sub65]\nParameterName=MOD_CfgEntry_01_U64\nObjectType=0x7\nDataType=0x001b\nAccessType=rw\n\n[3104sub66]\nParameterName=MOD_CfgEntry_02_U64\nObjectType=0x7\nDataType=0x001b\nAccessType=rw\n\n[3104sub67]\nParameterName=MOD_CfgEntry_03_U64\nObjectType=0x7\nDataType=0x001b\nAccessType=rw\n\n[3104sub68]\nParameterName=MOD_CfgEntry_04_U64\nObjectType=0x7\nDataType=0x001b\nAccessType=rw\n\n[3105]\nParameterName=MOD_Config_xxh_REC\nObjectType=0x9\nSubNumber=36\n\n[3105sub0]\nParameterName=Number of Entries\nObjectType=0x7\nDataType=0x0005\nAccessType=ro\nDefaultValue=0x68\nLowLimit=0x0\nHighLimit=0xFF\n\n[3105sub1]\nParameterName=MOD_ChildCfgIndex_U16\nObjectType=0x7\nDataType=0x0006\nAccessType=rw\n\n[3105sub2]\nParameterName=MOD_ChildCfgCount_U8\nObjectType=0x7\nDataType=0x0005\nAccessType=rw\n\n[3105sub3]\nParameterName=MOD_ChildActCount_U8\nObjectType=0x7\nDataType=0x0005\nAccessType=rw\n\n[3105sub4]\nParameterName=MOD_CfgMode_U8\nObjectType=0x7\nDataType=0x0005\nAccessType=rw\n\n[3105sub5]\nParameterName=MOD_RequestedHardwareId_U16\nObjectType=0x7\nDataType=0x0006\nAccessType=rw\n\n[3105sub6]\nParameterName=MOD_RequestedVendorId_U16\nObjectType=0x7\nDataType=0x0006\nAccessType=rw\n\n[3105sub7]\nParameterName=MOD_HardwareId_U16\nObjectType=0x7\nDataType=0x0006\nAccessType=ro\n\n[3105sub8]\nParameterName=MOD_VendorId_U16\nObjectType=0x7\nDataType=0x0006\nAccessType=ro\n\n[3105sub9]\nParameterName=MOD_InterfaceFlags_U8\nObjectType=0x7\nDataType=0x0005\nAccessType=ro\n\n[3105subA]\nParameterName=MOD_Status_U16\nObjectType=0x7\nDataType=0x0006\nAccessType=rw\n\n[3105subB]\nParameterName=MOD_NetworkStatus_U8\nObjectType=0x7\nDataType=0x0005\nAccessType=ro\n\n[3105subC]\nParameterName=MOD_BlockMask_U8\nObjectType=0x7\nDataType=0x0005\nAccessType=ro\n\n[3105subD]\nParameterName=MOD_BootCount_U8\nObjectType=0x7\nDataType=0x0005\nAccessType=rw\n\n[3105subE]\nParameterName=MOD_LastError_U8\nObjectType=0x7\nDataType=0x0005\nAccessType=rw\n\n[3105sub11]\nParameterName=MOD_FirmwareVersion_U16\nObjectType=0x7\nDataType=0x0006\nAccessType=ro\n\n[3105sub12]\nParameterName=MOD_HardwareVariant_U16\nObjectType=0x7\nDataType=0x0006\nAccessType=ro\n\n[3105sub13]\nParameterName=MOD_SerialNo_U32\nObjectType=0x7\nDataType=0x0007\nAccessType=ro\n\n[3105sub14]\nParameterName=MOD_PhysicalSlotNumber_U8\nObjectType=0x7\nDataType=0x0005\nAccessType=ro\n\n[3105sub15]\nParameterName=MOD_NodeSwitch_U8\nObjectType=0x7\nDataType=0x0005\nAccessType=ro\n\n[3105sub16]\nParameterName=MOD_RequestedSerialNo_U32\nObjectType=0x7\nDataType=0x0007\nAccessType=rw\n\n[3105sub17]\nParameterName=MOD_ModuleErrorReaction_U8\nObjectType=0x7\nDataType=0x0005\nAccessType=rw\n\n[3105sub21]\nParameterName=MOD_AsyncRead_U64\nObjectType=0x7\nDataType=0x001b\nAccessType=rw\n\n[3105sub22]\nParameterName=MOD_AsyncWrite_U64\nObjectType=0x7\nDataType=0x001b\nAccessType=wo\n\n[3105sub23]\nParameterName=MOD_Firmware_DOM\nObjectType=0x7\nDataType=0x000f\nAccessType=wo\n\n[3105sub24]\nParameterName=MOD_AsyncReadReg_U32\nObjectType=0x7\nDataType=0x0007\nAccessType=rw\n\n[3105sub25]\nParameterName=MOD_AsyncReadVal_U32\nObjectType=0x7\nDataType=0x0007\nAccessType=ro\n\n[3105sub26]\nParameterName=MOD_AsyncWriteReg_U32\nObjectType=0x7\nDataType=0x0007\nAccessType=rw\n\n[3105sub27]\nParameterName=MOD_AsyncWriteVal_U32\nObjectType=0x7\nDataType=0x0007\nAccessType=wo\n\n[3105sub5A]\nParameterName=MOD_CfgFunctionMode_U8\nObjectType=0x7\nDataType=0x0005\nAccessType=rw\n\n[3105sub5B]\nParameterName=MOD_CfgEntryCount_U8\nObjectType=0x7\nDataType=0x0005\nAccessType=rw\n\n[3105sub64]\nParameterName=MOD_CfgEntry_00_U64\nObjectType=0x7\nDataType=0x001b\nAccessType=rw\n\n[3105sub65]\nParameterName=MOD_CfgEntry_01_U64\nObjectType=0x7\nDataType=0x001b\nAccessType=rw\n\n[3105sub66]\nParameterName=MOD_CfgEntry_02_U64\nObjectType=0x7\nDataType=0x001b\nAccessType=rw\n\n[3105sub67]\nParameterName=MOD_CfgEntry_03_U64\nObjectType=0x7\nDataType=0x001b\nAccessType=rw\n\n[3105sub68]\nParameterName=MOD_CfgEntry_04_U64\nObjectType=0x7\nDataType=0x001b\nAccessType=rw\n\n[3106]\nParameterName=MOD_Config_xxh_REC\nObjectType=0x9\nSubNumber=36\n\n[3106sub0]\nParameterName=Number of Entries\nObjectType=0x7\nDataType=0x0005\nAccessType=ro\nDefaultValue=0x68\nLowLimit=0x0\nHighLimit=0xFF\n\n[3106sub1]\nParameterName=MOD_ChildCfgIndex_U16\nObjectType=0x7\nDataType=0x0006\nAccessType=rw\n\n[3106sub2]\nParameterName=MOD_ChildCfgCount_U8\nObjectType=0x7\nDataType=0x0005\nAccessType=rw\n\n[3106sub3]\nParameterName=MOD_ChildActCount_U8\nObjectType=0x7\nDataType=0x0005\nAccessType=rw\n\n[3106sub4]\nParameterName=MOD_CfgMode_U8\nObjectType=0x7\nDataType=0x0005\nAccessType=rw\n\n[3106sub5]\nParameterName=MOD_RequestedHardwareId_U16\nObjectType=0x7\nDataType=0x0006\nAccessType=rw\n\n[3106sub6]\nParameterName=MOD_RequestedVendorId_U16\nObjectType=0x7\nDataType=0x0006\nAccessType=rw\n\n[3106sub7]\nParameterName=MOD_HardwareId_U16\nObjectType=0x7\nDataType=0x0006\nAccessType=ro\n\n[3106sub8]\nParameterName=MOD_VendorId_U16\nObjectType=0x7\nDataType=0x0006\nAccessType=ro\n\n[3106sub9]\nParameterName=MOD_InterfaceFlags_U8\nObjectType=0x7\nDataType=0x0005\nAccessType=ro\n\n[3106subA]\nParameterName=MOD_Status_U16\nObjectType=0x7\nDataType=0x0006\nAccessType=rw\n\n[3106subB]\nParameterName=MOD_NetworkStatus_U8\nObjectType=0x7\nDataType=0x0005\nAccessType=ro\n\n[3106subC]\nParameterName=MOD_BlockMask_U8\nObjectType=0x7\nDataType=0x0005\nAccessType=ro\n\n[3106subD]\nParameterName=MOD_BootCount_U8\nObjectType=0x7\nDataType=0x0005\nAccessType=rw\n\n[3106subE]\nParameterName=MOD_LastError_U8\nObjectType=0x7\nDataType=0x0005\nAccessType=rw\n\n[3106sub11]\nParameterName=MOD_FirmwareVersion_U16\nObjectType=0x7\nDataType=0x0006\nAccessType=ro\n\n[3106sub12]\nParameterName=MOD_HardwareVariant_U16\nObjectType=0x7\nDataType=0x0006\nAccessType=ro\n\n[3106sub13]\nParameterName=MOD_SerialNo_U32\nObjectType=0x7\nDataType=0x0007\nAccessType=ro\n\n[3106sub14]\nParameterName=MOD_PhysicalSlotNumber_U8\nObjectType=0x7\nDataType=0x0005\nAccessType=ro\n\n[3106sub15]\nParameterName=MOD_NodeSwitch_U8\nObjectType=0x7\nDataType=0x0005\nAccessType=ro\n\n[3106sub16]\nParameterName=MOD_RequestedSerialNo_U32\nObjectType=0x7\nDataType=0x0007\nAccessType=rw\n\n[3106sub17]\nParameterName=MOD_ModuleErrorReaction_U8\nObjectType=0x7\nDataType=0x0005\nAccessType=rw\n\n[3106sub21]\nParameterName=MOD_AsyncRead_U64\nObjectType=0x7\nDataType=0x001b\nAccessType=rw\n\n[3106sub22]\nParameterName=MOD_AsyncWrite_U64\nObjectType=0x7\nDataType=0x001b\nAccessType=wo\n\n[3106sub23]\nParameterName=MOD_Firmware_DOM\nObjectType=0x7\nDataType=0x000f\nAccessType=wo\n\n[3106sub24]\nParameterName=MOD_AsyncReadReg_U32\nObjectType=0x7\nDataType=0x0007\nAccessType=rw\n\n[3106sub25]\nParameterName=MOD_AsyncReadVal_U32\nObjectType=0x7\nDataType=0x0007\nAccessType=ro\n\n[3106sub26]\nParameterName=MOD_AsyncWriteReg_U32\nObjectType=0x7\nDataType=0x0007\nAccessType=rw\n\n[3106sub27]\nParameterName=MOD_AsyncWriteVal_U32\nObjectType=0x7\nDataType=0x0007\nAccessType=wo\n\n[3106sub5A]\nParameterName=MOD_CfgFunctionMode_U8\nObjectType=0x7\nDataType=0x0005\nAccessType=rw\n\n[3106sub5B]\nParameterName=MOD_CfgEntryCount_U8\nObjectType=0x7\nDataType=0x0005\nAccessType=rw\n\n[3106sub64]\nParameterName=MOD_CfgEntry_00_U64\nObjectType=0x7\nDataType=0x001b\nAccessType=rw\n\n[3106sub65]\nParameterName=MOD_CfgEntry_01_U64\nObjectType=0x7\nDataType=0x001b\nAccessType=rw\n\n[3106sub66]\nParameterName=MOD_CfgEntry_02_U64\nObjectType=0x7\nDataType=0x001b\nAccessType=rw\n\n[3106sub67]\nParameterName=MOD_CfgEntry_03_U64\nObjectType=0x7\nDataType=0x001b\nAccessType=rw\n\n[3106sub68]\nParameterName=MOD_CfgEntry_04_U64\nObjectType=0x7\nDataType=0x001b\nAccessType=rw\n\n[3107]\nParameterName=MOD_Config_xxh_REC\nObjectType=0x9\nSubNumber=36\n\n[3107sub0]\nParameterName=Number of Entries\nObjectType=0x7\nDataType=0x0005\nAccessType=ro\nDefaultValue=0x68\nLowLimit=0x0\nHighLimit=0xFF\n\n[3107sub1]\nParameterName=MOD_ChildCfgIndex_U16\nObjectType=0x7\nDataType=0x0006\nAccessType=rw\n\n[3107sub2]\nParameterName=MOD_ChildCfgCount_U8\nObjectType=0x7\nDataType=0x0005\nAccessType=rw\n\n[3107sub3]\nParameterName=MOD_ChildActCount_U8\nObjectType=0x7\nDataType=0x0005\nAccessType=rw\n\n[3107sub4]\nParameterName=MOD_CfgMode_U8\nObjectType=0x7\nDataType=0x0005\nAccessType=rw\n\n[3107sub5]\nParameterName=MOD_RequestedHardwareId_U16\nObjectType=0x7\nDataType=0x0006\nAccessType=rw\n\n[3107sub6]\nParameterName=MOD_RequestedVendorId_U16\nObjectType=0x7\nDataType=0x0006\nAccessType=rw\n\n[3107sub7]\nParameterName=MOD_HardwareId_U16\nObjectType=0x7\nDataType=0x0006\nAccessType=ro\n\n[3107sub8]\nParameterName=MOD_VendorId_U16\nObjectType=0x7\nDataType=0x0006\nAccessType=ro\n\n[3107sub9]\nParameterName=MOD_InterfaceFlags_U8\nObjectType=0x7\nDataType=0x0005\nAccessType=ro\n\n[3107subA]\nParameterName=MOD_Status_U16\nObjectType=0x7\nDataType=0x0006\nAccessType=rw\n\n[3107subB]\nParameterName=MOD_NetworkStatus_U8\nObjectType=0x7\nDataType=0x0005\nAccessType=ro\n\n[3107subC]\nParameterName=MOD_BlockMask_U8\nObjectType=0x7\nDataType=0x0005\nAccessType=ro\n\n[3107subD]\nParameterName=MOD_BootCount_U8\nObjectType=0x7\nDataType=0x0005\nAccessType=rw\n\n[3107subE]\nParameterName=MOD_LastError_U8\nObjectType=0x7\nDataType=0x0005\nAccessType=rw\n\n[3107sub11]\nParameterName=MOD_FirmwareVersion_U16\nObjectType=0x7\nDataType=0x0006\nAccessType=ro\n\n[3107sub12]\nParameterName=MOD_HardwareVariant_U16\nObjectType=0x7\nDataType=0x0006\nAccessType=ro\n\n[3107sub13]\nParameterName=MOD_SerialNo_U32\nObjectType=0x7\nDataType=0x0007\nAccessType=ro\n\n[3107sub14]\nParameterName=MOD_PhysicalSlotNumber_U8\nObjectType=0x7\nDataType=0x0005\nAccessType=ro\n\n[3107sub15]\nParameterName=MOD_NodeSwitch_U8\nObjectType=0x7\nDataType=0x0005\nAccessType=ro\n\n[3107sub16]\nParameterName=MOD_RequestedSerialNo_U32\nObjectType=0x7\nDataType=0x0007\nAccessType=rw\n\n[3107sub17]\nParameterName=MOD_ModuleErrorReaction_U8\nObjectType=0x7\nDataType=0x0005\nAccessType=rw\n\n[3107sub21]\nParameterName=MOD_AsyncRead_U64\nObjectType=0x7\nDataType=0x001b\nAccessType=rw\n\n[3107sub22]\nParameterName=MOD_AsyncWrite_U64\nObjectType=0x7\nDataType=0x001b\nAccessType=wo\n\n[3107sub23]\nParameterName=MOD_Firmware_DOM\nObjectType=0x7\nDataType=0x000f\nAccessType=wo\n\n[3107sub24]\nParameterName=MOD_AsyncReadReg_U32\nObjectType=0x7\nDataType=0x0007\nAccessType=rw\n\n[3107sub25]\nParameterName=MOD_AsyncReadVal_U32\nObjectType=0x7\nDataType=0x0007\nAccessType=ro\n\n[3107sub26]\nParameterName=MOD_AsyncWriteReg_U32\nObjectType=0x7\nDataType=0x0007\nAccessType=rw\n\n[3107sub27]\nParameterName=MOD_AsyncWriteVal_U32\nObjectType=0x7\nDataType=0x0007\nAccessType=wo\n\n[3107sub5A]\nParameterName=MOD_CfgFunctionMode_U8\nObjectType=0x7\nDataType=0x0005\nAccessType=rw\n\n[3107sub5B]\nParameterName=MOD_CfgEntryCount_U8\nObjectType=0x7\nDataType=0x0005\nAccessType=rw\n\n[3107sub64]\nParameterName=MOD_CfgEntry_00_U64\nObjectType=0x7\nDataType=0x001b\nAccessType=rw\n\n[3107sub65]\nParameterName=MOD_CfgEntry_01_U64\nObjectType=0x7\nDataType=0x001b\nAccessType=rw\n\n[3107sub66]\nParameterName=MOD_CfgEntry_02_U64\nObjectType=0x7\nDataType=0x001b\nAccessType=rw\n\n[3107sub67]\nParameterName=MOD_CfgEntry_03_U64\nObjectType=0x7\nDataType=0x001b\nAccessType=rw\n\n[3107sub68]\nParameterName=MOD_CfgEntry_04_U64\nObjectType=0x7\nDataType=0x001b\nAccessType=rw\n\n[3108]\nParameterName=MOD_Config_xxh_REC\nObjectType=0x9\nSubNumber=36\n\n[3108sub0]\nParameterName=Number of Entries\nObjectType=0x7\nDataType=0x0005\nAccessType=ro\nDefaultValue=0x68\nLowLimit=0x0\nHighLimit=0xFF\n\n[3108sub1]\nParameterName=MOD_ChildCfgIndex_U16\nObjectType=0x7\nDataType=0x0006\nAccessType=rw\n\n[3108sub2]\nParameterName=MOD_ChildCfgCount_U8\nObjectType=0x7\nDataType=0x0005\nAccessType=rw\n\n[3108sub3]\nParameterName=MOD_ChildActCount_U8\nObjectType=0x7\nDataType=0x0005\nAccessType=rw\n\n[3108sub4]\nParameterName=MOD_CfgMode_U8\nObjectType=0x7\nDataType=0x0005\nAccessType=rw\n\n[3108sub5]\nParameterName=MOD_RequestedHardwareId_U16\nObjectType=0x7\nDataType=0x0006\nAccessType=rw\n\n[3108sub6]\nParameterName=MOD_RequestedVendorId_U16\nObjectType=0x7\nDataType=0x0006\nAccessType=rw\n\n[3108sub7]\nParameterName=MOD_HardwareId_U16\nObjectType=0x7\nDataType=0x0006\nAccessType=ro\n\n[3108sub8]\nParameterName=MOD_VendorId_U16\nObjectType=0x7\nDataType=0x0006\nAccessType=ro\n\n[3108sub9]\nParameterName=MOD_InterfaceFlags_U8\nObjectType=0x7\nDataType=0x0005\nAccessType=ro\n\n[3108subA]\nParameterName=MOD_Status_U16\nObjectType=0x7\nDataType=0x0006\nAccessType=rw\n\n[3108subB]\nParameterName=MOD_NetworkStatus_U8\nObjectType=0x7\nDataType=0x0005\nAccessType=ro\n\n[3108subC]\nParameterName=MOD_BlockMask_U8\nObjectType=0x7\nDataType=0x0005\nAccessType=ro\n\n[3108subD]\nParameterName=MOD_BootCount_U8\nObjectType=0x7\nDataType=0x0005\nAccessType=rw\n\n[3108subE]\nParameterName=MOD_LastError_U8\nObjectType=0x7\nDataType=0x0005\nAccessType=rw\n\n[3108sub11]\nParameterName=MOD_FirmwareVersion_U16\nObjectType=0x7\nDataType=0x0006\nAccessType=ro\n\n[3108sub12]\nParameterName=MOD_HardwareVariant_U16\nObjectType=0x7\nDataType=0x0006\nAccessType=ro\n\n[3108sub13]\nParameterName=MOD_SerialNo_U32\nObjectType=0x7\nDataType=0x0007\nAccessType=ro\n\n[3108sub14]\nParameterName=MOD_PhysicalSlotNumber_U8\nObjectType=0x7\nDataType=0x0005\nAccessType=ro\n\n[3108sub15]\nParameterName=MOD_NodeSwitch_U8\nObjectType=0x7\nDataType=0x0005\nAccessType=ro\n\n[3108sub16]\nParameterName=MOD_RequestedSerialNo_U32\nObjectType=0x7\nDataType=0x0007\nAccessType=rw\n\n[3108sub17]\nParameterName=MOD_ModuleErrorReaction_U8\nObjectType=0x7\nDataType=0x0005\nAccessType=rw\n\n[3108sub21]\nParameterName=MOD_AsyncRead_U64\nObjectType=0x7\nDataType=0x001b\nAccessType=rw\n\n[3108sub22]\nParameterName=MOD_AsyncWrite_U64\nObjectType=0x7\nDataType=0x001b\nAccessType=wo\n\n[3108sub23]\nParameterName=MOD_Firmware_DOM\nObjectType=0x7\nDataType=0x000f\nAccessType=wo\n\n[3108sub24]\nParameterName=MOD_AsyncReadReg_U32\nObjectType=0x7\nDataType=0x0007\nAccessType=rw\n\n[3108sub25]\nParameterName=MOD_AsyncReadVal_U32\nObjectType=0x7\nDataType=0x0007\nAccessType=ro\n\n[3108sub26]\nParameterName=MOD_AsyncWriteReg_U32\nObjectType=0x7\nDataType=0x0007\nAccessType=rw\n\n[3108sub27]\nParameterName=MOD_AsyncWriteVal_U32\nObjectType=0x7\nDataType=0x0007\nAccessType=wo\n\n[3108sub5A]\nParameterName=MOD_CfgFunctionMode_U8\nObjectType=0x7\nDataType=0x0005\nAccessType=rw\n\n[3108sub5B]\nParameterName=MOD_CfgEntryCount_U8\nObjectType=0x7\nDataType=0x0005\nAccessType=rw\n\n[3108sub64]\nParameterName=MOD_CfgEntry_00_U64\nObjectType=0x7\nDataType=0x001b\nAccessType=rw\n\n[3108sub65]\nParameterName=MOD_CfgEntry_01_U64\nObjectType=0x7\nDataType=0x001b\nAccessType=rw\n\n[3108sub66]\nParameterName=MOD_CfgEntry_02_U64\nObjectType=0x7\nDataType=0x001b\nAccessType=rw\n\n[3108sub67]\nParameterName=MOD_CfgEntry_03_U64\nObjectType=0x7\nDataType=0x001b\nAccessType=rw\n\n[3108sub68]\nParameterName=MOD_CfgEntry_04_U64\nObjectType=0x7\nDataType=0x001b\nAccessType=rw\n\n[3109]\nParameterName=MOD_Config_xxh_REC\nObjectType=0x9\nSubNumber=36\n\n[3109sub0]\nParameterName=Number of Entries\nObjectType=0x7\nDataType=0x0005\nAccessType=ro\nDefaultValue=0x68\nLowLimit=0x0\nHighLimit=0xFF\n\n[3109sub1]\nParameterName=MOD_ChildCfgIndex_U16\nObjectType=0x7\nDataType=0x0006\nAccessType=rw\n\n[3109sub2]\nParameterName=MOD_ChildCfgCount_U8\nObjectType=0x7\nDataType=0x0005\nAccessType=rw\n\n[3109sub3]\nParameterName=MOD_ChildActCount_U8\nObjectType=0x7\nDataType=0x0005\nAccessType=rw\n\n[3109sub4]\nParameterName=MOD_CfgMode_U8\nObjectType=0x7\nDataType=0x0005\nAccessType=rw\n\n[3109sub5]\nParameterName=MOD_RequestedHardwareId_U16\nObjectType=0x7\nDataType=0x0006\nAccessType=rw\n\n[3109sub6]\nParameterName=MOD_RequestedVendorId_U16\nObjectType=0x7\nDataType=0x0006\nAccessType=rw\n\n[3109sub7]\nParameterName=MOD_HardwareId_U16\nObjectType=0x7\nDataType=0x0006\nAccessType=ro\n\n[3109sub8]\nParameterName=MOD_VendorId_U16\nObjectType=0x7\nDataType=0x0006\nAccessType=ro\n\n[3109sub9]\nParameterName=MOD_InterfaceFlags_U8\nObjectType=0x7\nDataType=0x0005\nAccessType=ro\n\n[3109subA]\nParameterName=MOD_Status_U16\nObjectType=0x7\nDataType=0x0006\nAccessType=rw\n\n[3109subB]\nParameterName=MOD_NetworkStatus_U8\nObjectType=0x7\nDataType=0x0005\nAccessType=ro\n\n[3109subC]\nParameterName=MOD_BlockMask_U8\nObjectType=0x7\nDataType=0x0005\nAccessType=ro\n\n[3109subD]\nParameterName=MOD_BootCount_U8\nObjectType=0x7\nDataType=0x0005\nAccessType=rw\n\n[3109subE]\nParameterName=MOD_LastError_U8\nObjectType=0x7\nDataType=0x0005\nAccessType=rw\n\n[3109sub11]\nParameterName=MOD_FirmwareVersion_U16\nObjectType=0x7\nDataType=0x0006\nAccessType=ro\n\n[3109sub12]\nParameterName=MOD_HardwareVariant_U16\nObjectType=0x7\nDataType=0x0006\nAccessType=ro\n\n[3109sub13]\nParameterName=MOD_SerialNo_U32\nObjectType=0x7\nDataType=0x0007\nAccessType=ro\n\n[3109sub14]\nParameterName=MOD_PhysicalSlotNumber_U8\nObjectType=0x7\nDataType=0x0005\nAccessType=ro\n\n[3109sub15]\nParameterName=MOD_NodeSwitch_U8\nObjectType=0x7\nDataType=0x0005\nAccessType=ro\n\n[3109sub16]\nParameterName=MOD_RequestedSerialNo_U32\nObjectType=0x7\nDataType=0x0007\nAccessType=rw\n\n[3109sub17]\nParameterName=MOD_ModuleErrorReaction_U8\nObjectType=0x7\nDataType=0x0005\nAccessType=rw\n\n[3109sub21]\nParameterName=MOD_AsyncRead_U64\nObjectType=0x7\nDataType=0x001b\nAccessType=rw\n\n[3109sub22]\nParameterName=MOD_AsyncWrite_U64\nObjectType=0x7\nDataType=0x001b\nAccessType=wo\n\n[3109sub23]\nParameterName=MOD_Firmware_DOM\nObjectType=0x7\nDataType=0x000f\nAccessType=wo\n\n[3109sub24]\nParameterName=MOD_AsyncReadReg_U32\nObjectType=0x7\nDataType=0x0007\nAccessType=rw\n\n[3109sub25]\nParameterName=MOD_AsyncReadVal_U32\nObjectType=0x7\nDataType=0x0007\nAccessType=ro\n\n[3109sub26]\nParameterName=MOD_AsyncWriteReg_U32\nObjectType=0x7\nDataType=0x0007\nAccessType=rw\n\n[3109sub27]\nParameterName=MOD_AsyncWriteVal_U32\nObjectType=0x7\nDataType=0x0007\nAccessType=wo\n\n[3109sub5A]\nParameterName=MOD_CfgFunctionMode_U8\nObjectType=0x7\nDataType=0x0005\nAccessType=rw\n\n[3109sub5B]\nParameterName=MOD_CfgEntryCount_U8\nObjectType=0x7\nDataType=0x0005\nAccessType=rw\n\n[3109sub64]\nParameterName=MOD_CfgEntry_00_U64\nObjectType=0x7\nDataType=0x001b\nAccessType=rw\n\n[3109sub65]\nParameterName=MOD_CfgEntry_01_U64\nObjectType=0x7\nDataType=0x001b\nAccessType=rw\n\n[3109sub66]\nParameterName=MOD_CfgEntry_02_U64\nObjectType=0x7\nDataType=0x001b\nAccessType=rw\n\n[3109sub67]\nParameterName=MOD_CfgEntry_03_U64\nObjectType=0x7\nDataType=0x001b\nAccessType=rw\n\n[3109sub68]\nParameterName=MOD_CfgEntry_04_U64\nObjectType=0x7\nDataType=0x001b\nAccessType=rw\n\n[310A]\nParameterName=MOD_Config_xxh_REC\nObjectType=0x9\nSubNumber=36\n\n[310Asub0]\nParameterName=Number of Entries\nObjectType=0x7\nDataType=0x0005\nAccessType=ro\nDefaultValue=0x68\nLowLimit=0x0\nHighLimit=0xFF\n\n[310Asub1]\nParameterName=MOD_ChildCfgIndex_U16\nObjectType=0x7\nDataType=0x0006\nAccessType=rw\n\n[310Asub2]\nParameterName=MOD_ChildCfgCount_U8\nObjectType=0x7\nDataType=0x0005\nAccessType=rw\n\n[310Asub3]\nParameterName=MOD_ChildActCount_U8\nObjectType=0x7\nDataType=0x0005\nAccessType=rw\n\n[310Asub4]\nParameterName=MOD_CfgMode_U8\nObjectType=0x7\nDataType=0x0005\nAccessType=rw\n\n[310Asub5]\nParameterName=MOD_RequestedHardwareId_U16\nObjectType=0x7\nDataType=0x0006\nAccessType=rw\n\n[310Asub6]\nParameterName=MOD_RequestedVendorId_U16\nObjectType=0x7\nDataType=0x0006\nAccessType=rw\n\n[310Asub7]\nParameterName=MOD_HardwareId_U16\nObjectType=0x7\nDataType=0x0006\nAccessType=ro\n\n[310Asub8]\nParameterName=MOD_VendorId_U16\nObjectType=0x7\nDataType=0x0006\nAccessType=ro\n\n[310Asub9]\nParameterName=MOD_InterfaceFlags_U8\nObjectType=0x7\nDataType=0x0005\nAccessType=ro\n\n[310AsubA]\nParameterName=MOD_Status_U16\nObjectType=0x7\nDataType=0x0006\nAccessType=rw\n\n[310AsubB]\nParameterName=MOD_NetworkStatus_U8\nObjectType=0x7\nDataType=0x0005\nAccessType=ro\n\n[310AsubC]\nParameterName=MOD_BlockMask_U8\nObjectType=0x7\nDataType=0x0005\nAccessType=ro\n\n[310AsubD]\nParameterName=MOD_BootCount_U8\nObjectType=0x7\nDataType=0x0005\nAccessType=rw\n\n[310AsubE]\nParameterName=MOD_LastError_U8\nObjectType=0x7\nDataType=0x0005\nAccessType=rw\n\n[310Asub11]\nParameterName=MOD_FirmwareVersion_U16\nObjectType=0x7\nDataType=0x0006\nAccessType=ro\n\n[310Asub12]\nParameterName=MOD_HardwareVariant_U16\nObjectType=0x7\nDataType=0x0006\nAccessType=ro\n\n[310Asub13]\nParameterName=MOD_SerialNo_U32\nObjectType=0x7\nDataType=0x0007\nAccessType=ro\n\n[310Asub14]\nParameterName=MOD_PhysicalSlotNumber_U8\nObjectType=0x7\nDataType=0x0005\nAccessType=ro\n\n[310Asub15]\nParameterName=MOD_NodeSwitch_U8\nObjectType=0x7\nDataType=0x0005\nAccessType=ro\n\n[310Asub16]\nParameterName=MOD_RequestedSerialNo_U32\nObjectType=0x7\nDataType=0x0007\nAccessType=rw\n\n[310Asub17]\nParameterName=MOD_ModuleErrorReaction_U8\nObjectType=0x7\nDataType=0x0005\nAccessType=rw\n\n[310Asub21]\nParameterName=MOD_AsyncRead_U64\nObjectType=0x7\nDataType=0x001b\nAccessType=rw\n\n[310Asub22]\nParameterName=MOD_AsyncWrite_U64\nObjectType=0x7\nDataType=0x001b\nAccessType=wo\n\n[310Asub23]\nParameterName=MOD_Firmware_DOM\nObjectType=0x7\nDataType=0x000f\nAccessType=wo\n\n[310Asub24]\nParameterName=MOD_AsyncReadReg_U32\nObjectType=0x7\nDataType=0x0007\nAccessType=rw\n\n[310Asub25]\nParameterName=MOD_AsyncReadVal_U32\nObjectType=0x7\nDataType=0x0007\nAccessType=ro\n\n[310Asub26]\nParameterName=MOD_AsyncWriteReg_U32\nObjectType=0x7\nDataType=0x0007\nAccessType=rw\n\n[310Asub27]\nParameterName=MOD_AsyncWriteVal_U32\nObjectType=0x7\nDataType=0x0007\nAccessType=wo\n\n[310Asub5A]\nParameterName=MOD_CfgFunctionMode_U8\nObjectType=0x7\nDataType=0x0005\nAccessType=rw\n\n[310Asub5B]\nParameterName=MOD_CfgEntryCount_U8\nObjectType=0x7\nDataType=0x0005\nAccessType=rw\n\n[310Asub64]\nParameterName=MOD_CfgEntry_00_U64\nObjectType=0x7\nDataType=0x001b\nAccessType=rw\n\n[310Asub65]\nParameterName=MOD_CfgEntry_01_U64\nObjectType=0x7\nDataType=0x001b\nAccessType=rw\n\n[310Asub66]\nParameterName=MOD_CfgEntry_02_U64\nObjectType=0x7\nDataType=0x001b\nAccessType=rw\n\n[310Asub67]\nParameterName=MOD_CfgEntry_03_U64\nObjectType=0x7\nDataType=0x001b\nAccessType=rw\n\n[310Asub68]\nParameterName=MOD_CfgEntry_04_U64\nObjectType=0x7\nDataType=0x001b\nAccessType=rw\n\n[310B]\nParameterName=MOD_Config_xxh_REC\nObjectType=0x9\nSubNumber=36\n\n[310Bsub0]\nParameterName=Number of Entries\nObjectType=0x7\nDataType=0x0005\nAccessType=ro\nDefaultValue=0x68\nLowLimit=0x0\nHighLimit=0xFF\n\n[310Bsub1]\nParameterName=MOD_ChildCfgIndex_U16\nObjectType=0x7\nDataType=0x0006\nAccessType=rw\n\n[310Bsub2]\nParameterName=MOD_ChildCfgCount_U8\nObjectType=0x7\nDataType=0x0005\nAccessType=rw\n\n[310Bsub3]\nParameterName=MOD_ChildActCount_U8\nObjectType=0x7\nDataType=0x0005\nAccessType=rw\n\n[310Bsub4]\nParameterName=MOD_CfgMode_U8\nObjectType=0x7\nDataType=0x0005\nAccessType=rw\n\n[310Bsub5]\nParameterName=MOD_RequestedHardwareId_U16\nObjectType=0x7\nDataType=0x0006\nAccessType=rw\n\n[310Bsub6]\nParameterName=MOD_RequestedVendorId_U16\nObjectType=0x7\nDataType=0x0006\nAccessType=rw\n\n[310Bsub7]\nParameterName=MOD_HardwareId_U16\nObjectType=0x7\nDataType=0x0006\nAccessType=ro\n\n[310Bsub8]\nParameterName=MOD_VendorId_U16\nObjectType=0x7\nDataType=0x0006\nAccessType=ro\n\n[310Bsub9]\nParameterName=MOD_InterfaceFlags_U8\nObjectType=0x7\nDataType=0x0005\nAccessType=ro\n\n[310BsubA]\nParameterName=MOD_Status_U16\nObjectType=0x7\nDataType=0x0006\nAccessType=rw\n\n[310BsubB]\nParameterName=MOD_NetworkStatus_U8\nObjectType=0x7\nDataType=0x0005\nAccessType=ro\n\n[310BsubC]\nParameterName=MOD_BlockMask_U8\nObjectType=0x7\nDataType=0x0005\nAccessType=ro\n\n[310BsubD]\nParameterName=MOD_BootCount_U8\nObjectType=0x7\nDataType=0x0005\nAccessType=rw\n\n[310BsubE]\nParameterName=MOD_LastError_U8\nObjectType=0x7\nDataType=0x0005\nAccessType=rw\n\n[310Bsub11]\nParameterName=MOD_FirmwareVersion_U16\nObjectType=0x7\nDataType=0x0006\nAccessType=ro\n\n[310Bsub12]\nParameterName=MOD_HardwareVariant_U16\nObjectType=0x7\nDataType=0x0006\nAccessType=ro\n\n[310Bsub13]\nParameterName=MOD_SerialNo_U32\nObjectType=0x7\nDataType=0x0007\nAccessType=ro\n\n[310Bsub14]\nParameterName=MOD_PhysicalSlotNumber_U8\nObjectType=0x7\nDataType=0x0005\nAccessType=ro\n\n[310Bsub15]\nParameterName=MOD_NodeSwitch_U8\nObjectType=0x7\nDataType=0x0005\nAccessType=ro\n\n[310Bsub16]\nParameterName=MOD_RequestedSerialNo_U32\nObjectType=0x7\nDataType=0x0007\nAccessType=rw\n\n[310Bsub17]\nParameterName=MOD_ModuleErrorReaction_U8\nObjectType=0x7\nDataType=0x0005\nAccessType=rw\n\n[310Bsub21]\nParameterName=MOD_AsyncRead_U64\nObjectType=0x7\nDataType=0x001b\nAccessType=rw\n\n[310Bsub22]\nParameterName=MOD_AsyncWrite_U64\nObjectType=0x7\nDataType=0x001b\nAccessType=wo\n\n[310Bsub23]\nParameterName=MOD_Firmware_DOM\nObjectType=0x7\nDataType=0x000f\nAccessType=wo\n\n[310Bsub24]\nParameterName=MOD_AsyncReadReg_U32\nObjectType=0x7\nDataType=0x0007\nAccessType=rw\n\n[310Bsub25]\nParameterName=MOD_AsyncReadVal_U32\nObjectType=0x7\nDataType=0x0007\nAccessType=ro\n\n[310Bsub26]\nParameterName=MOD_AsyncWriteReg_U32\nObjectType=0x7\nDataType=0x0007\nAccessType=rw\n\n[310Bsub27]\nParameterName=MOD_AsyncWriteVal_U32\nObjectType=0x7\nDataType=0x0007\nAccessType=wo\n\n[310Bsub5A]\nParameterName=MOD_CfgFunctionMode_U8\nObjectType=0x7\nDataType=0x0005\nAccessType=rw\n\n[310Bsub5B]\nParameterName=MOD_CfgEntryCount_U8\nObjectType=0x7\nDataType=0x0005\nAccessType=rw\n\n[310Bsub64]\nParameterName=MOD_CfgEntry_00_U64\nObjectType=0x7\nDataType=0x001b\nAccessType=rw\n\n[310Bsub65]\nParameterName=MOD_CfgEntry_01_U64\nObjectType=0x7\nDataType=0x001b\nAccessType=rw\n\n[310Bsub66]\nParameterName=MOD_CfgEntry_02_U64\nObjectType=0x7\nDataType=0x001b\nAccessType=rw\n\n[310Bsub67]\nParameterName=MOD_CfgEntry_03_U64\nObjectType=0x7\nDataType=0x001b\nAccessType=rw\n\n[310Bsub68]\nParameterName=MOD_CfgEntry_04_U64\nObjectType=0x7\nDataType=0x001b\nAccessType=rw\n\n[310C]\nParameterName=MOD_Config_xxh_REC\nObjectType=0x9\nSubNumber=36\n\n[310Csub0]\nParameterName=Number of Entries\nObjectType=0x7\nDataType=0x0005\nAccessType=ro\nDefaultValue=0x68\nLowLimit=0x0\nHighLimit=0xFF\n\n[310Csub1]\nParameterName=MOD_ChildCfgIndex_U16\nObjectType=0x7\nDataType=0x0006\nAccessType=rw\n\n[310Csub2]\nParameterName=MOD_ChildCfgCount_U8\nObjectType=0x7\nDataType=0x0005\nAccessType=rw\n\n[310Csub3]\nParameterName=MOD_ChildActCount_U8\nObjectType=0x7\nDataType=0x0005\nAccessType=rw\n\n[310Csub4]\nParameterName=MOD_CfgMode_U8\nObjectType=0x7\nDataType=0x0005\nAccessType=rw\n\n[310Csub5]\nParameterName=MOD_RequestedHardwareId_U16\nObjectType=0x7\nDataType=0x0006\nAccessType=rw\n\n[310Csub6]\nParameterName=MOD_RequestedVendorId_U16\nObjectType=0x7\nDataType=0x0006\nAccessType=rw\n\n[310Csub7]\nParameterName=MOD_HardwareId_U16\nObjectType=0x7\nDataType=0x0006\nAccessType=ro\n\n[310Csub8]\nParameterName=MOD_VendorId_U16\nObjectType=0x7\nDataType=0x0006\nAccessType=ro\n\n[310Csub9]\nParameterName=MOD_InterfaceFlags_U8\nObjectType=0x7\nDataType=0x0005\nAccessType=ro\n\n[310CsubA]\nParameterName=MOD_Status_U16\nObjectType=0x7\nDataType=0x0006\nAccessType=rw\n\n[310CsubB]\nParameterName=MOD_NetworkStatus_U8\nObjectType=0x7\nDataType=0x0005\nAccessType=ro\n\n[310CsubC]\nParameterName=MOD_BlockMask_U8\nObjectType=0x7\nDataType=0x0005\nAccessType=ro\n\n[310CsubD]\nParameterName=MOD_BootCount_U8\nObjectType=0x7\nDataType=0x0005\nAccessType=rw\n\n[310CsubE]\nParameterName=MOD_LastError_U8\nObjectType=0x7\nDataType=0x0005\nAccessType=rw\n\n[310Csub11]\nParameterName=MOD_FirmwareVersion_U16\nObjectType=0x7\nDataType=0x0006\nAccessType=ro\n\n[310Csub12]\nParameterName=MOD_HardwareVariant_U16\nObjectType=0x7\nDataType=0x0006\nAccessType=ro\n\n[310Csub13]\nParameterName=MOD_SerialNo_U32\nObjectType=0x7\nDataType=0x0007\nAccessType=ro\n\n[310Csub14]\nParameterName=MOD_PhysicalSlotNumber_U8\nObjectType=0x7\nDataType=0x0005\nAccessType=ro\n\n[310Csub15]\nParameterName=MOD_NodeSwitch_U8\nObjectType=0x7\nDataType=0x0005\nAccessType=ro\n\n[310Csub16]\nParameterName=MOD_RequestedSerialNo_U32\nObjectType=0x7\nDataType=0x0007\nAccessType=rw\n\n[310Csub17]\nParameterName=MOD_ModuleErrorReaction_U8\nObjectType=0x7\nDataType=0x0005\nAccessType=rw\n\n[310Csub21]\nParameterName=MOD_AsyncRead_U64\nObjectType=0x7\nDataType=0x001b\nAccessType=rw\n\n[310Csub22]\nParameterName=MOD_AsyncWrite_U64\nObjectType=0x7\nDataType=0x001b\nAccessType=wo\n\n[310Csub23]\nParameterName=MOD_Firmware_DOM\nObjectType=0x7\nDataType=0x000f\nAccessType=wo\n\n[310Csub24]\nParameterName=MOD_AsyncReadReg_U32\nObjectType=0x7\nDataType=0x0007\nAccessType=rw\n\n[310Csub25]\nParameterName=MOD_AsyncReadVal_U32\nObjectType=0x7\nDataType=0x0007\nAccessType=ro\n\n[310Csub26]\nParameterName=MOD_AsyncWriteReg_U32\nObjectType=0x7\nDataType=0x0007\nAccessType=rw\n\n[310Csub27]\nParameterName=MOD_AsyncWriteVal_U32\nObjectType=0x7\nDataType=0x0007\nAccessType=wo\n\n[310Csub5A]\nParameterName=MOD_CfgFunctionMode_U8\nObjectType=0x7\nDataType=0x0005\nAccessType=rw\n\n[310Csub5B]\nParameterName=MOD_CfgEntryCount_U8\nObjectType=0x7\nDataType=0x0005\nAccessType=rw\n\n[310Csub64]\nParameterName=MOD_CfgEntry_00_U64\nObjectType=0x7\nDataType=0x001b\nAccessType=rw\n\n[310Csub65]\nParameterName=MOD_CfgEntry_01_U64\nObjectType=0x7\nDataType=0x001b\nAccessType=rw\n\n[310Csub66]\nParameterName=MOD_CfgEntry_02_U64\nObjectType=0x7\nDataType=0x001b\nAccessType=rw\n\n[310Csub67]\nParameterName=MOD_CfgEntry_03_U64\nObjectType=0x7\nDataType=0x001b\nAccessType=rw\n\n[310Csub68]\nParameterName=MOD_CfgEntry_04_U64\nObjectType=0x7\nDataType=0x001b\nAccessType=rw\n\n[310D]\nParameterName=MOD_Config_xxh_REC\nObjectType=0x9\nSubNumber=36\n\n[310Dsub0]\nParameterName=Number of Entries\nObjectType=0x7\nDataType=0x0005\nAccessType=ro\nDefaultValue=0x68\nLowLimit=0x0\nHighLimit=0xFF\n\n[310Dsub1]\nParameterName=MOD_ChildCfgIndex_U16\nObjectType=0x7\nDataType=0x0006\nAccessType=rw\n\n[310Dsub2]\nParameterName=MOD_ChildCfgCount_U8\nObjectType=0x7\nDataType=0x0005\nAccessType=rw\n\n[310Dsub3]\nParameterName=MOD_ChildActCount_U8\nObjectType=0x7\nDataType=0x0005\nAccessType=rw\n\n[310Dsub4]\nParameterName=MOD_CfgMode_U8\nObjectType=0x7\nDataType=0x0005\nAccessType=rw\n\n[310Dsub5]\nParameterName=MOD_RequestedHardwareId_U16\nObjectType=0x7\nDataType=0x0006\nAccessType=rw\n\n[310Dsub6]\nParameterName=MOD_RequestedVendorId_U16\nObjectType=0x7\nDataType=0x0006\nAccessType=rw\n\n[310Dsub7]\nParameterName=MOD_HardwareId_U16\nObjectType=0x7\nDataType=0x0006\nAccessType=ro\n\n[310Dsub8]\nParameterName=MOD_VendorId_U16\nObjectType=0x7\nDataType=0x0006\nAccessType=ro\n\n[310Dsub9]\nParameterName=MOD_InterfaceFlags_U8\nObjectType=0x7\nDataType=0x0005\nAccessType=ro\n\n[310DsubA]\nParameterName=MOD_Status_U16\nObjectType=0x7\nDataType=0x0006\nAccessType=rw\n\n[310DsubB]\nParameterName=MOD_NetworkStatus_U8\nObjectType=0x7\nDataType=0x0005\nAccessType=ro\n\n[310DsubC]\nParameterName=MOD_BlockMask_U8\nObjectType=0x7\nDataType=0x0005\nAccessType=ro\n\n[310DsubD]\nParameterName=MOD_BootCount_U8\nObjectType=0x7\nDataType=0x0005\nAccessType=rw\n\n[310DsubE]\nParameterName=MOD_LastError_U8\nObjectType=0x7\nDataType=0x0005\nAccessType=rw\n\n[310Dsub11]\nParameterName=MOD_FirmwareVersion_U16\nObjectType=0x7\nDataType=0x0006\nAccessType=ro\n\n[310Dsub12]\nParameterName=MOD_HardwareVariant_U16\nObjectType=0x7\nDataType=0x0006\nAccessType=ro\n\n[310Dsub13]\nParameterName=MOD_SerialNo_U32\nObjectType=0x7\nDataType=0x0007\nAccessType=ro\n\n[310Dsub14]\nParameterName=MOD_PhysicalSlotNumber_U8\nObjectType=0x7\nDataType=0x0005\nAccessType=ro\n\n[310Dsub15]\nParameterName=MOD_NodeSwitch_U8\nObjectType=0x7\nDataType=0x0005\nAccessType=ro\n\n[310Dsub16]\nParameterName=MOD_RequestedSerialNo_U32\nObjectType=0x7\nDataType=0x0007\nAccessType=rw\n\n[310Dsub17]\nParameterName=MOD_ModuleErrorReaction_U8\nObjectType=0x7\nDataType=0x0005\nAccessType=rw\n\n[310Dsub21]\nParameterName=MOD_AsyncRead_U64\nObjectType=0x7\nDataType=0x001b\nAccessType=rw\n\n[310Dsub22]\nParameterName=MOD_AsyncWrite_U64\nObjectType=0x7\nDataType=0x001b\nAccessType=wo\n\n[310Dsub23]\nParameterName=MOD_Firmware_DOM\nObjectType=0x7\nDataType=0x000f\nAccessType=wo\n\n[310Dsub24]\nParameterName=MOD_AsyncReadReg_U32\nObjectType=0x7\nDataType=0x0007\nAccessType=rw\n\n[310Dsub25]\nParameterName=MOD_AsyncReadVal_U32\nObjectType=0x7\nDataType=0x0007\nAccessType=ro\n\n[310Dsub26]\nParameterName=MOD_AsyncWriteReg_U32\nObjectType=0x7\nDataType=0x0007\nAccessType=rw\n\n[310Dsub27]\nParameterName=MOD_AsyncWriteVal_U32\nObjectType=0x7\nDataType=0x0007\nAccessType=wo\n\n[310Dsub5A]\nParameterName=MOD_CfgFunctionMode_U8\nObjectType=0x7\nDataType=0x0005\nAccessType=rw\n\n[310Dsub5B]\nParameterName=MOD_CfgEntryCount_U8\nObjectType=0x7\nDataType=0x0005\nAccessType=rw\n\n[310Dsub64]\nParameterName=MOD_CfgEntry_00_U64\nObjectType=0x7\nDataType=0x001b\nAccessType=rw\n\n[310Dsub65]\nParameterName=MOD_CfgEntry_01_U64\nObjectType=0x7\nDataType=0x001b\nAccessType=rw\n\n[310Dsub66]\nParameterName=MOD_CfgEntry_02_U64\nObjectType=0x7\nDataType=0x001b\nAccessType=rw\n\n[310Dsub67]\nParameterName=MOD_CfgEntry_03_U64\nObjectType=0x7\nDataType=0x001b\nAccessType=rw\n\n[310Dsub68]\nParameterName=MOD_CfgEntry_04_U64\nObjectType=0x7\nDataType=0x001b\nAccessType=rw\n\n[310E]\nParameterName=MOD_Config_xxh_REC\nObjectType=0x9\nSubNumber=36\n\n[310Esub0]\nParameterName=Number of Entries\nObjectType=0x7\nDataType=0x0005\nAccessType=ro\nDefaultValue=0x68\nLowLimit=0x0\nHighLimit=0xFF\n\n[310Esub1]\nParameterName=MOD_ChildCfgIndex_U16\nObjectType=0x7\nDataType=0x0006\nAccessType=rw\n\n[310Esub2]\nParameterName=MOD_ChildCfgCount_U8\nObjectType=0x7\nDataType=0x0005\nAccessType=rw\n\n[310Esub3]\nParameterName=MOD_ChildActCount_U8\nObjectType=0x7\nDataType=0x0005\nAccessType=rw\n\n[310Esub4]\nParameterName=MOD_CfgMode_U8\nObjectType=0x7\nDataType=0x0005\nAccessType=rw\n\n[310Esub5]\nParameterName=MOD_RequestedHardwareId_U16\nObjectType=0x7\nDataType=0x0006\nAccessType=rw\n\n[310Esub6]\nParameterName=MOD_RequestedVendorId_U16\nObjectType=0x7\nDataType=0x0006\nAccessType=rw\n\n[310Esub7]\nParameterName=MOD_HardwareId_U16\nObjectType=0x7\nDataType=0x0006\nAccessType=ro\n\n[310Esub8]\nParameterName=MOD_VendorId_U16\nObjectType=0x7\nDataType=0x0006\nAccessType=ro\n\n[310Esub9]\nParameterName=MOD_InterfaceFlags_U8\nObjectType=0x7\nDataType=0x0005\nAccessType=ro\n\n[310EsubA]\nParameterName=MOD_Status_U16\nObjectType=0x7\nDataType=0x0006\nAccessType=rw\n\n[310EsubB]\nParameterName=MOD_NetworkStatus_U8\nObjectType=0x7\nDataType=0x0005\nAccessType=ro\n\n[310EsubC]\nParameterName=MOD_BlockMask_U8\nObjectType=0x7\nDataType=0x0005\nAccessType=ro\n\n[310EsubD]\nParameterName=MOD_BootCount_U8\nObjectType=0x7\nDataType=0x0005\nAccessType=rw\n\n[310EsubE]\nParameterName=MOD_LastError_U8\nObjectType=0x7\nDataType=0x0005\nAccessType=rw\n\n[310Esub11]\nParameterName=MOD_FirmwareVersion_U16\nObjectType=0x7\nDataType=0x0006\nAccessType=ro\n\n[310Esub12]\nParameterName=MOD_HardwareVariant_U16\nObjectType=0x7\nDataType=0x0006\nAccessType=ro\n\n[310Esub13]\nParameterName=MOD_SerialNo_U32\nObjectType=0x7\nDataType=0x0007\nAccessType=ro\n\n[310Esub14]\nParameterName=MOD_PhysicalSlotNumber_U8\nObjectType=0x7\nDataType=0x0005\nAccessType=ro\n\n[310Esub15]\nParameterName=MOD_NodeSwitch_U8\nObjectType=0x7\nDataType=0x0005\nAccessType=ro\n\n[310Esub16]\nParameterName=MOD_RequestedSerialNo_U32\nObjectType=0x7\nDataType=0x0007\nAccessType=rw\n\n[310Esub17]\nParameterName=MOD_ModuleErrorReaction_U8\nObjectType=0x7\nDataType=0x0005\nAccessType=rw\n\n[310Esub21]\nParameterName=MOD_AsyncRead_U64\nObjectType=0x7\nDataType=0x001b\nAccessType=rw\n\n[310Esub22]\nParameterName=MOD_AsyncWrite_U64\nObjectType=0x7\nDataType=0x001b\nAccessType=wo\n\n[310Esub23]\nParameterName=MOD_Firmware_DOM\nObjectType=0x7\nDataType=0x000f\nAccessType=wo\n\n[310Esub24]\nParameterName=MOD_AsyncReadReg_U32\nObjectType=0x7\nDataType=0x0007\nAccessType=rw\n\n[310Esub25]\nParameterName=MOD_AsyncReadVal_U32\nObjectType=0x7\nDataType=0x0007\nAccessType=ro\n\n[310Esub26]\nParameterName=MOD_AsyncWriteReg_U32\nObjectType=0x7\nDataType=0x0007\nAccessType=rw\n\n[310Esub27]\nParameterName=MOD_AsyncWriteVal_U32\nObjectType=0x7\nDataType=0x0007\nAccessType=wo\n\n[310Esub5A]\nParameterName=MOD_CfgFunctionMode_U8\nObjectType=0x7\nDataType=0x0005\nAccessType=rw\n\n[310Esub5B]\nParameterName=MOD_CfgEntryCount_U8\nObjectType=0x7\nDataType=0x0005\nAccessType=rw\n\n[310Esub64]\nParameterName=MOD_CfgEntry_00_U64\nObjectType=0x7\nDataType=0x001b\nAccessType=rw\n\n[310Esub65]\nParameterName=MOD_CfgEntry_01_U64\nObjectType=0x7\nDataType=0x001b\nAccessType=rw\n\n[310Esub66]\nParameterName=MOD_CfgEntry_02_U64\nObjectType=0x7\nDataType=0x001b\nAccessType=rw\n\n[310Esub67]\nParameterName=MOD_CfgEntry_03_U64\nObjectType=0x7\nDataType=0x001b\nAccessType=rw\n\n[310Esub68]\nParameterName=MOD_CfgEntry_04_U64\nObjectType=0x7\nDataType=0x001b\nAccessType=rw\n\n[310F]\nParameterName=MOD_Config_xxh_REC\nObjectType=0x9\nSubNumber=36\n\n[310Fsub0]\nParameterName=Number of Entries\nObjectType=0x7\nDataType=0x0005\nAccessType=ro\nDefaultValue=0x68\nLowLimit=0x0\nHighLimit=0xFF\n\n[310Fsub1]\nParameterName=MOD_ChildCfgIndex_U16\nObjectType=0x7\nDataType=0x0006\nAccessType=rw\n\n[310Fsub2]\nParameterName=MOD_ChildCfgCount_U8\nObjectType=0x7\nDataType=0x0005\nAccessType=rw\n\n[310Fsub3]\nParameterName=MOD_ChildActCount_U8\nObjectType=0x7\nDataType=0x0005\nAccessType=rw\n\n[310Fsub4]\nParameterName=MOD_CfgMode_U8\nObjectType=0x7\nDataType=0x0005\nAccessType=rw\n\n[310Fsub5]\nParameterName=MOD_RequestedHardwareId_U16\nObjectType=0x7\nDataType=0x0006\nAccessType=rw\n\n[310Fsub6]\nParameterName=MOD_RequestedVendorId_U16\nObjectType=0x7\nDataType=0x0006\nAccessType=rw\n\n[310Fsub7]\nParameterName=MOD_HardwareId_U16\nObjectType=0x7\nDataType=0x0006\nAccessType=ro\n\n[310Fsub8]\nParameterName=MOD_VendorId_U16\nObjectType=0x7\nDataType=0x0006\nAccessType=ro\n\n[310Fsub9]\nParameterName=MOD_InterfaceFlags_U8\nObjectType=0x7\nDataType=0x0005\nAccessType=ro\n\n[310FsubA]\nParameterName=MOD_Status_U16\nObjectType=0x7\nDataType=0x0006\nAccessType=rw\n\n[310FsubB]\nParameterName=MOD_NetworkStatus_U8\nObjectType=0x7\nDataType=0x0005\nAccessType=ro\n\n[310FsubC]\nParameterName=MOD_BlockMask_U8\nObjectType=0x7\nDataType=0x0005\nAccessType=ro\n\n[310FsubD]\nParameterName=MOD_BootCount_U8\nObjectType=0x7\nDataType=0x0005\nAccessType=rw\n\n[310FsubE]\nParameterName=MOD_LastError_U8\nObjectType=0x7\nDataType=0x0005\nAccessType=rw\n\n[310Fsub11]\nParameterName=MOD_FirmwareVersion_U16\nObjectType=0x7\nDataType=0x0006\nAccessType=ro\n\n[310Fsub12]\nParameterName=MOD_HardwareVariant_U16\nObjectType=0x7\nDataType=0x0006\nAccessType=ro\n\n[310Fsub13]\nParameterName=MOD_SerialNo_U32\nObjectType=0x7\nDataType=0x0007\nAccessType=ro\n\n[310Fsub14]\nParameterName=MOD_PhysicalSlotNumber_U8\nObjectType=0x7\nDataType=0x0005\nAccessType=ro\n\n[310Fsub15]\nParameterName=MOD_NodeSwitch_U8\nObjectType=0x7\nDataType=0x0005\nAccessType=ro\n\n[310Fsub16]\nParameterName=MOD_RequestedSerialNo_U32\nObjectType=0x7\nDataType=0x0007\nAccessType=rw\n\n[310Fsub17]\nParameterName=MOD_ModuleErrorReaction_U8\nObjectType=0x7\nDataType=0x0005\nAccessType=rw\n\n[310Fsub21]\nParameterName=MOD_AsyncRead_U64\nObjectType=0x7\nDataType=0x001b\nAccessType=rw\n\n[310Fsub22]\nParameterName=MOD_AsyncWrite_U64\nObjectType=0x7\nDataType=0x001b\nAccessType=wo\n\n[310Fsub23]\nParameterName=MOD_Firmware_DOM\nObjectType=0x7\nDataType=0x000f\nAccessType=wo\n\n[310Fsub24]\nParameterName=MOD_AsyncReadReg_U32\nObjectType=0x7\nDataType=0x0007\nAccessType=rw\n\n[310Fsub25]\nParameterName=MOD_AsyncReadVal_U32\nObjectType=0x7\nDataType=0x0007\nAccessType=ro\n\n[310Fsub26]\nParameterName=MOD_AsyncWriteReg_U32\nObjectType=0x7\nDataType=0x0007\nAccessType=rw\n\n[310Fsub27]\nParameterName=MOD_AsyncWriteVal_U32\nObjectType=0x7\nDataType=0x0007\nAccessType=wo\n\n[310Fsub5A]\nParameterName=MOD_CfgFunctionMode_U8\nObjectType=0x7\nDataType=0x0005\nAccessType=rw\n\n[310Fsub5B]\nParameterName=MOD_CfgEntryCount_U8\nObjectType=0x7\nDataType=0x0005\nAccessType=rw\n\n[310Fsub64]\nParameterName=MOD_CfgEntry_00_U64\nObjectType=0x7\nDataType=0x001b\nAccessType=rw\n\n[310Fsub65]\nParameterName=MOD_CfgEntry_01_U64\nObjectType=0x7\nDataType=0x001b\nAccessType=rw\n\n[310Fsub66]\nParameterName=MOD_CfgEntry_02_U64\nObjectType=0x7\nDataType=0x001b\nAccessType=rw\n\n[310Fsub67]\nParameterName=MOD_CfgEntry_03_U64\nObjectType=0x7\nDataType=0x001b\nAccessType=rw\n\n[310Fsub68]\nParameterName=MOD_CfgEntry_04_U64\nObjectType=0x7\nDataType=0x001b\nAccessType=rw\n\n[3110]\nParameterName=MOD_Config_xxh_REC\nObjectType=0x9\nSubNumber=36\n\n[3110sub0]\nParameterName=Number of Entries\nObjectType=0x7\nDataType=0x0005\nAccessType=ro\nDefaultValue=0x68\nLowLimit=0x0\nHighLimit=0xFF\n\n[3110sub1]\nParameterName=MOD_ChildCfgIndex_U16\nObjectType=0x7\nDataType=0x0006\nAccessType=rw\n\n[3110sub2]\nParameterName=MOD_ChildCfgCount_U8\nObjectType=0x7\nDataType=0x0005\nAccessType=rw\n\n[3110sub3]\nParameterName=MOD_ChildActCount_U8\nObjectType=0x7\nDataType=0x0005\nAccessType=rw\n\n[3110sub4]\nParameterName=MOD_CfgMode_U8\nObjectType=0x7\nDataType=0x0005\nAccessType=rw\n\n[3110sub5]\nParameterName=MOD_RequestedHardwareId_U16\nObjectType=0x7\nDataType=0x0006\nAccessType=rw\n\n[3110sub6]\nParameterName=MOD_RequestedVendorId_U16\nObjectType=0x7\nDataType=0x0006\nAccessType=rw\n\n[3110sub7]\nParameterName=MOD_HardwareId_U16\nObjectType=0x7\nDataType=0x0006\nAccessType=ro\n\n[3110sub8]\nParameterName=MOD_VendorId_U16\nObjectType=0x7\nDataType=0x0006\nAccessType=ro\n\n[3110sub9]\nParameterName=MOD_InterfaceFlags_U8\nObjectType=0x7\nDataType=0x0005\nAccessType=ro\n\n[3110subA]\nParameterName=MOD_Status_U16\nObjectType=0x7\nDataType=0x0006\nAccessType=rw\n\n[3110subB]\nParameterName=MOD_NetworkStatus_U8\nObjectType=0x7\nDataType=0x0005\nAccessType=ro\n\n[3110subC]\nParameterName=MOD_BlockMask_U8\nObjectType=0x7\nDataType=0x0005\nAccessType=ro\n\n[3110subD]\nParameterName=MOD_BootCount_U8\nObjectType=0x7\nDataType=0x0005\nAccessType=rw\n\n[3110subE]\nParameterName=MOD_LastError_U8\nObjectType=0x7\nDataType=0x0005\nAccessType=rw\n\n[3110sub11]\nParameterName=MOD_FirmwareVersion_U16\nObjectType=0x7\nDataType=0x0006\nAccessType=ro\n\n[3110sub12]\nParameterName=MOD_HardwareVariant_U16\nObjectType=0x7\nDataType=0x0006\nAccessType=ro\n\n[3110sub13]\nParameterName=MOD_SerialNo_U32\nObjectType=0x7\nDataType=0x0007\nAccessType=ro\n\n[3110sub14]\nParameterName=MOD_PhysicalSlotNumber_U8\nObjectType=0x7\nDataType=0x0005\nAccessType=ro\n\n[3110sub15]\nParameterName=MOD_NodeSwitch_U8\nObjectType=0x7\nDataType=0x0005\nAccessType=ro\n\n[3110sub16]\nParameterName=MOD_RequestedSerialNo_U32\nObjectType=0x7\nDataType=0x0007\nAccessType=rw\n\n[3110sub17]\nParameterName=MOD_ModuleErrorReaction_U8\nObjectType=0x7\nDataType=0x0005\nAccessType=rw\n\n[3110sub21]\nParameterName=MOD_AsyncRead_U64\nObjectType=0x7\nDataType=0x001b\nAccessType=rw\n\n[3110sub22]\nParameterName=MOD_AsyncWrite_U64\nObjectType=0x7\nDataType=0x001b\nAccessType=wo\n\n[3110sub23]\nParameterName=MOD_Firmware_DOM\nObjectType=0x7\nDataType=0x000f\nAccessType=wo\n\n[3110sub24]\nParameterName=MOD_AsyncReadReg_U32\nObjectType=0x7\nDataType=0x0007\nAccessType=rw\n\n[3110sub25]\nParameterName=MOD_AsyncReadVal_U32\nObjectType=0x7\nDataType=0x0007\nAccessType=ro\n\n[3110sub26]\nParameterName=MOD_AsyncWriteReg_U32\nObjectType=0x7\nDataType=0x0007\nAccessType=rw\n\n[3110sub27]\nParameterName=MOD_AsyncWriteVal_U32\nObjectType=0x7\nDataType=0x0007\nAccessType=wo\n\n[3110sub5A]\nParameterName=MOD_CfgFunctionMode_U8\nObjectType=0x7\nDataType=0x0005\nAccessType=rw\n\n[3110sub5B]\nParameterName=MOD_CfgEntryCount_U8\nObjectType=0x7\nDataType=0x0005\nAccessType=rw\n\n[3110sub64]\nParameterName=MOD_CfgEntry_00_U64\nObjectType=0x7\nDataType=0x001b\nAccessType=rw\n\n[3110sub65]\nParameterName=MOD_CfgEntry_01_U64\nObjectType=0x7\nDataType=0x001b\nAccessType=rw\n\n[3110sub66]\nParameterName=MOD_CfgEntry_02_U64\nObjectType=0x7\nDataType=0x001b\nAccessType=rw\n\n[3110sub67]\nParameterName=MOD_CfgEntry_03_U64\nObjectType=0x7\nDataType=0x001b\nAccessType=rw\n\n[3110sub68]\nParameterName=MOD_CfgEntry_04_U64\nObjectType=0x7\nDataType=0x001b\nAccessType=rw\n\n[3111]\nParameterName=MOD_Config_xxh_REC\nObjectType=0x9\nSubNumber=36\n\n[3111sub0]\nParameterName=Number of Entries\nObjectType=0x7\nDataType=0x0005\nAccessType=ro\nDefaultValue=0x68\nLowLimit=0x0\nHighLimit=0xFF\n\n[3111sub1]\nParameterName=MOD_ChildCfgIndex_U16\nObjectType=0x7\nDataType=0x0006\nAccessType=rw\n\n[3111sub2]\nParameterName=MOD_ChildCfgCount_U8\nObjectType=0x7\nDataType=0x0005\nAccessType=rw\n\n[3111sub3]\nParameterName=MOD_ChildActCount_U8\nObjectType=0x7\nDataType=0x0005\nAccessType=rw\n\n[3111sub4]\nParameterName=MOD_CfgMode_U8\nObjectType=0x7\nDataType=0x0005\nAccessType=rw\n\n[3111sub5]\nParameterName=MOD_RequestedHardwareId_U16\nObjectType=0x7\nDataType=0x0006\nAccessType=rw\n\n[3111sub6]\nParameterName=MOD_RequestedVendorId_U16\nObjectType=0x7\nDataType=0x0006\nAccessType=rw\n\n[3111sub7]\nParameterName=MOD_HardwareId_U16\nObjectType=0x7\nDataType=0x0006\nAccessType=ro\n\n[3111sub8]\nParameterName=MOD_VendorId_U16\nObjectType=0x7\nDataType=0x0006\nAccessType=ro\n\n[3111sub9]\nParameterName=MOD_InterfaceFlags_U8\nObjectType=0x7\nDataType=0x0005\nAccessType=ro\n\n[3111subA]\nParameterName=MOD_Status_U16\nObjectType=0x7\nDataType=0x0006\nAccessType=rw\n\n[3111subB]\nParameterName=MOD_NetworkStatus_U8\nObjectType=0x7\nDataType=0x0005\nAccessType=ro\n\n[3111subC]\nParameterName=MOD_BlockMask_U8\nObjectType=0x7\nDataType=0x0005\nAccessType=ro\n\n[3111subD]\nParameterName=MOD_BootCount_U8\nObjectType=0x7\nDataType=0x0005\nAccessType=rw\n\n[3111subE]\nParameterName=MOD_LastError_U8\nObjectType=0x7\nDataType=0x0005\nAccessType=rw\n\n[3111sub11]\nParameterName=MOD_FirmwareVersion_U16\nObjectType=0x7\nDataType=0x0006\nAccessType=ro\n\n[3111sub12]\nParameterName=MOD_HardwareVariant_U16\nObjectType=0x7\nDataType=0x0006\nAccessType=ro\n\n[3111sub13]\nParameterName=MOD_SerialNo_U32\nObjectType=0x7\nDataType=0x0007\nAccessType=ro\n\n[3111sub14]\nParameterName=MOD_PhysicalSlotNumber_U8\nObjectType=0x7\nDataType=0x0005\nAccessType=ro\n\n[3111sub15]\nParameterName=MOD_NodeSwitch_U8\nObjectType=0x7\nDataType=0x0005\nAccessType=ro\n\n[3111sub16]\nParameterName=MOD_RequestedSerialNo_U32\nObjectType=0x7\nDataType=0x0007\nAccessType=rw\n\n[3111sub17]\nParameterName=MOD_ModuleErrorReaction_U8\nObjectType=0x7\nDataType=0x0005\nAccessType=rw\n\n[3111sub21]\nParameterName=MOD_AsyncRead_U64\nObjectType=0x7\nDataType=0x001b\nAccessType=rw\n\n[3111sub22]\nParameterName=MOD_AsyncWrite_U64\nObjectType=0x7\nDataType=0x001b\nAccessType=wo\n\n[3111sub23]\nParameterName=MOD_Firmware_DOM\nObjectType=0x7\nDataType=0x000f\nAccessType=wo\n\n[3111sub24]\nParameterName=MOD_AsyncReadReg_U32\nObjectType=0x7\nDataType=0x0007\nAccessType=rw\n\n[3111sub25]\nParameterName=MOD_AsyncReadVal_U32\nObjectType=0x7\nDataType=0x0007\nAccessType=ro\n\n[3111sub26]\nParameterName=MOD_AsyncWriteReg_U32\nObjectType=0x7\nDataType=0x0007\nAccessType=rw\n\n[3111sub27]\nParameterName=MOD_AsyncWriteVal_U32\nObjectType=0x7\nDataType=0x0007\nAccessType=wo\n\n[3111sub5A]\nParameterName=MOD_CfgFunctionMode_U8\nObjectType=0x7\nDataType=0x0005\nAccessType=rw\n\n[3111sub5B]\nParameterName=MOD_CfgEntryCount_U8\nObjectType=0x7\nDataType=0x0005\nAccessType=rw\n\n[3111sub64]\nParameterName=MOD_CfgEntry_00_U64\nObjectType=0x7\nDataType=0x001b\nAccessType=rw\n\n[3111sub65]\nParameterName=MOD_CfgEntry_01_U64\nObjectType=0x7\nDataType=0x001b\nAccessType=rw\n\n[3111sub66]\nParameterName=MOD_CfgEntry_02_U64\nObjectType=0x7\nDataType=0x001b\nAccessType=rw\n\n[3111sub67]\nParameterName=MOD_CfgEntry_03_U64\nObjectType=0x7\nDataType=0x001b\nAccessType=rw\n\n[3111sub68]\nParameterName=MOD_CfgEntry_04_U64\nObjectType=0x7\nDataType=0x001b\nAccessType=rw\n\n[3112]\nParameterName=MOD_Config_xxh_REC\nObjectType=0x9\nSubNumber=36\n\n[3112sub0]\nParameterName=Number of Entries\nObjectType=0x7\nDataType=0x0005\nAccessType=ro\nDefaultValue=0x68\nLowLimit=0x0\nHighLimit=0xFF\n\n[3112sub1]\nParameterName=MOD_ChildCfgIndex_U16\nObjectType=0x7\nDataType=0x0006\nAccessType=rw\n\n[3112sub2]\nParameterName=MOD_ChildCfgCount_U8\nObjectType=0x7\nDataType=0x0005\nAccessType=rw\n\n[3112sub3]\nParameterName=MOD_ChildActCount_U8\nObjectType=0x7\nDataType=0x0005\nAccessType=rw\n\n[3112sub4]\nParameterName=MOD_CfgMode_U8\nObjectType=0x7\nDataType=0x0005\nAccessType=rw\n\n[3112sub5]\nParameterName=MOD_RequestedHardwareId_U16\nObjectType=0x7\nDataType=0x0006\nAccessType=rw\n\n[3112sub6]\nParameterName=MOD_RequestedVendorId_U16\nObjectType=0x7\nDataType=0x0006\nAccessType=rw\n\n[3112sub7]\nParameterName=MOD_HardwareId_U16\nObjectType=0x7\nDataType=0x0006\nAccessType=ro\n\n[3112sub8]\nParameterName=MOD_VendorId_U16\nObjectType=0x7\nDataType=0x0006\nAccessType=ro\n\n[3112sub9]\nParameterName=MOD_InterfaceFlags_U8\nObjectType=0x7\nDataType=0x0005\nAccessType=ro\n\n[3112subA]\nParameterName=MOD_Status_U16\nObjectType=0x7\nDataType=0x0006\nAccessType=rw\n\n[3112subB]\nParameterName=MOD_NetworkStatus_U8\nObjectType=0x7\nDataType=0x0005\nAccessType=ro\n\n[3112subC]\nParameterName=MOD_BlockMask_U8\nObjectType=0x7\nDataType=0x0005\nAccessType=ro\n\n[3112subD]\nParameterName=MOD_BootCount_U8\nObjectType=0x7\nDataType=0x0005\nAccessType=rw\n\n[3112subE]\nParameterName=MOD_LastError_U8\nObjectType=0x7\nDataType=0x0005\nAccessType=rw\n\n[3112sub11]\nParameterName=MOD_FirmwareVersion_U16\nObjectType=0x7\nDataType=0x0006\nAccessType=ro\n\n[3112sub12]\nParameterName=MOD_HardwareVariant_U16\nObjectType=0x7\nDataType=0x0006\nAccessType=ro\n\n[3112sub13]\nParameterName=MOD_SerialNo_U32\nObjectType=0x7\nDataType=0x0007\nAccessType=ro\n\n[3112sub14]\nParameterName=MOD_PhysicalSlotNumber_U8\nObjectType=0x7\nDataType=0x0005\nAccessType=ro\n\n[3112sub15]\nParameterName=MOD_NodeSwitch_U8\nObjectType=0x7\nDataType=0x0005\nAccessType=ro\n\n[3112sub16]\nParameterName=MOD_RequestedSerialNo_U32\nObjectType=0x7\nDataType=0x0007\nAccessType=rw\n\n[3112sub17]\nParameterName=MOD_ModuleErrorReaction_U8\nObjectType=0x7\nDataType=0x0005\nAccessType=rw\n\n[3112sub21]\nParameterName=MOD_AsyncRead_U64\nObjectType=0x7\nDataType=0x001b\nAccessType=rw\n\n[3112sub22]\nParameterName=MOD_AsyncWrite_U64\nObjectType=0x7\nDataType=0x001b\nAccessType=wo\n\n[3112sub23]\nParameterName=MOD_Firmware_DOM\nObjectType=0x7\nDataType=0x000f\nAccessType=wo\n\n[3112sub24]\nParameterName=MOD_AsyncReadReg_U32\nObjectType=0x7\nDataType=0x0007\nAccessType=rw\n\n[3112sub25]\nParameterName=MOD_AsyncReadVal_U32\nObjectType=0x7\nDataType=0x0007\nAccessType=ro\n\n[3112sub26]\nParameterName=MOD_AsyncWriteReg_U32\nObjectType=0x7\nDataType=0x0007\nAccessType=rw\n\n[3112sub27]\nParameterName=MOD_AsyncWriteVal_U32\nObjectType=0x7\nDataType=0x0007\nAccessType=wo\n\n[3112sub5A]\nParameterName=MOD_CfgFunctionMode_U8\nObjectType=0x7\nDataType=0x0005\nAccessType=rw\n\n[3112sub5B]\nParameterName=MOD_CfgEntryCount_U8\nObjectType=0x7\nDataType=0x0005\nAccessType=rw\n\n[3112sub64]\nParameterName=MOD_CfgEntry_00_U64\nObjectType=0x7\nDataType=0x001b\nAccessType=rw\n\n[3112sub65]\nParameterName=MOD_CfgEntry_01_U64\nObjectType=0x7\nDataType=0x001b\nAccessType=rw\n\n[3112sub66]\nParameterName=MOD_CfgEntry_02_U64\nObjectType=0x7\nDataType=0x001b\nAccessType=rw\n\n[3112sub67]\nParameterName=MOD_CfgEntry_03_U64\nObjectType=0x7\nDataType=0x001b\nAccessType=rw\n\n[3112sub68]\nParameterName=MOD_CfgEntry_04_U64\nObjectType=0x7\nDataType=0x001b\nAccessType=rw\n\n[3113]\nParameterName=MOD_Config_xxh_REC\nObjectType=0x9\nSubNumber=36\n\n[3113sub0]\nParameterName=Number of Entries\nObjectType=0x7\nDataType=0x0005\nAccessType=ro\nDefaultValue=0x68\nLowLimit=0x0\nHighLimit=0xFF\n\n[3113sub1]\nParameterName=MOD_ChildCfgIndex_U16\nObjectType=0x7\nDataType=0x0006\nAccessType=rw\n\n[3113sub2]\nParameterName=MOD_ChildCfgCount_U8\nObjectType=0x7\nDataType=0x0005\nAccessType=rw\n\n[3113sub3]\nParameterName=MOD_ChildActCount_U8\nObjectType=0x7\nDataType=0x0005\nAccessType=rw\n\n[3113sub4]\nParameterName=MOD_CfgMode_U8\nObjectType=0x7\nDataType=0x0005\nAccessType=rw\n\n[3113sub5]\nParameterName=MOD_RequestedHardwareId_U16\nObjectType=0x7\nDataType=0x0006\nAccessType=rw\n\n[3113sub6]\nParameterName=MOD_RequestedVendorId_U16\nObjectType=0x7\nDataType=0x0006\nAccessType=rw\n\n[3113sub7]\nParameterName=MOD_HardwareId_U16\nObjectType=0x7\nDataType=0x0006\nAccessType=ro\n\n[3113sub8]\nParameterName=MOD_VendorId_U16\nObjectType=0x7\nDataType=0x0006\nAccessType=ro\n\n[3113sub9]\nParameterName=MOD_InterfaceFlags_U8\nObjectType=0x7\nDataType=0x0005\nAccessType=ro\n\n[3113subA]\nParameterName=MOD_Status_U16\nObjectType=0x7\nDataType=0x0006\nAccessType=rw\n\n[3113subB]\nParameterName=MOD_NetworkStatus_U8\nObjectType=0x7\nDataType=0x0005\nAccessType=ro\n\n[3113subC]\nParameterName=MOD_BlockMask_U8\nObjectType=0x7\nDataType=0x0005\nAccessType=ro\n\n[3113subD]\nParameterName=MOD_BootCount_U8\nObjectType=0x7\nDataType=0x0005\nAccessType=rw\n\n[3113subE]\nParameterName=MOD_LastError_U8\nObjectType=0x7\nDataType=0x0005\nAccessType=rw\n\n[3113sub11]\nParameterName=MOD_FirmwareVersion_U16\nObjectType=0x7\nDataType=0x0006\nAccessType=ro\n\n[3113sub12]\nParameterName=MOD_HardwareVariant_U16\nObjectType=0x7\nDataType=0x0006\nAccessType=ro\n\n[3113sub13]\nParameterName=MOD_SerialNo_U32\nObjectType=0x7\nDataType=0x0007\nAccessType=ro\n\n[3113sub14]\nParameterName=MOD_PhysicalSlotNumber_U8\nObjectType=0x7\nDataType=0x0005\nAccessType=ro\n\n[3113sub15]\nParameterName=MOD_NodeSwitch_U8\nObjectType=0x7\nDataType=0x0005\nAccessType=ro\n\n[3113sub16]\nParameterName=MOD_RequestedSerialNo_U32\nObjectType=0x7\nDataType=0x0007\nAccessType=rw\n\n[3113sub17]\nParameterName=MOD_ModuleErrorReaction_U8\nObjectType=0x7\nDataType=0x0005\nAccessType=rw\n\n[3113sub21]\nParameterName=MOD_AsyncRead_U64\nObjectType=0x7\nDataType=0x001b\nAccessType=rw\n\n[3113sub22]\nParameterName=MOD_AsyncWrite_U64\nObjectType=0x7\nDataType=0x001b\nAccessType=wo\n\n[3113sub23]\nParameterName=MOD_Firmware_DOM\nObjectType=0x7\nDataType=0x000f\nAccessType=wo\n\n[3113sub24]\nParameterName=MOD_AsyncReadReg_U32\nObjectType=0x7\nDataType=0x0007\nAccessType=rw\n\n[3113sub25]\nParameterName=MOD_AsyncReadVal_U32\nObjectType=0x7\nDataType=0x0007\nAccessType=ro\n\n[3113sub26]\nParameterName=MOD_AsyncWriteReg_U32\nObjectType=0x7\nDataType=0x0007\nAccessType=rw\n\n[3113sub27]\nParameterName=MOD_AsyncWriteVal_U32\nObjectType=0x7\nDataType=0x0007\nAccessType=wo\n\n[3113sub5A]\nParameterName=MOD_CfgFunctionMode_U8\nObjectType=0x7\nDataType=0x0005\nAccessType=rw\n\n[3113sub5B]\nParameterName=MOD_CfgEntryCount_U8\nObjectType=0x7\nDataType=0x0005\nAccessType=rw\n\n[3113sub64]\nParameterName=MOD_CfgEntry_00_U64\nObjectType=0x7\nDataType=0x001b\nAccessType=rw\n\n[3113sub65]\nParameterName=MOD_CfgEntry_01_U64\nObjectType=0x7\nDataType=0x001b\nAccessType=rw\n\n[3113sub66]\nParameterName=MOD_CfgEntry_02_U64\nObjectType=0x7\nDataType=0x001b\nAccessType=rw\n\n[3113sub67]\nParameterName=MOD_CfgEntry_03_U64\nObjectType=0x7\nDataType=0x001b\nAccessType=rw\n\n[3113sub68]\nParameterName=MOD_CfgEntry_04_U64\nObjectType=0x7\nDataType=0x001b\nAccessType=rw\n\n[3200]\nParameterName=MOD_DataIn_xxh_AU8\nObjectType=0x8\nSubNumber=11\n\n[3200sub0]\nParameterName=Number of Entries\nObjectType=0x7\nDataType=0x0005\nAccessType=ro\nDefaultValue=0xA\nLowLimit=0x0\nHighLimit=0xFF\n\n[3200sub1]\nParameterName=MOD_DataIn_xxh_AU8[1]\nObjectType=0x7\nDataType=0x0005\nAccessType=rwr\n\n[3200sub2]\nParameterName=MOD_DataIn_xxh_AU8[2]\nObjectType=0x7\nDataType=0x0005\nAccessType=rwr\n\n[3200sub3]\nParameterName=MOD_DataIn_xxh_AU8[3]\nObjectType=0x7\nDataType=0x0005\nAccessType=rwr\n\n[3200sub4]\nParameterName=MOD_DataIn_xxh_AU8[4]\nObjectType=0x7\nDataType=0x0005\nAccessType=rwr\n\n[3200sub5]\nParameterName=MOD_DataIn_xxh_AU8[5]\nObjectType=0x7\nDataType=0x0005\nAccessType=rwr\n\n[3200sub6]\nParameterName=MOD_DataIn_xxh_AU8[6]\nObjectType=0x7\nDataType=0x0005\nAccessType=rwr\n\n[3200sub7]\nParameterName=MOD_DataIn_xxh_AU8[7]\nObjectType=0x7\nDataType=0x0005\nAccessType=rwr\n\n[3200sub8]\nParameterName=MOD_DataIn_xxh_AU8[8]\nObjectType=0x7\nDataType=0x0005\nAccessType=rwr\n\n[3200sub9]\nParameterName=MOD_DataIn_xxh_AU8[9]\nObjectType=0x7\nDataType=0x0005\nAccessType=rwr\n\n[3200subA]\nParameterName=MOD_DataIn_xxh_AU8[10]\nObjectType=0x7\nDataType=0x0005\nAccessType=rwr\n\n[3201]\nParameterName=MOD_DataIn_xxh_AU8\nObjectType=0x8\nSubNumber=11\n\n[3201sub0]\nParameterName=Number of Entries\nObjectType=0x7\nDataType=0x0005\nAccessType=ro\nDefaultValue=0xA\nLowLimit=0x0\nHighLimit=0xFF\n\n[3201sub1]\nParameterName=MOD_DataIn_xxh_AU8[1]\nObjectType=0x7\nDataType=0x0005\nAccessType=rwr\n\n[3201sub2]\nParameterName=MOD_DataIn_xxh_AU8[2]\nObjectType=0x7\nDataType=0x0005\nAccessType=rwr\n\n[3201sub3]\nParameterName=MOD_DataIn_xxh_AU8[3]\nObjectType=0x7\nDataType=0x0005\nAccessType=rwr\n\n[3201sub4]\nParameterName=MOD_DataIn_xxh_AU8[4]\nObjectType=0x7\nDataType=0x0005\nAccessType=rwr\n\n[3201sub5]\nParameterName=MOD_DataIn_xxh_AU8[5]\nObjectType=0x7\nDataType=0x0005\nAccessType=rwr\n\n[3201sub6]\nParameterName=MOD_DataIn_xxh_AU8[6]\nObjectType=0x7\nDataType=0x0005\nAccessType=rwr\n\n[3201sub7]\nParameterName=MOD_DataIn_xxh_AU8[7]\nObjectType=0x7\nDataType=0x0005\nAccessType=rwr\n\n[3201sub8]\nParameterName=MOD_DataIn_xxh_AU8[8]\nObjectType=0x7\nDataType=0x0005\nAccessType=rwr\n\n[3201sub9]\nParameterName=MOD_DataIn_xxh_AU8[9]\nObjectType=0x7\nDataType=0x0005\nAccessType=rwr\n\n[3201subA]\nParameterName=MOD_DataIn_xxh_AU8[10]\nObjectType=0x7\nDataType=0x0005\nAccessType=rwr\n\n[3202]\nParameterName=MOD_DataIn_xxh_AU8\nObjectType=0x8\nSubNumber=11\n\n[3202sub0]\nParameterName=Number of Entries\nObjectType=0x7\nDataType=0x0005\nAccessType=ro\nDefaultValue=0xA\nLowLimit=0x0\nHighLimit=0xFF\n\n[3202sub1]\nParameterName=MOD_DataIn_xxh_AU8[1]\nObjectType=0x7\nDataType=0x0005\nAccessType=rwr\n\n[3202sub2]\nParameterName=MOD_DataIn_xxh_AU8[2]\nObjectType=0x7\nDataType=0x0005\nAccessType=rwr\n\n[3202sub3]\nParameterName=MOD_DataIn_xxh_AU8[3]\nObjectType=0x7\nDataType=0x0005\nAccessType=rwr\n\n[3202sub4]\nParameterName=MOD_DataIn_xxh_AU8[4]\nObjectType=0x7\nDataType=0x0005\nAccessType=rwr\n\n[3202sub5]\nParameterName=MOD_DataIn_xxh_AU8[5]\nObjectType=0x7\nDataType=0x0005\nAccessType=rwr\n\n[3202sub6]\nParameterName=MOD_DataIn_xxh_AU8[6]\nObjectType=0x7\nDataType=0x0005\nAccessType=rwr\n\n[3202sub7]\nParameterName=MOD_DataIn_xxh_AU8[7]\nObjectType=0x7\nDataType=0x0005\nAccessType=rwr\n\n[3202sub8]\nParameterName=MOD_DataIn_xxh_AU8[8]\nObjectType=0x7\nDataType=0x0005\nAccessType=rwr\n\n[3202sub9]\nParameterName=MOD_DataIn_xxh_AU8[9]\nObjectType=0x7\nDataType=0x0005\nAccessType=rwr\n\n[3202subA]\nParameterName=MOD_DataIn_xxh_AU8[10]\nObjectType=0x7\nDataType=0x0005\nAccessType=rwr\n\n[3203]\nParameterName=MOD_DataIn_xxh_AU8\nObjectType=0x8\nSubNumber=11\n\n[3203sub0]\nParameterName=Number of Entries\nObjectType=0x7\nDataType=0x0005\nAccessType=ro\nDefaultValue=0xA\nLowLimit=0x0\nHighLimit=0xFF\n\n[3203sub1]\nParameterName=MOD_DataIn_xxh_AU8[1]\nObjectType=0x7\nDataType=0x0005\nAccessType=rwr\n\n[3203sub2]\nParameterName=MOD_DataIn_xxh_AU8[2]\nObjectType=0x7\nDataType=0x0005\nAccessType=rwr\n\n[3203sub3]\nParameterName=MOD_DataIn_xxh_AU8[3]\nObjectType=0x7\nDataType=0x0005\nAccessType=rwr\n\n[3203sub4]\nParameterName=MOD_DataIn_xxh_AU8[4]\nObjectType=0x7\nDataType=0x0005\nAccessType=rwr\n\n[3203sub5]\nParameterName=MOD_DataIn_xxh_AU8[5]\nObjectType=0x7\nDataType=0x0005\nAccessType=rwr\n\n[3203sub6]\nParameterName=MOD_DataIn_xxh_AU8[6]\nObjectType=0x7\nDataType=0x0005\nAccessType=rwr\n\n[3203sub7]\nParameterName=MOD_DataIn_xxh_AU8[7]\nObjectType=0x7\nDataType=0x0005\nAccessType=rwr\n\n[3203sub8]\nParameterName=MOD_DataIn_xxh_AU8[8]\nObjectType=0x7\nDataType=0x0005\nAccessType=rwr\n\n[3203sub9]\nParameterName=MOD_DataIn_xxh_AU8[9]\nObjectType=0x7\nDataType=0x0005\nAccessType=rwr\n\n[3203subA]\nParameterName=MOD_DataIn_xxh_AU8[10]\nObjectType=0x7\nDataType=0x0005\nAccessType=rwr\n\n[3204]\nParameterName=MOD_DataIn_xxh_AU8\nObjectType=0x8\nSubNumber=11\n\n[3204sub0]\nParameterName=Number of Entries\nObjectType=0x7\nDataType=0x0005\nAccessType=ro\nDefaultValue=0xA\nLowLimit=0x0\nHighLimit=0xFF\n\n[3204sub1]\nParameterName=MOD_DataIn_xxh_AU8[1]\nObjectType=0x7\nDataType=0x0005\nAccessType=rwr\n\n[3204sub2]\nParameterName=MOD_DataIn_xxh_AU8[2]\nObjectType=0x7\nDataType=0x0005\nAccessType=rwr\n\n[3204sub3]\nParameterName=MOD_DataIn_xxh_AU8[3]\nObjectType=0x7\nDataType=0x0005\nAccessType=rwr\n\n[3204sub4]\nParameterName=MOD_DataIn_xxh_AU8[4]\nObjectType=0x7\nDataType=0x0005\nAccessType=rwr\n\n[3204sub5]\nParameterName=MOD_DataIn_xxh_AU8[5]\nObjectType=0x7\nDataType=0x0005\nAccessType=rwr\n\n[3204sub6]\nParameterName=MOD_DataIn_xxh_AU8[6]\nObjectType=0x7\nDataType=0x0005\nAccessType=rwr\n\n[3204sub7]\nParameterName=MOD_DataIn_xxh_AU8[7]\nObjectType=0x7\nDataType=0x0005\nAccessType=rwr\n\n[3204sub8]\nParameterName=MOD_DataIn_xxh_AU8[8]\nObjectType=0x7\nDataType=0x0005\nAccessType=rwr\n\n[3204sub9]\nParameterName=MOD_DataIn_xxh_AU8[9]\nObjectType=0x7\nDataType=0x0005\nAccessType=rwr\n\n[3204subA]\nParameterName=MOD_DataIn_xxh_AU8[10]\nObjectType=0x7\nDataType=0x0005\nAccessType=rwr\n\n[3205]\nParameterName=MOD_DataIn_xxh_AU8\nObjectType=0x8\nSubNumber=11\n\n[3205sub0]\nParameterName=Number of Entries\nObjectType=0x7\nDataType=0x0005\nAccessType=ro\nDefaultValue=0xA\nLowLimit=0x0\nHighLimit=0xFF\n\n[3205sub1]\nParameterName=MOD_DataIn_xxh_AU8[1]\nObjectType=0x7\nDataType=0x0005\nAccessType=rwr\n\n[3205sub2]\nParameterName=MOD_DataIn_xxh_AU8[2]\nObjectType=0x7\nDataType=0x0005\nAccessType=rwr\n\n[3205sub3]\nParameterName=MOD_DataIn_xxh_AU8[3]\nObjectType=0x7\nDataType=0x0005\nAccessType=rwr\n\n[3205sub4]\nParameterName=MOD_DataIn_xxh_AU8[4]\nObjectType=0x7\nDataType=0x0005\nAccessType=rwr\n\n[3205sub5]\nParameterName=MOD_DataIn_xxh_AU8[5]\nObjectType=0x7\nDataType=0x0005\nAccessType=rwr\n\n[3205sub6]\nParameterName=MOD_DataIn_xxh_AU8[6]\nObjectType=0x7\nDataType=0x0005\nAccessType=rwr\n\n[3205sub7]\nParameterName=MOD_DataIn_xxh_AU8[7]\nObjectType=0x7\nDataType=0x0005\nAccessType=rwr\n\n[3205sub8]\nParameterName=MOD_DataIn_xxh_AU8[8]\nObjectType=0x7\nDataType=0x0005\nAccessType=rwr\n\n[3205sub9]\nParameterName=MOD_DataIn_xxh_AU8[9]\nObjectType=0x7\nDataType=0x0005\nAccessType=rwr\n\n[3205subA]\nParameterName=MOD_DataIn_xxh_AU8[10]\nObjectType=0x7\nDataType=0x0005\nAccessType=rwr\n\n[3206]\nParameterName=MOD_DataIn_xxh_AU8\nObjectType=0x8\nSubNumber=11\n\n[3206sub0]\nParameterName=Number of Entries\nObjectType=0x7\nDataType=0x0005\nAccessType=ro\nDefaultValue=0xA\nLowLimit=0x0\nHighLimit=0xFF\n\n[3206sub1]\nParameterName=MOD_DataIn_xxh_AU8[1]\nObjectType=0x7\nDataType=0x0005\nAccessType=rwr\n\n[3206sub2]\nParameterName=MOD_DataIn_xxh_AU8[2]\nObjectType=0x7\nDataType=0x0005\nAccessType=rwr\n\n[3206sub3]\nParameterName=MOD_DataIn_xxh_AU8[3]\nObjectType=0x7\nDataType=0x0005\nAccessType=rwr\n\n[3206sub4]\nParameterName=MOD_DataIn_xxh_AU8[4]\nObjectType=0x7\nDataType=0x0005\nAccessType=rwr\n\n[3206sub5]\nParameterName=MOD_DataIn_xxh_AU8[5]\nObjectType=0x7\nDataType=0x0005\nAccessType=rwr\n\n[3206sub6]\nParameterName=MOD_DataIn_xxh_AU8[6]\nObjectType=0x7\nDataType=0x0005\nAccessType=rwr\n\n[3206sub7]\nParameterName=MOD_DataIn_xxh_AU8[7]\nObjectType=0x7\nDataType=0x0005\nAccessType=rwr\n\n[3206sub8]\nParameterName=MOD_DataIn_xxh_AU8[8]\nObjectType=0x7\nDataType=0x0005\nAccessType=rwr\n\n[3206sub9]\nParameterName=MOD_DataIn_xxh_AU8[9]\nObjectType=0x7\nDataType=0x0005\nAccessType=rwr\n\n[3206subA]\nParameterName=MOD_DataIn_xxh_AU8[10]\nObjectType=0x7\nDataType=0x0005\nAccessType=rwr\n\n[3207]\nParameterName=MOD_DataIn_xxh_AU8\nObjectType=0x8\nSubNumber=11\n\n[3207sub0]\nParameterName=Number of Entries\nObjectType=0x7\nDataType=0x0005\nAccessType=ro\nDefaultValue=0xA\nLowLimit=0x0\nHighLimit=0xFF\n\n[3207sub1]\nParameterName=MOD_DataIn_xxh_AU8[1]\nObjectType=0x7\nDataType=0x0005\nAccessType=rwr\n\n[3207sub2]\nParameterName=MOD_DataIn_xxh_AU8[2]\nObjectType=0x7\nDataType=0x0005\nAccessType=rwr\n\n[3207sub3]\nParameterName=MOD_DataIn_xxh_AU8[3]\nObjectType=0x7\nDataType=0x0005\nAccessType=rwr\n\n[3207sub4]\nParameterName=MOD_DataIn_xxh_AU8[4]\nObjectType=0x7\nDataType=0x0005\nAccessType=rwr\n\n[3207sub5]\nParameterName=MOD_DataIn_xxh_AU8[5]\nObjectType=0x7\nDataType=0x0005\nAccessType=rwr\n\n[3207sub6]\nParameterName=MOD_DataIn_xxh_AU8[6]\nObjectType=0x7\nDataType=0x0005\nAccessType=rwr\n\n[3207sub7]\nParameterName=MOD_DataIn_xxh_AU8[7]\nObjectType=0x7\nDataType=0x0005\nAccessType=rwr\n\n[3207sub8]\nParameterName=MOD_DataIn_xxh_AU8[8]\nObjectType=0x7\nDataType=0x0005\nAccessType=rwr\n\n[3207sub9]\nParameterName=MOD_DataIn_xxh_AU8[9]\nObjectType=0x7\nDataType=0x0005\nAccessType=rwr\n\n[3207subA]\nParameterName=MOD_DataIn_xxh_AU8[10]\nObjectType=0x7\nDataType=0x0005\nAccessType=rwr\n\n[3208]\nParameterName=MOD_DataIn_xxh_AU8\nObjectType=0x8\nSubNumber=11\n\n[3208sub0]\nParameterName=Number of Entries\nObjectType=0x7\nDataType=0x0005\nAccessType=ro\nDefaultValue=0xA\nLowLimit=0x0\nHighLimit=0xFF\n\n[3208sub1]\nParameterName=MOD_DataIn_xxh_AU8[1]\nObjectType=0x7\nDataType=0x0005\nAccessType=rwr\n\n[3208sub2]\nParameterName=MOD_DataIn_xxh_AU8[2]\nObjectType=0x7\nDataType=0x0005\nAccessType=rwr\n\n[3208sub3]\nParameterName=MOD_DataIn_xxh_AU8[3]\nObjectType=0x7\nDataType=0x0005\nAccessType=rwr\n\n[3208sub4]\nParameterName=MOD_DataIn_xxh_AU8[4]\nObjectType=0x7\nDataType=0x0005\nAccessType=rwr\n\n[3208sub5]\nParameterName=MOD_DataIn_xxh_AU8[5]\nObjectType=0x7\nDataType=0x0005\nAccessType=rwr\n\n[3208sub6]\nParameterName=MOD_DataIn_xxh_AU8[6]\nObjectType=0x7\nDataType=0x0005\nAccessType=rwr\n\n[3208sub7]\nParameterName=MOD_DataIn_xxh_AU8[7]\nObjectType=0x7\nDataType=0x0005\nAccessType=rwr\n\n[3208sub8]\nParameterName=MOD_DataIn_xxh_AU8[8]\nObjectType=0x7\nDataType=0x0005\nAccessType=rwr\n\n[3208sub9]\nParameterName=MOD_DataIn_xxh_AU8[9]\nObjectType=0x7\nDataType=0x0005\nAccessType=rwr\n\n[3208subA]\nParameterName=MOD_DataIn_xxh_AU8[10]\nObjectType=0x7\nDataType=0x0005\nAccessType=rwr\n\n[3209]\nParameterName=MOD_DataIn_xxh_AU8\nObjectType=0x8\nSubNumber=11\n\n[3209sub0]\nParameterName=Number of Entries\nObjectType=0x7\nDataType=0x0005\nAccessType=ro\nDefaultValue=0xA\nLowLimit=0x0\nHighLimit=0xFF\n\n[3209sub1]\nParameterName=MOD_DataIn_xxh_AU8[1]\nObjectType=0x7\nDataType=0x0005\nAccessType=rwr\n\n[3209sub2]\nParameterName=MOD_DataIn_xxh_AU8[2]\nObjectType=0x7\nDataType=0x0005\nAccessType=rwr\n\n[3209sub3]\nParameterName=MOD_DataIn_xxh_AU8[3]\nObjectType=0x7\nDataType=0x0005\nAccessType=rwr\n\n[3209sub4]\nParameterName=MOD_DataIn_xxh_AU8[4]\nObjectType=0x7\nDataType=0x0005\nAccessType=rwr\n\n[3209sub5]\nParameterName=MOD_DataIn_xxh_AU8[5]\nObjectType=0x7\nDataType=0x0005\nAccessType=rwr\n\n[3209sub6]\nParameterName=MOD_DataIn_xxh_AU8[6]\nObjectType=0x7\nDataType=0x0005\nAccessType=rwr\n\n[3209sub7]\nParameterName=MOD_DataIn_xxh_AU8[7]\nObjectType=0x7\nDataType=0x0005\nAccessType=rwr\n\n[3209sub8]\nParameterName=MOD_DataIn_xxh_AU8[8]\nObjectType=0x7\nDataType=0x0005\nAccessType=rwr\n\n[3209sub9]\nParameterName=MOD_DataIn_xxh_AU8[9]\nObjectType=0x7\nDataType=0x0005\nAccessType=rwr\n\n[3209subA]\nParameterName=MOD_DataIn_xxh_AU8[10]\nObjectType=0x7\nDataType=0x0005\nAccessType=rwr\n\n[320A]\nParameterName=MOD_DataIn_xxh_AU8\nObjectType=0x8\nSubNumber=11\n\n[320Asub0]\nParameterName=Number of Entries\nObjectType=0x7\nDataType=0x0005\nAccessType=ro\nDefaultValue=0xA\nLowLimit=0x0\nHighLimit=0xFF\n\n[320Asub1]\nParameterName=MOD_DataIn_xxh_AU8[1]\nObjectType=0x7\nDataType=0x0005\nAccessType=rwr\n\n[320Asub2]\nParameterName=MOD_DataIn_xxh_AU8[2]\nObjectType=0x7\nDataType=0x0005\nAccessType=rwr\n\n[320Asub3]\nParameterName=MOD_DataIn_xxh_AU8[3]\nObjectType=0x7\nDataType=0x0005\nAccessType=rwr\n\n[320Asub4]\nParameterName=MOD_DataIn_xxh_AU8[4]\nObjectType=0x7\nDataType=0x0005\nAccessType=rwr\n\n[320Asub5]\nParameterName=MOD_DataIn_xxh_AU8[5]\nObjectType=0x7\nDataType=0x0005\nAccessType=rwr\n\n[320Asub6]\nParameterName=MOD_DataIn_xxh_AU8[6]\nObjectType=0x7\nDataType=0x0005\nAccessType=rwr\n\n[320Asub7]\nParameterName=MOD_DataIn_xxh_AU8[7]\nObjectType=0x7\nDataType=0x0005\nAccessType=rwr\n\n[320Asub8]\nParameterName=MOD_DataIn_xxh_AU8[8]\nObjectType=0x7\nDataType=0x0005\nAccessType=rwr\n\n[320Asub9]\nParameterName=MOD_DataIn_xxh_AU8[9]\nObjectType=0x7\nDataType=0x0005\nAccessType=rwr\n\n[320AsubA]\nParameterName=MOD_DataIn_xxh_AU8[10]\nObjectType=0x7\nDataType=0x0005\nAccessType=rwr\n\n[320B]\nParameterName=MOD_DataIn_xxh_AU8\nObjectType=0x8\nSubNumber=11\n\n[320Bsub0]\nParameterName=Number of Entries\nObjectType=0x7\nDataType=0x0005\nAccessType=ro\nDefaultValue=0xA\nLowLimit=0x0\nHighLimit=0xFF\n\n[320Bsub1]\nParameterName=MOD_DataIn_xxh_AU8[1]\nObjectType=0x7\nDataType=0x0005\nAccessType=rwr\n\n[320Bsub2]\nParameterName=MOD_DataIn_xxh_AU8[2]\nObjectType=0x7\nDataType=0x0005\nAccessType=rwr\n\n[320Bsub3]\nParameterName=MOD_DataIn_xxh_AU8[3]\nObjectType=0x7\nDataType=0x0005\nAccessType=rwr\n\n[320Bsub4]\nParameterName=MOD_DataIn_xxh_AU8[4]\nObjectType=0x7\nDataType=0x0005\nAccessType=rwr\n\n[320Bsub5]\nParameterName=MOD_DataIn_xxh_AU8[5]\nObjectType=0x7\nDataType=0x0005\nAccessType=rwr\n\n[320Bsub6]\nParameterName=MOD_DataIn_xxh_AU8[6]\nObjectType=0x7\nDataType=0x0005\nAccessType=rwr\n\n[320Bsub7]\nParameterName=MOD_DataIn_xxh_AU8[7]\nObjectType=0x7\nDataType=0x0005\nAccessType=rwr\n\n[320Bsub8]\nParameterName=MOD_DataIn_xxh_AU8[8]\nObjectType=0x7\nDataType=0x0005\nAccessType=rwr\n\n[320Bsub9]\nParameterName=MOD_DataIn_xxh_AU8[9]\nObjectType=0x7\nDataType=0x0005\nAccessType=rwr\n\n[320BsubA]\nParameterName=MOD_DataIn_xxh_AU8[10]\nObjectType=0x7\nDataType=0x0005\nAccessType=rwr\n\n[320C]\nParameterName=MOD_DataIn_xxh_AU8\nObjectType=0x8\nSubNumber=11\n\n[320Csub0]\nParameterName=Number of Entries\nObjectType=0x7\nDataType=0x0005\nAccessType=ro\nDefaultValue=0xA\nLowLimit=0x0\nHighLimit=0xFF\n\n[320Csub1]\nParameterName=MOD_DataIn_xxh_AU8[1]\nObjectType=0x7\nDataType=0x0005\nAccessType=rwr\n\n[320Csub2]\nParameterName=MOD_DataIn_xxh_AU8[2]\nObjectType=0x7\nDataType=0x0005\nAccessType=rwr\n\n[320Csub3]\nParameterName=MOD_DataIn_xxh_AU8[3]\nObjectType=0x7\nDataType=0x0005\nAccessType=rwr\n\n[320Csub4]\nParameterName=MOD_DataIn_xxh_AU8[4]\nObjectType=0x7\nDataType=0x0005\nAccessType=rwr\n\n[320Csub5]\nParameterName=MOD_DataIn_xxh_AU8[5]\nObjectType=0x7\nDataType=0x0005\nAccessType=rwr\n\n[320Csub6]\nParameterName=MOD_DataIn_xxh_AU8[6]\nObjectType=0x7\nDataType=0x0005\nAccessType=rwr\n\n[320Csub7]\nParameterName=MOD_DataIn_xxh_AU8[7]\nObjectType=0x7\nDataType=0x0005\nAccessType=rwr\n\n[320Csub8]\nParameterName=MOD_DataIn_xxh_AU8[8]\nObjectType=0x7\nDataType=0x0005\nAccessType=rwr\n\n[320Csub9]\nParameterName=MOD_DataIn_xxh_AU8[9]\nObjectType=0x7\nDataType=0x0005\nAccessType=rwr\n\n[320CsubA]\nParameterName=MOD_DataIn_xxh_AU8[10]\nObjectType=0x7\nDataType=0x0005\nAccessType=rwr\n\n[320D]\nParameterName=MOD_DataIn_xxh_AU8\nObjectType=0x8\nSubNumber=11\n\n[320Dsub0]\nParameterName=Number of Entries\nObjectType=0x7\nDataType=0x0005\nAccessType=ro\nDefaultValue=0xA\nLowLimit=0x0\nHighLimit=0xFF\n\n[320Dsub1]\nParameterName=MOD_DataIn_xxh_AU8[1]\nObjectType=0x7\nDataType=0x0005\nAccessType=rwr\n\n[320Dsub2]\nParameterName=MOD_DataIn_xxh_AU8[2]\nObjectType=0x7\nDataType=0x0005\nAccessType=rwr\n\n[320Dsub3]\nParameterName=MOD_DataIn_xxh_AU8[3]\nObjectType=0x7\nDataType=0x0005\nAccessType=rwr\n\n[320Dsub4]\nParameterName=MOD_DataIn_xxh_AU8[4]\nObjectType=0x7\nDataType=0x0005\nAccessType=rwr\n\n[320Dsub5]\nParameterName=MOD_DataIn_xxh_AU8[5]\nObjectType=0x7\nDataType=0x0005\nAccessType=rwr\n\n[320Dsub6]\nParameterName=MOD_DataIn_xxh_AU8[6]\nObjectType=0x7\nDataType=0x0005\nAccessType=rwr\n\n[320Dsub7]\nParameterName=MOD_DataIn_xxh_AU8[7]\nObjectType=0x7\nDataType=0x0005\nAccessType=rwr\n\n[320Dsub8]\nParameterName=MOD_DataIn_xxh_AU8[8]\nObjectType=0x7\nDataType=0x0005\nAccessType=rwr\n\n[320Dsub9]\nParameterName=MOD_DataIn_xxh_AU8[9]\nObjectType=0x7\nDataType=0x0005\nAccessType=rwr\n\n[320DsubA]\nParameterName=MOD_DataIn_xxh_AU8[10]\nObjectType=0x7\nDataType=0x0005\nAccessType=rwr\n\n[320E]\nParameterName=MOD_DataIn_xxh_AU8\nObjectType=0x8\nSubNumber=11\n\n[320Esub0]\nParameterName=Number of Entries\nObjectType=0x7\nDataType=0x0005\nAccessType=ro\nDefaultValue=0xA\nLowLimit=0x0\nHighLimit=0xFF\n\n[320Esub1]\nParameterName=MOD_DataIn_xxh_AU8[1]\nObjectType=0x7\nDataType=0x0005\nAccessType=rwr\n\n[320Esub2]\nParameterName=MOD_DataIn_xxh_AU8[2]\nObjectType=0x7\nDataType=0x0005\nAccessType=rwr\n\n[320Esub3]\nParameterName=MOD_DataIn_xxh_AU8[3]\nObjectType=0x7\nDataType=0x0005\nAccessType=rwr\n\n[320Esub4]\nParameterName=MOD_DataIn_xxh_AU8[4]\nObjectType=0x7\nDataType=0x0005\nAccessType=rwr\n\n[320Esub5]\nParameterName=MOD_DataIn_xxh_AU8[5]\nObjectType=0x7\nDataType=0x0005\nAccessType=rwr\n\n[320Esub6]\nParameterName=MOD_DataIn_xxh_AU8[6]\nObjectType=0x7\nDataType=0x0005\nAccessType=rwr\n\n[320Esub7]\nParameterName=MOD_DataIn_xxh_AU8[7]\nObjectType=0x7\nDataType=0x0005\nAccessType=rwr\n\n[320Esub8]\nParameterName=MOD_DataIn_xxh_AU8[8]\nObjectType=0x7\nDataType=0x0005\nAccessType=rwr\n\n[320Esub9]\nParameterName=MOD_DataIn_xxh_AU8[9]\nObjectType=0x7\nDataType=0x0005\nAccessType=rwr\n\n[320EsubA]\nParameterName=MOD_DataIn_xxh_AU8[10]\nObjectType=0x7\nDataType=0x0005\nAccessType=rwr\n\n[320F]\nParameterName=MOD_DataIn_xxh_AU8\nObjectType=0x8\nSubNumber=11\n\n[320Fsub0]\nParameterName=Number of Entries\nObjectType=0x7\nDataType=0x0005\nAccessType=ro\nDefaultValue=0xA\nLowLimit=0x0\nHighLimit=0xFF\n\n[320Fsub1]\nParameterName=MOD_DataIn_xxh_AU8[1]\nObjectType=0x7\nDataType=0x0005\nAccessType=rwr\n\n[320Fsub2]\nParameterName=MOD_DataIn_xxh_AU8[2]\nObjectType=0x7\nDataType=0x0005\nAccessType=rwr\n\n[320Fsub3]\nParameterName=MOD_DataIn_xxh_AU8[3]\nObjectType=0x7\nDataType=0x0005\nAccessType=rwr\n\n[320Fsub4]\nParameterName=MOD_DataIn_xxh_AU8[4]\nObjectType=0x7\nDataType=0x0005\nAccessType=rwr\n\n[320Fsub5]\nParameterName=MOD_DataIn_xxh_AU8[5]\nObjectType=0x7\nDataType=0x0005\nAccessType=rwr\n\n[320Fsub6]\nParameterName=MOD_DataIn_xxh_AU8[6]\nObjectType=0x7\nDataType=0x0005\nAccessType=rwr\n\n[320Fsub7]\nParameterName=MOD_DataIn_xxh_AU8[7]\nObjectType=0x7\nDataType=0x0005\nAccessType=rwr\n\n[320Fsub8]\nParameterName=MOD_DataIn_xxh_AU8[8]\nObjectType=0x7\nDataType=0x0005\nAccessType=rwr\n\n[320Fsub9]\nParameterName=MOD_DataIn_xxh_AU8[9]\nObjectType=0x7\nDataType=0x0005\nAccessType=rwr\n\n[320FsubA]\nParameterName=MOD_DataIn_xxh_AU8[10]\nObjectType=0x7\nDataType=0x0005\nAccessType=rwr\n\n[3210]\nParameterName=MOD_DataIn_xxh_AU8\nObjectType=0x8\nSubNumber=11\n\n[3210sub0]\nParameterName=Number of Entries\nObjectType=0x7\nDataType=0x0005\nAccessType=ro\nDefaultValue=0xA\nLowLimit=0x0\nHighLimit=0xFF\n\n[3210sub1]\nParameterName=MOD_DataIn_xxh_AU8[1]\nObjectType=0x7\nDataType=0x0005\nAccessType=rwr\n\n[3210sub2]\nParameterName=MOD_DataIn_xxh_AU8[2]\nObjectType=0x7\nDataType=0x0005\nAccessType=rwr\n\n[3210sub3]\nParameterName=MOD_DataIn_xxh_AU8[3]\nObjectType=0x7\nDataType=0x0005\nAccessType=rwr\n\n[3210sub4]\nParameterName=MOD_DataIn_xxh_AU8[4]\nObjectType=0x7\nDataType=0x0005\nAccessType=rwr\n\n[3210sub5]\nParameterName=MOD_DataIn_xxh_AU8[5]\nObjectType=0x7\nDataType=0x0005\nAccessType=rwr\n\n[3210sub6]\nParameterName=MOD_DataIn_xxh_AU8[6]\nObjectType=0x7\nDataType=0x0005\nAccessType=rwr\n\n[3210sub7]\nParameterName=MOD_DataIn_xxh_AU8[7]\nObjectType=0x7\nDataType=0x0005\nAccessType=rwr\n\n[3210sub8]\nParameterName=MOD_DataIn_xxh_AU8[8]\nObjectType=0x7\nDataType=0x0005\nAccessType=rwr\n\n[3210sub9]\nParameterName=MOD_DataIn_xxh_AU8[9]\nObjectType=0x7\nDataType=0x0005\nAccessType=rwr\n\n[3210subA]\nParameterName=MOD_DataIn_xxh_AU8[10]\nObjectType=0x7\nDataType=0x0005\nAccessType=rwr\n\n[3211]\nParameterName=MOD_DataIn_xxh_AU8\nObjectType=0x8\nSubNumber=11\n\n[3211sub0]\nParameterName=Number of Entries\nObjectType=0x7\nDataType=0x0005\nAccessType=ro\nDefaultValue=0xA\nLowLimit=0x0\nHighLimit=0xFF\n\n[3211sub1]\nParameterName=MOD_DataIn_xxh_AU8[1]\nObjectType=0x7\nDataType=0x0005\nAccessType=rwr\n\n[3211sub2]\nParameterName=MOD_DataIn_xxh_AU8[2]\nObjectType=0x7\nDataType=0x0005\nAccessType=rwr\n\n[3211sub3]\nParameterName=MOD_DataIn_xxh_AU8[3]\nObjectType=0x7\nDataType=0x0005\nAccessType=rwr\n\n[3211sub4]\nParameterName=MOD_DataIn_xxh_AU8[4]\nObjectType=0x7\nDataType=0x0005\nAccessType=rwr\n\n[3211sub5]\nParameterName=MOD_DataIn_xxh_AU8[5]\nObjectType=0x7\nDataType=0x0005\nAccessType=rwr\n\n[3211sub6]\nParameterName=MOD_DataIn_xxh_AU8[6]\nObjectType=0x7\nDataType=0x0005\nAccessType=rwr\n\n[3211sub7]\nParameterName=MOD_DataIn_xxh_AU8[7]\nObjectType=0x7\nDataType=0x0005\nAccessType=rwr\n\n[3211sub8]\nParameterName=MOD_DataIn_xxh_AU8[8]\nObjectType=0x7\nDataType=0x0005\nAccessType=rwr\n\n[3211sub9]\nParameterName=MOD_DataIn_xxh_AU8[9]\nObjectType=0x7\nDataType=0x0005\nAccessType=rwr\n\n[3211subA]\nParameterName=MOD_DataIn_xxh_AU8[10]\nObjectType=0x7\nDataType=0x0005\nAccessType=rwr\n\n[3212]\nParameterName=MOD_DataIn_xxh_AU8\nObjectType=0x8\nSubNumber=11\n\n[3212sub0]\nParameterName=Number of Entries\nObjectType=0x7\nDataType=0x0005\nAccessType=ro\nDefaultValue=0xA\nLowLimit=0x0\nHighLimit=0xFF\n\n[3212sub1]\nParameterName=MOD_DataIn_xxh_AU8[1]\nObjectType=0x7\nDataType=0x0005\nAccessType=rwr\n\n[3212sub2]\nParameterName=MOD_DataIn_xxh_AU8[2]\nObjectType=0x7\nDataType=0x0005\nAccessType=rwr\n\n[3212sub3]\nParameterName=MOD_DataIn_xxh_AU8[3]\nObjectType=0x7\nDataType=0x0005\nAccessType=rwr\n\n[3212sub4]\nParameterName=MOD_DataIn_xxh_AU8[4]\nObjectType=0x7\nDataType=0x0005\nAccessType=rwr\n\n[3212sub5]\nParameterName=MOD_DataIn_xxh_AU8[5]\nObjectType=0x7\nDataType=0x0005\nAccessType=rwr\n\n[3212sub6]\nParameterName=MOD_DataIn_xxh_AU8[6]\nObjectType=0x7\nDataType=0x0005\nAccessType=rwr\n\n[3212sub7]\nParameterName=MOD_DataIn_xxh_AU8[7]\nObjectType=0x7\nDataType=0x0005\nAccessType=rwr\n\n[3212sub8]\nParameterName=MOD_DataIn_xxh_AU8[8]\nObjectType=0x7\nDataType=0x0005\nAccessType=rwr\n\n[3212sub9]\nParameterName=MOD_DataIn_xxh_AU8[9]\nObjectType=0x7\nDataType=0x0005\nAccessType=rwr\n\n[3212subA]\nParameterName=MOD_DataIn_xxh_AU8[10]\nObjectType=0x7\nDataType=0x0005\nAccessType=rwr\n\n[3213]\nParameterName=MOD_DataIn_xxh_AU8\nObjectType=0x8\nSubNumber=11\n\n[3213sub0]\nParameterName=Number of Entries\nObjectType=0x7\nDataType=0x0005\nAccessType=ro\nDefaultValue=0xA\nLowLimit=0x0\nHighLimit=0xFF\n\n[3213sub1]\nParameterName=MOD_DataIn_xxh_AU8[1]\nObjectType=0x7\nDataType=0x0005\nAccessType=rwr\n\n[3213sub2]\nParameterName=MOD_DataIn_xxh_AU8[2]\nObjectType=0x7\nDataType=0x0005\nAccessType=rwr\n\n[3213sub3]\nParameterName=MOD_DataIn_xxh_AU8[3]\nObjectType=0x7\nDataType=0x0005\nAccessType=rwr\n\n[3213sub4]\nParameterName=MOD_DataIn_xxh_AU8[4]\nObjectType=0x7\nDataType=0x0005\nAccessType=rwr\n\n[3213sub5]\nParameterName=MOD_DataIn_xxh_AU8[5]\nObjectType=0x7\nDataType=0x0005\nAccessType=rwr\n\n[3213sub6]\nParameterName=MOD_DataIn_xxh_AU8[6]\nObjectType=0x7\nDataType=0x0005\nAccessType=rwr\n\n[3213sub7]\nParameterName=MOD_DataIn_xxh_AU8[7]\nObjectType=0x7\nDataType=0x0005\nAccessType=rwr\n\n[3213sub8]\nParameterName=MOD_DataIn_xxh_AU8[8]\nObjectType=0x7\nDataType=0x0005\nAccessType=rwr\n\n[3213sub9]\nParameterName=MOD_DataIn_xxh_AU8[9]\nObjectType=0x7\nDataType=0x0005\nAccessType=rwr\n\n[3213subA]\nParameterName=MOD_DataIn_xxh_AU8[10]\nObjectType=0x7\nDataType=0x0005\nAccessType=rwr\n\n[3300]\nParameterName=MOD_DataIn_xxh_AU16\nObjectType=0x8\nSubNumber=11\n\n[3300sub0]\nParameterName=Number of Entries\nObjectType=0x7\nDataType=0x0005\nAccessType=ro\nDefaultValue=0xA\nLowLimit=0x0\nHighLimit=0xFF\n\n[3300sub1]\nParameterName=MOD_DataIn_xxh_AU16[1]\nObjectType=0x7\nDataType=0x0006\nAccessType=rwr\n\n[3300sub2]\nParameterName=MOD_DataIn_xxh_AU16[2]\nObjectType=0x7\nDataType=0x0006\nAccessType=rwr\n\n[3300sub3]\nParameterName=MOD_DataIn_xxh_AU16[3]\nObjectType=0x7\nDataType=0x0006\nAccessType=rwr\n\n[3300sub4]\nParameterName=MOD_DataIn_xxh_AU16[4]\nObjectType=0x7\nDataType=0x0006\nAccessType=rwr\n\n[3300sub5]\nParameterName=MOD_DataIn_xxh_AU16[5]\nObjectType=0x7\nDataType=0x0006\nAccessType=rwr\n\n[3300sub6]\nParameterName=MOD_DataIn_xxh_AU16[6]\nObjectType=0x7\nDataType=0x0006\nAccessType=rwr\n\n[3300sub7]\nParameterName=MOD_DataIn_xxh_AU16[7]\nObjectType=0x7\nDataType=0x0006\nAccessType=rwr\n\n[3300sub8]\nParameterName=MOD_DataIn_xxh_AU16[8]\nObjectType=0x7\nDataType=0x0006\nAccessType=rwr\n\n[3300sub9]\nParameterName=MOD_DataIn_xxh_AU16[9]\nObjectType=0x7\nDataType=0x0006\nAccessType=rwr\n\n[3300subA]\nParameterName=MOD_DataIn_xxh_AU16[10]\nObjectType=0x7\nDataType=0x0006\nAccessType=rwr\n\n[3301]\nParameterName=MOD_DataIn_xxh_AU16\nObjectType=0x8\nSubNumber=11\n\n[3301sub0]\nParameterName=Number of Entries\nObjectType=0x7\nDataType=0x0005\nAccessType=ro\nDefaultValue=0xA\nLowLimit=0x0\nHighLimit=0xFF\n\n[3301sub1]\nParameterName=MOD_DataIn_xxh_AU16[1]\nObjectType=0x7\nDataType=0x0006\nAccessType=rwr\n\n[3301sub2]\nParameterName=MOD_DataIn_xxh_AU16[2]\nObjectType=0x7\nDataType=0x0006\nAccessType=rwr\n\n[3301sub3]\nParameterName=MOD_DataIn_xxh_AU16[3]\nObjectType=0x7\nDataType=0x0006\nAccessType=rwr\n\n[3301sub4]\nParameterName=MOD_DataIn_xxh_AU16[4]\nObjectType=0x7\nDataType=0x0006\nAccessType=rwr\n\n[3301sub5]\nParameterName=MOD_DataIn_xxh_AU16[5]\nObjectType=0x7\nDataType=0x0006\nAccessType=rwr\n\n[3301sub6]\nParameterName=MOD_DataIn_xxh_AU16[6]\nObjectType=0x7\nDataType=0x0006\nAccessType=rwr\n\n[3301sub7]\nParameterName=MOD_DataIn_xxh_AU16[7]\nObjectType=0x7\nDataType=0x0006\nAccessType=rwr\n\n[3301sub8]\nParameterName=MOD_DataIn_xxh_AU16[8]\nObjectType=0x7\nDataType=0x0006\nAccessType=rwr\n\n[3301sub9]\nParameterName=MOD_DataIn_xxh_AU16[9]\nObjectType=0x7\nDataType=0x0006\nAccessType=rwr\n\n[3301subA]\nParameterName=MOD_DataIn_xxh_AU16[10]\nObjectType=0x7\nDataType=0x0006\nAccessType=rwr\n\n[3302]\nParameterName=MOD_DataIn_xxh_AU16\nObjectType=0x8\nSubNumber=11\n\n[3302sub0]\nParameterName=Number of Entries\nObjectType=0x7\nDataType=0x0005\nAccessType=ro\nDefaultValue=0xA\nLowLimit=0x0\nHighLimit=0xFF\n\n[3302sub1]\nParameterName=MOD_DataIn_xxh_AU16[1]\nObjectType=0x7\nDataType=0x0006\nAccessType=rwr\n\n[3302sub2]\nParameterName=MOD_DataIn_xxh_AU16[2]\nObjectType=0x7\nDataType=0x0006\nAccessType=rwr\n\n[3302sub3]\nParameterName=MOD_DataIn_xxh_AU16[3]\nObjectType=0x7\nDataType=0x0006\nAccessType=rwr\n\n[3302sub4]\nParameterName=MOD_DataIn_xxh_AU16[4]\nObjectType=0x7\nDataType=0x0006\nAccessType=rwr\n\n[3302sub5]\nParameterName=MOD_DataIn_xxh_AU16[5]\nObjectType=0x7\nDataType=0x0006\nAccessType=rwr\n\n[3302sub6]\nParameterName=MOD_DataIn_xxh_AU16[6]\nObjectType=0x7\nDataType=0x0006\nAccessType=rwr\n\n[3302sub7]\nParameterName=MOD_DataIn_xxh_AU16[7]\nObjectType=0x7\nDataType=0x0006\nAccessType=rwr\n\n[3302sub8]\nParameterName=MOD_DataIn_xxh_AU16[8]\nObjectType=0x7\nDataType=0x0006\nAccessType=rwr\n\n[3302sub9]\nParameterName=MOD_DataIn_xxh_AU16[9]\nObjectType=0x7\nDataType=0x0006\nAccessType=rwr\n\n[3302subA]\nParameterName=MOD_DataIn_xxh_AU16[10]\nObjectType=0x7\nDataType=0x0006\nAccessType=rwr\n\n[3303]\nParameterName=MOD_DataIn_xxh_AU16\nObjectType=0x8\nSubNumber=11\n\n[3303sub0]\nParameterName=Number of Entries\nObjectType=0x7\nDataType=0x0005\nAccessType=ro\nDefaultValue=0xA\nLowLimit=0x0\nHighLimit=0xFF\n\n[3303sub1]\nParameterName=MOD_DataIn_xxh_AU16[1]\nObjectType=0x7\nDataType=0x0006\nAccessType=rwr\n\n[3303sub2]\nParameterName=MOD_DataIn_xxh_AU16[2]\nObjectType=0x7\nDataType=0x0006\nAccessType=rwr\n\n[3303sub3]\nParameterName=MOD_DataIn_xxh_AU16[3]\nObjectType=0x7\nDataType=0x0006\nAccessType=rwr\n\n[3303sub4]\nParameterName=MOD_DataIn_xxh_AU16[4]\nObjectType=0x7\nDataType=0x0006\nAccessType=rwr\n\n[3303sub5]\nParameterName=MOD_DataIn_xxh_AU16[5]\nObjectType=0x7\nDataType=0x0006\nAccessType=rwr\n\n[3303sub6]\nParameterName=MOD_DataIn_xxh_AU16[6]\nObjectType=0x7\nDataType=0x0006\nAccessType=rwr\n\n[3303sub7]\nParameterName=MOD_DataIn_xxh_AU16[7]\nObjectType=0x7\nDataType=0x0006\nAccessType=rwr\n\n[3303sub8]\nParameterName=MOD_DataIn_xxh_AU16[8]\nObjectType=0x7\nDataType=0x0006\nAccessType=rwr\n\n[3303sub9]\nParameterName=MOD_DataIn_xxh_AU16[9]\nObjectType=0x7\nDataType=0x0006\nAccessType=rwr\n\n[3303subA]\nParameterName=MOD_DataIn_xxh_AU16[10]\nObjectType=0x7\nDataType=0x0006\nAccessType=rwr\n\n[3304]\nParameterName=MOD_DataIn_xxh_AU16\nObjectType=0x8\nSubNumber=11\n\n[3304sub0]\nParameterName=Number of Entries\nObjectType=0x7\nDataType=0x0005\nAccessType=ro\nDefaultValue=0xA\nLowLimit=0x0\nHighLimit=0xFF\n\n[3304sub1]\nParameterName=MOD_DataIn_xxh_AU16[1]\nObjectType=0x7\nDataType=0x0006\nAccessType=rwr\n\n[3304sub2]\nParameterName=MOD_DataIn_xxh_AU16[2]\nObjectType=0x7\nDataType=0x0006\nAccessType=rwr\n\n[3304sub3]\nParameterName=MOD_DataIn_xxh_AU16[3]\nObjectType=0x7\nDataType=0x0006\nAccessType=rwr\n\n[3304sub4]\nParameterName=MOD_DataIn_xxh_AU16[4]\nObjectType=0x7\nDataType=0x0006\nAccessType=rwr\n\n[3304sub5]\nParameterName=MOD_DataIn_xxh_AU16[5]\nObjectType=0x7\nDataType=0x0006\nAccessType=rwr\n\n[3304sub6]\nParameterName=MOD_DataIn_xxh_AU16[6]\nObjectType=0x7\nDataType=0x0006\nAccessType=rwr\n\n[3304sub7]\nParameterName=MOD_DataIn_xxh_AU16[7]\nObjectType=0x7\nDataType=0x0006\nAccessType=rwr\n\n[3304sub8]\nParameterName=MOD_DataIn_xxh_AU16[8]\nObjectType=0x7\nDataType=0x0006\nAccessType=rwr\n\n[3304sub9]\nParameterName=MOD_DataIn_xxh_AU16[9]\nObjectType=0x7\nDataType=0x0006\nAccessType=rwr\n\n[3304subA]\nParameterName=MOD_DataIn_xxh_AU16[10]\nObjectType=0x7\nDataType=0x0006\nAccessType=rwr\n\n[3305]\nParameterName=MOD_DataIn_xxh_AU16\nObjectType=0x8\nSubNumber=11\n\n[3305sub0]\nParameterName=Number of Entries\nObjectType=0x7\nDataType=0x0005\nAccessType=ro\nDefaultValue=0xA\nLowLimit=0x0\nHighLimit=0xFF\n\n[3305sub1]\nParameterName=MOD_DataIn_xxh_AU16[1]\nObjectType=0x7\nDataType=0x0006\nAccessType=rwr\n\n[3305sub2]\nParameterName=MOD_DataIn_xxh_AU16[2]\nObjectType=0x7\nDataType=0x0006\nAccessType=rwr\n\n[3305sub3]\nParameterName=MOD_DataIn_xxh_AU16[3]\nObjectType=0x7\nDataType=0x0006\nAccessType=rwr\n\n[3305sub4]\nParameterName=MOD_DataIn_xxh_AU16[4]\nObjectType=0x7\nDataType=0x0006\nAccessType=rwr\n\n[3305sub5]\nParameterName=MOD_DataIn_xxh_AU16[5]\nObjectType=0x7\nDataType=0x0006\nAccessType=rwr\n\n[3305sub6]\nParameterName=MOD_DataIn_xxh_AU16[6]\nObjectType=0x7\nDataType=0x0006\nAccessType=rwr\n\n[3305sub7]\nParameterName=MOD_DataIn_xxh_AU16[7]\nObjectType=0x7\nDataType=0x0006\nAccessType=rwr\n\n[3305sub8]\nParameterName=MOD_DataIn_xxh_AU16[8]\nObjectType=0x7\nDataType=0x0006\nAccessType=rwr\n\n[3305sub9]\nParameterName=MOD_DataIn_xxh_AU16[9]\nObjectType=0x7\nDataType=0x0006\nAccessType=rwr\n\n[3305subA]\nParameterName=MOD_DataIn_xxh_AU16[10]\nObjectType=0x7\nDataType=0x0006\nAccessType=rwr\n\n[3306]\nParameterName=MOD_DataIn_xxh_AU16\nObjectType=0x8\nSubNumber=11\n\n[3306sub0]\nParameterName=Number of Entries\nObjectType=0x7\nDataType=0x0005\nAccessType=ro\nDefaultValue=0xA\nLowLimit=0x0\nHighLimit=0xFF\n\n[3306sub1]\nParameterName=MOD_DataIn_xxh_AU16[1]\nObjectType=0x7\nDataType=0x0006\nAccessType=rwr\n\n[3306sub2]\nParameterName=MOD_DataIn_xxh_AU16[2]\nObjectType=0x7\nDataType=0x0006\nAccessType=rwr\n\n[3306sub3]\nParameterName=MOD_DataIn_xxh_AU16[3]\nObjectType=0x7\nDataType=0x0006\nAccessType=rwr\n\n[3306sub4]\nParameterName=MOD_DataIn_xxh_AU16[4]\nObjectType=0x7\nDataType=0x0006\nAccessType=rwr\n\n[3306sub5]\nParameterName=MOD_DataIn_xxh_AU16[5]\nObjectType=0x7\nDataType=0x0006\nAccessType=rwr\n\n[3306sub6]\nParameterName=MOD_DataIn_xxh_AU16[6]\nObjectType=0x7\nDataType=0x0006\nAccessType=rwr\n\n[3306sub7]\nParameterName=MOD_DataIn_xxh_AU16[7]\nObjectType=0x7\nDataType=0x0006\nAccessType=rwr\n\n[3306sub8]\nParameterName=MOD_DataIn_xxh_AU16[8]\nObjectType=0x7\nDataType=0x0006\nAccessType=rwr\n\n[3306sub9]\nParameterName=MOD_DataIn_xxh_AU16[9]\nObjectType=0x7\nDataType=0x0006\nAccessType=rwr\n\n[3306subA]\nParameterName=MOD_DataIn_xxh_AU16[10]\nObjectType=0x7\nDataType=0x0006\nAccessType=rwr\n\n[3307]\nParameterName=MOD_DataIn_xxh_AU16\nObjectType=0x8\nSubNumber=11\n\n[3307sub0]\nParameterName=Number of Entries\nObjectType=0x7\nDataType=0x0005\nAccessType=ro\nDefaultValue=0xA\nLowLimit=0x0\nHighLimit=0xFF\n\n[3307sub1]\nParameterName=MOD_DataIn_xxh_AU16[1]\nObjectType=0x7\nDataType=0x0006\nAccessType=rwr\n\n[3307sub2]\nParameterName=MOD_DataIn_xxh_AU16[2]\nObjectType=0x7\nDataType=0x0006\nAccessType=rwr\n\n[3307sub3]\nParameterName=MOD_DataIn_xxh_AU16[3]\nObjectType=0x7\nDataType=0x0006\nAccessType=rwr\n\n[3307sub4]\nParameterName=MOD_DataIn_xxh_AU16[4]\nObjectType=0x7\nDataType=0x0006\nAccessType=rwr\n\n[3307sub5]\nParameterName=MOD_DataIn_xxh_AU16[5]\nObjectType=0x7\nDataType=0x0006\nAccessType=rwr\n\n[3307sub6]\nParameterName=MOD_DataIn_xxh_AU16[6]\nObjectType=0x7\nDataType=0x0006\nAccessType=rwr\n\n[3307sub7]\nParameterName=MOD_DataIn_xxh_AU16[7]\nObjectType=0x7\nDataType=0x0006\nAccessType=rwr\n\n[3307sub8]\nParameterName=MOD_DataIn_xxh_AU16[8]\nObjectType=0x7\nDataType=0x0006\nAccessType=rwr\n\n[3307sub9]\nParameterName=MOD_DataIn_xxh_AU16[9]\nObjectType=0x7\nDataType=0x0006\nAccessType=rwr\n\n[3307subA]\nParameterName=MOD_DataIn_xxh_AU16[10]\nObjectType=0x7\nDataType=0x0006\nAccessType=rwr\n\n[3308]\nParameterName=MOD_DataIn_xxh_AU16\nObjectType=0x8\nSubNumber=11\n\n[3308sub0]\nParameterName=Number of Entries\nObjectType=0x7\nDataType=0x0005\nAccessType=ro\nDefaultValue=0xA\nLowLimit=0x0\nHighLimit=0xFF\n\n[3308sub1]\nParameterName=MOD_DataIn_xxh_AU16[1]\nObjectType=0x7\nDataType=0x0006\nAccessType=rwr\n\n[3308sub2]\nParameterName=MOD_DataIn_xxh_AU16[2]\nObjectType=0x7\nDataType=0x0006\nAccessType=rwr\n\n[3308sub3]\nParameterName=MOD_DataIn_xxh_AU16[3]\nObjectType=0x7\nDataType=0x0006\nAccessType=rwr\n\n[3308sub4]\nParameterName=MOD_DataIn_xxh_AU16[4]\nObjectType=0x7\nDataType=0x0006\nAccessType=rwr\n\n[3308sub5]\nParameterName=MOD_DataIn_xxh_AU16[5]\nObjectType=0x7\nDataType=0x0006\nAccessType=rwr\n\n[3308sub6]\nParameterName=MOD_DataIn_xxh_AU16[6]\nObjectType=0x7\nDataType=0x0006\nAccessType=rwr\n\n[3308sub7]\nParameterName=MOD_DataIn_xxh_AU16[7]\nObjectType=0x7\nDataType=0x0006\nAccessType=rwr\n\n[3308sub8]\nParameterName=MOD_DataIn_xxh_AU16[8]\nObjectType=0x7\nDataType=0x0006\nAccessType=rwr\n\n[3308sub9]\nParameterName=MOD_DataIn_xxh_AU16[9]\nObjectType=0x7\nDataType=0x0006\nAccessType=rwr\n\n[3308subA]\nParameterName=MOD_DataIn_xxh_AU16[10]\nObjectType=0x7\nDataType=0x0006\nAccessType=rwr\n\n[3309]\nParameterName=MOD_DataIn_xxh_AU16\nObjectType=0x8\nSubNumber=11\n\n[3309sub0]\nParameterName=Number of Entries\nObjectType=0x7\nDataType=0x0005\nAccessType=ro\nDefaultValue=0xA\nLowLimit=0x0\nHighLimit=0xFF\n\n[3309sub1]\nParameterName=MOD_DataIn_xxh_AU16[1]\nObjectType=0x7\nDataType=0x0006\nAccessType=rwr\n\n[3309sub2]\nParameterName=MOD_DataIn_xxh_AU16[2]\nObjectType=0x7\nDataType=0x0006\nAccessType=rwr\n\n[3309sub3]\nParameterName=MOD_DataIn_xxh_AU16[3]\nObjectType=0x7\nDataType=0x0006\nAccessType=rwr\n\n[3309sub4]\nParameterName=MOD_DataIn_xxh_AU16[4]\nObjectType=0x7\nDataType=0x0006\nAccessType=rwr\n\n[3309sub5]\nParameterName=MOD_DataIn_xxh_AU16[5]\nObjectType=0x7\nDataType=0x0006\nAccessType=rwr\n\n[3309sub6]\nParameterName=MOD_DataIn_xxh_AU16[6]\nObjectType=0x7\nDataType=0x0006\nAccessType=rwr\n\n[3309sub7]\nParameterName=MOD_DataIn_xxh_AU16[7]\nObjectType=0x7\nDataType=0x0006\nAccessType=rwr\n\n[3309sub8]\nParameterName=MOD_DataIn_xxh_AU16[8]\nObjectType=0x7\nDataType=0x0006\nAccessType=rwr\n\n[3309sub9]\nParameterName=MOD_DataIn_xxh_AU16[9]\nObjectType=0x7\nDataType=0x0006\nAccessType=rwr\n\n[3309subA]\nParameterName=MOD_DataIn_xxh_AU16[10]\nObjectType=0x7\nDataType=0x0006\nAccessType=rwr\n\n[330A]\nParameterName=MOD_DataIn_xxh_AU16\nObjectType=0x8\nSubNumber=11\n\n[330Asub0]\nParameterName=Number of Entries\nObjectType=0x7\nDataType=0x0005\nAccessType=ro\nDefaultValue=0xA\nLowLimit=0x0\nHighLimit=0xFF\n\n[330Asub1]\nParameterName=MOD_DataIn_xxh_AU16[1]\nObjectType=0x7\nDataType=0x0006\nAccessType=rwr\n\n[330Asub2]\nParameterName=MOD_DataIn_xxh_AU16[2]\nObjectType=0x7\nDataType=0x0006\nAccessType=rwr\n\n[330Asub3]\nParameterName=MOD_DataIn_xxh_AU16[3]\nObjectType=0x7\nDataType=0x0006\nAccessType=rwr\n\n[330Asub4]\nParameterName=MOD_DataIn_xxh_AU16[4]\nObjectType=0x7\nDataType=0x0006\nAccessType=rwr\n\n[330Asub5]\nParameterName=MOD_DataIn_xxh_AU16[5]\nObjectType=0x7\nDataType=0x0006\nAccessType=rwr\n\n[330Asub6]\nParameterName=MOD_DataIn_xxh_AU16[6]\nObjectType=0x7\nDataType=0x0006\nAccessType=rwr\n\n[330Asub7]\nParameterName=MOD_DataIn_xxh_AU16[7]\nObjectType=0x7\nDataType=0x0006\nAccessType=rwr\n\n[330Asub8]\nParameterName=MOD_DataIn_xxh_AU16[8]\nObjectType=0x7\nDataType=0x0006\nAccessType=rwr\n\n[330Asub9]\nParameterName=MOD_DataIn_xxh_AU16[9]\nObjectType=0x7\nDataType=0x0006\nAccessType=rwr\n\n[330AsubA]\nParameterName=MOD_DataIn_xxh_AU16[10]\nObjectType=0x7\nDataType=0x0006\nAccessType=rwr\n\n[330B]\nParameterName=MOD_DataIn_xxh_AU16\nObjectType=0x8\nSubNumber=11\n\n[330Bsub0]\nParameterName=Number of Entries\nObjectType=0x7\nDataType=0x0005\nAccessType=ro\nDefaultValue=0xA\nLowLimit=0x0\nHighLimit=0xFF\n\n[330Bsub1]\nParameterName=MOD_DataIn_xxh_AU16[1]\nObjectType=0x7\nDataType=0x0006\nAccessType=rwr\n\n[330Bsub2]\nParameterName=MOD_DataIn_xxh_AU16[2]\nObjectType=0x7\nDataType=0x0006\nAccessType=rwr\n\n[330Bsub3]\nParameterName=MOD_DataIn_xxh_AU16[3]\nObjectType=0x7\nDataType=0x0006\nAccessType=rwr\n\n[330Bsub4]\nParameterName=MOD_DataIn_xxh_AU16[4]\nObjectType=0x7\nDataType=0x0006\nAccessType=rwr\n\n[330Bsub5]\nParameterName=MOD_DataIn_xxh_AU16[5]\nObjectType=0x7\nDataType=0x0006\nAccessType=rwr\n\n[330Bsub6]\nParameterName=MOD_DataIn_xxh_AU16[6]\nObjectType=0x7\nDataType=0x0006\nAccessType=rwr\n\n[330Bsub7]\nParameterName=MOD_DataIn_xxh_AU16[7]\nObjectType=0x7\nDataType=0x0006\nAccessType=rwr\n\n[330Bsub8]\nParameterName=MOD_DataIn_xxh_AU16[8]\nObjectType=0x7\nDataType=0x0006\nAccessType=rwr\n\n[330Bsub9]\nParameterName=MOD_DataIn_xxh_AU16[9]\nObjectType=0x7\nDataType=0x0006\nAccessType=rwr\n\n[330BsubA]\nParameterName=MOD_DataIn_xxh_AU16[10]\nObjectType=0x7\nDataType=0x0006\nAccessType=rwr\n\n[330C]\nParameterName=MOD_DataIn_xxh_AU16\nObjectType=0x8\nSubNumber=11\n\n[330Csub0]\nParameterName=Number of Entries\nObjectType=0x7\nDataType=0x0005\nAccessType=ro\nDefaultValue=0xA\nLowLimit=0x0\nHighLimit=0xFF\n\n[330Csub1]\nParameterName=MOD_DataIn_xxh_AU16[1]\nObjectType=0x7\nDataType=0x0006\nAccessType=rwr\n\n[330Csub2]\nParameterName=MOD_DataIn_xxh_AU16[2]\nObjectType=0x7\nDataType=0x0006\nAccessType=rwr\n\n[330Csub3]\nParameterName=MOD_DataIn_xxh_AU16[3]\nObjectType=0x7\nDataType=0x0006\nAccessType=rwr\n\n[330Csub4]\nParameterName=MOD_DataIn_xxh_AU16[4]\nObjectType=0x7\nDataType=0x0006\nAccessType=rwr\n\n[330Csub5]\nParameterName=MOD_DataIn_xxh_AU16[5]\nObjectType=0x7\nDataType=0x0006\nAccessType=rwr\n\n[330Csub6]\nParameterName=MOD_DataIn_xxh_AU16[6]\nObjectType=0x7\nDataType=0x0006\nAccessType=rwr\n\n[330Csub7]\nParameterName=MOD_DataIn_xxh_AU16[7]\nObjectType=0x7\nDataType=0x0006\nAccessType=rwr\n\n[330Csub8]\nParameterName=MOD_DataIn_xxh_AU16[8]\nObjectType=0x7\nDataType=0x0006\nAccessType=rwr\n\n[330Csub9]\nParameterName=MOD_DataIn_xxh_AU16[9]\nObjectType=0x7\nDataType=0x0006\nAccessType=rwr\n\n[330CsubA]\nParameterName=MOD_DataIn_xxh_AU16[10]\nObjectType=0x7\nDataType=0x0006\nAccessType=rwr\n\n[330D]\nParameterName=MOD_DataIn_xxh_AU16\nObjectType=0x8\nSubNumber=11\n\n[330Dsub0]\nParameterName=Number of Entries\nObjectType=0x7\nDataType=0x0005\nAccessType=ro\nDefaultValue=0xA\nLowLimit=0x0\nHighLimit=0xFF\n\n[330Dsub1]\nParameterName=MOD_DataIn_xxh_AU16[1]\nObjectType=0x7\nDataType=0x0006\nAccessType=rwr\n\n[330Dsub2]\nParameterName=MOD_DataIn_xxh_AU16[2]\nObjectType=0x7\nDataType=0x0006\nAccessType=rwr\n\n[330Dsub3]\nParameterName=MOD_DataIn_xxh_AU16[3]\nObjectType=0x7\nDataType=0x0006\nAccessType=rwr\n\n[330Dsub4]\nParameterName=MOD_DataIn_xxh_AU16[4]\nObjectType=0x7\nDataType=0x0006\nAccessType=rwr\n\n[330Dsub5]\nParameterName=MOD_DataIn_xxh_AU16[5]\nObjectType=0x7\nDataType=0x0006\nAccessType=rwr\n\n[330Dsub6]\nParameterName=MOD_DataIn_xxh_AU16[6]\nObjectType=0x7\nDataType=0x0006\nAccessType=rwr\n\n[330Dsub7]\nParameterName=MOD_DataIn_xxh_AU16[7]\nObjectType=0x7\nDataType=0x0006\nAccessType=rwr\n\n[330Dsub8]\nParameterName=MOD_DataIn_xxh_AU16[8]\nObjectType=0x7\nDataType=0x0006\nAccessType=rwr\n\n[330Dsub9]\nParameterName=MOD_DataIn_xxh_AU16[9]\nObjectType=0x7\nDataType=0x0006\nAccessType=rwr\n\n[330DsubA]\nParameterName=MOD_DataIn_xxh_AU16[10]\nObjectType=0x7\nDataType=0x0006\nAccessType=rwr\n\n[330E]\nParameterName=MOD_DataIn_xxh_AU16\nObjectType=0x8\nSubNumber=11\n\n[330Esub0]\nParameterName=Number of Entries\nObjectType=0x7\nDataType=0x0005\nAccessType=ro\nDefaultValue=0xA\nLowLimit=0x0\nHighLimit=0xFF\n\n[330Esub1]\nParameterName=MOD_DataIn_xxh_AU16[1]\nObjectType=0x7\nDataType=0x0006\nAccessType=rwr\n\n[330Esub2]\nParameterName=MOD_DataIn_xxh_AU16[2]\nObjectType=0x7\nDataType=0x0006\nAccessType=rwr\n\n[330Esub3]\nParameterName=MOD_DataIn_xxh_AU16[3]\nObjectType=0x7\nDataType=0x0006\nAccessType=rwr\n\n[330Esub4]\nParameterName=MOD_DataIn_xxh_AU16[4]\nObjectType=0x7\nDataType=0x0006\nAccessType=rwr\n\n[330Esub5]\nParameterName=MOD_DataIn_xxh_AU16[5]\nObjectType=0x7\nDataType=0x0006\nAccessType=rwr\n\n[330Esub6]\nParameterName=MOD_DataIn_xxh_AU16[6]\nObjectType=0x7\nDataType=0x0006\nAccessType=rwr\n\n[330Esub7]\nParameterName=MOD_DataIn_xxh_AU16[7]\nObjectType=0x7\nDataType=0x0006\nAccessType=rwr\n\n[330Esub8]\nParameterName=MOD_DataIn_xxh_AU16[8]\nObjectType=0x7\nDataType=0x0006\nAccessType=rwr\n\n[330Esub9]\nParameterName=MOD_DataIn_xxh_AU16[9]\nObjectType=0x7\nDataType=0x0006\nAccessType=rwr\n\n[330EsubA]\nParameterName=MOD_DataIn_xxh_AU16[10]\nObjectType=0x7\nDataType=0x0006\nAccessType=rwr\n\n[330F]\nParameterName=MOD_DataIn_xxh_AU16\nObjectType=0x8\nSubNumber=11\n\n[330Fsub0]\nParameterName=Number of Entries\nObjectType=0x7\nDataType=0x0005\nAccessType=ro\nDefaultValue=0xA\nLowLimit=0x0\nHighLimit=0xFF\n\n[330Fsub1]\nParameterName=MOD_DataIn_xxh_AU16[1]\nObjectType=0x7\nDataType=0x0006\nAccessType=rwr\n\n[330Fsub2]\nParameterName=MOD_DataIn_xxh_AU16[2]\nObjectType=0x7\nDataType=0x0006\nAccessType=rwr\n\n[330Fsub3]\nParameterName=MOD_DataIn_xxh_AU16[3]\nObjectType=0x7\nDataType=0x0006\nAccessType=rwr\n\n[330Fsub4]\nParameterName=MOD_DataIn_xxh_AU16[4]\nObjectType=0x7\nDataType=0x0006\nAccessType=rwr\n\n[330Fsub5]\nParameterName=MOD_DataIn_xxh_AU16[5]\nObjectType=0x7\nDataType=0x0006\nAccessType=rwr\n\n[330Fsub6]\nParameterName=MOD_DataIn_xxh_AU16[6]\nObjectType=0x7\nDataType=0x0006\nAccessType=rwr\n\n[330Fsub7]\nParameterName=MOD_DataIn_xxh_AU16[7]\nObjectType=0x7\nDataType=0x0006\nAccessType=rwr\n\n[330Fsub8]\nParameterName=MOD_DataIn_xxh_AU16[8]\nObjectType=0x7\nDataType=0x0006\nAccessType=rwr\n\n[330Fsub9]\nParameterName=MOD_DataIn_xxh_AU16[9]\nObjectType=0x7\nDataType=0x0006\nAccessType=rwr\n\n[330FsubA]\nParameterName=MOD_DataIn_xxh_AU16[10]\nObjectType=0x7\nDataType=0x0006\nAccessType=rwr\n\n[3310]\nParameterName=MOD_DataIn_xxh_AU16\nObjectType=0x8\nSubNumber=11\n\n[3310sub0]\nParameterName=Number of Entries\nObjectType=0x7\nDataType=0x0005\nAccessType=ro\nDefaultValue=0xA\nLowLimit=0x0\nHighLimit=0xFF\n\n[3310sub1]\nParameterName=MOD_DataIn_xxh_AU16[1]\nObjectType=0x7\nDataType=0x0006\nAccessType=rwr\n\n[3310sub2]\nParameterName=MOD_DataIn_xxh_AU16[2]\nObjectType=0x7\nDataType=0x0006\nAccessType=rwr\n\n[3310sub3]\nParameterName=MOD_DataIn_xxh_AU16[3]\nObjectType=0x7\nDataType=0x0006\nAccessType=rwr\n\n[3310sub4]\nParameterName=MOD_DataIn_xxh_AU16[4]\nObjectType=0x7\nDataType=0x0006\nAccessType=rwr\n\n[3310sub5]\nParameterName=MOD_DataIn_xxh_AU16[5]\nObjectType=0x7\nDataType=0x0006\nAccessType=rwr\n\n[3310sub6]\nParameterName=MOD_DataIn_xxh_AU16[6]\nObjectType=0x7\nDataType=0x0006\nAccessType=rwr\n\n[3310sub7]\nParameterName=MOD_DataIn_xxh_AU16[7]\nObjectType=0x7\nDataType=0x0006\nAccessType=rwr\n\n[3310sub8]\nParameterName=MOD_DataIn_xxh_AU16[8]\nObjectType=0x7\nDataType=0x0006\nAccessType=rwr\n\n[3310sub9]\nParameterName=MOD_DataIn_xxh_AU16[9]\nObjectType=0x7\nDataType=0x0006\nAccessType=rwr\n\n[3310subA]\nParameterName=MOD_DataIn_xxh_AU16[10]\nObjectType=0x7\nDataType=0x0006\nAccessType=rwr\n\n[3311]\nParameterName=MOD_DataIn_xxh_AU16\nObjectType=0x8\nSubNumber=11\n\n[3311sub0]\nParameterName=Number of Entries\nObjectType=0x7\nDataType=0x0005\nAccessType=ro\nDefaultValue=0xA\nLowLimit=0x0\nHighLimit=0xFF\n\n[3311sub1]\nParameterName=MOD_DataIn_xxh_AU16[1]\nObjectType=0x7\nDataType=0x0006\nAccessType=rwr\n\n[3311sub2]\nParameterName=MOD_DataIn_xxh_AU16[2]\nObjectType=0x7\nDataType=0x0006\nAccessType=rwr\n\n[3311sub3]\nParameterName=MOD_DataIn_xxh_AU16[3]\nObjectType=0x7\nDataType=0x0006\nAccessType=rwr\n\n[3311sub4]\nParameterName=MOD_DataIn_xxh_AU16[4]\nObjectType=0x7\nDataType=0x0006\nAccessType=rwr\n\n[3311sub5]\nParameterName=MOD_DataIn_xxh_AU16[5]\nObjectType=0x7\nDataType=0x0006\nAccessType=rwr\n\n[3311sub6]\nParameterName=MOD_DataIn_xxh_AU16[6]\nObjectType=0x7\nDataType=0x0006\nAccessType=rwr\n\n[3311sub7]\nParameterName=MOD_DataIn_xxh_AU16[7]\nObjectType=0x7\nDataType=0x0006\nAccessType=rwr\n\n[3311sub8]\nParameterName=MOD_DataIn_xxh_AU16[8]\nObjectType=0x7\nDataType=0x0006\nAccessType=rwr\n\n[3311sub9]\nParameterName=MOD_DataIn_xxh_AU16[9]\nObjectType=0x7\nDataType=0x0006\nAccessType=rwr\n\n[3311subA]\nParameterName=MOD_DataIn_xxh_AU16[10]\nObjectType=0x7\nDataType=0x0006\nAccessType=rwr\n\n[3312]\nParameterName=MOD_DataIn_xxh_AU16\nObjectType=0x8\nSubNumber=11\n\n[3312sub0]\nParameterName=Number of Entries\nObjectType=0x7\nDataType=0x0005\nAccessType=ro\nDefaultValue=0xA\nLowLimit=0x0\nHighLimit=0xFF\n\n[3312sub1]\nParameterName=MOD_DataIn_xxh_AU16[1]\nObjectType=0x7\nDataType=0x0006\nAccessType=rwr\n\n[3312sub2]\nParameterName=MOD_DataIn_xxh_AU16[2]\nObjectType=0x7\nDataType=0x0006\nAccessType=rwr\n\n[3312sub3]\nParameterName=MOD_DataIn_xxh_AU16[3]\nObjectType=0x7\nDataType=0x0006\nAccessType=rwr\n\n[3312sub4]\nParameterName=MOD_DataIn_xxh_AU16[4]\nObjectType=0x7\nDataType=0x0006\nAccessType=rwr\n\n[3312sub5]\nParameterName=MOD_DataIn_xxh_AU16[5]\nObjectType=0x7\nDataType=0x0006\nAccessType=rwr\n\n[3312sub6]\nParameterName=MOD_DataIn_xxh_AU16[6]\nObjectType=0x7\nDataType=0x0006\nAccessType=rwr\n\n[3312sub7]\nParameterName=MOD_DataIn_xxh_AU16[7]\nObjectType=0x7\nDataType=0x0006\nAccessType=rwr\n\n[3312sub8]\nParameterName=MOD_DataIn_xxh_AU16[8]\nObjectType=0x7\nDataType=0x0006\nAccessType=rwr\n\n[3312sub9]\nParameterName=MOD_DataIn_xxh_AU16[9]\nObjectType=0x7\nDataType=0x0006\nAccessType=rwr\n\n[3312subA]\nParameterName=MOD_DataIn_xxh_AU16[10]\nObjectType=0x7\nDataType=0x0006\nAccessType=rwr\n\n[3313]\nParameterName=MOD_DataIn_xxh_AU16\nObjectType=0x8\nSubNumber=11\n\n[3313sub0]\nParameterName=Number of Entries\nObjectType=0x7\nDataType=0x0005\nAccessType=ro\nDefaultValue=0xA\nLowLimit=0x0\nHighLimit=0xFF\n\n[3313sub1]\nParameterName=MOD_DataIn_xxh_AU16[1]\nObjectType=0x7\nDataType=0x0006\nAccessType=rwr\n\n[3313sub2]\nParameterName=MOD_DataIn_xxh_AU16[2]\nObjectType=0x7\nDataType=0x0006\nAccessType=rwr\n\n[3313sub3]\nParameterName=MOD_DataIn_xxh_AU16[3]\nObjectType=0x7\nDataType=0x0006\nAccessType=rwr\n\n[3313sub4]\nParameterName=MOD_DataIn_xxh_AU16[4]\nObjectType=0x7\nDataType=0x0006\nAccessType=rwr\n\n[3313sub5]\nParameterName=MOD_DataIn_xxh_AU16[5]\nObjectType=0x7\nDataType=0x0006\nAccessType=rwr\n\n[3313sub6]\nParameterName=MOD_DataIn_xxh_AU16[6]\nObjectType=0x7\nDataType=0x0006\nAccessType=rwr\n\n[3313sub7]\nParameterName=MOD_DataIn_xxh_AU16[7]\nObjectType=0x7\nDataType=0x0006\nAccessType=rwr\n\n[3313sub8]\nParameterName=MOD_DataIn_xxh_AU16[8]\nObjectType=0x7\nDataType=0x0006\nAccessType=rwr\n\n[3313sub9]\nParameterName=MOD_DataIn_xxh_AU16[9]\nObjectType=0x7\nDataType=0x0006\nAccessType=rwr\n\n[3313subA]\nParameterName=MOD_DataIn_xxh_AU16[10]\nObjectType=0x7\nDataType=0x0006\nAccessType=rwr\n\n[3314]\nParameterName=MOD_DataIn_xxh_AU16\nObjectType=0x8\nSubNumber=11\n\n[3314sub0]\nParameterName=Number of Entries\nObjectType=0x7\nDataType=0x0005\nAccessType=ro\nDefaultValue=0xA\nLowLimit=0x0\nHighLimit=0xFF\n\n[3314sub1]\nParameterName=MOD_DataIn_xxh_AU16[1]\nObjectType=0x7\nDataType=0x0006\nAccessType=rwr\n\n[3314sub2]\nParameterName=MOD_DataIn_xxh_AU16[2]\nObjectType=0x7\nDataType=0x0006\nAccessType=rwr\n\n[3314sub3]\nParameterName=MOD_DataIn_xxh_AU16[3]\nObjectType=0x7\nDataType=0x0006\nAccessType=rwr\n\n[3314sub4]\nParameterName=MOD_DataIn_xxh_AU16[4]\nObjectType=0x7\nDataType=0x0006\nAccessType=rwr\n\n[3314sub5]\nParameterName=MOD_DataIn_xxh_AU16[5]\nObjectType=0x7\nDataType=0x0006\nAccessType=rwr\n\n[3314sub6]\nParameterName=MOD_DataIn_xxh_AU16[6]\nObjectType=0x7\nDataType=0x0006\nAccessType=rwr\n\n[3314sub7]\nParameterName=MOD_DataIn_xxh_AU16[7]\nObjectType=0x7\nDataType=0x0006\nAccessType=rwr\n\n[3314sub8]\nParameterName=MOD_DataIn_xxh_AU16[8]\nObjectType=0x7\nDataType=0x0006\nAccessType=rwr\n\n[3314sub9]\nParameterName=MOD_DataIn_xxh_AU16[9]\nObjectType=0x7\nDataType=0x0006\nAccessType=rwr\n\n[3314subA]\nParameterName=MOD_DataIn_xxh_AU16[10]\nObjectType=0x7\nDataType=0x0006\nAccessType=rwr\n\n[3400]\nParameterName=MOD_DataIn_xxh_AU32\nObjectType=0x8\nSubNumber=11\n\n[3400sub0]\nParameterName=Number of Entries\nObjectType=0x7\nDataType=0x0005\nAccessType=ro\nDefaultValue=0xA\nLowLimit=0x0\nHighLimit=0xFF\n\n[3400sub1]\nParameterName=MOD_DataIn_xxh_AU32[1]\nObjectType=0x7\nDataType=0x0007\nAccessType=rwr\n\n[3400sub2]\nParameterName=MOD_DataIn_xxh_AU32[2]\nObjectType=0x7\nDataType=0x0007\nAccessType=rwr\n\n[3400sub3]\nParameterName=MOD_DataIn_xxh_AU32[3]\nObjectType=0x7\nDataType=0x0007\nAccessType=rwr\n\n[3400sub4]\nParameterName=MOD_DataIn_xxh_AU32[4]\nObjectType=0x7\nDataType=0x0007\nAccessType=rwr\n\n[3400sub5]\nParameterName=MOD_DataIn_xxh_AU32[5]\nObjectType=0x7\nDataType=0x0007\nAccessType=rwr\n\n[3400sub6]\nParameterName=MOD_DataIn_xxh_AU32[6]\nObjectType=0x7\nDataType=0x0007\nAccessType=rwr\n\n[3400sub7]\nParameterName=MOD_DataIn_xxh_AU32[7]\nObjectType=0x7\nDataType=0x0007\nAccessType=rwr\n\n[3400sub8]\nParameterName=MOD_DataIn_xxh_AU32[8]\nObjectType=0x7\nDataType=0x0007\nAccessType=rwr\n\n[3400sub9]\nParameterName=MOD_DataIn_xxh_AU32[9]\nObjectType=0x7\nDataType=0x0007\nAccessType=rwr\n\n[3400subA]\nParameterName=MOD_DataIn_xxh_AU32[10]\nObjectType=0x7\nDataType=0x0007\nAccessType=rwr\n\n[3401]\nParameterName=MOD_DataIn_xxh_AU32\nObjectType=0x8\nSubNumber=11\n\n[3401sub0]\nParameterName=Number of Entries\nObjectType=0x7\nDataType=0x0005\nAccessType=ro\nDefaultValue=0xA\nLowLimit=0x0\nHighLimit=0xFF\n\n[3401sub1]\nParameterName=MOD_DataIn_xxh_AU32[1]\nObjectType=0x7\nDataType=0x0007\nAccessType=rwr\n\n[3401sub2]\nParameterName=MOD_DataIn_xxh_AU32[2]\nObjectType=0x7\nDataType=0x0007\nAccessType=rwr\n\n[3401sub3]\nParameterName=MOD_DataIn_xxh_AU32[3]\nObjectType=0x7\nDataType=0x0007\nAccessType=rwr\n\n[3401sub4]\nParameterName=MOD_DataIn_xxh_AU32[4]\nObjectType=0x7\nDataType=0x0007\nAccessType=rwr\n\n[3401sub5]\nParameterName=MOD_DataIn_xxh_AU32[5]\nObjectType=0x7\nDataType=0x0007\nAccessType=rwr\n\n[3401sub6]\nParameterName=MOD_DataIn_xxh_AU32[6]\nObjectType=0x7\nDataType=0x0007\nAccessType=rwr\n\n[3401sub7]\nParameterName=MOD_DataIn_xxh_AU32[7]\nObjectType=0x7\nDataType=0x0007\nAccessType=rwr\n\n[3401sub8]\nParameterName=MOD_DataIn_xxh_AU32[8]\nObjectType=0x7\nDataType=0x0007\nAccessType=rwr\n\n[3401sub9]\nParameterName=MOD_DataIn_xxh_AU32[9]\nObjectType=0x7\nDataType=0x0007\nAccessType=rwr\n\n[3401subA]\nParameterName=MOD_DataIn_xxh_AU32[10]\nObjectType=0x7\nDataType=0x0007\nAccessType=rwr\n\n[3402]\nParameterName=MOD_DataIn_xxh_AU32\nObjectType=0x8\nSubNumber=11\n\n[3402sub0]\nParameterName=Number of Entries\nObjectType=0x7\nDataType=0x0005\nAccessType=ro\nDefaultValue=0xA\nLowLimit=0x0\nHighLimit=0xFF\n\n[3402sub1]\nParameterName=MOD_DataIn_xxh_AU32[1]\nObjectType=0x7\nDataType=0x0007\nAccessType=rwr\n\n[3402sub2]\nParameterName=MOD_DataIn_xxh_AU32[2]\nObjectType=0x7\nDataType=0x0007\nAccessType=rwr\n\n[3402sub3]\nParameterName=MOD_DataIn_xxh_AU32[3]\nObjectType=0x7\nDataType=0x0007\nAccessType=rwr\n\n[3402sub4]\nParameterName=MOD_DataIn_xxh_AU32[4]\nObjectType=0x7\nDataType=0x0007\nAccessType=rwr\n\n[3402sub5]\nParameterName=MOD_DataIn_xxh_AU32[5]\nObjectType=0x7\nDataType=0x0007\nAccessType=rwr\n\n[3402sub6]\nParameterName=MOD_DataIn_xxh_AU32[6]\nObjectType=0x7\nDataType=0x0007\nAccessType=rwr\n\n[3402sub7]\nParameterName=MOD_DataIn_xxh_AU32[7]\nObjectType=0x7\nDataType=0x0007\nAccessType=rwr\n\n[3402sub8]\nParameterName=MOD_DataIn_xxh_AU32[8]\nObjectType=0x7\nDataType=0x0007\nAccessType=rwr\n\n[3402sub9]\nParameterName=MOD_DataIn_xxh_AU32[9]\nObjectType=0x7\nDataType=0x0007\nAccessType=rwr\n\n[3402subA]\nParameterName=MOD_DataIn_xxh_AU32[10]\nObjectType=0x7\nDataType=0x0007\nAccessType=rwr\n\n[3403]\nParameterName=MOD_DataIn_xxh_AU32\nObjectType=0x8\nSubNumber=11\n\n[3403sub0]\nParameterName=Number of Entries\nObjectType=0x7\nDataType=0x0005\nAccessType=ro\nDefaultValue=0xA\nLowLimit=0x0\nHighLimit=0xFF\n\n[3403sub1]\nParameterName=MOD_DataIn_xxh_AU32[1]\nObjectType=0x7\nDataType=0x0007\nAccessType=rwr\n\n[3403sub2]\nParameterName=MOD_DataIn_xxh_AU32[2]\nObjectType=0x7\nDataType=0x0007\nAccessType=rwr\n\n[3403sub3]\nParameterName=MOD_DataIn_xxh_AU32[3]\nObjectType=0x7\nDataType=0x0007\nAccessType=rwr\n\n[3403sub4]\nParameterName=MOD_DataIn_xxh_AU32[4]\nObjectType=0x7\nDataType=0x0007\nAccessType=rwr\n\n[3403sub5]\nParameterName=MOD_DataIn_xxh_AU32[5]\nObjectType=0x7\nDataType=0x0007\nAccessType=rwr\n\n[3403sub6]\nParameterName=MOD_DataIn_xxh_AU32[6]\nObjectType=0x7\nDataType=0x0007\nAccessType=rwr\n\n[3403sub7]\nParameterName=MOD_DataIn_xxh_AU32[7]\nObjectType=0x7\nDataType=0x0007\nAccessType=rwr\n\n[3403sub8]\nParameterName=MOD_DataIn_xxh_AU32[8]\nObjectType=0x7\nDataType=0x0007\nAccessType=rwr\n\n[3403sub9]\nParameterName=MOD_DataIn_xxh_AU32[9]\nObjectType=0x7\nDataType=0x0007\nAccessType=rwr\n\n[3403subA]\nParameterName=MOD_DataIn_xxh_AU32[10]\nObjectType=0x7\nDataType=0x0007\nAccessType=rwr\n\n[3404]\nParameterName=MOD_DataIn_xxh_AU32\nObjectType=0x8\nSubNumber=11\n\n[3404sub0]\nParameterName=Number of Entries\nObjectType=0x7\nDataType=0x0005\nAccessType=ro\nDefaultValue=0xA\nLowLimit=0x0\nHighLimit=0xFF\n\n[3404sub1]\nParameterName=MOD_DataIn_xxh_AU32[1]\nObjectType=0x7\nDataType=0x0007\nAccessType=rwr\n\n[3404sub2]\nParameterName=MOD_DataIn_xxh_AU32[2]\nObjectType=0x7\nDataType=0x0007\nAccessType=rwr\n\n[3404sub3]\nParameterName=MOD_DataIn_xxh_AU32[3]\nObjectType=0x7\nDataType=0x0007\nAccessType=rwr\n\n[3404sub4]\nParameterName=MOD_DataIn_xxh_AU32[4]\nObjectType=0x7\nDataType=0x0007\nAccessType=rwr\n\n[3404sub5]\nParameterName=MOD_DataIn_xxh_AU32[5]\nObjectType=0x7\nDataType=0x0007\nAccessType=rwr\n\n[3404sub6]\nParameterName=MOD_DataIn_xxh_AU32[6]\nObjectType=0x7\nDataType=0x0007\nAccessType=rwr\n\n[3404sub7]\nParameterName=MOD_DataIn_xxh_AU32[7]\nObjectType=0x7\nDataType=0x0007\nAccessType=rwr\n\n[3404sub8]\nParameterName=MOD_DataIn_xxh_AU32[8]\nObjectType=0x7\nDataType=0x0007\nAccessType=rwr\n\n[3404sub9]\nParameterName=MOD_DataIn_xxh_AU32[9]\nObjectType=0x7\nDataType=0x0007\nAccessType=rwr\n\n[3404subA]\nParameterName=MOD_DataIn_xxh_AU32[10]\nObjectType=0x7\nDataType=0x0007\nAccessType=rwr\n\n[3405]\nParameterName=MOD_DataIn_xxh_AU32\nObjectType=0x8\nSubNumber=11\n\n[3405sub0]\nParameterName=Number of Entries\nObjectType=0x7\nDataType=0x0005\nAccessType=ro\nDefaultValue=0xA\nLowLimit=0x0\nHighLimit=0xFF\n\n[3405sub1]\nParameterName=MOD_DataIn_xxh_AU32[1]\nObjectType=0x7\nDataType=0x0007\nAccessType=rwr\n\n[3405sub2]\nParameterName=MOD_DataIn_xxh_AU32[2]\nObjectType=0x7\nDataType=0x0007\nAccessType=rwr\n\n[3405sub3]\nParameterName=MOD_DataIn_xxh_AU32[3]\nObjectType=0x7\nDataType=0x0007\nAccessType=rwr\n\n[3405sub4]\nParameterName=MOD_DataIn_xxh_AU32[4]\nObjectType=0x7\nDataType=0x0007\nAccessType=rwr\n\n[3405sub5]\nParameterName=MOD_DataIn_xxh_AU32[5]\nObjectType=0x7\nDataType=0x0007\nAccessType=rwr\n\n[3405sub6]\nParameterName=MOD_DataIn_xxh_AU32[6]\nObjectType=0x7\nDataType=0x0007\nAccessType=rwr\n\n[3405sub7]\nParameterName=MOD_DataIn_xxh_AU32[7]\nObjectType=0x7\nDataType=0x0007\nAccessType=rwr\n\n[3405sub8]\nParameterName=MOD_DataIn_xxh_AU32[8]\nObjectType=0x7\nDataType=0x0007\nAccessType=rwr\n\n[3405sub9]\nParameterName=MOD_DataIn_xxh_AU32[9]\nObjectType=0x7\nDataType=0x0007\nAccessType=rwr\n\n[3405subA]\nParameterName=MOD_DataIn_xxh_AU32[10]\nObjectType=0x7\nDataType=0x0007\nAccessType=rwr\n\n[3406]\nParameterName=MOD_DataIn_xxh_AU32\nObjectType=0x8\nSubNumber=11\n\n[3406sub0]\nParameterName=Number of Entries\nObjectType=0x7\nDataType=0x0005\nAccessType=ro\nDefaultValue=0xA\nLowLimit=0x0\nHighLimit=0xFF\n\n[3406sub1]\nParameterName=MOD_DataIn_xxh_AU32[1]\nObjectType=0x7\nDataType=0x0007\nAccessType=rwr\n\n[3406sub2]\nParameterName=MOD_DataIn_xxh_AU32[2]\nObjectType=0x7\nDataType=0x0007\nAccessType=rwr\n\n[3406sub3]\nParameterName=MOD_DataIn_xxh_AU32[3]\nObjectType=0x7\nDataType=0x0007\nAccessType=rwr\n\n[3406sub4]\nParameterName=MOD_DataIn_xxh_AU32[4]\nObjectType=0x7\nDataType=0x0007\nAccessType=rwr\n\n[3406sub5]\nParameterName=MOD_DataIn_xxh_AU32[5]\nObjectType=0x7\nDataType=0x0007\nAccessType=rwr\n\n[3406sub6]\nParameterName=MOD_DataIn_xxh_AU32[6]\nObjectType=0x7\nDataType=0x0007\nAccessType=rwr\n\n[3406sub7]\nParameterName=MOD_DataIn_xxh_AU32[7]\nObjectType=0x7\nDataType=0x0007\nAccessType=rwr\n\n[3406sub8]\nParameterName=MOD_DataIn_xxh_AU32[8]\nObjectType=0x7\nDataType=0x0007\nAccessType=rwr\n\n[3406sub9]\nParameterName=MOD_DataIn_xxh_AU32[9]\nObjectType=0x7\nDataType=0x0007\nAccessType=rwr\n\n[3406subA]\nParameterName=MOD_DataIn_xxh_AU32[10]\nObjectType=0x7\nDataType=0x0007\nAccessType=rwr\n\n[3407]\nParameterName=MOD_DataIn_xxh_AU32\nObjectType=0x8\nSubNumber=11\n\n[3407sub0]\nParameterName=Number of Entries\nObjectType=0x7\nDataType=0x0005\nAccessType=ro\nDefaultValue=0xA\nLowLimit=0x0\nHighLimit=0xFF\n\n[3407sub1]\nParameterName=MOD_DataIn_xxh_AU32[1]\nObjectType=0x7\nDataType=0x0007\nAccessType=rwr\n\n[3407sub2]\nParameterName=MOD_DataIn_xxh_AU32[2]\nObjectType=0x7\nDataType=0x0007\nAccessType=rwr\n\n[3407sub3]\nParameterName=MOD_DataIn_xxh_AU32[3]\nObjectType=0x7\nDataType=0x0007\nAccessType=rwr\n\n[3407sub4]\nParameterName=MOD_DataIn_xxh_AU32[4]\nObjectType=0x7\nDataType=0x0007\nAccessType=rwr\n\n[3407sub5]\nParameterName=MOD_DataIn_xxh_AU32[5]\nObjectType=0x7\nDataType=0x0007\nAccessType=rwr\n\n[3407sub6]\nParameterName=MOD_DataIn_xxh_AU32[6]\nObjectType=0x7\nDataType=0x0007\nAccessType=rwr\n\n[3407sub7]\nParameterName=MOD_DataIn_xxh_AU32[7]\nObjectType=0x7\nDataType=0x0007\nAccessType=rwr\n\n[3407sub8]\nParameterName=MOD_DataIn_xxh_AU32[8]\nObjectType=0x7\nDataType=0x0007\nAccessType=rwr\n\n[3407sub9]\nParameterName=MOD_DataIn_xxh_AU32[9]\nObjectType=0x7\nDataType=0x0007\nAccessType=rwr\n\n[3407subA]\nParameterName=MOD_DataIn_xxh_AU32[10]\nObjectType=0x7\nDataType=0x0007\nAccessType=rwr\n\n[3408]\nParameterName=MOD_DataIn_xxh_AU32\nObjectType=0x8\nSubNumber=11\n\n[3408sub0]\nParameterName=Number of Entries\nObjectType=0x7\nDataType=0x0005\nAccessType=ro\nDefaultValue=0xA\nLowLimit=0x0\nHighLimit=0xFF\n\n[3408sub1]\nParameterName=MOD_DataIn_xxh_AU32[1]\nObjectType=0x7\nDataType=0x0007\nAccessType=rwr\n\n[3408sub2]\nParameterName=MOD_DataIn_xxh_AU32[2]\nObjectType=0x7\nDataType=0x0007\nAccessType=rwr\n\n[3408sub3]\nParameterName=MOD_DataIn_xxh_AU32[3]\nObjectType=0x7\nDataType=0x0007\nAccessType=rwr\n\n[3408sub4]\nParameterName=MOD_DataIn_xxh_AU32[4]\nObjectType=0x7\nDataType=0x0007\nAccessType=rwr\n\n[3408sub5]\nParameterName=MOD_DataIn_xxh_AU32[5]\nObjectType=0x7\nDataType=0x0007\nAccessType=rwr\n\n[3408sub6]\nParameterName=MOD_DataIn_xxh_AU32[6]\nObjectType=0x7\nDataType=0x0007\nAccessType=rwr\n\n[3408sub7]\nParameterName=MOD_DataIn_xxh_AU32[7]\nObjectType=0x7\nDataType=0x0007\nAccessType=rwr\n\n[3408sub8]\nParameterName=MOD_DataIn_xxh_AU32[8]\nObjectType=0x7\nDataType=0x0007\nAccessType=rwr\n\n[3408sub9]\nParameterName=MOD_DataIn_xxh_AU32[9]\nObjectType=0x7\nDataType=0x0007\nAccessType=rwr\n\n[3408subA]\nParameterName=MOD_DataIn_xxh_AU32[10]\nObjectType=0x7\nDataType=0x0007\nAccessType=rwr\n\n[3409]\nParameterName=MOD_DataIn_xxh_AU32\nObjectType=0x8\nSubNumber=11\n\n[3409sub0]\nParameterName=Number of Entries\nObjectType=0x7\nDataType=0x0005\nAccessType=ro\nDefaultValue=0xA\nLowLimit=0x0\nHighLimit=0xFF\n\n[3409sub1]\nParameterName=MOD_DataIn_xxh_AU32[1]\nObjectType=0x7\nDataType=0x0007\nAccessType=rwr\n\n[3409sub2]\nParameterName=MOD_DataIn_xxh_AU32[2]\nObjectType=0x7\nDataType=0x0007\nAccessType=rwr\n\n[3409sub3]\nParameterName=MOD_DataIn_xxh_AU32[3]\nObjectType=0x7\nDataType=0x0007\nAccessType=rwr\n\n[3409sub4]\nParameterName=MOD_DataIn_xxh_AU32[4]\nObjectType=0x7\nDataType=0x0007\nAccessType=rwr\n\n[3409sub5]\nParameterName=MOD_DataIn_xxh_AU32[5]\nObjectType=0x7\nDataType=0x0007\nAccessType=rwr\n\n[3409sub6]\nParameterName=MOD_DataIn_xxh_AU32[6]\nObjectType=0x7\nDataType=0x0007\nAccessType=rwr\n\n[3409sub7]\nParameterName=MOD_DataIn_xxh_AU32[7]\nObjectType=0x7\nDataType=0x0007\nAccessType=rwr\n\n[3409sub8]\nParameterName=MOD_DataIn_xxh_AU32[8]\nObjectType=0x7\nDataType=0x0007\nAccessType=rwr\n\n[3409sub9]\nParameterName=MOD_DataIn_xxh_AU32[9]\nObjectType=0x7\nDataType=0x0007\nAccessType=rwr\n\n[3409subA]\nParameterName=MOD_DataIn_xxh_AU32[10]\nObjectType=0x7\nDataType=0x0007\nAccessType=rwr\n\n[340A]\nParameterName=MOD_DataIn_xxh_AU32\nObjectType=0x8\nSubNumber=11\n\n[340Asub0]\nParameterName=Number of Entries\nObjectType=0x7\nDataType=0x0005\nAccessType=ro\nDefaultValue=0xA\nLowLimit=0x0\nHighLimit=0xFF\n\n[340Asub1]\nParameterName=MOD_DataIn_xxh_AU32[1]\nObjectType=0x7\nDataType=0x0007\nAccessType=rwr\n\n[340Asub2]\nParameterName=MOD_DataIn_xxh_AU32[2]\nObjectType=0x7\nDataType=0x0007\nAccessType=rwr\n\n[340Asub3]\nParameterName=MOD_DataIn_xxh_AU32[3]\nObjectType=0x7\nDataType=0x0007\nAccessType=rwr\n\n[340Asub4]\nParameterName=MOD_DataIn_xxh_AU32[4]\nObjectType=0x7\nDataType=0x0007\nAccessType=rwr\n\n[340Asub5]\nParameterName=MOD_DataIn_xxh_AU32[5]\nObjectType=0x7\nDataType=0x0007\nAccessType=rwr\n\n[340Asub6]\nParameterName=MOD_DataIn_xxh_AU32[6]\nObjectType=0x7\nDataType=0x0007\nAccessType=rwr\n\n[340Asub7]\nParameterName=MOD_DataIn_xxh_AU32[7]\nObjectType=0x7\nDataType=0x0007\nAccessType=rwr\n\n[340Asub8]\nParameterName=MOD_DataIn_xxh_AU32[8]\nObjectType=0x7\nDataType=0x0007\nAccessType=rwr\n\n[340Asub9]\nParameterName=MOD_DataIn_xxh_AU32[9]\nObjectType=0x7\nDataType=0x0007\nAccessType=rwr\n\n[340AsubA]\nParameterName=MOD_DataIn_xxh_AU32[10]\nObjectType=0x7\nDataType=0x0007\nAccessType=rwr\n\n[340B]\nParameterName=MOD_DataIn_xxh_AU32\nObjectType=0x8\nSubNumber=11\n\n[340Bsub0]\nParameterName=Number of Entries\nObjectType=0x7\nDataType=0x0005\nAccessType=ro\nDefaultValue=0xA\nLowLimit=0x0\nHighLimit=0xFF\n\n[340Bsub1]\nParameterName=MOD_DataIn_xxh_AU32[1]\nObjectType=0x7\nDataType=0x0007\nAccessType=rwr\n\n[340Bsub2]\nParameterName=MOD_DataIn_xxh_AU32[2]\nObjectType=0x7\nDataType=0x0007\nAccessType=rwr\n\n[340Bsub3]\nParameterName=MOD_DataIn_xxh_AU32[3]\nObjectType=0x7\nDataType=0x0007\nAccessType=rwr\n\n[340Bsub4]\nParameterName=MOD_DataIn_xxh_AU32[4]\nObjectType=0x7\nDataType=0x0007\nAccessType=rwr\n\n[340Bsub5]\nParameterName=MOD_DataIn_xxh_AU32[5]\nObjectType=0x7\nDataType=0x0007\nAccessType=rwr\n\n[340Bsub6]\nParameterName=MOD_DataIn_xxh_AU32[6]\nObjectType=0x7\nDataType=0x0007\nAccessType=rwr\n\n[340Bsub7]\nParameterName=MOD_DataIn_xxh_AU32[7]\nObjectType=0x7\nDataType=0x0007\nAccessType=rwr\n\n[340Bsub8]\nParameterName=MOD_DataIn_xxh_AU32[8]\nObjectType=0x7\nDataType=0x0007\nAccessType=rwr\n\n[340Bsub9]\nParameterName=MOD_DataIn_xxh_AU32[9]\nObjectType=0x7\nDataType=0x0007\nAccessType=rwr\n\n[340BsubA]\nParameterName=MOD_DataIn_xxh_AU32[10]\nObjectType=0x7\nDataType=0x0007\nAccessType=rwr\n\n[340C]\nParameterName=MOD_DataIn_xxh_AU32\nObjectType=0x8\nSubNumber=11\n\n[340Csub0]\nParameterName=Number of Entries\nObjectType=0x7\nDataType=0x0005\nAccessType=ro\nDefaultValue=0xA\nLowLimit=0x0\nHighLimit=0xFF\n\n[340Csub1]\nParameterName=MOD_DataIn_xxh_AU32[1]\nObjectType=0x7\nDataType=0x0007\nAccessType=rwr\n\n[340Csub2]\nParameterName=MOD_DataIn_xxh_AU32[2]\nObjectType=0x7\nDataType=0x0007\nAccessType=rwr\n\n[340Csub3]\nParameterName=MOD_DataIn_xxh_AU32[3]\nObjectType=0x7\nDataType=0x0007\nAccessType=rwr\n\n[340Csub4]\nParameterName=MOD_DataIn_xxh_AU32[4]\nObjectType=0x7\nDataType=0x0007\nAccessType=rwr\n\n[340Csub5]\nParameterName=MOD_DataIn_xxh_AU32[5]\nObjectType=0x7\nDataType=0x0007\nAccessType=rwr\n\n[340Csub6]\nParameterName=MOD_DataIn_xxh_AU32[6]\nObjectType=0x7\nDataType=0x0007\nAccessType=rwr\n\n[340Csub7]\nParameterName=MOD_DataIn_xxh_AU32[7]\nObjectType=0x7\nDataType=0x0007\nAccessType=rwr\n\n[340Csub8]\nParameterName=MOD_DataIn_xxh_AU32[8]\nObjectType=0x7\nDataType=0x0007\nAccessType=rwr\n\n[340Csub9]\nParameterName=MOD_DataIn_xxh_AU32[9]\nObjectType=0x7\nDataType=0x0007\nAccessType=rwr\n\n[340CsubA]\nParameterName=MOD_DataIn_xxh_AU32[10]\nObjectType=0x7\nDataType=0x0007\nAccessType=rwr\n\n[340D]\nParameterName=MOD_DataIn_xxh_AU32\nObjectType=0x8\nSubNumber=11\n\n[340Dsub0]\nParameterName=Number of Entries\nObjectType=0x7\nDataType=0x0005\nAccessType=ro\nDefaultValue=0xA\nLowLimit=0x0\nHighLimit=0xFF\n\n[340Dsub1]\nParameterName=MOD_DataIn_xxh_AU32[1]\nObjectType=0x7\nDataType=0x0007\nAccessType=rwr\n\n[340Dsub2]\nParameterName=MOD_DataIn_xxh_AU32[2]\nObjectType=0x7\nDataType=0x0007\nAccessType=rwr\n\n[340Dsub3]\nParameterName=MOD_DataIn_xxh_AU32[3]\nObjectType=0x7\nDataType=0x0007\nAccessType=rwr\n\n[340Dsub4]\nParameterName=MOD_DataIn_xxh_AU32[4]\nObjectType=0x7\nDataType=0x0007\nAccessType=rwr\n\n[340Dsub5]\nParameterName=MOD_DataIn_xxh_AU32[5]\nObjectType=0x7\nDataType=0x0007\nAccessType=rwr\n\n[340Dsub6]\nParameterName=MOD_DataIn_xxh_AU32[6]\nObjectType=0x7\nDataType=0x0007\nAccessType=rwr\n\n[340Dsub7]\nParameterName=MOD_DataIn_xxh_AU32[7]\nObjectType=0x7\nDataType=0x0007\nAccessType=rwr\n\n[340Dsub8]\nParameterName=MOD_DataIn_xxh_AU32[8]\nObjectType=0x7\nDataType=0x0007\nAccessType=rwr\n\n[340Dsub9]\nParameterName=MOD_DataIn_xxh_AU32[9]\nObjectType=0x7\nDataType=0x0007\nAccessType=rwr\n\n[340DsubA]\nParameterName=MOD_DataIn_xxh_AU32[10]\nObjectType=0x7\nDataType=0x0007\nAccessType=rwr\n\n[340E]\nParameterName=MOD_DataIn_xxh_AU32\nObjectType=0x8\nSubNumber=11\n\n[340Esub0]\nParameterName=Number of Entries\nObjectType=0x7\nDataType=0x0005\nAccessType=ro\nDefaultValue=0xA\nLowLimit=0x0\nHighLimit=0xFF\n\n[340Esub1]\nParameterName=MOD_DataIn_xxh_AU32[1]\nObjectType=0x7\nDataType=0x0007\nAccessType=rwr\n\n[340Esub2]\nParameterName=MOD_DataIn_xxh_AU32[2]\nObjectType=0x7\nDataType=0x0007\nAccessType=rwr\n\n[340Esub3]\nParameterName=MOD_DataIn_xxh_AU32[3]\nObjectType=0x7\nDataType=0x0007\nAccessType=rwr\n\n[340Esub4]\nParameterName=MOD_DataIn_xxh_AU32[4]\nObjectType=0x7\nDataType=0x0007\nAccessType=rwr\n\n[340Esub5]\nParameterName=MOD_DataIn_xxh_AU32[5]\nObjectType=0x7\nDataType=0x0007\nAccessType=rwr\n\n[340Esub6]\nParameterName=MOD_DataIn_xxh_AU32[6]\nObjectType=0x7\nDataType=0x0007\nAccessType=rwr\n\n[340Esub7]\nParameterName=MOD_DataIn_xxh_AU32[7]\nObjectType=0x7\nDataType=0x0007\nAccessType=rwr\n\n[340Esub8]\nParameterName=MOD_DataIn_xxh_AU32[8]\nObjectType=0x7\nDataType=0x0007\nAccessType=rwr\n\n[340Esub9]\nParameterName=MOD_DataIn_xxh_AU32[9]\nObjectType=0x7\nDataType=0x0007\nAccessType=rwr\n\n[340EsubA]\nParameterName=MOD_DataIn_xxh_AU32[10]\nObjectType=0x7\nDataType=0x0007\nAccessType=rwr\n\n[340F]\nParameterName=MOD_DataIn_xxh_AU32\nObjectType=0x8\nSubNumber=11\n\n[340Fsub0]\nParameterName=Number of Entries\nObjectType=0x7\nDataType=0x0005\nAccessType=ro\nDefaultValue=0xA\nLowLimit=0x0\nHighLimit=0xFF\n\n[340Fsub1]\nParameterName=MOD_DataIn_xxh_AU32[1]\nObjectType=0x7\nDataType=0x0007\nAccessType=rwr\n\n[340Fsub2]\nParameterName=MOD_DataIn_xxh_AU32[2]\nObjectType=0x7\nDataType=0x0007\nAccessType=rwr\n\n[340Fsub3]\nParameterName=MOD_DataIn_xxh_AU32[3]\nObjectType=0x7\nDataType=0x0007\nAccessType=rwr\n\n[340Fsub4]\nParameterName=MOD_DataIn_xxh_AU32[4]\nObjectType=0x7\nDataType=0x0007\nAccessType=rwr\n\n[340Fsub5]\nParameterName=MOD_DataIn_xxh_AU32[5]\nObjectType=0x7\nDataType=0x0007\nAccessType=rwr\n\n[340Fsub6]\nParameterName=MOD_DataIn_xxh_AU32[6]\nObjectType=0x7\nDataType=0x0007\nAccessType=rwr\n\n[340Fsub7]\nParameterName=MOD_DataIn_xxh_AU32[7]\nObjectType=0x7\nDataType=0x0007\nAccessType=rwr\n\n[340Fsub8]\nParameterName=MOD_DataIn_xxh_AU32[8]\nObjectType=0x7\nDataType=0x0007\nAccessType=rwr\n\n[340Fsub9]\nParameterName=MOD_DataIn_xxh_AU32[9]\nObjectType=0x7\nDataType=0x0007\nAccessType=rwr\n\n[340FsubA]\nParameterName=MOD_DataIn_xxh_AU32[10]\nObjectType=0x7\nDataType=0x0007\nAccessType=rwr\n\n[3410]\nParameterName=MOD_DataIn_xxh_AU32\nObjectType=0x8\nSubNumber=11\n\n[3410sub0]\nParameterName=Number of Entries\nObjectType=0x7\nDataType=0x0005\nAccessType=ro\nDefaultValue=0xA\nLowLimit=0x0\nHighLimit=0xFF\n\n[3410sub1]\nParameterName=MOD_DataIn_xxh_AU32[1]\nObjectType=0x7\nDataType=0x0007\nAccessType=rwr\n\n[3410sub2]\nParameterName=MOD_DataIn_xxh_AU32[2]\nObjectType=0x7\nDataType=0x0007\nAccessType=rwr\n\n[3410sub3]\nParameterName=MOD_DataIn_xxh_AU32[3]\nObjectType=0x7\nDataType=0x0007\nAccessType=rwr\n\n[3410sub4]\nParameterName=MOD_DataIn_xxh_AU32[4]\nObjectType=0x7\nDataType=0x0007\nAccessType=rwr\n\n[3410sub5]\nParameterName=MOD_DataIn_xxh_AU32[5]\nObjectType=0x7\nDataType=0x0007\nAccessType=rwr\n\n[3410sub6]\nParameterName=MOD_DataIn_xxh_AU32[6]\nObjectType=0x7\nDataType=0x0007\nAccessType=rwr\n\n[3410sub7]\nParameterName=MOD_DataIn_xxh_AU32[7]\nObjectType=0x7\nDataType=0x0007\nAccessType=rwr\n\n[3410sub8]\nParameterName=MOD_DataIn_xxh_AU32[8]\nObjectType=0x7\nDataType=0x0007\nAccessType=rwr\n\n[3410sub9]\nParameterName=MOD_DataIn_xxh_AU32[9]\nObjectType=0x7\nDataType=0x0007\nAccessType=rwr\n\n[3410subA]\nParameterName=MOD_DataIn_xxh_AU32[10]\nObjectType=0x7\nDataType=0x0007\nAccessType=rwr\n\n[3411]\nParameterName=MOD_DataIn_xxh_AU32\nObjectType=0x8\nSubNumber=11\n\n[3411sub0]\nParameterName=Number of Entries\nObjectType=0x7\nDataType=0x0005\nAccessType=ro\nDefaultValue=0xA\nLowLimit=0x0\nHighLimit=0xFF\n\n[3411sub1]\nParameterName=MOD_DataIn_xxh_AU32[1]\nObjectType=0x7\nDataType=0x0007\nAccessType=rwr\n\n[3411sub2]\nParameterName=MOD_DataIn_xxh_AU32[2]\nObjectType=0x7\nDataType=0x0007\nAccessType=rwr\n\n[3411sub3]\nParameterName=MOD_DataIn_xxh_AU32[3]\nObjectType=0x7\nDataType=0x0007\nAccessType=rwr\n\n[3411sub4]\nParameterName=MOD_DataIn_xxh_AU32[4]\nObjectType=0x7\nDataType=0x0007\nAccessType=rwr\n\n[3411sub5]\nParameterName=MOD_DataIn_xxh_AU32[5]\nObjectType=0x7\nDataType=0x0007\nAccessType=rwr\n\n[3411sub6]\nParameterName=MOD_DataIn_xxh_AU32[6]\nObjectType=0x7\nDataType=0x0007\nAccessType=rwr\n\n[3411sub7]\nParameterName=MOD_DataIn_xxh_AU32[7]\nObjectType=0x7\nDataType=0x0007\nAccessType=rwr\n\n[3411sub8]\nParameterName=MOD_DataIn_xxh_AU32[8]\nObjectType=0x7\nDataType=0x0007\nAccessType=rwr\n\n[3411sub9]\nParameterName=MOD_DataIn_xxh_AU32[9]\nObjectType=0x7\nDataType=0x0007\nAccessType=rwr\n\n[3411subA]\nParameterName=MOD_DataIn_xxh_AU32[10]\nObjectType=0x7\nDataType=0x0007\nAccessType=rwr\n\n[3412]\nParameterName=MOD_DataIn_xxh_AU32\nObjectType=0x8\nSubNumber=11\n\n[3412sub0]\nParameterName=Number of Entries\nObjectType=0x7\nDataType=0x0005\nAccessType=ro\nDefaultValue=0xA\nLowLimit=0x0\nHighLimit=0xFF\n\n[3412sub1]\nParameterName=MOD_DataIn_xxh_AU32[1]\nObjectType=0x7\nDataType=0x0007\nAccessType=rwr\n\n[3412sub2]\nParameterName=MOD_DataIn_xxh_AU32[2]\nObjectType=0x7\nDataType=0x0007\nAccessType=rwr\n\n[3412sub3]\nParameterName=MOD_DataIn_xxh_AU32[3]\nObjectType=0x7\nDataType=0x0007\nAccessType=rwr\n\n[3412sub4]\nParameterName=MOD_DataIn_xxh_AU32[4]\nObjectType=0x7\nDataType=0x0007\nAccessType=rwr\n\n[3412sub5]\nParameterName=MOD_DataIn_xxh_AU32[5]\nObjectType=0x7\nDataType=0x0007\nAccessType=rwr\n\n[3412sub6]\nParameterName=MOD_DataIn_xxh_AU32[6]\nObjectType=0x7\nDataType=0x0007\nAccessType=rwr\n\n[3412sub7]\nParameterName=MOD_DataIn_xxh_AU32[7]\nObjectType=0x7\nDataType=0x0007\nAccessType=rwr\n\n[3412sub8]\nParameterName=MOD_DataIn_xxh_AU32[8]\nObjectType=0x7\nDataType=0x0007\nAccessType=rwr\n\n[3412sub9]\nParameterName=MOD_DataIn_xxh_AU32[9]\nObjectType=0x7\nDataType=0x0007\nAccessType=rwr\n\n[3412subA]\nParameterName=MOD_DataIn_xxh_AU32[10]\nObjectType=0x7\nDataType=0x0007\nAccessType=rwr\n\n[3413]\nParameterName=MOD_DataIn_xxh_AU32\nObjectType=0x8\nSubNumber=11\n\n[3413sub0]\nParameterName=Number of Entries\nObjectType=0x7\nDataType=0x0005\nAccessType=ro\nDefaultValue=0xA\nLowLimit=0x0\nHighLimit=0xFF\n\n[3413sub1]\nParameterName=MOD_DataIn_xxh_AU32[1]\nObjectType=0x7\nDataType=0x0007\nAccessType=rwr\n\n[3413sub2]\nParameterName=MOD_DataIn_xxh_AU32[2]\nObjectType=0x7\nDataType=0x0007\nAccessType=rwr\n\n[3413sub3]\nParameterName=MOD_DataIn_xxh_AU32[3]\nObjectType=0x7\nDataType=0x0007\nAccessType=rwr\n\n[3413sub4]\nParameterName=MOD_DataIn_xxh_AU32[4]\nObjectType=0x7\nDataType=0x0007\nAccessType=rwr\n\n[3413sub5]\nParameterName=MOD_DataIn_xxh_AU32[5]\nObjectType=0x7\nDataType=0x0007\nAccessType=rwr\n\n[3413sub6]\nParameterName=MOD_DataIn_xxh_AU32[6]\nObjectType=0x7\nDataType=0x0007\nAccessType=rwr\n\n[3413sub7]\nParameterName=MOD_DataIn_xxh_AU32[7]\nObjectType=0x7\nDataType=0x0007\nAccessType=rwr\n\n[3413sub8]\nParameterName=MOD_DataIn_xxh_AU32[8]\nObjectType=0x7\nDataType=0x0007\nAccessType=rwr\n\n[3413sub9]\nParameterName=MOD_DataIn_xxh_AU32[9]\nObjectType=0x7\nDataType=0x0007\nAccessType=rwr\n\n[3413subA]\nParameterName=MOD_DataIn_xxh_AU32[10]\nObjectType=0x7\nDataType=0x0007\nAccessType=rwr\n\n[3500]\nParameterName=MOD_DataOut_xxh_AU8\nObjectType=0x8\nSubNumber=11\n\n[3500sub0]\nParameterName=Number of Entries\nObjectType=0x7\nDataType=0x0005\nAccessType=ro\nDefaultValue=0xa\nLowLimit=0x0\nHighLimit=0xFF\n\n[3500sub1]\nParameterName=MOD_DataOut_xxh_AU8[1]\nObjectType=0x7\nDataType=0x0005\nAccessType=rwr\n\n[3500sub2]\nParameterName=MOD_DataOut_xxh_AU8[2]\nObjectType=0x7\nDataType=0x0005\nAccessType=rwr\n\n[3500sub3]\nParameterName=MOD_DataOut_xxh_AU8[3]\nObjectType=0x7\nDataType=0x0005\nAccessType=rwr\n\n[3500sub4]\nParameterName=MOD_DataOut_xxh_AU8[4]\nObjectType=0x7\nDataType=0x0005\nAccessType=rwr\n\n[3500sub5]\nParameterName=MOD_DataOut_xxh_AU8[5]\nObjectType=0x7\nDataType=0x0005\nAccessType=rwr\n\n[3500sub6]\nParameterName=MOD_DataOut_xxh_AU8[6]\nObjectType=0x7\nDataType=0x0005\nAccessType=rwr\n\n[3500sub7]\nParameterName=MOD_DataOut_xxh_AU8[7]\nObjectType=0x7\nDataType=0x0005\nAccessType=rwr\n\n[3500sub8]\nParameterName=MOD_DataOut_xxh_AU8[8]\nObjectType=0x7\nDataType=0x0005\nAccessType=rwr\n\n[3500sub9]\nParameterName=MOD_DataOut_xxh_AU8[9]\nObjectType=0x7\nDataType=0x0005\nAccessType=rwr\n\n[3500subA]\nParameterName=MOD_DataOut_xxh_AU8[10]\nObjectType=0x7\nDataType=0x0005\nAccessType=rwr\n\n[3501]\nParameterName=MOD_DataOut_xxh_AU8\nObjectType=0x8\nSubNumber=11\n\n[3501sub0]\nParameterName=Number of Entries\nObjectType=0x7\nDataType=0x0005\nAccessType=ro\nDefaultValue=0xa\nLowLimit=0x0\nHighLimit=0xFF\n\n[3501sub1]\nParameterName=MOD_DataOut_xxh_AU8[1]\nObjectType=0x7\nDataType=0x0005\nAccessType=rwr\n\n[3501sub2]\nParameterName=MOD_DataOut_xxh_AU8[2]\nObjectType=0x7\nDataType=0x0005\nAccessType=rwr\n\n[3501sub3]\nParameterName=MOD_DataOut_xxh_AU8[3]\nObjectType=0x7\nDataType=0x0005\nAccessType=rwr\n\n[3501sub4]\nParameterName=MOD_DataOut_xxh_AU8[4]\nObjectType=0x7\nDataType=0x0005\nAccessType=rwr\n\n[3501sub5]\nParameterName=MOD_DataOut_xxh_AU8[5]\nObjectType=0x7\nDataType=0x0005\nAccessType=rwr\n\n[3501sub6]\nParameterName=MOD_DataOut_xxh_AU8[6]\nObjectType=0x7\nDataType=0x0005\nAccessType=rwr\n\n[3501sub7]\nParameterName=MOD_DataOut_xxh_AU8[7]\nObjectType=0x7\nDataType=0x0005\nAccessType=rwr\n\n[3501sub8]\nParameterName=MOD_DataOut_xxh_AU8[8]\nObjectType=0x7\nDataType=0x0005\nAccessType=rwr\n\n[3501sub9]\nParameterName=MOD_DataOut_xxh_AU8[9]\nObjectType=0x7\nDataType=0x0005\nAccessType=rwr\n\n[3501subA]\nParameterName=MOD_DataOut_xxh_AU8[10]\nObjectType=0x7\nDataType=0x0005\nAccessType=rwr\n\n[3502]\nParameterName=MOD_DataOut_xxh_AU8\nObjectType=0x8\nSubNumber=11\n\n[3502sub0]\nParameterName=Number of Entries\nObjectType=0x7\nDataType=0x0005\nAccessType=ro\nDefaultValue=0xa\nLowLimit=0x0\nHighLimit=0xFF\n\n[3502sub1]\nParameterName=MOD_DataOut_xxh_AU8[1]\nObjectType=0x7\nDataType=0x0005\nAccessType=rwr\n\n[3502sub2]\nParameterName=MOD_DataOut_xxh_AU8[2]\nObjectType=0x7\nDataType=0x0005\nAccessType=rwr\n\n[3502sub3]\nParameterName=MOD_DataOut_xxh_AU8[3]\nObjectType=0x7\nDataType=0x0005\nAccessType=rwr\n\n[3502sub4]\nParameterName=MOD_DataOut_xxh_AU8[4]\nObjectType=0x7\nDataType=0x0005\nAccessType=rwr\n\n[3502sub5]\nParameterName=MOD_DataOut_xxh_AU8[5]\nObjectType=0x7\nDataType=0x0005\nAccessType=rwr\n\n[3502sub6]\nParameterName=MOD_DataOut_xxh_AU8[6]\nObjectType=0x7\nDataType=0x0005\nAccessType=rwr\n\n[3502sub7]\nParameterName=MOD_DataOut_xxh_AU8[7]\nObjectType=0x7\nDataType=0x0005\nAccessType=rwr\n\n[3502sub8]\nParameterName=MOD_DataOut_xxh_AU8[8]\nObjectType=0x7\nDataType=0x0005\nAccessType=rwr\n\n[3502sub9]\nParameterName=MOD_DataOut_xxh_AU8[9]\nObjectType=0x7\nDataType=0x0005\nAccessType=rwr\n\n[3502subA]\nParameterName=MOD_DataOut_xxh_AU8[10]\nObjectType=0x7\nDataType=0x0005\nAccessType=rwr\n\n[3503]\nParameterName=MOD_DataOut_xxh_AU8\nObjectType=0x8\nSubNumber=11\n\n[3503sub0]\nParameterName=Number of Entries\nObjectType=0x7\nDataType=0x0005\nAccessType=ro\nDefaultValue=0xa\nLowLimit=0x0\nHighLimit=0xFF\n\n[3503sub1]\nParameterName=MOD_DataOut_xxh_AU8[1]\nObjectType=0x7\nDataType=0x0005\nAccessType=rwr\n\n[3503sub2]\nParameterName=MOD_DataOut_xxh_AU8[2]\nObjectType=0x7\nDataType=0x0005\nAccessType=rwr\n\n[3503sub3]\nParameterName=MOD_DataOut_xxh_AU8[3]\nObjectType=0x7\nDataType=0x0005\nAccessType=rwr\n\n[3503sub4]\nParameterName=MOD_DataOut_xxh_AU8[4]\nObjectType=0x7\nDataType=0x0005\nAccessType=rwr\n\n[3503sub5]\nParameterName=MOD_DataOut_xxh_AU8[5]\nObjectType=0x7\nDataType=0x0005\nAccessType=rwr\n\n[3503sub6]\nParameterName=MOD_DataOut_xxh_AU8[6]\nObjectType=0x7\nDataType=0x0005\nAccessType=rwr\n\n[3503sub7]\nParameterName=MOD_DataOut_xxh_AU8[7]\nObjectType=0x7\nDataType=0x0005\nAccessType=rwr\n\n[3503sub8]\nParameterName=MOD_DataOut_xxh_AU8[8]\nObjectType=0x7\nDataType=0x0005\nAccessType=rwr\n\n[3503sub9]\nParameterName=MOD_DataOut_xxh_AU8[9]\nObjectType=0x7\nDataType=0x0005\nAccessType=rwr\n\n[3503subA]\nParameterName=MOD_DataOut_xxh_AU8[10]\nObjectType=0x7\nDataType=0x0005\nAccessType=rwr\n\n[3504]\nParameterName=MOD_DataOut_xxh_AU8\nObjectType=0x8\nSubNumber=11\n\n[3504sub0]\nParameterName=Number of Entries\nObjectType=0x7\nDataType=0x0005\nAccessType=ro\nDefaultValue=0xa\nLowLimit=0x0\nHighLimit=0xFF\n\n[3504sub1]\nParameterName=MOD_DataOut_xxh_AU8[1]\nObjectType=0x7\nDataType=0x0005\nAccessType=rwr\n\n[3504sub2]\nParameterName=MOD_DataOut_xxh_AU8[2]\nObjectType=0x7\nDataType=0x0005\nAccessType=rwr\n\n[3504sub3]\nParameterName=MOD_DataOut_xxh_AU8[3]\nObjectType=0x7\nDataType=0x0005\nAccessType=rwr\n\n[3504sub4]\nParameterName=MOD_DataOut_xxh_AU8[4]\nObjectType=0x7\nDataType=0x0005\nAccessType=rwr\n\n[3504sub5]\nParameterName=MOD_DataOut_xxh_AU8[5]\nObjectType=0x7\nDataType=0x0005\nAccessType=rwr\n\n[3504sub6]\nParameterName=MOD_DataOut_xxh_AU8[6]\nObjectType=0x7\nDataType=0x0005\nAccessType=rwr\n\n[3504sub7]\nParameterName=MOD_DataOut_xxh_AU8[7]\nObjectType=0x7\nDataType=0x0005\nAccessType=rwr\n\n[3504sub8]\nParameterName=MOD_DataOut_xxh_AU8[8]\nObjectType=0x7\nDataType=0x0005\nAccessType=rwr\n\n[3504sub9]\nParameterName=MOD_DataOut_xxh_AU8[9]\nObjectType=0x7\nDataType=0x0005\nAccessType=rwr\n\n[3504subA]\nParameterName=MOD_DataOut_xxh_AU8[10]\nObjectType=0x7\nDataType=0x0005\nAccessType=rwr\n\n[3505]\nParameterName=MOD_DataOut_xxh_AU8\nObjectType=0x8\nSubNumber=11\n\n[3505sub0]\nParameterName=Number of Entries\nObjectType=0x7\nDataType=0x0005\nAccessType=ro\nDefaultValue=0xa\nLowLimit=0x0\nHighLimit=0xFF\n\n[3505sub1]\nParameterName=MOD_DataOut_xxh_AU8[1]\nObjectType=0x7\nDataType=0x0005\nAccessType=rwr\n\n[3505sub2]\nParameterName=MOD_DataOut_xxh_AU8[2]\nObjectType=0x7\nDataType=0x0005\nAccessType=rwr\n\n[3505sub3]\nParameterName=MOD_DataOut_xxh_AU8[3]\nObjectType=0x7\nDataType=0x0005\nAccessType=rwr\n\n[3505sub4]\nParameterName=MOD_DataOut_xxh_AU8[4]\nObjectType=0x7\nDataType=0x0005\nAccessType=rwr\n\n[3505sub5]\nParameterName=MOD_DataOut_xxh_AU8[5]\nObjectType=0x7\nDataType=0x0005\nAccessType=rwr\n\n[3505sub6]\nParameterName=MOD_DataOut_xxh_AU8[6]\nObjectType=0x7\nDataType=0x0005\nAccessType=rwr\n\n[3505sub7]\nParameterName=MOD_DataOut_xxh_AU8[7]\nObjectType=0x7\nDataType=0x0005\nAccessType=rwr\n\n[3505sub8]\nParameterName=MOD_DataOut_xxh_AU8[8]\nObjectType=0x7\nDataType=0x0005\nAccessType=rwr\n\n[3505sub9]\nParameterName=MOD_DataOut_xxh_AU8[9]\nObjectType=0x7\nDataType=0x0005\nAccessType=rwr\n\n[3505subA]\nParameterName=MOD_DataOut_xxh_AU8[10]\nObjectType=0x7\nDataType=0x0005\nAccessType=rwr\n\n[3506]\nParameterName=MOD_DataOut_xxh_AU8\nObjectType=0x8\nSubNumber=11\n\n[3506sub0]\nParameterName=Number of Entries\nObjectType=0x7\nDataType=0x0005\nAccessType=ro\nDefaultValue=0xa\nLowLimit=0x0\nHighLimit=0xFF\n\n[3506sub1]\nParameterName=MOD_DataOut_xxh_AU8[1]\nObjectType=0x7\nDataType=0x0005\nAccessType=rwr\n\n[3506sub2]\nParameterName=MOD_DataOut_xxh_AU8[2]\nObjectType=0x7\nDataType=0x0005\nAccessType=rwr\n\n[3506sub3]\nParameterName=MOD_DataOut_xxh_AU8[3]\nObjectType=0x7\nDataType=0x0005\nAccessType=rwr\n\n[3506sub4]\nParameterName=MOD_DataOut_xxh_AU8[4]\nObjectType=0x7\nDataType=0x0005\nAccessType=rwr\n\n[3506sub5]\nParameterName=MOD_DataOut_xxh_AU8[5]\nObjectType=0x7\nDataType=0x0005\nAccessType=rwr\n\n[3506sub6]\nParameterName=MOD_DataOut_xxh_AU8[6]\nObjectType=0x7\nDataType=0x0005\nAccessType=rwr\n\n[3506sub7]\nParameterName=MOD_DataOut_xxh_AU8[7]\nObjectType=0x7\nDataType=0x0005\nAccessType=rwr\n\n[3506sub8]\nParameterName=MOD_DataOut_xxh_AU8[8]\nObjectType=0x7\nDataType=0x0005\nAccessType=rwr\n\n[3506sub9]\nParameterName=MOD_DataOut_xxh_AU8[9]\nObjectType=0x7\nDataType=0x0005\nAccessType=rwr\n\n[3506subA]\nParameterName=MOD_DataOut_xxh_AU8[10]\nObjectType=0x7\nDataType=0x0005\nAccessType=rwr\n\n[3507]\nParameterName=MOD_DataOut_xxh_AU8\nObjectType=0x8\nSubNumber=11\n\n[3507sub0]\nParameterName=Number of Entries\nObjectType=0x7\nDataType=0x0005\nAccessType=ro\nDefaultValue=0xa\nLowLimit=0x0\nHighLimit=0xFF\n\n[3507sub1]\nParameterName=MOD_DataOut_xxh_AU8[1]\nObjectType=0x7\nDataType=0x0005\nAccessType=rwr\n\n[3507sub2]\nParameterName=MOD_DataOut_xxh_AU8[2]\nObjectType=0x7\nDataType=0x0005\nAccessType=rwr\n\n[3507sub3]\nParameterName=MOD_DataOut_xxh_AU8[3]\nObjectType=0x7\nDataType=0x0005\nAccessType=rwr\n\n[3507sub4]\nParameterName=MOD_DataOut_xxh_AU8[4]\nObjectType=0x7\nDataType=0x0005\nAccessType=rwr\n\n[3507sub5]\nParameterName=MOD_DataOut_xxh_AU8[5]\nObjectType=0x7\nDataType=0x0005\nAccessType=rwr\n\n[3507sub6]\nParameterName=MOD_DataOut_xxh_AU8[6]\nObjectType=0x7\nDataType=0x0005\nAccessType=rwr\n\n[3507sub7]\nParameterName=MOD_DataOut_xxh_AU8[7]\nObjectType=0x7\nDataType=0x0005\nAccessType=rwr\n\n[3507sub8]\nParameterName=MOD_DataOut_xxh_AU8[8]\nObjectType=0x7\nDataType=0x0005\nAccessType=rwr\n\n[3507sub9]\nParameterName=MOD_DataOut_xxh_AU8[9]\nObjectType=0x7\nDataType=0x0005\nAccessType=rwr\n\n[3507subA]\nParameterName=MOD_DataOut_xxh_AU8[10]\nObjectType=0x7\nDataType=0x0005\nAccessType=rwr\n\n[3508]\nParameterName=MOD_DataOut_xxh_AU8\nObjectType=0x8\nSubNumber=11\n\n[3508sub0]\nParameterName=Number of Entries\nObjectType=0x7\nDataType=0x0005\nAccessType=ro\nDefaultValue=0xa\nLowLimit=0x0\nHighLimit=0xFF\n\n[3508sub1]\nParameterName=MOD_DataOut_xxh_AU8[1]\nObjectType=0x7\nDataType=0x0005\nAccessType=rwr\n\n[3508sub2]\nParameterName=MOD_DataOut_xxh_AU8[2]\nObjectType=0x7\nDataType=0x0005\nAccessType=rwr\n\n[3508sub3]\nParameterName=MOD_DataOut_xxh_AU8[3]\nObjectType=0x7\nDataType=0x0005\nAccessType=rwr\n\n[3508sub4]\nParameterName=MOD_DataOut_xxh_AU8[4]\nObjectType=0x7\nDataType=0x0005\nAccessType=rwr\n\n[3508sub5]\nParameterName=MOD_DataOut_xxh_AU8[5]\nObjectType=0x7\nDataType=0x0005\nAccessType=rwr\n\n[3508sub6]\nParameterName=MOD_DataOut_xxh_AU8[6]\nObjectType=0x7\nDataType=0x0005\nAccessType=rwr\n\n[3508sub7]\nParameterName=MOD_DataOut_xxh_AU8[7]\nObjectType=0x7\nDataType=0x0005\nAccessType=rwr\n\n[3508sub8]\nParameterName=MOD_DataOut_xxh_AU8[8]\nObjectType=0x7\nDataType=0x0005\nAccessType=rwr\n\n[3508sub9]\nParameterName=MOD_DataOut_xxh_AU8[9]\nObjectType=0x7\nDataType=0x0005\nAccessType=rwr\n\n[3508subA]\nParameterName=MOD_DataOut_xxh_AU8[10]\nObjectType=0x7\nDataType=0x0005\nAccessType=rwr\n\n[3509]\nParameterName=MOD_DataOut_xxh_AU8\nObjectType=0x8\nSubNumber=11\n\n[3509sub0]\nParameterName=Number of Entries\nObjectType=0x7\nDataType=0x0005\nAccessType=ro\nDefaultValue=0xa\nLowLimit=0x0\nHighLimit=0xFF\n\n[3509sub1]\nParameterName=MOD_DataOut_xxh_AU8[1]\nObjectType=0x7\nDataType=0x0005\nAccessType=rwr\n\n[3509sub2]\nParameterName=MOD_DataOut_xxh_AU8[2]\nObjectType=0x7\nDataType=0x0005\nAccessType=rwr\n\n[3509sub3]\nParameterName=MOD_DataOut_xxh_AU8[3]\nObjectType=0x7\nDataType=0x0005\nAccessType=rwr\n\n[3509sub4]\nParameterName=MOD_DataOut_xxh_AU8[4]\nObjectType=0x7\nDataType=0x0005\nAccessType=rwr\n\n[3509sub5]\nParameterName=MOD_DataOut_xxh_AU8[5]\nObjectType=0x7\nDataType=0x0005\nAccessType=rwr\n\n[3509sub6]\nParameterName=MOD_DataOut_xxh_AU8[6]\nObjectType=0x7\nDataType=0x0005\nAccessType=rwr\n\n[3509sub7]\nParameterName=MOD_DataOut_xxh_AU8[7]\nObjectType=0x7\nDataType=0x0005\nAccessType=rwr\n\n[3509sub8]\nParameterName=MOD_DataOut_xxh_AU8[8]\nObjectType=0x7\nDataType=0x0005\nAccessType=rwr\n\n[3509sub9]\nParameterName=MOD_DataOut_xxh_AU8[9]\nObjectType=0x7\nDataType=0x0005\nAccessType=rwr\n\n[3509subA]\nParameterName=MOD_DataOut_xxh_AU8[10]\nObjectType=0x7\nDataType=0x0005\nAccessType=rwr\n\n[350A]\nParameterName=MOD_DataOut_xxh_AU8\nObjectType=0x8\nSubNumber=11\n\n[350Asub0]\nParameterName=Number of Entries\nObjectType=0x7\nDataType=0x0005\nAccessType=ro\nDefaultValue=0xa\nLowLimit=0x0\nHighLimit=0xFF\n\n[350Asub1]\nParameterName=MOD_DataOut_xxh_AU8[1]\nObjectType=0x7\nDataType=0x0005\nAccessType=rwr\n\n[350Asub2]\nParameterName=MOD_DataOut_xxh_AU8[2]\nObjectType=0x7\nDataType=0x0005\nAccessType=rwr\n\n[350Asub3]\nParameterName=MOD_DataOut_xxh_AU8[3]\nObjectType=0x7\nDataType=0x0005\nAccessType=rwr\n\n[350Asub4]\nParameterName=MOD_DataOut_xxh_AU8[4]\nObjectType=0x7\nDataType=0x0005\nAccessType=rwr\n\n[350Asub5]\nParameterName=MOD_DataOut_xxh_AU8[5]\nObjectType=0x7\nDataType=0x0005\nAccessType=rwr\n\n[350Asub6]\nParameterName=MOD_DataOut_xxh_AU8[6]\nObjectType=0x7\nDataType=0x0005\nAccessType=rwr\n\n[350Asub7]\nParameterName=MOD_DataOut_xxh_AU8[7]\nObjectType=0x7\nDataType=0x0005\nAccessType=rwr\n\n[350Asub8]\nParameterName=MOD_DataOut_xxh_AU8[8]\nObjectType=0x7\nDataType=0x0005\nAccessType=rwr\n\n[350Asub9]\nParameterName=MOD_DataOut_xxh_AU8[9]\nObjectType=0x7\nDataType=0x0005\nAccessType=rwr\n\n[350AsubA]\nParameterName=MOD_DataOut_xxh_AU8[10]\nObjectType=0x7\nDataType=0x0005\nAccessType=rwr\n\n[350B]\nParameterName=MOD_DataOut_xxh_AU8\nObjectType=0x8\nSubNumber=11\n\n[350Bsub0]\nParameterName=Number of Entries\nObjectType=0x7\nDataType=0x0005\nAccessType=ro\nDefaultValue=0xa\nLowLimit=0x0\nHighLimit=0xFF\n\n[350Bsub1]\nParameterName=MOD_DataOut_xxh_AU8[1]\nObjectType=0x7\nDataType=0x0005\nAccessType=rwr\n\n[350Bsub2]\nParameterName=MOD_DataOut_xxh_AU8[2]\nObjectType=0x7\nDataType=0x0005\nAccessType=rwr\n\n[350Bsub3]\nParameterName=MOD_DataOut_xxh_AU8[3]\nObjectType=0x7\nDataType=0x0005\nAccessType=rwr\n\n[350Bsub4]\nParameterName=MOD_DataOut_xxh_AU8[4]\nObjectType=0x7\nDataType=0x0005\nAccessType=rwr\n\n[350Bsub5]\nParameterName=MOD_DataOut_xxh_AU8[5]\nObjectType=0x7\nDataType=0x0005\nAccessType=rwr\n\n[350Bsub6]\nParameterName=MOD_DataOut_xxh_AU8[6]\nObjectType=0x7\nDataType=0x0005\nAccessType=rwr\n\n[350Bsub7]\nParameterName=MOD_DataOut_xxh_AU8[7]\nObjectType=0x7\nDataType=0x0005\nAccessType=rwr\n\n[350Bsub8]\nParameterName=MOD_DataOut_xxh_AU8[8]\nObjectType=0x7\nDataType=0x0005\nAccessType=rwr\n\n[350Bsub9]\nParameterName=MOD_DataOut_xxh_AU8[9]\nObjectType=0x7\nDataType=0x0005\nAccessType=rwr\n\n[350BsubA]\nParameterName=MOD_DataOut_xxh_AU8[10]\nObjectType=0x7\nDataType=0x0005\nAccessType=rwr\n\n[350C]\nParameterName=MOD_DataOut_xxh_AU8\nObjectType=0x8\nSubNumber=11\n\n[350Csub0]\nParameterName=Number of Entries\nObjectType=0x7\nDataType=0x0005\nAccessType=ro\nDefaultValue=0xa\nLowLimit=0x0\nHighLimit=0xFF\n\n[350Csub1]\nParameterName=MOD_DataOut_xxh_AU8[1]\nObjectType=0x7\nDataType=0x0005\nAccessType=rwr\n\n[350Csub2]\nParameterName=MOD_DataOut_xxh_AU8[2]\nObjectType=0x7\nDataType=0x0005\nAccessType=rwr\n\n[350Csub3]\nParameterName=MOD_DataOut_xxh_AU8[3]\nObjectType=0x7\nDataType=0x0005\nAccessType=rwr\n\n[350Csub4]\nParameterName=MOD_DataOut_xxh_AU8[4]\nObjectType=0x7\nDataType=0x0005\nAccessType=rwr\n\n[350Csub5]\nParameterName=MOD_DataOut_xxh_AU8[5]\nObjectType=0x7\nDataType=0x0005\nAccessType=rwr\n\n[350Csub6]\nParameterName=MOD_DataOut_xxh_AU8[6]\nObjectType=0x7\nDataType=0x0005\nAccessType=rwr\n\n[350Csub7]\nParameterName=MOD_DataOut_xxh_AU8[7]\nObjectType=0x7\nDataType=0x0005\nAccessType=rwr\n\n[350Csub8]\nParameterName=MOD_DataOut_xxh_AU8[8]\nObjectType=0x7\nDataType=0x0005\nAccessType=rwr\n\n[350Csub9]\nParameterName=MOD_DataOut_xxh_AU8[9]\nObjectType=0x7\nDataType=0x0005\nAccessType=rwr\n\n[350CsubA]\nParameterName=MOD_DataOut_xxh_AU8[10]\nObjectType=0x7\nDataType=0x0005\nAccessType=rwr\n\n[350D]\nParameterName=MOD_DataOut_xxh_AU8\nObjectType=0x8\nSubNumber=11\n\n[350Dsub0]\nParameterName=Number of Entries\nObjectType=0x7\nDataType=0x0005\nAccessType=ro\nDefaultValue=0xa\nLowLimit=0x0\nHighLimit=0xFF\n\n[350Dsub1]\nParameterName=MOD_DataOut_xxh_AU8[1]\nObjectType=0x7\nDataType=0x0005\nAccessType=rwr\n\n[350Dsub2]\nParameterName=MOD_DataOut_xxh_AU8[2]\nObjectType=0x7\nDataType=0x0005\nAccessType=rwr\n\n[350Dsub3]\nParameterName=MOD_DataOut_xxh_AU8[3]\nObjectType=0x7\nDataType=0x0005\nAccessType=rwr\n\n[350Dsub4]\nParameterName=MOD_DataOut_xxh_AU8[4]\nObjectType=0x7\nDataType=0x0005\nAccessType=rwr\n\n[350Dsub5]\nParameterName=MOD_DataOut_xxh_AU8[5]\nObjectType=0x7\nDataType=0x0005\nAccessType=rwr\n\n[350Dsub6]\nParameterName=MOD_DataOut_xxh_AU8[6]\nObjectType=0x7\nDataType=0x0005\nAccessType=rwr\n\n[350Dsub7]\nParameterName=MOD_DataOut_xxh_AU8[7]\nObjectType=0x7\nDataType=0x0005\nAccessType=rwr\n\n[350Dsub8]\nParameterName=MOD_DataOut_xxh_AU8[8]\nObjectType=0x7\nDataType=0x0005\nAccessType=rwr\n\n[350Dsub9]\nParameterName=MOD_DataOut_xxh_AU8[9]\nObjectType=0x7\nDataType=0x0005\nAccessType=rwr\n\n[350DsubA]\nParameterName=MOD_DataOut_xxh_AU8[10]\nObjectType=0x7\nDataType=0x0005\nAccessType=rwr\n\n[350E]\nParameterName=MOD_DataOut_xxh_AU8\nObjectType=0x8\nSubNumber=11\n\n[350Esub0]\nParameterName=Number of Entries\nObjectType=0x7\nDataType=0x0005\nAccessType=ro\nDefaultValue=0xa\nLowLimit=0x0\nHighLimit=0xFF\n\n[350Esub1]\nParameterName=MOD_DataOut_xxh_AU8[1]\nObjectType=0x7\nDataType=0x0005\nAccessType=rwr\n\n[350Esub2]\nParameterName=MOD_DataOut_xxh_AU8[2]\nObjectType=0x7\nDataType=0x0005\nAccessType=rwr\n\n[350Esub3]\nParameterName=MOD_DataOut_xxh_AU8[3]\nObjectType=0x7\nDataType=0x0005\nAccessType=rwr\n\n[350Esub4]\nParameterName=MOD_DataOut_xxh_AU8[4]\nObjectType=0x7\nDataType=0x0005\nAccessType=rwr\n\n[350Esub5]\nParameterName=MOD_DataOut_xxh_AU8[5]\nObjectType=0x7\nDataType=0x0005\nAccessType=rwr\n\n[350Esub6]\nParameterName=MOD_DataOut_xxh_AU8[6]\nObjectType=0x7\nDataType=0x0005\nAccessType=rwr\n\n[350Esub7]\nParameterName=MOD_DataOut_xxh_AU8[7]\nObjectType=0x7\nDataType=0x0005\nAccessType=rwr\n\n[350Esub8]\nParameterName=MOD_DataOut_xxh_AU8[8]\nObjectType=0x7\nDataType=0x0005\nAccessType=rwr\n\n[350Esub9]\nParameterName=MOD_DataOut_xxh_AU8[9]\nObjectType=0x7\nDataType=0x0005\nAccessType=rwr\n\n[350EsubA]\nParameterName=MOD_DataOut_xxh_AU8[10]\nObjectType=0x7\nDataType=0x0005\nAccessType=rwr\n\n[350F]\nParameterName=MOD_DataOut_xxh_AU8\nObjectType=0x8\nSubNumber=11\n\n[350Fsub0]\nParameterName=Number of Entries\nObjectType=0x7\nDataType=0x0005\nAccessType=ro\nDefaultValue=0xa\nLowLimit=0x0\nHighLimit=0xFF\n\n[350Fsub1]\nParameterName=MOD_DataOut_xxh_AU8[1]\nObjectType=0x7\nDataType=0x0005\nAccessType=rwr\n\n[350Fsub2]\nParameterName=MOD_DataOut_xxh_AU8[2]\nObjectType=0x7\nDataType=0x0005\nAccessType=rwr\n\n[350Fsub3]\nParameterName=MOD_DataOut_xxh_AU8[3]\nObjectType=0x7\nDataType=0x0005\nAccessType=rwr\n\n[350Fsub4]\nParameterName=MOD_DataOut_xxh_AU8[4]\nObjectType=0x7\nDataType=0x0005\nAccessType=rwr\n\n[350Fsub5]\nParameterName=MOD_DataOut_xxh_AU8[5]\nObjectType=0x7\nDataType=0x0005\nAccessType=rwr\n\n[350Fsub6]\nParameterName=MOD_DataOut_xxh_AU8[6]\nObjectType=0x7\nDataType=0x0005\nAccessType=rwr\n\n[350Fsub7]\nParameterName=MOD_DataOut_xxh_AU8[7]\nObjectType=0x7\nDataType=0x0005\nAccessType=rwr\n\n[350Fsub8]\nParameterName=MOD_DataOut_xxh_AU8[8]\nObjectType=0x7\nDataType=0x0005\nAccessType=rwr\n\n[350Fsub9]\nParameterName=MOD_DataOut_xxh_AU8[9]\nObjectType=0x7\nDataType=0x0005\nAccessType=rwr\n\n[350FsubA]\nParameterName=MOD_DataOut_xxh_AU8[10]\nObjectType=0x7\nDataType=0x0005\nAccessType=rwr\n\n[3510]\nParameterName=MOD_DataOut_xxh_AU8\nObjectType=0x8\nSubNumber=11\n\n[3510sub0]\nParameterName=Number of Entries\nObjectType=0x7\nDataType=0x0005\nAccessType=ro\nDefaultValue=0xa\nLowLimit=0x0\nHighLimit=0xFF\n\n[3510sub1]\nParameterName=MOD_DataOut_xxh_AU8[1]\nObjectType=0x7\nDataType=0x0005\nAccessType=rwr\n\n[3510sub2]\nParameterName=MOD_DataOut_xxh_AU8[2]\nObjectType=0x7\nDataType=0x0005\nAccessType=rwr\n\n[3510sub3]\nParameterName=MOD_DataOut_xxh_AU8[3]\nObjectType=0x7\nDataType=0x0005\nAccessType=rwr\n\n[3510sub4]\nParameterName=MOD_DataOut_xxh_AU8[4]\nObjectType=0x7\nDataType=0x0005\nAccessType=rwr\n\n[3510sub5]\nParameterName=MOD_DataOut_xxh_AU8[5]\nObjectType=0x7\nDataType=0x0005\nAccessType=rwr\n\n[3510sub6]\nParameterName=MOD_DataOut_xxh_AU8[6]\nObjectType=0x7\nDataType=0x0005\nAccessType=rwr\n\n[3510sub7]\nParameterName=MOD_DataOut_xxh_AU8[7]\nObjectType=0x7\nDataType=0x0005\nAccessType=rwr\n\n[3510sub8]\nParameterName=MOD_DataOut_xxh_AU8[8]\nObjectType=0x7\nDataType=0x0005\nAccessType=rwr\n\n[3510sub9]\nParameterName=MOD_DataOut_xxh_AU8[9]\nObjectType=0x7\nDataType=0x0005\nAccessType=rwr\n\n[3510subA]\nParameterName=MOD_DataOut_xxh_AU8[10]\nObjectType=0x7\nDataType=0x0005\nAccessType=rwr\n\n[3511]\nParameterName=MOD_DataOut_xxh_AU8\nObjectType=0x8\nSubNumber=11\n\n[3511sub0]\nParameterName=Number of Entries\nObjectType=0x7\nDataType=0x0005\nAccessType=ro\nDefaultValue=0xa\nLowLimit=0x0\nHighLimit=0xFF\n\n[3511sub1]\nParameterName=MOD_DataOut_xxh_AU8[1]\nObjectType=0x7\nDataType=0x0005\nAccessType=rwr\n\n[3511sub2]\nParameterName=MOD_DataOut_xxh_AU8[2]\nObjectType=0x7\nDataType=0x0005\nAccessType=rwr\n\n[3511sub3]\nParameterName=MOD_DataOut_xxh_AU8[3]\nObjectType=0x7\nDataType=0x0005\nAccessType=rwr\n\n[3511sub4]\nParameterName=MOD_DataOut_xxh_AU8[4]\nObjectType=0x7\nDataType=0x0005\nAccessType=rwr\n\n[3511sub5]\nParameterName=MOD_DataOut_xxh_AU8[5]\nObjectType=0x7\nDataType=0x0005\nAccessType=rwr\n\n[3511sub6]\nParameterName=MOD_DataOut_xxh_AU8[6]\nObjectType=0x7\nDataType=0x0005\nAccessType=rwr\n\n[3511sub7]\nParameterName=MOD_DataOut_xxh_AU8[7]\nObjectType=0x7\nDataType=0x0005\nAccessType=rwr\n\n[3511sub8]\nParameterName=MOD_DataOut_xxh_AU8[8]\nObjectType=0x7\nDataType=0x0005\nAccessType=rwr\n\n[3511sub9]\nParameterName=MOD_DataOut_xxh_AU8[9]\nObjectType=0x7\nDataType=0x0005\nAccessType=rwr\n\n[3511subA]\nParameterName=MOD_DataOut_xxh_AU8[10]\nObjectType=0x7\nDataType=0x0005\nAccessType=rwr\n\n[3512]\nParameterName=MOD_DataOut_xxh_AU8\nObjectType=0x8\nSubNumber=11\n\n[3512sub0]\nParameterName=Number of Entries\nObjectType=0x7\nDataType=0x0005\nAccessType=ro\nDefaultValue=0xa\nLowLimit=0x0\nHighLimit=0xFF\n\n[3512sub1]\nParameterName=MOD_DataOut_xxh_AU8[1]\nObjectType=0x7\nDataType=0x0005\nAccessType=rwr\n\n[3512sub2]\nParameterName=MOD_DataOut_xxh_AU8[2]\nObjectType=0x7\nDataType=0x0005\nAccessType=rwr\n\n[3512sub3]\nParameterName=MOD_DataOut_xxh_AU8[3]\nObjectType=0x7\nDataType=0x0005\nAccessType=rwr\n\n[3512sub4]\nParameterName=MOD_DataOut_xxh_AU8[4]\nObjectType=0x7\nDataType=0x0005\nAccessType=rwr\n\n[3512sub5]\nParameterName=MOD_DataOut_xxh_AU8[5]\nObjectType=0x7\nDataType=0x0005\nAccessType=rwr\n\n[3512sub6]\nParameterName=MOD_DataOut_xxh_AU8[6]\nObjectType=0x7\nDataType=0x0005\nAccessType=rwr\n\n[3512sub7]\nParameterName=MOD_DataOut_xxh_AU8[7]\nObjectType=0x7\nDataType=0x0005\nAccessType=rwr\n\n[3512sub8]\nParameterName=MOD_DataOut_xxh_AU8[8]\nObjectType=0x7\nDataType=0x0005\nAccessType=rwr\n\n[3512sub9]\nParameterName=MOD_DataOut_xxh_AU8[9]\nObjectType=0x7\nDataType=0x0005\nAccessType=rwr\n\n[3512subA]\nParameterName=MOD_DataOut_xxh_AU8[10]\nObjectType=0x7\nDataType=0x0005\nAccessType=rwr\n\n[3513]\nParameterName=MOD_DataOut_xxh_AU8\nObjectType=0x8\nSubNumber=11\n\n[3513sub0]\nParameterName=Number of Entries\nObjectType=0x7\nDataType=0x0005\nAccessType=ro\nDefaultValue=0xa\nLowLimit=0x0\nHighLimit=0xFF\n\n[3513sub1]\nParameterName=MOD_DataOut_xxh_AU8[1]\nObjectType=0x7\nDataType=0x0005\nAccessType=rwr\n\n[3513sub2]\nParameterName=MOD_DataOut_xxh_AU8[2]\nObjectType=0x7\nDataType=0x0005\nAccessType=rwr\n\n[3513sub3]\nParameterName=MOD_DataOut_xxh_AU8[3]\nObjectType=0x7\nDataType=0x0005\nAccessType=rwr\n\n[3513sub4]\nParameterName=MOD_DataOut_xxh_AU8[4]\nObjectType=0x7\nDataType=0x0005\nAccessType=rwr\n\n[3513sub5]\nParameterName=MOD_DataOut_xxh_AU8[5]\nObjectType=0x7\nDataType=0x0005\nAccessType=rwr\n\n[3513sub6]\nParameterName=MOD_DataOut_xxh_AU8[6]\nObjectType=0x7\nDataType=0x0005\nAccessType=rwr\n\n[3513sub7]\nParameterName=MOD_DataOut_xxh_AU8[7]\nObjectType=0x7\nDataType=0x0005\nAccessType=rwr\n\n[3513sub8]\nParameterName=MOD_DataOut_xxh_AU8[8]\nObjectType=0x7\nDataType=0x0005\nAccessType=rwr\n\n[3513sub9]\nParameterName=MOD_DataOut_xxh_AU8[9]\nObjectType=0x7\nDataType=0x0005\nAccessType=rwr\n\n[3513subA]\nParameterName=MOD_DataOut_xxh_AU8[10]\nObjectType=0x7\nDataType=0x0005\nAccessType=rwr\n\n[3600]\nParameterName=MOD_DataOut_xxh_AU16\nObjectType=0x8\nSubNumber=11\n\n[3600sub0]\nParameterName=Number of Entries\nObjectType=0x7\nDataType=0x0005\nAccessType=ro\nDefaultValue=0xA\nLowLimit=0x0\nHighLimit=0xFF\n\n[3600sub1]\nParameterName=MOD_DataOut_xxh_AU16[1]\nObjectType=0x7\nDataType=0x0006\nAccessType=rwr\n\n[3600sub2]\nParameterName=MOD_DataOut_xxh_AU16[2]\nObjectType=0x7\nDataType=0x0006\nAccessType=rwr\n\n[3600sub3]\nParameterName=MOD_DataOut_xxh_AU16[3]\nObjectType=0x7\nDataType=0x0006\nAccessType=rwr\n\n[3600sub4]\nParameterName=MOD_DataOut_xxh_AU16[4]\nObjectType=0x7\nDataType=0x0006\nAccessType=rwr\n\n[3600sub5]\nParameterName=MOD_DataOut_xxh_AU16[5]\nObjectType=0x7\nDataType=0x0006\nAccessType=rwr\n\n[3600sub6]\nParameterName=MOD_DataOut_xxh_AU16[6]\nObjectType=0x7\nDataType=0x0006\nAccessType=rwr\n\n[3600sub7]\nParameterName=MOD_DataOut_xxh_AU16[7]\nObjectType=0x7\nDataType=0x0006\nAccessType=rwr\n\n[3600sub8]\nParameterName=MOD_DataOut_xxh_AU16[8]\nObjectType=0x7\nDataType=0x0006\nAccessType=rwr\n\n[3600sub9]\nParameterName=MOD_DataOut_xxh_AU16[9]\nObjectType=0x7\nDataType=0x0006\nAccessType=rwr\n\n[3600subA]\nParameterName=MOD_DataOut_xxh_AU16[10]\nObjectType=0x7\nDataType=0x0006\nAccessType=rwr\n\n[3601]\nParameterName=MOD_DataOut_xxh_AU16\nObjectType=0x8\nSubNumber=11\n\n[3601sub0]\nParameterName=Number of Entries\nObjectType=0x7\nDataType=0x0005\nAccessType=ro\nDefaultValue=0xA\nLowLimit=0x0\nHighLimit=0xFF\n\n[3601sub1]\nParameterName=MOD_DataOut_xxh_AU16[1]\nObjectType=0x7\nDataType=0x0006\nAccessType=rwr\n\n[3601sub2]\nParameterName=MOD_DataOut_xxh_AU16[2]\nObjectType=0x7\nDataType=0x0006\nAccessType=rwr\n\n[3601sub3]\nParameterName=MOD_DataOut_xxh_AU16[3]\nObjectType=0x7\nDataType=0x0006\nAccessType=rwr\n\n[3601sub4]\nParameterName=MOD_DataOut_xxh_AU16[4]\nObjectType=0x7\nDataType=0x0006\nAccessType=rwr\n\n[3601sub5]\nParameterName=MOD_DataOut_xxh_AU16[5]\nObjectType=0x7\nDataType=0x0006\nAccessType=rwr\n\n[3601sub6]\nParameterName=MOD_DataOut_xxh_AU16[6]\nObjectType=0x7\nDataType=0x0006\nAccessType=rwr\n\n[3601sub7]\nParameterName=MOD_DataOut_xxh_AU16[7]\nObjectType=0x7\nDataType=0x0006\nAccessType=rwr\n\n[3601sub8]\nParameterName=MOD_DataOut_xxh_AU16[8]\nObjectType=0x7\nDataType=0x0006\nAccessType=rwr\n\n[3601sub9]\nParameterName=MOD_DataOut_xxh_AU16[9]\nObjectType=0x7\nDataType=0x0006\nAccessType=rwr\n\n[3601subA]\nParameterName=MOD_DataOut_xxh_AU16[10]\nObjectType=0x7\nDataType=0x0006\nAccessType=rwr\n\n[3602]\nParameterName=MOD_DataOut_xxh_AU16\nObjectType=0x8\nSubNumber=11\n\n[3602sub0]\nParameterName=Number of Entries\nObjectType=0x7\nDataType=0x0005\nAccessType=ro\nDefaultValue=0xA\nLowLimit=0x0\nHighLimit=0xFF\n\n[3602sub1]\nParameterName=MOD_DataOut_xxh_AU16[1]\nObjectType=0x7\nDataType=0x0006\nAccessType=rwr\n\n[3602sub2]\nParameterName=MOD_DataOut_xxh_AU16[2]\nObjectType=0x7\nDataType=0x0006\nAccessType=rwr\n\n[3602sub3]\nParameterName=MOD_DataOut_xxh_AU16[3]\nObjectType=0x7\nDataType=0x0006\nAccessType=rwr\n\n[3602sub4]\nParameterName=MOD_DataOut_xxh_AU16[4]\nObjectType=0x7\nDataType=0x0006\nAccessType=rwr\n\n[3602sub5]\nParameterName=MOD_DataOut_xxh_AU16[5]\nObjectType=0x7\nDataType=0x0006\nAccessType=rwr\n\n[3602sub6]\nParameterName=MOD_DataOut_xxh_AU16[6]\nObjectType=0x7\nDataType=0x0006\nAccessType=rwr\n\n[3602sub7]\nParameterName=MOD_DataOut_xxh_AU16[7]\nObjectType=0x7\nDataType=0x0006\nAccessType=rwr\n\n[3602sub8]\nParameterName=MOD_DataOut_xxh_AU16[8]\nObjectType=0x7\nDataType=0x0006\nAccessType=rwr\n\n[3602sub9]\nParameterName=MOD_DataOut_xxh_AU16[9]\nObjectType=0x7\nDataType=0x0006\nAccessType=rwr\n\n[3602subA]\nParameterName=MOD_DataOut_xxh_AU16[10]\nObjectType=0x7\nDataType=0x0006\nAccessType=rwr\n\n[3603]\nParameterName=MOD_DataOut_xxh_AU16\nObjectType=0x8\nSubNumber=11\n\n[3603sub0]\nParameterName=Number of Entries\nObjectType=0x7\nDataType=0x0005\nAccessType=ro\nDefaultValue=0xA\nLowLimit=0x0\nHighLimit=0xFF\n\n[3603sub1]\nParameterName=MOD_DataOut_xxh_AU16[1]\nObjectType=0x7\nDataType=0x0006\nAccessType=rwr\n\n[3603sub2]\nParameterName=MOD_DataOut_xxh_AU16[2]\nObjectType=0x7\nDataType=0x0006\nAccessType=rwr\n\n[3603sub3]\nParameterName=MOD_DataOut_xxh_AU16[3]\nObjectType=0x7\nDataType=0x0006\nAccessType=rwr\n\n[3603sub4]\nParameterName=MOD_DataOut_xxh_AU16[4]\nObjectType=0x7\nDataType=0x0006\nAccessType=rwr\n\n[3603sub5]\nParameterName=MOD_DataOut_xxh_AU16[5]\nObjectType=0x7\nDataType=0x0006\nAccessType=rwr\n\n[3603sub6]\nParameterName=MOD_DataOut_xxh_AU16[6]\nObjectType=0x7\nDataType=0x0006\nAccessType=rwr\n\n[3603sub7]\nParameterName=MOD_DataOut_xxh_AU16[7]\nObjectType=0x7\nDataType=0x0006\nAccessType=rwr\n\n[3603sub8]\nParameterName=MOD_DataOut_xxh_AU16[8]\nObjectType=0x7\nDataType=0x0006\nAccessType=rwr\n\n[3603sub9]\nParameterName=MOD_DataOut_xxh_AU16[9]\nObjectType=0x7\nDataType=0x0006\nAccessType=rwr\n\n[3603subA]\nParameterName=MOD_DataOut_xxh_AU16[10]\nObjectType=0x7\nDataType=0x0006\nAccessType=rwr\n\n[3604]\nParameterName=MOD_DataOut_xxh_AU16\nObjectType=0x8\nSubNumber=11\n\n[3604sub0]\nParameterName=Number of Entries\nObjectType=0x7\nDataType=0x0005\nAccessType=ro\nDefaultValue=0xA\nLowLimit=0x0\nHighLimit=0xFF\n\n[3604sub1]\nParameterName=MOD_DataOut_xxh_AU16[1]\nObjectType=0x7\nDataType=0x0006\nAccessType=rwr\n\n[3604sub2]\nParameterName=MOD_DataOut_xxh_AU16[2]\nObjectType=0x7\nDataType=0x0006\nAccessType=rwr\n\n[3604sub3]\nParameterName=MOD_DataOut_xxh_AU16[3]\nObjectType=0x7\nDataType=0x0006\nAccessType=rwr\n\n[3604sub4]\nParameterName=MOD_DataOut_xxh_AU16[4]\nObjectType=0x7\nDataType=0x0006\nAccessType=rwr\n\n[3604sub5]\nParameterName=MOD_DataOut_xxh_AU16[5]\nObjectType=0x7\nDataType=0x0006\nAccessType=rwr\n\n[3604sub6]\nParameterName=MOD_DataOut_xxh_AU16[6]\nObjectType=0x7\nDataType=0x0006\nAccessType=rwr\n\n[3604sub7]\nParameterName=MOD_DataOut_xxh_AU16[7]\nObjectType=0x7\nDataType=0x0006\nAccessType=rwr\n\n[3604sub8]\nParameterName=MOD_DataOut_xxh_AU16[8]\nObjectType=0x7\nDataType=0x0006\nAccessType=rwr\n\n[3604sub9]\nParameterName=MOD_DataOut_xxh_AU16[9]\nObjectType=0x7\nDataType=0x0006\nAccessType=rwr\n\n[3604subA]\nParameterName=MOD_DataOut_xxh_AU16[10]\nObjectType=0x7\nDataType=0x0006\nAccessType=rwr\n\n[3605]\nParameterName=MOD_DataOut_xxh_AU16\nObjectType=0x8\nSubNumber=11\n\n[3605sub0]\nParameterName=Number of Entries\nObjectType=0x7\nDataType=0x0005\nAccessType=ro\nDefaultValue=0xA\nLowLimit=0x0\nHighLimit=0xFF\n\n[3605sub1]\nParameterName=MOD_DataOut_xxh_AU16[1]\nObjectType=0x7\nDataType=0x0006\nAccessType=rwr\n\n[3605sub2]\nParameterName=MOD_DataOut_xxh_AU16[2]\nObjectType=0x7\nDataType=0x0006\nAccessType=rwr\n\n[3605sub3]\nParameterName=MOD_DataOut_xxh_AU16[3]\nObjectType=0x7\nDataType=0x0006\nAccessType=rwr\n\n[3605sub4]\nParameterName=MOD_DataOut_xxh_AU16[4]\nObjectType=0x7\nDataType=0x0006\nAccessType=rwr\n\n[3605sub5]\nParameterName=MOD_DataOut_xxh_AU16[5]\nObjectType=0x7\nDataType=0x0006\nAccessType=rwr\n\n[3605sub6]\nParameterName=MOD_DataOut_xxh_AU16[6]\nObjectType=0x7\nDataType=0x0006\nAccessType=rwr\n\n[3605sub7]\nParameterName=MOD_DataOut_xxh_AU16[7]\nObjectType=0x7\nDataType=0x0006\nAccessType=rwr\n\n[3605sub8]\nParameterName=MOD_DataOut_xxh_AU16[8]\nObjectType=0x7\nDataType=0x0006\nAccessType=rwr\n\n[3605sub9]\nParameterName=MOD_DataOut_xxh_AU16[9]\nObjectType=0x7\nDataType=0x0006\nAccessType=rwr\n\n[3605subA]\nParameterName=MOD_DataOut_xxh_AU16[10]\nObjectType=0x7\nDataType=0x0006\nAccessType=rwr\n\n[3606]\nParameterName=MOD_DataOut_xxh_AU16\nObjectType=0x8\nSubNumber=11\n\n[3606sub0]\nParameterName=Number of Entries\nObjectType=0x7\nDataType=0x0005\nAccessType=ro\nDefaultValue=0xA\nLowLimit=0x0\nHighLimit=0xFF\n\n[3606sub1]\nParameterName=MOD_DataOut_xxh_AU16[1]\nObjectType=0x7\nDataType=0x0006\nAccessType=rwr\n\n[3606sub2]\nParameterName=MOD_DataOut_xxh_AU16[2]\nObjectType=0x7\nDataType=0x0006\nAccessType=rwr\n\n[3606sub3]\nParameterName=MOD_DataOut_xxh_AU16[3]\nObjectType=0x7\nDataType=0x0006\nAccessType=rwr\n\n[3606sub4]\nParameterName=MOD_DataOut_xxh_AU16[4]\nObjectType=0x7\nDataType=0x0006\nAccessType=rwr\n\n[3606sub5]\nParameterName=MOD_DataOut_xxh_AU16[5]\nObjectType=0x7\nDataType=0x0006\nAccessType=rwr\n\n[3606sub6]\nParameterName=MOD_DataOut_xxh_AU16[6]\nObjectType=0x7\nDataType=0x0006\nAccessType=rwr\n\n[3606sub7]\nParameterName=MOD_DataOut_xxh_AU16[7]\nObjectType=0x7\nDataType=0x0006\nAccessType=rwr\n\n[3606sub8]\nParameterName=MOD_DataOut_xxh_AU16[8]\nObjectType=0x7\nDataType=0x0006\nAccessType=rwr\n\n[3606sub9]\nParameterName=MOD_DataOut_xxh_AU16[9]\nObjectType=0x7\nDataType=0x0006\nAccessType=rwr\n\n[3606subA]\nParameterName=MOD_DataOut_xxh_AU16[10]\nObjectType=0x7\nDataType=0x0006\nAccessType=rwr\n\n[3607]\nParameterName=MOD_DataOut_xxh_AU16\nObjectType=0x8\nSubNumber=11\n\n[3607sub0]\nParameterName=Number of Entries\nObjectType=0x7\nDataType=0x0005\nAccessType=ro\nDefaultValue=0xA\nLowLimit=0x0\nHighLimit=0xFF\n\n[3607sub1]\nParameterName=MOD_DataOut_xxh_AU16[1]\nObjectType=0x7\nDataType=0x0006\nAccessType=rwr\n\n[3607sub2]\nParameterName=MOD_DataOut_xxh_AU16[2]\nObjectType=0x7\nDataType=0x0006\nAccessType=rwr\n\n[3607sub3]\nParameterName=MOD_DataOut_xxh_AU16[3]\nObjectType=0x7\nDataType=0x0006\nAccessType=rwr\n\n[3607sub4]\nParameterName=MOD_DataOut_xxh_AU16[4]\nObjectType=0x7\nDataType=0x0006\nAccessType=rwr\n\n[3607sub5]\nParameterName=MOD_DataOut_xxh_AU16[5]\nObjectType=0x7\nDataType=0x0006\nAccessType=rwr\n\n[3607sub6]\nParameterName=MOD_DataOut_xxh_AU16[6]\nObjectType=0x7\nDataType=0x0006\nAccessType=rwr\n\n[3607sub7]\nParameterName=MOD_DataOut_xxh_AU16[7]\nObjectType=0x7\nDataType=0x0006\nAccessType=rwr\n\n[3607sub8]\nParameterName=MOD_DataOut_xxh_AU16[8]\nObjectType=0x7\nDataType=0x0006\nAccessType=rwr\n\n[3607sub9]\nParameterName=MOD_DataOut_xxh_AU16[9]\nObjectType=0x7\nDataType=0x0006\nAccessType=rwr\n\n[3607subA]\nParameterName=MOD_DataOut_xxh_AU16[10]\nObjectType=0x7\nDataType=0x0006\nAccessType=rwr\n\n[3608]\nParameterName=MOD_DataOut_xxh_AU16\nObjectType=0x8\nSubNumber=11\n\n[3608sub0]\nParameterName=Number of Entries\nObjectType=0x7\nDataType=0x0005\nAccessType=ro\nDefaultValue=0xA\nLowLimit=0x0\nHighLimit=0xFF\n\n[3608sub1]\nParameterName=MOD_DataOut_xxh_AU16[1]\nObjectType=0x7\nDataType=0x0006\nAccessType=rwr\n\n[3608sub2]\nParameterName=MOD_DataOut_xxh_AU16[2]\nObjectType=0x7\nDataType=0x0006\nAccessType=rwr\n\n[3608sub3]\nParameterName=MOD_DataOut_xxh_AU16[3]\nObjectType=0x7\nDataType=0x0006\nAccessType=rwr\n\n[3608sub4]\nParameterName=MOD_DataOut_xxh_AU16[4]\nObjectType=0x7\nDataType=0x0006\nAccessType=rwr\n\n[3608sub5]\nParameterName=MOD_DataOut_xxh_AU16[5]\nObjectType=0x7\nDataType=0x0006\nAccessType=rwr\n\n[3608sub6]\nParameterName=MOD_DataOut_xxh_AU16[6]\nObjectType=0x7\nDataType=0x0006\nAccessType=rwr\n\n[3608sub7]\nParameterName=MOD_DataOut_xxh_AU16[7]\nObjectType=0x7\nDataType=0x0006\nAccessType=rwr\n\n[3608sub8]\nParameterName=MOD_DataOut_xxh_AU16[8]\nObjectType=0x7\nDataType=0x0006\nAccessType=rwr\n\n[3608sub9]\nParameterName=MOD_DataOut_xxh_AU16[9]\nObjectType=0x7\nDataType=0x0006\nAccessType=rwr\n\n[3608subA]\nParameterName=MOD_DataOut_xxh_AU16[10]\nObjectType=0x7\nDataType=0x0006\nAccessType=rwr\n\n[3609]\nParameterName=MOD_DataOut_xxh_AU16\nObjectType=0x8\nSubNumber=11\n\n[3609sub0]\nParameterName=Number of Entries\nObjectType=0x7\nDataType=0x0005\nAccessType=ro\nDefaultValue=0xA\nLowLimit=0x0\nHighLimit=0xFF\n\n[3609sub1]\nParameterName=MOD_DataOut_xxh_AU16[1]\nObjectType=0x7\nDataType=0x0006\nAccessType=rwr\n\n[3609sub2]\nParameterName=MOD_DataOut_xxh_AU16[2]\nObjectType=0x7\nDataType=0x0006\nAccessType=rwr\n\n[3609sub3]\nParameterName=MOD_DataOut_xxh_AU16[3]\nObjectType=0x7\nDataType=0x0006\nAccessType=rwr\n\n[3609sub4]\nParameterName=MOD_DataOut_xxh_AU16[4]\nObjectType=0x7\nDataType=0x0006\nAccessType=rwr\n\n[3609sub5]\nParameterName=MOD_DataOut_xxh_AU16[5]\nObjectType=0x7\nDataType=0x0006\nAccessType=rwr\n\n[3609sub6]\nParameterName=MOD_DataOut_xxh_AU16[6]\nObjectType=0x7\nDataType=0x0006\nAccessType=rwr\n\n[3609sub7]\nParameterName=MOD_DataOut_xxh_AU16[7]\nObjectType=0x7\nDataType=0x0006\nAccessType=rwr\n\n[3609sub8]\nParameterName=MOD_DataOut_xxh_AU16[8]\nObjectType=0x7\nDataType=0x0006\nAccessType=rwr\n\n[3609sub9]\nParameterName=MOD_DataOut_xxh_AU16[9]\nObjectType=0x7\nDataType=0x0006\nAccessType=rwr\n\n[3609subA]\nParameterName=MOD_DataOut_xxh_AU16[10]\nObjectType=0x7\nDataType=0x0006\nAccessType=rwr\n\n[360A]\nParameterName=MOD_DataOut_xxh_AU16\nObjectType=0x8\nSubNumber=11\n\n[360Asub0]\nParameterName=Number of Entries\nObjectType=0x7\nDataType=0x0005\nAccessType=ro\nDefaultValue=0xA\nLowLimit=0x0\nHighLimit=0xFF\n\n[360Asub1]\nParameterName=MOD_DataOut_xxh_AU16[1]\nObjectType=0x7\nDataType=0x0006\nAccessType=rwr\n\n[360Asub2]\nParameterName=MOD_DataOut_xxh_AU16[2]\nObjectType=0x7\nDataType=0x0006\nAccessType=rwr\n\n[360Asub3]\nParameterName=MOD_DataOut_xxh_AU16[3]\nObjectType=0x7\nDataType=0x0006\nAccessType=rwr\n\n[360Asub4]\nParameterName=MOD_DataOut_xxh_AU16[4]\nObjectType=0x7\nDataType=0x0006\nAccessType=rwr\n\n[360Asub5]\nParameterName=MOD_DataOut_xxh_AU16[5]\nObjectType=0x7\nDataType=0x0006\nAccessType=rwr\n\n[360Asub6]\nParameterName=MOD_DataOut_xxh_AU16[6]\nObjectType=0x7\nDataType=0x0006\nAccessType=rwr\n\n[360Asub7]\nParameterName=MOD_DataOut_xxh_AU16[7]\nObjectType=0x7\nDataType=0x0006\nAccessType=rwr\n\n[360Asub8]\nParameterName=MOD_DataOut_xxh_AU16[8]\nObjectType=0x7\nDataType=0x0006\nAccessType=rwr\n\n[360Asub9]\nParameterName=MOD_DataOut_xxh_AU16[9]\nObjectType=0x7\nDataType=0x0006\nAccessType=rwr\n\n[360AsubA]\nParameterName=MOD_DataOut_xxh_AU16[10]\nObjectType=0x7\nDataType=0x0006\nAccessType=rwr\n\n[360B]\nParameterName=MOD_DataOut_xxh_AU16\nObjectType=0x8\nSubNumber=11\n\n[360Bsub0]\nParameterName=Number of Entries\nObjectType=0x7\nDataType=0x0005\nAccessType=ro\nDefaultValue=0xA\nLowLimit=0x0\nHighLimit=0xFF\n\n[360Bsub1]\nParameterName=MOD_DataOut_xxh_AU16[1]\nObjectType=0x7\nDataType=0x0006\nAccessType=rwr\n\n[360Bsub2]\nParameterName=MOD_DataOut_xxh_AU16[2]\nObjectType=0x7\nDataType=0x0006\nAccessType=rwr\n\n[360Bsub3]\nParameterName=MOD_DataOut_xxh_AU16[3]\nObjectType=0x7\nDataType=0x0006\nAccessType=rwr\n\n[360Bsub4]\nParameterName=MOD_DataOut_xxh_AU16[4]\nObjectType=0x7\nDataType=0x0006\nAccessType=rwr\n\n[360Bsub5]\nParameterName=MOD_DataOut_xxh_AU16[5]\nObjectType=0x7\nDataType=0x0006\nAccessType=rwr\n\n[360Bsub6]\nParameterName=MOD_DataOut_xxh_AU16[6]\nObjectType=0x7\nDataType=0x0006\nAccessType=rwr\n\n[360Bsub7]\nParameterName=MOD_DataOut_xxh_AU16[7]\nObjectType=0x7\nDataType=0x0006\nAccessType=rwr\n\n[360Bsub8]\nParameterName=MOD_DataOut_xxh_AU16[8]\nObjectType=0x7\nDataType=0x0006\nAccessType=rwr\n\n[360Bsub9]\nParameterName=MOD_DataOut_xxh_AU16[9]\nObjectType=0x7\nDataType=0x0006\nAccessType=rwr\n\n[360BsubA]\nParameterName=MOD_DataOut_xxh_AU16[10]\nObjectType=0x7\nDataType=0x0006\nAccessType=rwr\n\n[360C]\nParameterName=MOD_DataOut_xxh_AU16\nObjectType=0x8\nSubNumber=11\n\n[360Csub0]\nParameterName=Number of Entries\nObjectType=0x7\nDataType=0x0005\nAccessType=ro\nDefaultValue=0xA\nLowLimit=0x0\nHighLimit=0xFF\n\n[360Csub1]\nParameterName=MOD_DataOut_xxh_AU16[1]\nObjectType=0x7\nDataType=0x0006\nAccessType=rwr\n\n[360Csub2]\nParameterName=MOD_DataOut_xxh_AU16[2]\nObjectType=0x7\nDataType=0x0006\nAccessType=rwr\n\n[360Csub3]\nParameterName=MOD_DataOut_xxh_AU16[3]\nObjectType=0x7\nDataType=0x0006\nAccessType=rwr\n\n[360Csub4]\nParameterName=MOD_DataOut_xxh_AU16[4]\nObjectType=0x7\nDataType=0x0006\nAccessType=rwr\n\n[360Csub5]\nParameterName=MOD_DataOut_xxh_AU16[5]\nObjectType=0x7\nDataType=0x0006\nAccessType=rwr\n\n[360Csub6]\nParameterName=MOD_DataOut_xxh_AU16[6]\nObjectType=0x7\nDataType=0x0006\nAccessType=rwr\n\n[360Csub7]\nParameterName=MOD_DataOut_xxh_AU16[7]\nObjectType=0x7\nDataType=0x0006\nAccessType=rwr\n\n[360Csub8]\nParameterName=MOD_DataOut_xxh_AU16[8]\nObjectType=0x7\nDataType=0x0006\nAccessType=rwr\n\n[360Csub9]\nParameterName=MOD_DataOut_xxh_AU16[9]\nObjectType=0x7\nDataType=0x0006\nAccessType=rwr\n\n[360CsubA]\nParameterName=MOD_DataOut_xxh_AU16[10]\nObjectType=0x7\nDataType=0x0006\nAccessType=rwr\n\n[360D]\nParameterName=MOD_DataOut_xxh_AU16\nObjectType=0x8\nSubNumber=11\n\n[360Dsub0]\nParameterName=Number of Entries\nObjectType=0x7\nDataType=0x0005\nAccessType=ro\nDefaultValue=0xA\nLowLimit=0x0\nHighLimit=0xFF\n\n[360Dsub1]\nParameterName=MOD_DataOut_xxh_AU16[1]\nObjectType=0x7\nDataType=0x0006\nAccessType=rwr\n\n[360Dsub2]\nParameterName=MOD_DataOut_xxh_AU16[2]\nObjectType=0x7\nDataType=0x0006\nAccessType=rwr\n\n[360Dsub3]\nParameterName=MOD_DataOut_xxh_AU16[3]\nObjectType=0x7\nDataType=0x0006\nAccessType=rwr\n\n[360Dsub4]\nParameterName=MOD_DataOut_xxh_AU16[4]\nObjectType=0x7\nDataType=0x0006\nAccessType=rwr\n\n[360Dsub5]\nParameterName=MOD_DataOut_xxh_AU16[5]\nObjectType=0x7\nDataType=0x0006\nAccessType=rwr\n\n[360Dsub6]\nParameterName=MOD_DataOut_xxh_AU16[6]\nObjectType=0x7\nDataType=0x0006\nAccessType=rwr\n\n[360Dsub7]\nParameterName=MOD_DataOut_xxh_AU16[7]\nObjectType=0x7\nDataType=0x0006\nAccessType=rwr\n\n[360Dsub8]\nParameterName=MOD_DataOut_xxh_AU16[8]\nObjectType=0x7\nDataType=0x0006\nAccessType=rwr\n\n[360Dsub9]\nParameterName=MOD_DataOut_xxh_AU16[9]\nObjectType=0x7\nDataType=0x0006\nAccessType=rwr\n\n[360DsubA]\nParameterName=MOD_DataOut_xxh_AU16[10]\nObjectType=0x7\nDataType=0x0006\nAccessType=rwr\n\n[360E]\nParameterName=MOD_DataOut_xxh_AU16\nObjectType=0x8\nSubNumber=11\n\n[360Esub0]\nParameterName=Number of Entries\nObjectType=0x7\nDataType=0x0005\nAccessType=ro\nDefaultValue=0xA\nLowLimit=0x0\nHighLimit=0xFF\n\n[360Esub1]\nParameterName=MOD_DataOut_xxh_AU16[1]\nObjectType=0x7\nDataType=0x0006\nAccessType=rwr\n\n[360Esub2]\nParameterName=MOD_DataOut_xxh_AU16[2]\nObjectType=0x7\nDataType=0x0006\nAccessType=rwr\n\n[360Esub3]\nParameterName=MOD_DataOut_xxh_AU16[3]\nObjectType=0x7\nDataType=0x0006\nAccessType=rwr\n\n[360Esub4]\nParameterName=MOD_DataOut_xxh_AU16[4]\nObjectType=0x7\nDataType=0x0006\nAccessType=rwr\n\n[360Esub5]\nParameterName=MOD_DataOut_xxh_AU16[5]\nObjectType=0x7\nDataType=0x0006\nAccessType=rwr\n\n[360Esub6]\nParameterName=MOD_DataOut_xxh_AU16[6]\nObjectType=0x7\nDataType=0x0006\nAccessType=rwr\n\n[360Esub7]\nParameterName=MOD_DataOut_xxh_AU16[7]\nObjectType=0x7\nDataType=0x0006\nAccessType=rwr\n\n[360Esub8]\nParameterName=MOD_DataOut_xxh_AU16[8]\nObjectType=0x7\nDataType=0x0006\nAccessType=rwr\n\n[360Esub9]\nParameterName=MOD_DataOut_xxh_AU16[9]\nObjectType=0x7\nDataType=0x0006\nAccessType=rwr\n\n[360EsubA]\nParameterName=MOD_DataOut_xxh_AU16[10]\nObjectType=0x7\nDataType=0x0006\nAccessType=rwr\n\n[360F]\nParameterName=MOD_DataOut_xxh_AU16\nObjectType=0x8\nSubNumber=11\n\n[360Fsub0]\nParameterName=Number of Entries\nObjectType=0x7\nDataType=0x0005\nAccessType=ro\nDefaultValue=0xA\nLowLimit=0x0\nHighLimit=0xFF\n\n[360Fsub1]\nParameterName=MOD_DataOut_xxh_AU16[1]\nObjectType=0x7\nDataType=0x0006\nAccessType=rwr\n\n[360Fsub2]\nParameterName=MOD_DataOut_xxh_AU16[2]\nObjectType=0x7\nDataType=0x0006\nAccessType=rwr\n\n[360Fsub3]\nParameterName=MOD_DataOut_xxh_AU16[3]\nObjectType=0x7\nDataType=0x0006\nAccessType=rwr\n\n[360Fsub4]\nParameterName=MOD_DataOut_xxh_AU16[4]\nObjectType=0x7\nDataType=0x0006\nAccessType=rwr\n\n[360Fsub5]\nParameterName=MOD_DataOut_xxh_AU16[5]\nObjectType=0x7\nDataType=0x0006\nAccessType=rwr\n\n[360Fsub6]\nParameterName=MOD_DataOut_xxh_AU16[6]\nObjectType=0x7\nDataType=0x0006\nAccessType=rwr\n\n[360Fsub7]\nParameterName=MOD_DataOut_xxh_AU16[7]\nObjectType=0x7\nDataType=0x0006\nAccessType=rwr\n\n[360Fsub8]\nParameterName=MOD_DataOut_xxh_AU16[8]\nObjectType=0x7\nDataType=0x0006\nAccessType=rwr\n\n[360Fsub9]\nParameterName=MOD_DataOut_xxh_AU16[9]\nObjectType=0x7\nDataType=0x0006\nAccessType=rwr\n\n[360FsubA]\nParameterName=MOD_DataOut_xxh_AU16[10]\nObjectType=0x7\nDataType=0x0006\nAccessType=rwr\n\n[3610]\nParameterName=MOD_DataOut_xxh_AU16\nObjectType=0x8\nSubNumber=11\n\n[3610sub0]\nParameterName=Number of Entries\nObjectType=0x7\nDataType=0x0005\nAccessType=ro\nDefaultValue=0xA\nLowLimit=0x0\nHighLimit=0xFF\n\n[3610sub1]\nParameterName=MOD_DataOut_xxh_AU16[1]\nObjectType=0x7\nDataType=0x0006\nAccessType=rwr\n\n[3610sub2]\nParameterName=MOD_DataOut_xxh_AU16[2]\nObjectType=0x7\nDataType=0x0006\nAccessType=rwr\n\n[3610sub3]\nParameterName=MOD_DataOut_xxh_AU16[3]\nObjectType=0x7\nDataType=0x0006\nAccessType=rwr\n\n[3610sub4]\nParameterName=MOD_DataOut_xxh_AU16[4]\nObjectType=0x7\nDataType=0x0006\nAccessType=rwr\n\n[3610sub5]\nParameterName=MOD_DataOut_xxh_AU16[5]\nObjectType=0x7\nDataType=0x0006\nAccessType=rwr\n\n[3610sub6]\nParameterName=MOD_DataOut_xxh_AU16[6]\nObjectType=0x7\nDataType=0x0006\nAccessType=rwr\n\n[3610sub7]\nParameterName=MOD_DataOut_xxh_AU16[7]\nObjectType=0x7\nDataType=0x0006\nAccessType=rwr\n\n[3610sub8]\nParameterName=MOD_DataOut_xxh_AU16[8]\nObjectType=0x7\nDataType=0x0006\nAccessType=rwr\n\n[3610sub9]\nParameterName=MOD_DataOut_xxh_AU16[9]\nObjectType=0x7\nDataType=0x0006\nAccessType=rwr\n\n[3610subA]\nParameterName=MOD_DataOut_xxh_AU16[10]\nObjectType=0x7\nDataType=0x0006\nAccessType=rwr\n\n[3611]\nParameterName=MOD_DataOut_xxh_AU16\nObjectType=0x8\nSubNumber=11\n\n[3611sub0]\nParameterName=Number of Entries\nObjectType=0x7\nDataType=0x0005\nAccessType=ro\nDefaultValue=0xA\nLowLimit=0x0\nHighLimit=0xFF\n\n[3611sub1]\nParameterName=MOD_DataOut_xxh_AU16[1]\nObjectType=0x7\nDataType=0x0006\nAccessType=rwr\n\n[3611sub2]\nParameterName=MOD_DataOut_xxh_AU16[2]\nObjectType=0x7\nDataType=0x0006\nAccessType=rwr\n\n[3611sub3]\nParameterName=MOD_DataOut_xxh_AU16[3]\nObjectType=0x7\nDataType=0x0006\nAccessType=rwr\n\n[3611sub4]\nParameterName=MOD_DataOut_xxh_AU16[4]\nObjectType=0x7\nDataType=0x0006\nAccessType=rwr\n\n[3611sub5]\nParameterName=MOD_DataOut_xxh_AU16[5]\nObjectType=0x7\nDataType=0x0006\nAccessType=rwr\n\n[3611sub6]\nParameterName=MOD_DataOut_xxh_AU16[6]\nObjectType=0x7\nDataType=0x0006\nAccessType=rwr\n\n[3611sub7]\nParameterName=MOD_DataOut_xxh_AU16[7]\nObjectType=0x7\nDataType=0x0006\nAccessType=rwr\n\n[3611sub8]\nParameterName=MOD_DataOut_xxh_AU16[8]\nObjectType=0x7\nDataType=0x0006\nAccessType=rwr\n\n[3611sub9]\nParameterName=MOD_DataOut_xxh_AU16[9]\nObjectType=0x7\nDataType=0x0006\nAccessType=rwr\n\n[3611subA]\nParameterName=MOD_DataOut_xxh_AU16[10]\nObjectType=0x7\nDataType=0x0006\nAccessType=rwr\n\n[3612]\nParameterName=MOD_DataOut_xxh_AU16\nObjectType=0x8\nSubNumber=11\n\n[3612sub0]\nParameterName=Number of Entries\nObjectType=0x7\nDataType=0x0005\nAccessType=ro\nDefaultValue=0xA\nLowLimit=0x0\nHighLimit=0xFF\n\n[3612sub1]\nParameterName=MOD_DataOut_xxh_AU16[1]\nObjectType=0x7\nDataType=0x0006\nAccessType=rwr\n\n[3612sub2]\nParameterName=MOD_DataOut_xxh_AU16[2]\nObjectType=0x7\nDataType=0x0006\nAccessType=rwr\n\n[3612sub3]\nParameterName=MOD_DataOut_xxh_AU16[3]\nObjectType=0x7\nDataType=0x0006\nAccessType=rwr\n\n[3612sub4]\nParameterName=MOD_DataOut_xxh_AU16[4]\nObjectType=0x7\nDataType=0x0006\nAccessType=rwr\n\n[3612sub5]\nParameterName=MOD_DataOut_xxh_AU16[5]\nObjectType=0x7\nDataType=0x0006\nAccessType=rwr\n\n[3612sub6]\nParameterName=MOD_DataOut_xxh_AU16[6]\nObjectType=0x7\nDataType=0x0006\nAccessType=rwr\n\n[3612sub7]\nParameterName=MOD_DataOut_xxh_AU16[7]\nObjectType=0x7\nDataType=0x0006\nAccessType=rwr\n\n[3612sub8]\nParameterName=MOD_DataOut_xxh_AU16[8]\nObjectType=0x7\nDataType=0x0006\nAccessType=rwr\n\n[3612sub9]\nParameterName=MOD_DataOut_xxh_AU16[9]\nObjectType=0x7\nDataType=0x0006\nAccessType=rwr\n\n[3612subA]\nParameterName=MOD_DataOut_xxh_AU16[10]\nObjectType=0x7\nDataType=0x0006\nAccessType=rwr\n\n[3613]\nParameterName=MOD_DataOut_xxh_AU16\nObjectType=0x8\nSubNumber=11\n\n[3613sub0]\nParameterName=Number of Entries\nObjectType=0x7\nDataType=0x0005\nAccessType=ro\nDefaultValue=0xA\nLowLimit=0x0\nHighLimit=0xFF\n\n[3613sub1]\nParameterName=MOD_DataOut_xxh_AU16[1]\nObjectType=0x7\nDataType=0x0006\nAccessType=rwr\n\n[3613sub2]\nParameterName=MOD_DataOut_xxh_AU16[2]\nObjectType=0x7\nDataType=0x0006\nAccessType=rwr\n\n[3613sub3]\nParameterName=MOD_DataOut_xxh_AU16[3]\nObjectType=0x7\nDataType=0x0006\nAccessType=rwr\n\n[3613sub4]\nParameterName=MOD_DataOut_xxh_AU16[4]\nObjectType=0x7\nDataType=0x0006\nAccessType=rwr\n\n[3613sub5]\nParameterName=MOD_DataOut_xxh_AU16[5]\nObjectType=0x7\nDataType=0x0006\nAccessType=rwr\n\n[3613sub6]\nParameterName=MOD_DataOut_xxh_AU16[6]\nObjectType=0x7\nDataType=0x0006\nAccessType=rwr\n\n[3613sub7]\nParameterName=MOD_DataOut_xxh_AU16[7]\nObjectType=0x7\nDataType=0x0006\nAccessType=rwr\n\n[3613sub8]\nParameterName=MOD_DataOut_xxh_AU16[8]\nObjectType=0x7\nDataType=0x0006\nAccessType=rwr\n\n[3613sub9]\nParameterName=MOD_DataOut_xxh_AU16[9]\nObjectType=0x7\nDataType=0x0006\nAccessType=rwr\n\n[3613subA]\nParameterName=MOD_DataOut_xxh_AU16[10]\nObjectType=0x7\nDataType=0x0006\nAccessType=rwr\n\n[3700]\nParameterName=MOD_DataOut_xxh_AU32\nObjectType=0x8\nSubNumber=11\n\n[3700sub0]\nParameterName=Number of Entries\nObjectType=0x7\nDataType=0x0005\nAccessType=ro\nDefaultValue=0xA\nLowLimit=0x0\nHighLimit=0xFF\n\n[3700sub1]\nParameterName=MOD_DataOut_xxh_AU32[1]\nObjectType=0x7\nDataType=0x0007\nAccessType=rwr\n\n[3700sub2]\nParameterName=MOD_DataOut_xxh_AU32[2]\nObjectType=0x7\nDataType=0x0007\nAccessType=rwr\n\n[3700sub3]\nParameterName=MOD_DataOut_xxh_AU32[3]\nObjectType=0x7\nDataType=0x0007\nAccessType=rwr\n\n[3700sub4]\nParameterName=MOD_DataOut_xxh_AU32[4]\nObjectType=0x7\nDataType=0x0007\nAccessType=rwr\n\n[3700sub5]\nParameterName=MOD_DataOut_xxh_AU32[5]\nObjectType=0x7\nDataType=0x0007\nAccessType=rwr\n\n[3700sub6]\nParameterName=MOD_DataOut_xxh_AU32[6]\nObjectType=0x7\nDataType=0x0007\nAccessType=rwr\n\n[3700sub7]\nParameterName=MOD_DataOut_xxh_AU32[7]\nObjectType=0x7\nDataType=0x0007\nAccessType=rwr\n\n[3700sub8]\nParameterName=MOD_DataOut_xxh_AU32[8]\nObjectType=0x7\nDataType=0x0007\nAccessType=rwr\n\n[3700sub9]\nParameterName=MOD_DataOut_xxh_AU32[9]\nObjectType=0x7\nDataType=0x0007\nAccessType=rwr\n\n[3700subA]\nParameterName=MOD_DataOut_xxh_AU32[10]\nObjectType=0x7\nDataType=0x0007\nAccessType=rwr\n\n[3701]\nParameterName=MOD_DataOut_xxh_AU32\nObjectType=0x8\nSubNumber=11\n\n[3701sub0]\nParameterName=Number of Entries\nObjectType=0x7\nDataType=0x0005\nAccessType=ro\nDefaultValue=0xA\nLowLimit=0x0\nHighLimit=0xFF\n\n[3701sub1]\nParameterName=MOD_DataOut_xxh_AU32[1]\nObjectType=0x7\nDataType=0x0007\nAccessType=rwr\n\n[3701sub2]\nParameterName=MOD_DataOut_xxh_AU32[2]\nObjectType=0x7\nDataType=0x0007\nAccessType=rwr\n\n[3701sub3]\nParameterName=MOD_DataOut_xxh_AU32[3]\nObjectType=0x7\nDataType=0x0007\nAccessType=rwr\n\n[3701sub4]\nParameterName=MOD_DataOut_xxh_AU32[4]\nObjectType=0x7\nDataType=0x0007\nAccessType=rwr\n\n[3701sub5]\nParameterName=MOD_DataOut_xxh_AU32[5]\nObjectType=0x7\nDataType=0x0007\nAccessType=rwr\n\n[3701sub6]\nParameterName=MOD_DataOut_xxh_AU32[6]\nObjectType=0x7\nDataType=0x0007\nAccessType=rwr\n\n[3701sub7]\nParameterName=MOD_DataOut_xxh_AU32[7]\nObjectType=0x7\nDataType=0x0007\nAccessType=rwr\n\n[3701sub8]\nParameterName=MOD_DataOut_xxh_AU32[8]\nObjectType=0x7\nDataType=0x0007\nAccessType=rwr\n\n[3701sub9]\nParameterName=MOD_DataOut_xxh_AU32[9]\nObjectType=0x7\nDataType=0x0007\nAccessType=rwr\n\n[3701subA]\nParameterName=MOD_DataOut_xxh_AU32[10]\nObjectType=0x7\nDataType=0x0007\nAccessType=rwr\n\n[3702]\nParameterName=MOD_DataOut_xxh_AU32\nObjectType=0x8\nSubNumber=11\n\n[3702sub0]\nParameterName=Number of Entries\nObjectType=0x7\nDataType=0x0005\nAccessType=ro\nDefaultValue=0xA\nLowLimit=0x0\nHighLimit=0xFF\n\n[3702sub1]\nParameterName=MOD_DataOut_xxh_AU32[1]\nObjectType=0x7\nDataType=0x0007\nAccessType=rwr\n\n[3702sub2]\nParameterName=MOD_DataOut_xxh_AU32[2]\nObjectType=0x7\nDataType=0x0007\nAccessType=rwr\n\n[3702sub3]\nParameterName=MOD_DataOut_xxh_AU32[3]\nObjectType=0x7\nDataType=0x0007\nAccessType=rwr\n\n[3702sub4]\nParameterName=MOD_DataOut_xxh_AU32[4]\nObjectType=0x7\nDataType=0x0007\nAccessType=rwr\n\n[3702sub5]\nParameterName=MOD_DataOut_xxh_AU32[5]\nObjectType=0x7\nDataType=0x0007\nAccessType=rwr\n\n[3702sub6]\nParameterName=MOD_DataOut_xxh_AU32[6]\nObjectType=0x7\nDataType=0x0007\nAccessType=rwr\n\n[3702sub7]\nParameterName=MOD_DataOut_xxh_AU32[7]\nObjectType=0x7\nDataType=0x0007\nAccessType=rwr\n\n[3702sub8]\nParameterName=MOD_DataOut_xxh_AU32[8]\nObjectType=0x7\nDataType=0x0007\nAccessType=rwr\n\n[3702sub9]\nParameterName=MOD_DataOut_xxh_AU32[9]\nObjectType=0x7\nDataType=0x0007\nAccessType=rwr\n\n[3702subA]\nParameterName=MOD_DataOut_xxh_AU32[10]\nObjectType=0x7\nDataType=0x0007\nAccessType=rwr\n\n[3703]\nParameterName=MOD_DataOut_xxh_AU32\nObjectType=0x8\nSubNumber=11\n\n[3703sub0]\nParameterName=Number of Entries\nObjectType=0x7\nDataType=0x0005\nAccessType=ro\nDefaultValue=0xA\nLowLimit=0x0\nHighLimit=0xFF\n\n[3703sub1]\nParameterName=MOD_DataOut_xxh_AU32[1]\nObjectType=0x7\nDataType=0x0007\nAccessType=rwr\n\n[3703sub2]\nParameterName=MOD_DataOut_xxh_AU32[2]\nObjectType=0x7\nDataType=0x0007\nAccessType=rwr\n\n[3703sub3]\nParameterName=MOD_DataOut_xxh_AU32[3]\nObjectType=0x7\nDataType=0x0007\nAccessType=rwr\n\n[3703sub4]\nParameterName=MOD_DataOut_xxh_AU32[4]\nObjectType=0x7\nDataType=0x0007\nAccessType=rwr\n\n[3703sub5]\nParameterName=MOD_DataOut_xxh_AU32[5]\nObjectType=0x7\nDataType=0x0007\nAccessType=rwr\n\n[3703sub6]\nParameterName=MOD_DataOut_xxh_AU32[6]\nObjectType=0x7\nDataType=0x0007\nAccessType=rwr\n\n[3703sub7]\nParameterName=MOD_DataOut_xxh_AU32[7]\nObjectType=0x7\nDataType=0x0007\nAccessType=rwr\n\n[3703sub8]\nParameterName=MOD_DataOut_xxh_AU32[8]\nObjectType=0x7\nDataType=0x0007\nAccessType=rwr\n\n[3703sub9]\nParameterName=MOD_DataOut_xxh_AU32[9]\nObjectType=0x7\nDataType=0x0007\nAccessType=rwr\n\n[3703subA]\nParameterName=MOD_DataOut_xxh_AU32[10]\nObjectType=0x7\nDataType=0x0007\nAccessType=rwr\n\n[3704]\nParameterName=MOD_DataOut_xxh_AU32\nObjectType=0x8\nSubNumber=11\n\n[3704sub0]\nParameterName=Number of Entries\nObjectType=0x7\nDataType=0x0005\nAccessType=ro\nDefaultValue=0xA\nLowLimit=0x0\nHighLimit=0xFF\n\n[3704sub1]\nParameterName=MOD_DataOut_xxh_AU32[1]\nObjectType=0x7\nDataType=0x0007\nAccessType=rwr\n\n[3704sub2]\nParameterName=MOD_DataOut_xxh_AU32[2]\nObjectType=0x7\nDataType=0x0007\nAccessType=rwr\n\n[3704sub3]\nParameterName=MOD_DataOut_xxh_AU32[3]\nObjectType=0x7\nDataType=0x0007\nAccessType=rwr\n\n[3704sub4]\nParameterName=MOD_DataOut_xxh_AU32[4]\nObjectType=0x7\nDataType=0x0007\nAccessType=rwr\n\n[3704sub5]\nParameterName=MOD_DataOut_xxh_AU32[5]\nObjectType=0x7\nDataType=0x0007\nAccessType=rwr\n\n[3704sub6]\nParameterName=MOD_DataOut_xxh_AU32[6]\nObjectType=0x7\nDataType=0x0007\nAccessType=rwr\n\n[3704sub7]\nParameterName=MOD_DataOut_xxh_AU32[7]\nObjectType=0x7\nDataType=0x0007\nAccessType=rwr\n\n[3704sub8]\nParameterName=MOD_DataOut_xxh_AU32[8]\nObjectType=0x7\nDataType=0x0007\nAccessType=rwr\n\n[3704sub9]\nParameterName=MOD_DataOut_xxh_AU32[9]\nObjectType=0x7\nDataType=0x0007\nAccessType=rwr\n\n[3704subA]\nParameterName=MOD_DataOut_xxh_AU32[10]\nObjectType=0x7\nDataType=0x0007\nAccessType=rwr\n\n[3705]\nParameterName=MOD_DataOut_xxh_AU32\nObjectType=0x8\nSubNumber=11\n\n[3705sub0]\nParameterName=Number of Entries\nObjectType=0x7\nDataType=0x0005\nAccessType=ro\nDefaultValue=0xA\nLowLimit=0x0\nHighLimit=0xFF\n\n[3705sub1]\nParameterName=MOD_DataOut_xxh_AU32[1]\nObjectType=0x7\nDataType=0x0007\nAccessType=rwr\n\n[3705sub2]\nParameterName=MOD_DataOut_xxh_AU32[2]\nObjectType=0x7\nDataType=0x0007\nAccessType=rwr\n\n[3705sub3]\nParameterName=MOD_DataOut_xxh_AU32[3]\nObjectType=0x7\nDataType=0x0007\nAccessType=rwr\n\n[3705sub4]\nParameterName=MOD_DataOut_xxh_AU32[4]\nObjectType=0x7\nDataType=0x0007\nAccessType=rwr\n\n[3705sub5]\nParameterName=MOD_DataOut_xxh_AU32[5]\nObjectType=0x7\nDataType=0x0007\nAccessType=rwr\n\n[3705sub6]\nParameterName=MOD_DataOut_xxh_AU32[6]\nObjectType=0x7\nDataType=0x0007\nAccessType=rwr\n\n[3705sub7]\nParameterName=MOD_DataOut_xxh_AU32[7]\nObjectType=0x7\nDataType=0x0007\nAccessType=rwr\n\n[3705sub8]\nParameterName=MOD_DataOut_xxh_AU32[8]\nObjectType=0x7\nDataType=0x0007\nAccessType=rwr\n\n[3705sub9]\nParameterName=MOD_DataOut_xxh_AU32[9]\nObjectType=0x7\nDataType=0x0007\nAccessType=rwr\n\n[3705subA]\nParameterName=MOD_DataOut_xxh_AU32[10]\nObjectType=0x7\nDataType=0x0007\nAccessType=rwr\n\n[3706]\nParameterName=MOD_DataOut_xxh_AU32\nObjectType=0x8\nSubNumber=11\n\n[3706sub0]\nParameterName=Number of Entries\nObjectType=0x7\nDataType=0x0005\nAccessType=ro\nDefaultValue=0xA\nLowLimit=0x0\nHighLimit=0xFF\n\n[3706sub1]\nParameterName=MOD_DataOut_xxh_AU32[1]\nObjectType=0x7\nDataType=0x0007\nAccessType=rwr\n\n[3706sub2]\nParameterName=MOD_DataOut_xxh_AU32[2]\nObjectType=0x7\nDataType=0x0007\nAccessType=rwr\n\n[3706sub3]\nParameterName=MOD_DataOut_xxh_AU32[3]\nObjectType=0x7\nDataType=0x0007\nAccessType=rwr\n\n[3706sub4]\nParameterName=MOD_DataOut_xxh_AU32[4]\nObjectType=0x7\nDataType=0x0007\nAccessType=rwr\n\n[3706sub5]\nParameterName=MOD_DataOut_xxh_AU32[5]\nObjectType=0x7\nDataType=0x0007\nAccessType=rwr\n\n[3706sub6]\nParameterName=MOD_DataOut_xxh_AU32[6]\nObjectType=0x7\nDataType=0x0007\nAccessType=rwr\n\n[3706sub7]\nParameterName=MOD_DataOut_xxh_AU32[7]\nObjectType=0x7\nDataType=0x0007\nAccessType=rwr\n\n[3706sub8]\nParameterName=MOD_DataOut_xxh_AU32[8]\nObjectType=0x7\nDataType=0x0007\nAccessType=rwr\n\n[3706sub9]\nParameterName=MOD_DataOut_xxh_AU32[9]\nObjectType=0x7\nDataType=0x0007\nAccessType=rwr\n\n[3706subA]\nParameterName=MOD_DataOut_xxh_AU32[10]\nObjectType=0x7\nDataType=0x0007\nAccessType=rwr\n\n[3707]\nParameterName=MOD_DataOut_xxh_AU32\nObjectType=0x8\nSubNumber=11\n\n[3707sub0]\nParameterName=Number of Entries\nObjectType=0x7\nDataType=0x0005\nAccessType=ro\nDefaultValue=0xA\nLowLimit=0x0\nHighLimit=0xFF\n\n[3707sub1]\nParameterName=MOD_DataOut_xxh_AU32[1]\nObjectType=0x7\nDataType=0x0007\nAccessType=rwr\n\n[3707sub2]\nParameterName=MOD_DataOut_xxh_AU32[2]\nObjectType=0x7\nDataType=0x0007\nAccessType=rwr\n\n[3707sub3]\nParameterName=MOD_DataOut_xxh_AU32[3]\nObjectType=0x7\nDataType=0x0007\nAccessType=rwr\n\n[3707sub4]\nParameterName=MOD_DataOut_xxh_AU32[4]\nObjectType=0x7\nDataType=0x0007\nAccessType=rwr\n\n[3707sub5]\nParameterName=MOD_DataOut_xxh_AU32[5]\nObjectType=0x7\nDataType=0x0007\nAccessType=rwr\n\n[3707sub6]\nParameterName=MOD_DataOut_xxh_AU32[6]\nObjectType=0x7\nDataType=0x0007\nAccessType=rwr\n\n[3707sub7]\nParameterName=MOD_DataOut_xxh_AU32[7]\nObjectType=0x7\nDataType=0x0007\nAccessType=rwr\n\n[3707sub8]\nParameterName=MOD_DataOut_xxh_AU32[8]\nObjectType=0x7\nDataType=0x0007\nAccessType=rwr\n\n[3707sub9]\nParameterName=MOD_DataOut_xxh_AU32[9]\nObjectType=0x7\nDataType=0x0007\nAccessType=rwr\n\n[3707subA]\nParameterName=MOD_DataOut_xxh_AU32[10]\nObjectType=0x7\nDataType=0x0007\nAccessType=rwr\n\n[3708]\nParameterName=MOD_DataOut_xxh_AU32\nObjectType=0x8\nSubNumber=11\n\n[3708sub0]\nParameterName=Number of Entries\nObjectType=0x7\nDataType=0x0005\nAccessType=ro\nDefaultValue=0xA\nLowLimit=0x0\nHighLimit=0xFF\n\n[3708sub1]\nParameterName=MOD_DataOut_xxh_AU32[1]\nObjectType=0x7\nDataType=0x0007\nAccessType=rwr\n\n[3708sub2]\nParameterName=MOD_DataOut_xxh_AU32[2]\nObjectType=0x7\nDataType=0x0007\nAccessType=rwr\n\n[3708sub3]\nParameterName=MOD_DataOut_xxh_AU32[3]\nObjectType=0x7\nDataType=0x0007\nAccessType=rwr\n\n[3708sub4]\nParameterName=MOD_DataOut_xxh_AU32[4]\nObjectType=0x7\nDataType=0x0007\nAccessType=rwr\n\n[3708sub5]\nParameterName=MOD_DataOut_xxh_AU32[5]\nObjectType=0x7\nDataType=0x0007\nAccessType=rwr\n\n[3708sub6]\nParameterName=MOD_DataOut_xxh_AU32[6]\nObjectType=0x7\nDataType=0x0007\nAccessType=rwr\n\n[3708sub7]\nParameterName=MOD_DataOut_xxh_AU32[7]\nObjectType=0x7\nDataType=0x0007\nAccessType=rwr\n\n[3708sub8]\nParameterName=MOD_DataOut_xxh_AU32[8]\nObjectType=0x7\nDataType=0x0007\nAccessType=rwr\n\n[3708sub9]\nParameterName=MOD_DataOut_xxh_AU32[9]\nObjectType=0x7\nDataType=0x0007\nAccessType=rwr\n\n[3708subA]\nParameterName=MOD_DataOut_xxh_AU32[10]\nObjectType=0x7\nDataType=0x0007\nAccessType=rwr\n\n[3709]\nParameterName=MOD_DataOut_xxh_AU32\nObjectType=0x8\nSubNumber=11\n\n[3709sub0]\nParameterName=Number of Entries\nObjectType=0x7\nDataType=0x0005\nAccessType=ro\nDefaultValue=0xA\nLowLimit=0x0\nHighLimit=0xFF\n\n[3709sub1]\nParameterName=MOD_DataOut_xxh_AU32[1]\nObjectType=0x7\nDataType=0x0007\nAccessType=rwr\n\n[3709sub2]\nParameterName=MOD_DataOut_xxh_AU32[2]\nObjectType=0x7\nDataType=0x0007\nAccessType=rwr\n\n[3709sub3]\nParameterName=MOD_DataOut_xxh_AU32[3]\nObjectType=0x7\nDataType=0x0007\nAccessType=rwr\n\n[3709sub4]\nParameterName=MOD_DataOut_xxh_AU32[4]\nObjectType=0x7\nDataType=0x0007\nAccessType=rwr\n\n[3709sub5]\nParameterName=MOD_DataOut_xxh_AU32[5]\nObjectType=0x7\nDataType=0x0007\nAccessType=rwr\n\n[3709sub6]\nParameterName=MOD_DataOut_xxh_AU32[6]\nObjectType=0x7\nDataType=0x0007\nAccessType=rwr\n\n[3709sub7]\nParameterName=MOD_DataOut_xxh_AU32[7]\nObjectType=0x7\nDataType=0x0007\nAccessType=rwr\n\n[3709sub8]\nParameterName=MOD_DataOut_xxh_AU32[8]\nObjectType=0x7\nDataType=0x0007\nAccessType=rwr\n\n[3709sub9]\nParameterName=MOD_DataOut_xxh_AU32[9]\nObjectType=0x7\nDataType=0x0007\nAccessType=rwr\n\n[3709subA]\nParameterName=MOD_DataOut_xxh_AU32[10]\nObjectType=0x7\nDataType=0x0007\nAccessType=rwr\n\n[370A]\nParameterName=MOD_DataOut_xxh_AU32\nObjectType=0x8\nSubNumber=11\n\n[370Asub0]\nParameterName=Number of Entries\nObjectType=0x7\nDataType=0x0005\nAccessType=ro\nDefaultValue=0xA\nLowLimit=0x0\nHighLimit=0xFF\n\n[370Asub1]\nParameterName=MOD_DataOut_xxh_AU32[1]\nObjectType=0x7\nDataType=0x0007\nAccessType=rwr\n\n[370Asub2]\nParameterName=MOD_DataOut_xxh_AU32[2]\nObjectType=0x7\nDataType=0x0007\nAccessType=rwr\n\n[370Asub3]\nParameterName=MOD_DataOut_xxh_AU32[3]\nObjectType=0x7\nDataType=0x0007\nAccessType=rwr\n\n[370Asub4]\nParameterName=MOD_DataOut_xxh_AU32[4]\nObjectType=0x7\nDataType=0x0007\nAccessType=rwr\n\n[370Asub5]\nParameterName=MOD_DataOut_xxh_AU32[5]\nObjectType=0x7\nDataType=0x0007\nAccessType=rwr\n\n[370Asub6]\nParameterName=MOD_DataOut_xxh_AU32[6]\nObjectType=0x7\nDataType=0x0007\nAccessType=rwr\n\n[370Asub7]\nParameterName=MOD_DataOut_xxh_AU32[7]\nObjectType=0x7\nDataType=0x0007\nAccessType=rwr\n\n[370Asub8]\nParameterName=MOD_DataOut_xxh_AU32[8]\nObjectType=0x7\nDataType=0x0007\nAccessType=rwr\n\n[370Asub9]\nParameterName=MOD_DataOut_xxh_AU32[9]\nObjectType=0x7\nDataType=0x0007\nAccessType=rwr\n\n[370AsubA]\nParameterName=MOD_DataOut_xxh_AU32[10]\nObjectType=0x7\nDataType=0x0007\nAccessType=rwr\n\n[370B]\nParameterName=MOD_DataOut_xxh_AU32\nObjectType=0x8\nSubNumber=11\n\n[370Bsub0]\nParameterName=Number of Entries\nObjectType=0x7\nDataType=0x0005\nAccessType=ro\nDefaultValue=0xA\nLowLimit=0x0\nHighLimit=0xFF\n\n[370Bsub1]\nParameterName=MOD_DataOut_xxh_AU32[1]\nObjectType=0x7\nDataType=0x0007\nAccessType=rwr\n\n[370Bsub2]\nParameterName=MOD_DataOut_xxh_AU32[2]\nObjectType=0x7\nDataType=0x0007\nAccessType=rwr\n\n[370Bsub3]\nParameterName=MOD_DataOut_xxh_AU32[3]\nObjectType=0x7\nDataType=0x0007\nAccessType=rwr\n\n[370Bsub4]\nParameterName=MOD_DataOut_xxh_AU32[4]\nObjectType=0x7\nDataType=0x0007\nAccessType=rwr\n\n[370Bsub5]\nParameterName=MOD_DataOut_xxh_AU32[5]\nObjectType=0x7\nDataType=0x0007\nAccessType=rwr\n\n[370Bsub6]\nParameterName=MOD_DataOut_xxh_AU32[6]\nObjectType=0x7\nDataType=0x0007\nAccessType=rwr\n\n[370Bsub7]\nParameterName=MOD_DataOut_xxh_AU32[7]\nObjectType=0x7\nDataType=0x0007\nAccessType=rwr\n\n[370Bsub8]\nParameterName=MOD_DataOut_xxh_AU32[8]\nObjectType=0x7\nDataType=0x0007\nAccessType=rwr\n\n[370Bsub9]\nParameterName=MOD_DataOut_xxh_AU32[9]\nObjectType=0x7\nDataType=0x0007\nAccessType=rwr\n\n[370BsubA]\nParameterName=MOD_DataOut_xxh_AU32[10]\nObjectType=0x7\nDataType=0x0007\nAccessType=rwr\n\n[370C]\nParameterName=MOD_DataOut_xxh_AU32\nObjectType=0x8\nSubNumber=11\n\n[370Csub0]\nParameterName=Number of Entries\nObjectType=0x7\nDataType=0x0005\nAccessType=ro\nDefaultValue=0xA\nLowLimit=0x0\nHighLimit=0xFF\n\n[370Csub1]\nParameterName=MOD_DataOut_xxh_AU32[1]\nObjectType=0x7\nDataType=0x0007\nAccessType=rwr\n\n[370Csub2]\nParameterName=MOD_DataOut_xxh_AU32[2]\nObjectType=0x7\nDataType=0x0007\nAccessType=rwr\n\n[370Csub3]\nParameterName=MOD_DataOut_xxh_AU32[3]\nObjectType=0x7\nDataType=0x0007\nAccessType=rwr\n\n[370Csub4]\nParameterName=MOD_DataOut_xxh_AU32[4]\nObjectType=0x7\nDataType=0x0007\nAccessType=rwr\n\n[370Csub5]\nParameterName=MOD_DataOut_xxh_AU32[5]\nObjectType=0x7\nDataType=0x0007\nAccessType=rwr\n\n[370Csub6]\nParameterName=MOD_DataOut_xxh_AU32[6]\nObjectType=0x7\nDataType=0x0007\nAccessType=rwr\n\n[370Csub7]\nParameterName=MOD_DataOut_xxh_AU32[7]\nObjectType=0x7\nDataType=0x0007\nAccessType=rwr\n\n[370Csub8]\nParameterName=MOD_DataOut_xxh_AU32[8]\nObjectType=0x7\nDataType=0x0007\nAccessType=rwr\n\n[370Csub9]\nParameterName=MOD_DataOut_xxh_AU32[9]\nObjectType=0x7\nDataType=0x0007\nAccessType=rwr\n\n[370CsubA]\nParameterName=MOD_DataOut_xxh_AU32[10]\nObjectType=0x7\nDataType=0x0007\nAccessType=rwr\n\n[370D]\nParameterName=MOD_DataOut_xxh_AU32\nObjectType=0x8\nSubNumber=11\n\n[370Dsub0]\nParameterName=Number of Entries\nObjectType=0x7\nDataType=0x0005\nAccessType=ro\nDefaultValue=0xA\nLowLimit=0x0\nHighLimit=0xFF\n\n[370Dsub1]\nParameterName=MOD_DataOut_xxh_AU32[1]\nObjectType=0x7\nDataType=0x0007\nAccessType=rwr\n\n[370Dsub2]\nParameterName=MOD_DataOut_xxh_AU32[2]\nObjectType=0x7\nDataType=0x0007\nAccessType=rwr\n\n[370Dsub3]\nParameterName=MOD_DataOut_xxh_AU32[3]\nObjectType=0x7\nDataType=0x0007\nAccessType=rwr\n\n[370Dsub4]\nParameterName=MOD_DataOut_xxh_AU32[4]\nObjectType=0x7\nDataType=0x0007\nAccessType=rwr\n\n[370Dsub5]\nParameterName=MOD_DataOut_xxh_AU32[5]\nObjectType=0x7\nDataType=0x0007\nAccessType=rwr\n\n[370Dsub6]\nParameterName=MOD_DataOut_xxh_AU32[6]\nObjectType=0x7\nDataType=0x0007\nAccessType=rwr\n\n[370Dsub7]\nParameterName=MOD_DataOut_xxh_AU32[7]\nObjectType=0x7\nDataType=0x0007\nAccessType=rwr\n\n[370Dsub8]\nParameterName=MOD_DataOut_xxh_AU32[8]\nObjectType=0x7\nDataType=0x0007\nAccessType=rwr\n\n[370Dsub9]\nParameterName=MOD_DataOut_xxh_AU32[9]\nObjectType=0x7\nDataType=0x0007\nAccessType=rwr\n\n[370DsubA]\nParameterName=MOD_DataOut_xxh_AU32[10]\nObjectType=0x7\nDataType=0x0007\nAccessType=rwr\n\n[370E]\nParameterName=MOD_DataOut_xxh_AU32\nObjectType=0x8\nSubNumber=11\n\n[370Esub0]\nParameterName=Number of Entries\nObjectType=0x7\nDataType=0x0005\nAccessType=ro\nDefaultValue=0xA\nLowLimit=0x0\nHighLimit=0xFF\n\n[370Esub1]\nParameterName=MOD_DataOut_xxh_AU32[1]\nObjectType=0x7\nDataType=0x0007\nAccessType=rwr\n\n[370Esub2]\nParameterName=MOD_DataOut_xxh_AU32[2]\nObjectType=0x7\nDataType=0x0007\nAccessType=rwr\n\n[370Esub3]\nParameterName=MOD_DataOut_xxh_AU32[3]\nObjectType=0x7\nDataType=0x0007\nAccessType=rwr\n\n[370Esub4]\nParameterName=MOD_DataOut_xxh_AU32[4]\nObjectType=0x7\nDataType=0x0007\nAccessType=rwr\n\n[370Esub5]\nParameterName=MOD_DataOut_xxh_AU32[5]\nObjectType=0x7\nDataType=0x0007\nAccessType=rwr\n\n[370Esub6]\nParameterName=MOD_DataOut_xxh_AU32[6]\nObjectType=0x7\nDataType=0x0007\nAccessType=rwr\n\n[370Esub7]\nParameterName=MOD_DataOut_xxh_AU32[7]\nObjectType=0x7\nDataType=0x0007\nAccessType=rwr\n\n[370Esub8]\nParameterName=MOD_DataOut_xxh_AU32[8]\nObjectType=0x7\nDataType=0x0007\nAccessType=rwr\n\n[370Esub9]\nParameterName=MOD_DataOut_xxh_AU32[9]\nObjectType=0x7\nDataType=0x0007\nAccessType=rwr\n\n[370EsubA]\nParameterName=MOD_DataOut_xxh_AU32[10]\nObjectType=0x7\nDataType=0x0007\nAccessType=rwr\n\n[370F]\nParameterName=MOD_DataOut_xxh_AU32\nObjectType=0x8\nSubNumber=11\n\n[370Fsub0]\nParameterName=Number of Entries\nObjectType=0x7\nDataType=0x0005\nAccessType=ro\nDefaultValue=0xA\nLowLimit=0x0\nHighLimit=0xFF\n\n[370Fsub1]\nParameterName=MOD_DataOut_xxh_AU32[1]\nObjectType=0x7\nDataType=0x0007\nAccessType=rwr\n\n[370Fsub2]\nParameterName=MOD_DataOut_xxh_AU32[2]\nObjectType=0x7\nDataType=0x0007\nAccessType=rwr\n\n[370Fsub3]\nParameterName=MOD_DataOut_xxh_AU32[3]\nObjectType=0x7\nDataType=0x0007\nAccessType=rwr\n\n[370Fsub4]\nParameterName=MOD_DataOut_xxh_AU32[4]\nObjectType=0x7\nDataType=0x0007\nAccessType=rwr\n\n[370Fsub5]\nParameterName=MOD_DataOut_xxh_AU32[5]\nObjectType=0x7\nDataType=0x0007\nAccessType=rwr\n\n[370Fsub6]\nParameterName=MOD_DataOut_xxh_AU32[6]\nObjectType=0x7\nDataType=0x0007\nAccessType=rwr\n\n[370Fsub7]\nParameterName=MOD_DataOut_xxh_AU32[7]\nObjectType=0x7\nDataType=0x0007\nAccessType=rwr\n\n[370Fsub8]\nParameterName=MOD_DataOut_xxh_AU32[8]\nObjectType=0x7\nDataType=0x0007\nAccessType=rwr\n\n[370Fsub9]\nParameterName=MOD_DataOut_xxh_AU32[9]\nObjectType=0x7\nDataType=0x0007\nAccessType=rwr\n\n[370FsubA]\nParameterName=MOD_DataOut_xxh_AU32[10]\nObjectType=0x7\nDataType=0x0007\nAccessType=rwr\n\n[3710]\nParameterName=MOD_DataOut_xxh_AU32\nObjectType=0x8\nSubNumber=11\n\n[3710sub0]\nParameterName=Number of Entries\nObjectType=0x7\nDataType=0x0005\nAccessType=ro\nDefaultValue=0xA\nLowLimit=0x0\nHighLimit=0xFF\n\n[3710sub1]\nParameterName=MOD_DataOut_xxh_AU32[1]\nObjectType=0x7\nDataType=0x0007\nAccessType=rwr\n\n[3710sub2]\nParameterName=MOD_DataOut_xxh_AU32[2]\nObjectType=0x7\nDataType=0x0007\nAccessType=rwr\n\n[3710sub3]\nParameterName=MOD_DataOut_xxh_AU32[3]\nObjectType=0x7\nDataType=0x0007\nAccessType=rwr\n\n[3710sub4]\nParameterName=MOD_DataOut_xxh_AU32[4]\nObjectType=0x7\nDataType=0x0007\nAccessType=rwr\n\n[3710sub5]\nParameterName=MOD_DataOut_xxh_AU32[5]\nObjectType=0x7\nDataType=0x0007\nAccessType=rwr\n\n[3710sub6]\nParameterName=MOD_DataOut_xxh_AU32[6]\nObjectType=0x7\nDataType=0x0007\nAccessType=rwr\n\n[3710sub7]\nParameterName=MOD_DataOut_xxh_AU32[7]\nObjectType=0x7\nDataType=0x0007\nAccessType=rwr\n\n[3710sub8]\nParameterName=MOD_DataOut_xxh_AU32[8]\nObjectType=0x7\nDataType=0x0007\nAccessType=rwr\n\n[3710sub9]\nParameterName=MOD_DataOut_xxh_AU32[9]\nObjectType=0x7\nDataType=0x0007\nAccessType=rwr\n\n[3710subA]\nParameterName=MOD_DataOut_xxh_AU32[10]\nObjectType=0x7\nDataType=0x0007\nAccessType=rwr\n\n[3711]\nParameterName=MOD_DataOut_xxh_AU32\nObjectType=0x8\nSubNumber=11\n\n[3711sub0]\nParameterName=Number of Entries\nObjectType=0x7\nDataType=0x0005\nAccessType=ro\nDefaultValue=0xA\nLowLimit=0x0\nHighLimit=0xFF\n\n[3711sub1]\nParameterName=MOD_DataOut_xxh_AU32[1]\nObjectType=0x7\nDataType=0x0007\nAccessType=rwr\n\n[3711sub2]\nParameterName=MOD_DataOut_xxh_AU32[2]\nObjectType=0x7\nDataType=0x0007\nAccessType=rwr\n\n[3711sub3]\nParameterName=MOD_DataOut_xxh_AU32[3]\nObjectType=0x7\nDataType=0x0007\nAccessType=rwr\n\n[3711sub4]\nParameterName=MOD_DataOut_xxh_AU32[4]\nObjectType=0x7\nDataType=0x0007\nAccessType=rwr\n\n[3711sub5]\nParameterName=MOD_DataOut_xxh_AU32[5]\nObjectType=0x7\nDataType=0x0007\nAccessType=rwr\n\n[3711sub6]\nParameterName=MOD_DataOut_xxh_AU32[6]\nObjectType=0x7\nDataType=0x0007\nAccessType=rwr\n\n[3711sub7]\nParameterName=MOD_DataOut_xxh_AU32[7]\nObjectType=0x7\nDataType=0x0007\nAccessType=rwr\n\n[3711sub8]\nParameterName=MOD_DataOut_xxh_AU32[8]\nObjectType=0x7\nDataType=0x0007\nAccessType=rwr\n\n[3711sub9]\nParameterName=MOD_DataOut_xxh_AU32[9]\nObjectType=0x7\nDataType=0x0007\nAccessType=rwr\n\n[3711subA]\nParameterName=MOD_DataOut_xxh_AU32[10]\nObjectType=0x7\nDataType=0x0007\nAccessType=rwr\n\n[3712]\nParameterName=MOD_DataOut_xxh_AU32\nObjectType=0x8\nSubNumber=11\n\n[3712sub0]\nParameterName=Number of Entries\nObjectType=0x7\nDataType=0x0005\nAccessType=ro\nDefaultValue=0xA\nLowLimit=0x0\nHighLimit=0xFF\n\n[3712sub1]\nParameterName=MOD_DataOut_xxh_AU32[1]\nObjectType=0x7\nDataType=0x0007\nAccessType=rwr\n\n[3712sub2]\nParameterName=MOD_DataOut_xxh_AU32[2]\nObjectType=0x7\nDataType=0x0007\nAccessType=rwr\n\n[3712sub3]\nParameterName=MOD_DataOut_xxh_AU32[3]\nObjectType=0x7\nDataType=0x0007\nAccessType=rwr\n\n[3712sub4]\nParameterName=MOD_DataOut_xxh_AU32[4]\nObjectType=0x7\nDataType=0x0007\nAccessType=rwr\n\n[3712sub5]\nParameterName=MOD_DataOut_xxh_AU32[5]\nObjectType=0x7\nDataType=0x0007\nAccessType=rwr\n\n[3712sub6]\nParameterName=MOD_DataOut_xxh_AU32[6]\nObjectType=0x7\nDataType=0x0007\nAccessType=rwr\n\n[3712sub7]\nParameterName=MOD_DataOut_xxh_AU32[7]\nObjectType=0x7\nDataType=0x0007\nAccessType=rwr\n\n[3712sub8]\nParameterName=MOD_DataOut_xxh_AU32[8]\nObjectType=0x7\nDataType=0x0007\nAccessType=rwr\n\n[3712sub9]\nParameterName=MOD_DataOut_xxh_AU32[9]\nObjectType=0x7\nDataType=0x0007\nAccessType=rwr\n\n[3712subA]\nParameterName=MOD_DataOut_xxh_AU32[10]\nObjectType=0x7\nDataType=0x0007\nAccessType=rwr\n\n[3713]\nParameterName=MOD_DataOut_xxh_AU32\nObjectType=0x8\nSubNumber=11\n\n[3713sub0]\nParameterName=Number of Entries\nObjectType=0x7\nDataType=0x0005\nAccessType=ro\nDefaultValue=0xA\nLowLimit=0x0\nHighLimit=0xFF\n\n[3713sub1]\nParameterName=MOD_DataOut_xxh_AU32[1]\nObjectType=0x7\nDataType=0x0007\nAccessType=rwr\n\n[3713sub2]\nParameterName=MOD_DataOut_xxh_AU32[2]\nObjectType=0x7\nDataType=0x0007\nAccessType=rwr\n\n[3713sub3]\nParameterName=MOD_DataOut_xxh_AU32[3]\nObjectType=0x7\nDataType=0x0007\nAccessType=rwr\n\n[3713sub4]\nParameterName=MOD_DataOut_xxh_AU32[4]\nObjectType=0x7\nDataType=0x0007\nAccessType=rwr\n\n[3713sub5]\nParameterName=MOD_DataOut_xxh_AU32[5]\nObjectType=0x7\nDataType=0x0007\nAccessType=rwr\n\n[3713sub6]\nParameterName=MOD_DataOut_xxh_AU32[6]\nObjectType=0x7\nDataType=0x0007\nAccessType=rwr\n\n[3713sub7]\nParameterName=MOD_DataOut_xxh_AU32[7]\nObjectType=0x7\nDataType=0x0007\nAccessType=rwr\n\n[3713sub8]\nParameterName=MOD_DataOut_xxh_AU32[8]\nObjectType=0x7\nDataType=0x0007\nAccessType=rwr\n\n[3713sub9]\nParameterName=MOD_DataOut_xxh_AU32[9]\nObjectType=0x7\nDataType=0x0007\nAccessType=rwr\n\n[3713subA]\nParameterName=MOD_DataOut_xxh_AU32[10]\nObjectType=0x7\nDataType=0x0007\nAccessType=rwr\n\n[3800]\nParameterName=MOD_ConfigEntryReg_xxh_AU32\nObjectType=0x8\nSubNumber=6\n\n[3800sub0]\nParameterName=Number of Entries\nObjectType=0x7\nDataType=0x0005\nAccessType=ro\nDefaultValue=0x5\nLowLimit=0x0\nHighLimit=0xFF\n\n[3800sub1]\nParameterName=MOD_ConfigEntryReg_xxh_AU32[n]\nObjectType=0x7\nDataType=0x0007\nAccessType=rw\n\n[3800sub2]\nParameterName=MOD_ConfigEntryReg_xxh_AU32[n]\nObjectType=0x7\nDataType=0x0007\nAccessType=rw\n\n[3800sub3]\nParameterName=MOD_ConfigEntryReg_xxh_AU32[n]\nObjectType=0x7\nDataType=0x0007\nAccessType=rw\n\n[3800sub4]\nParameterName=MOD_ConfigEntryReg_xxh_AU32[n]\nObjectType=0x7\nDataType=0x0007\nAccessType=rw\n\n[3800sub5]\nParameterName=MOD_ConfigEntryReg_xxh_AU32[n]\nObjectType=0x7\nDataType=0x0007\nAccessType=rw\n\n[3801]\nParameterName=MOD_ConfigEntryReg_xxh_AU32\nObjectType=0x8\nSubNumber=6\n\n[3801sub0]\nParameterName=Number of Entries\nObjectType=0x7\nDataType=0x0005\nAccessType=ro\nDefaultValue=0x5\nLowLimit=0x0\nHighLimit=0xFF\n\n[3801sub1]\nParameterName=MOD_ConfigEntryReg_xxh_AU32[n]\nObjectType=0x7\nDataType=0x0007\nAccessType=rw\n\n[3801sub2]\nParameterName=MOD_ConfigEntryReg_xxh_AU32[n]\nObjectType=0x7\nDataType=0x0007\nAccessType=rw\n\n[3801sub3]\nParameterName=MOD_ConfigEntryReg_xxh_AU32[n]\nObjectType=0x7\nDataType=0x0007\nAccessType=rw\n\n[3801sub4]\nParameterName=MOD_ConfigEntryReg_xxh_AU32[n]\nObjectType=0x7\nDataType=0x0007\nAccessType=rw\n\n[3801sub5]\nParameterName=MOD_ConfigEntryReg_xxh_AU32[n]\nObjectType=0x7\nDataType=0x0007\nAccessType=rw\n\n[3802]\nParameterName=MOD_ConfigEntryReg_xxh_AU32\nObjectType=0x8\nSubNumber=6\n\n[3802sub0]\nParameterName=Number of Entries\nObjectType=0x7\nDataType=0x0005\nAccessType=ro\nDefaultValue=0x5\nLowLimit=0x0\nHighLimit=0xFF\n\n[3802sub1]\nParameterName=MOD_ConfigEntryReg_xxh_AU32[n]\nObjectType=0x7\nDataType=0x0007\nAccessType=rw\n\n[3802sub2]\nParameterName=MOD_ConfigEntryReg_xxh_AU32[n]\nObjectType=0x7\nDataType=0x0007\nAccessType=rw\n\n[3802sub3]\nParameterName=MOD_ConfigEntryReg_xxh_AU32[n]\nObjectType=0x7\nDataType=0x0007\nAccessType=rw\n\n[3802sub4]\nParameterName=MOD_ConfigEntryReg_xxh_AU32[n]\nObjectType=0x7\nDataType=0x0007\nAccessType=rw\n\n[3802sub5]\nParameterName=MOD_ConfigEntryReg_xxh_AU32[n]\nObjectType=0x7\nDataType=0x0007\nAccessType=rw\n\n[3803]\nParameterName=MOD_ConfigEntryReg_xxh_AU32\nObjectType=0x8\nSubNumber=6\n\n[3803sub0]\nParameterName=Number of Entries\nObjectType=0x7\nDataType=0x0005\nAccessType=ro\nDefaultValue=0x5\nLowLimit=0x0\nHighLimit=0xFF\n\n[3803sub1]\nParameterName=MOD_ConfigEntryReg_xxh_AU32[n]\nObjectType=0x7\nDataType=0x0007\nAccessType=rw\n\n[3803sub2]\nParameterName=MOD_ConfigEntryReg_xxh_AU32[n]\nObjectType=0x7\nDataType=0x0007\nAccessType=rw\n\n[3803sub3]\nParameterName=MOD_ConfigEntryReg_xxh_AU32[n]\nObjectType=0x7\nDataType=0x0007\nAccessType=rw\n\n[3803sub4]\nParameterName=MOD_ConfigEntryReg_xxh_AU32[n]\nObjectType=0x7\nDataType=0x0007\nAccessType=rw\n\n[3803sub5]\nParameterName=MOD_ConfigEntryReg_xxh_AU32[n]\nObjectType=0x7\nDataType=0x0007\nAccessType=rw\n\n[3804]\nParameterName=MOD_ConfigEntryReg_xxh_AU32\nObjectType=0x8\nSubNumber=6\n\n[3804sub0]\nParameterName=Number of Entries\nObjectType=0x7\nDataType=0x0005\nAccessType=ro\nDefaultValue=0x5\nLowLimit=0x0\nHighLimit=0xFF\n\n[3804sub1]\nParameterName=MOD_ConfigEntryReg_xxh_AU32[n]\nObjectType=0x7\nDataType=0x0007\nAccessType=rw\n\n[3804sub2]\nParameterName=MOD_ConfigEntryReg_xxh_AU32[n]\nObjectType=0x7\nDataType=0x0007\nAccessType=rw\n\n[3804sub3]\nParameterName=MOD_ConfigEntryReg_xxh_AU32[n]\nObjectType=0x7\nDataType=0x0007\nAccessType=rw\n\n[3804sub4]\nParameterName=MOD_ConfigEntryReg_xxh_AU32[n]\nObjectType=0x7\nDataType=0x0007\nAccessType=rw\n\n[3804sub5]\nParameterName=MOD_ConfigEntryReg_xxh_AU32[n]\nObjectType=0x7\nDataType=0x0007\nAccessType=rw\n\n[3805]\nParameterName=MOD_ConfigEntryReg_xxh_AU32\nObjectType=0x8\nSubNumber=6\n\n[3805sub0]\nParameterName=Number of Entries\nObjectType=0x7\nDataType=0x0005\nAccessType=ro\nDefaultValue=0x5\nLowLimit=0x0\nHighLimit=0xFF\n\n[3805sub1]\nParameterName=MOD_ConfigEntryReg_xxh_AU32[n]\nObjectType=0x7\nDataType=0x0007\nAccessType=rw\n\n[3805sub2]\nParameterName=MOD_ConfigEntryReg_xxh_AU32[n]\nObjectType=0x7\nDataType=0x0007\nAccessType=rw\n\n[3805sub3]\nParameterName=MOD_ConfigEntryReg_xxh_AU32[n]\nObjectType=0x7\nDataType=0x0007\nAccessType=rw\n\n[3805sub4]\nParameterName=MOD_ConfigEntryReg_xxh_AU32[n]\nObjectType=0x7\nDataType=0x0007\nAccessType=rw\n\n[3805sub5]\nParameterName=MOD_ConfigEntryReg_xxh_AU32[n]\nObjectType=0x7\nDataType=0x0007\nAccessType=rw\n\n[3806]\nParameterName=MOD_ConfigEntryReg_xxh_AU32\nObjectType=0x8\nSubNumber=6\n\n[3806sub0]\nParameterName=Number of Entries\nObjectType=0x7\nDataType=0x0005\nAccessType=ro\nDefaultValue=0x5\nLowLimit=0x0\nHighLimit=0xFF\n\n[3806sub1]\nParameterName=MOD_ConfigEntryReg_xxh_AU32[n]\nObjectType=0x7\nDataType=0x0007\nAccessType=rw\n\n[3806sub2]\nParameterName=MOD_ConfigEntryReg_xxh_AU32[n]\nObjectType=0x7\nDataType=0x0007\nAccessType=rw\n\n[3806sub3]\nParameterName=MOD_ConfigEntryReg_xxh_AU32[n]\nObjectType=0x7\nDataType=0x0007\nAccessType=rw\n\n[3806sub4]\nParameterName=MOD_ConfigEntryReg_xxh_AU32[n]\nObjectType=0x7\nDataType=0x0007\nAccessType=rw\n\n[3806sub5]\nParameterName=MOD_ConfigEntryReg_xxh_AU32[n]\nObjectType=0x7\nDataType=0x0007\nAccessType=rw\n\n[3807]\nParameterName=MOD_ConfigEntryReg_xxh_AU32\nObjectType=0x8\nSubNumber=6\n\n[3807sub0]\nParameterName=Number of Entries\nObjectType=0x7\nDataType=0x0005\nAccessType=ro\nDefaultValue=0x5\nLowLimit=0x0\nHighLimit=0xFF\n\n[3807sub1]\nParameterName=MOD_ConfigEntryReg_xxh_AU32[n]\nObjectType=0x7\nDataType=0x0007\nAccessType=rw\n\n[3807sub2]\nParameterName=MOD_ConfigEntryReg_xxh_AU32[n]\nObjectType=0x7\nDataType=0x0007\nAccessType=rw\n\n[3807sub3]\nParameterName=MOD_ConfigEntryReg_xxh_AU32[n]\nObjectType=0x7\nDataType=0x0007\nAccessType=rw\n\n[3807sub4]\nParameterName=MOD_ConfigEntryReg_xxh_AU32[n]\nObjectType=0x7\nDataType=0x0007\nAccessType=rw\n\n[3807sub5]\nParameterName=MOD_ConfigEntryReg_xxh_AU32[n]\nObjectType=0x7\nDataType=0x0007\nAccessType=rw\n\n[3808]\nParameterName=MOD_ConfigEntryReg_xxh_AU32\nObjectType=0x8\nSubNumber=6\n\n[3808sub0]\nParameterName=Number of Entries\nObjectType=0x7\nDataType=0x0005\nAccessType=ro\nDefaultValue=0x5\nLowLimit=0x0\nHighLimit=0xFF\n\n[3808sub1]\nParameterName=MOD_ConfigEntryReg_xxh_AU32[n]\nObjectType=0x7\nDataType=0x0007\nAccessType=rw\n\n[3808sub2]\nParameterName=MOD_ConfigEntryReg_xxh_AU32[n]\nObjectType=0x7\nDataType=0x0007\nAccessType=rw\n\n[3808sub3]\nParameterName=MOD_ConfigEntryReg_xxh_AU32[n]\nObjectType=0x7\nDataType=0x0007\nAccessType=rw\n\n[3808sub4]\nParameterName=MOD_ConfigEntryReg_xxh_AU32[n]\nObjectType=0x7\nDataType=0x0007\nAccessType=rw\n\n[3808sub5]\nParameterName=MOD_ConfigEntryReg_xxh_AU32[n]\nObjectType=0x7\nDataType=0x0007\nAccessType=rw\n\n[3809]\nParameterName=MOD_ConfigEntryReg_xxh_AU32\nObjectType=0x8\nSubNumber=6\n\n[3809sub0]\nParameterName=Number of Entries\nObjectType=0x7\nDataType=0x0005\nAccessType=ro\nDefaultValue=0x5\nLowLimit=0x0\nHighLimit=0xFF\n\n[3809sub1]\nParameterName=MOD_ConfigEntryReg_xxh_AU32[n]\nObjectType=0x7\nDataType=0x0007\nAccessType=rw\n\n[3809sub2]\nParameterName=MOD_ConfigEntryReg_xxh_AU32[n]\nObjectType=0x7\nDataType=0x0007\nAccessType=rw\n\n[3809sub3]\nParameterName=MOD_ConfigEntryReg_xxh_AU32[n]\nObjectType=0x7\nDataType=0x0007\nAccessType=rw\n\n[3809sub4]\nParameterName=MOD_ConfigEntryReg_xxh_AU32[n]\nObjectType=0x7\nDataType=0x0007\nAccessType=rw\n\n[3809sub5]\nParameterName=MOD_ConfigEntryReg_xxh_AU32[n]\nObjectType=0x7\nDataType=0x0007\nAccessType=rw\n\n[380A]\nParameterName=MOD_ConfigEntryReg_xxh_AU32\nObjectType=0x8\nSubNumber=6\n\n[380Asub0]\nParameterName=Number of Entries\nObjectType=0x7\nDataType=0x0005\nAccessType=ro\nDefaultValue=0x5\nLowLimit=0x0\nHighLimit=0xFF\n\n[380Asub1]\nParameterName=MOD_ConfigEntryReg_xxh_AU32[n]\nObjectType=0x7\nDataType=0x0007\nAccessType=rw\n\n[380Asub2]\nParameterName=MOD_ConfigEntryReg_xxh_AU32[n]\nObjectType=0x7\nDataType=0x0007\nAccessType=rw\n\n[380Asub3]\nParameterName=MOD_ConfigEntryReg_xxh_AU32[n]\nObjectType=0x7\nDataType=0x0007\nAccessType=rw\n\n[380Asub4]\nParameterName=MOD_ConfigEntryReg_xxh_AU32[n]\nObjectType=0x7\nDataType=0x0007\nAccessType=rw\n\n[380Asub5]\nParameterName=MOD_ConfigEntryReg_xxh_AU32[n]\nObjectType=0x7\nDataType=0x0007\nAccessType=rw\n\n[380B]\nParameterName=MOD_ConfigEntryReg_xxh_AU32\nObjectType=0x8\nSubNumber=6\n\n[380Bsub0]\nParameterName=Number of Entries\nObjectType=0x7\nDataType=0x0005\nAccessType=ro\nDefaultValue=0x5\nLowLimit=0x0\nHighLimit=0xFF\n\n[380Bsub1]\nParameterName=MOD_ConfigEntryReg_xxh_AU32[n]\nObjectType=0x7\nDataType=0x0007\nAccessType=rw\n\n[380Bsub2]\nParameterName=MOD_ConfigEntryReg_xxh_AU32[n]\nObjectType=0x7\nDataType=0x0007\nAccessType=rw\n\n[380Bsub3]\nParameterName=MOD_ConfigEntryReg_xxh_AU32[n]\nObjectType=0x7\nDataType=0x0007\nAccessType=rw\n\n[380Bsub4]\nParameterName=MOD_ConfigEntryReg_xxh_AU32[n]\nObjectType=0x7\nDataType=0x0007\nAccessType=rw\n\n[380Bsub5]\nParameterName=MOD_ConfigEntryReg_xxh_AU32[n]\nObjectType=0x7\nDataType=0x0007\nAccessType=rw\n\n[380C]\nParameterName=MOD_ConfigEntryReg_xxh_AU32\nObjectType=0x8\nSubNumber=6\n\n[380Csub0]\nParameterName=Number of Entries\nObjectType=0x7\nDataType=0x0005\nAccessType=ro\nDefaultValue=0x5\nLowLimit=0x0\nHighLimit=0xFF\n\n[380Csub1]\nParameterName=MOD_ConfigEntryReg_xxh_AU32[n]\nObjectType=0x7\nDataType=0x0007\nAccessType=rw\n\n[380Csub2]\nParameterName=MOD_ConfigEntryReg_xxh_AU32[n]\nObjectType=0x7\nDataType=0x0007\nAccessType=rw\n\n[380Csub3]\nParameterName=MOD_ConfigEntryReg_xxh_AU32[n]\nObjectType=0x7\nDataType=0x0007\nAccessType=rw\n\n[380Csub4]\nParameterName=MOD_ConfigEntryReg_xxh_AU32[n]\nObjectType=0x7\nDataType=0x0007\nAccessType=rw\n\n[380Csub5]\nParameterName=MOD_ConfigEntryReg_xxh_AU32[n]\nObjectType=0x7\nDataType=0x0007\nAccessType=rw\n\n[380D]\nParameterName=MOD_ConfigEntryReg_xxh_AU32\nObjectType=0x8\nSubNumber=6\n\n[380Dsub0]\nParameterName=Number of Entries\nObjectType=0x7\nDataType=0x0005\nAccessType=ro\nDefaultValue=0x5\nLowLimit=0x0\nHighLimit=0xFF\n\n[380Dsub1]\nParameterName=MOD_ConfigEntryReg_xxh_AU32[n]\nObjectType=0x7\nDataType=0x0007\nAccessType=rw\n\n[380Dsub2]\nParameterName=MOD_ConfigEntryReg_xxh_AU32[n]\nObjectType=0x7\nDataType=0x0007\nAccessType=rw\n\n[380Dsub3]\nParameterName=MOD_ConfigEntryReg_xxh_AU32[n]\nObjectType=0x7\nDataType=0x0007\nAccessType=rw\n\n[380Dsub4]\nParameterName=MOD_ConfigEntryReg_xxh_AU32[n]\nObjectType=0x7\nDataType=0x0007\nAccessType=rw\n\n[380Dsub5]\nParameterName=MOD_ConfigEntryReg_xxh_AU32[n]\nObjectType=0x7\nDataType=0x0007\nAccessType=rw\n\n[380E]\nParameterName=MOD_ConfigEntryReg_xxh_AU32\nObjectType=0x8\nSubNumber=6\n\n[380Esub0]\nParameterName=Number of Entries\nObjectType=0x7\nDataType=0x0005\nAccessType=ro\nDefaultValue=0x5\nLowLimit=0x0\nHighLimit=0xFF\n\n[380Esub1]\nParameterName=MOD_ConfigEntryReg_xxh_AU32[n]\nObjectType=0x7\nDataType=0x0007\nAccessType=rw\n\n[380Esub2]\nParameterName=MOD_ConfigEntryReg_xxh_AU32[n]\nObjectType=0x7\nDataType=0x0007\nAccessType=rw\n\n[380Esub3]\nParameterName=MOD_ConfigEntryReg_xxh_AU32[n]\nObjectType=0x7\nDataType=0x0007\nAccessType=rw\n\n[380Esub4]\nParameterName=MOD_ConfigEntryReg_xxh_AU32[n]\nObjectType=0x7\nDataType=0x0007\nAccessType=rw\n\n[380Esub5]\nParameterName=MOD_ConfigEntryReg_xxh_AU32[n]\nObjectType=0x7\nDataType=0x0007\nAccessType=rw\n\n[380F]\nParameterName=MOD_ConfigEntryReg_xxh_AU32\nObjectType=0x8\nSubNumber=6\n\n[380Fsub0]\nParameterName=Number of Entries\nObjectType=0x7\nDataType=0x0005\nAccessType=ro\nDefaultValue=0x5\nLowLimit=0x0\nHighLimit=0xFF\n\n[380Fsub1]\nParameterName=MOD_ConfigEntryReg_xxh_AU32[n]\nObjectType=0x7\nDataType=0x0007\nAccessType=rw\n\n[380Fsub2]\nParameterName=MOD_ConfigEntryReg_xxh_AU32[n]\nObjectType=0x7\nDataType=0x0007\nAccessType=rw\n\n[380Fsub3]\nParameterName=MOD_ConfigEntryReg_xxh_AU32[n]\nObjectType=0x7\nDataType=0x0007\nAccessType=rw\n\n[380Fsub4]\nParameterName=MOD_ConfigEntryReg_xxh_AU32[n]\nObjectType=0x7\nDataType=0x0007\nAccessType=rw\n\n[380Fsub5]\nParameterName=MOD_ConfigEntryReg_xxh_AU32[n]\nObjectType=0x7\nDataType=0x0007\nAccessType=rw\n\n[3810]\nParameterName=MOD_ConfigEntryReg_xxh_AU32\nObjectType=0x8\nSubNumber=6\n\n[3810sub0]\nParameterName=Number of Entries\nObjectType=0x7\nDataType=0x0005\nAccessType=ro\nDefaultValue=0x5\nLowLimit=0x0\nHighLimit=0xFF\n\n[3810sub1]\nParameterName=MOD_ConfigEntryReg_xxh_AU32[n]\nObjectType=0x7\nDataType=0x0007\nAccessType=rw\n\n[3810sub2]\nParameterName=MOD_ConfigEntryReg_xxh_AU32[n]\nObjectType=0x7\nDataType=0x0007\nAccessType=rw\n\n[3810sub3]\nParameterName=MOD_ConfigEntryReg_xxh_AU32[n]\nObjectType=0x7\nDataType=0x0007\nAccessType=rw\n\n[3810sub4]\nParameterName=MOD_ConfigEntryReg_xxh_AU32[n]\nObjectType=0x7\nDataType=0x0007\nAccessType=rw\n\n[3810sub5]\nParameterName=MOD_ConfigEntryReg_xxh_AU32[n]\nObjectType=0x7\nDataType=0x0007\nAccessType=rw\n\n[3811]\nParameterName=MOD_ConfigEntryReg_xxh_AU32\nObjectType=0x8\nSubNumber=6\n\n[3811sub0]\nParameterName=Number of Entries\nObjectType=0x7\nDataType=0x0005\nAccessType=ro\nDefaultValue=0x5\nLowLimit=0x0\nHighLimit=0xFF\n\n[3811sub1]\nParameterName=MOD_ConfigEntryReg_xxh_AU32[n]\nObjectType=0x7\nDataType=0x0007\nAccessType=rw\n\n[3811sub2]\nParameterName=MOD_ConfigEntryReg_xxh_AU32[n]\nObjectType=0x7\nDataType=0x0007\nAccessType=rw\n\n[3811sub3]\nParameterName=MOD_ConfigEntryReg_xxh_AU32[n]\nObjectType=0x7\nDataType=0x0007\nAccessType=rw\n\n[3811sub4]\nParameterName=MOD_ConfigEntryReg_xxh_AU32[n]\nObjectType=0x7\nDataType=0x0007\nAccessType=rw\n\n[3811sub5]\nParameterName=MOD_ConfigEntryReg_xxh_AU32[n]\nObjectType=0x7\nDataType=0x0007\nAccessType=rw\n\n[3812]\nParameterName=MOD_ConfigEntryReg_xxh_AU32\nObjectType=0x8\nSubNumber=6\n\n[3812sub0]\nParameterName=Number of Entries\nObjectType=0x7\nDataType=0x0005\nAccessType=ro\nDefaultValue=0x5\nLowLimit=0x0\nHighLimit=0xFF\n\n[3812sub1]\nParameterName=MOD_ConfigEntryReg_xxh_AU32[n]\nObjectType=0x7\nDataType=0x0007\nAccessType=rw\n\n[3812sub2]\nParameterName=MOD_ConfigEntryReg_xxh_AU32[n]\nObjectType=0x7\nDataType=0x0007\nAccessType=rw\n\n[3812sub3]\nParameterName=MOD_ConfigEntryReg_xxh_AU32[n]\nObjectType=0x7\nDataType=0x0007\nAccessType=rw\n\n[3812sub4]\nParameterName=MOD_ConfigEntryReg_xxh_AU32[n]\nObjectType=0x7\nDataType=0x0007\nAccessType=rw\n\n[3812sub5]\nParameterName=MOD_ConfigEntryReg_xxh_AU32[n]\nObjectType=0x7\nDataType=0x0007\nAccessType=rw\n\n[3813]\nParameterName=MOD_ConfigEntryReg_xxh_AU32\nObjectType=0x8\nSubNumber=6\n\n[3813sub0]\nParameterName=Number of Entries\nObjectType=0x7\nDataType=0x0005\nAccessType=ro\nDefaultValue=0x5\nLowLimit=0x0\nHighLimit=0xFF\n\n[3813sub1]\nParameterName=MOD_ConfigEntryReg_xxh_AU32[n]\nObjectType=0x7\nDataType=0x0007\nAccessType=rw\n\n[3813sub2]\nParameterName=MOD_ConfigEntryReg_xxh_AU32[n]\nObjectType=0x7\nDataType=0x0007\nAccessType=rw\n\n[3813sub3]\nParameterName=MOD_ConfigEntryReg_xxh_AU32[n]\nObjectType=0x7\nDataType=0x0007\nAccessType=rw\n\n[3813sub4]\nParameterName=MOD_ConfigEntryReg_xxh_AU32[n]\nObjectType=0x7\nDataType=0x0007\nAccessType=rw\n\n[3813sub5]\nParameterName=MOD_ConfigEntryReg_xxh_AU32[n]\nObjectType=0x7\nDataType=0x0007\nAccessType=rw\n\n[3900]\nParameterName=MOD_ConfigEntryVal_xxh_AU32\nObjectType=0x8\nSubNumber=6\n\n[3900sub0]\nParameterName=Number of Entries\nObjectType=0x7\nDataType=0x0005\nAccessType=ro\nDefaultValue=0x5\nLowLimit=0x0\nHighLimit=0xFF\n\n[3900sub1]\nParameterName=MOD_ConfigEntryVal_xxh_AU32[n]\nObjectType=0x7\nDataType=0x0007\nAccessType=rw\n\n[3900sub2]\nParameterName=MOD_ConfigEntryVal_xxh_AU32[n]\nObjectType=0x7\nDataType=0x0007\nAccessType=rw\n\n[3900sub3]\nParameterName=MOD_ConfigEntryVal_xxh_AU32[n]\nObjectType=0x7\nDataType=0x0007\nAccessType=rw\n\n[3900sub4]\nParameterName=MOD_ConfigEntryVal_xxh_AU32[n]\nObjectType=0x7\nDataType=0x0007\nAccessType=rw\n\n[3900sub5]\nParameterName=MOD_ConfigEntryVal_xxh_AU32[n]\nObjectType=0x7\nDataType=0x0007\nAccessType=rw\n\n[3901]\nParameterName=MOD_ConfigEntryVal_xxh_AU32\nObjectType=0x8\nSubNumber=6\n\n[3901sub0]\nParameterName=Number of Entries\nObjectType=0x7\nDataType=0x0005\nAccessType=ro\nDefaultValue=0x5\nLowLimit=0x0\nHighLimit=0xFF\n\n[3901sub1]\nParameterName=MOD_ConfigEntryVal_xxh_AU32[n]\nObjectType=0x7\nDataType=0x0007\nAccessType=rw\n\n[3901sub2]\nParameterName=MOD_ConfigEntryVal_xxh_AU32[n]\nObjectType=0x7\nDataType=0x0007\nAccessType=rw\n\n[3901sub3]\nParameterName=MOD_ConfigEntryVal_xxh_AU32[n]\nObjectType=0x7\nDataType=0x0007\nAccessType=rw\n\n[3901sub4]\nParameterName=MOD_ConfigEntryVal_xxh_AU32[n]\nObjectType=0x7\nDataType=0x0007\nAccessType=rw\n\n[3901sub5]\nParameterName=MOD_ConfigEntryVal_xxh_AU32[n]\nObjectType=0x7\nDataType=0x0007\nAccessType=rw\n\n[3902]\nParameterName=MOD_ConfigEntryVal_xxh_AU32\nObjectType=0x8\nSubNumber=6\n\n[3902sub0]\nParameterName=Number of Entries\nObjectType=0x7\nDataType=0x0005\nAccessType=ro\nDefaultValue=0x5\nLowLimit=0x0\nHighLimit=0xFF\n\n[3902sub1]\nParameterName=MOD_ConfigEntryVal_xxh_AU32[n]\nObjectType=0x7\nDataType=0x0007\nAccessType=rw\n\n[3902sub2]\nParameterName=MOD_ConfigEntryVal_xxh_AU32[n]\nObjectType=0x7\nDataType=0x0007\nAccessType=rw\n\n[3902sub3]\nParameterName=MOD_ConfigEntryVal_xxh_AU32[n]\nObjectType=0x7\nDataType=0x0007\nAccessType=rw\n\n[3902sub4]\nParameterName=MOD_ConfigEntryVal_xxh_AU32[n]\nObjectType=0x7\nDataType=0x0007\nAccessType=rw\n\n[3902sub5]\nParameterName=MOD_ConfigEntryVal_xxh_AU32[n]\nObjectType=0x7\nDataType=0x0007\nAccessType=rw\n\n[3903]\nParameterName=MOD_ConfigEntryVal_xxh_AU32\nObjectType=0x8\nSubNumber=6\n\n[3903sub0]\nParameterName=Number of Entries\nObjectType=0x7\nDataType=0x0005\nAccessType=ro\nDefaultValue=0x5\nLowLimit=0x0\nHighLimit=0xFF\n\n[3903sub1]\nParameterName=MOD_ConfigEntryVal_xxh_AU32[n]\nObjectType=0x7\nDataType=0x0007\nAccessType=rw\n\n[3903sub2]\nParameterName=MOD_ConfigEntryVal_xxh_AU32[n]\nObjectType=0x7\nDataType=0x0007\nAccessType=rw\n\n[3903sub3]\nParameterName=MOD_ConfigEntryVal_xxh_AU32[n]\nObjectType=0x7\nDataType=0x0007\nAccessType=rw\n\n[3903sub4]\nParameterName=MOD_ConfigEntryVal_xxh_AU32[n]\nObjectType=0x7\nDataType=0x0007\nAccessType=rw\n\n[3903sub5]\nParameterName=MOD_ConfigEntryVal_xxh_AU32[n]\nObjectType=0x7\nDataType=0x0007\nAccessType=rw\n\n[3904]\nParameterName=MOD_ConfigEntryVal_xxh_AU32\nObjectType=0x8\nSubNumber=6\n\n[3904sub0]\nParameterName=Number of Entries\nObjectType=0x7\nDataType=0x0005\nAccessType=ro\nDefaultValue=0x5\nLowLimit=0x0\nHighLimit=0xFF\n\n[3904sub1]\nParameterName=MOD_ConfigEntryVal_xxh_AU32[n]\nObjectType=0x7\nDataType=0x0007\nAccessType=rw\n\n[3904sub2]\nParameterName=MOD_ConfigEntryVal_xxh_AU32[n]\nObjectType=0x7\nDataType=0x0007\nAccessType=rw\n\n[3904sub3]\nParameterName=MOD_ConfigEntryVal_xxh_AU32[n]\nObjectType=0x7\nDataType=0x0007\nAccessType=rw\n\n[3904sub4]\nParameterName=MOD_ConfigEntryVal_xxh_AU32[n]\nObjectType=0x7\nDataType=0x0007\nAccessType=rw\n\n[3904sub5]\nParameterName=MOD_ConfigEntryVal_xxh_AU32[n]\nObjectType=0x7\nDataType=0x0007\nAccessType=rw\n\n[3905]\nParameterName=MOD_ConfigEntryVal_xxh_AU32\nObjectType=0x8\nSubNumber=6\n\n[3905sub0]\nParameterName=Number of Entries\nObjectType=0x7\nDataType=0x0005\nAccessType=ro\nDefaultValue=0x5\nLowLimit=0x0\nHighLimit=0xFF\n\n[3905sub1]\nParameterName=MOD_ConfigEntryVal_xxh_AU32[n]\nObjectType=0x7\nDataType=0x0007\nAccessType=rw\n\n[3905sub2]\nParameterName=MOD_ConfigEntryVal_xxh_AU32[n]\nObjectType=0x7\nDataType=0x0007\nAccessType=rw\n\n[3905sub3]\nParameterName=MOD_ConfigEntryVal_xxh_AU32[n]\nObjectType=0x7\nDataType=0x0007\nAccessType=rw\n\n[3905sub4]\nParameterName=MOD_ConfigEntryVal_xxh_AU32[n]\nObjectType=0x7\nDataType=0x0007\nAccessType=rw\n\n[3905sub5]\nParameterName=MOD_ConfigEntryVal_xxh_AU32[n]\nObjectType=0x7\nDataType=0x0007\nAccessType=rw\n\n[3906]\nParameterName=MOD_ConfigEntryVal_xxh_AU32\nObjectType=0x8\nSubNumber=6\n\n[3906sub0]\nParameterName=Number of Entries\nObjectType=0x7\nDataType=0x0005\nAccessType=ro\nDefaultValue=0x5\nLowLimit=0x0\nHighLimit=0xFF\n\n[3906sub1]\nParameterName=MOD_ConfigEntryVal_xxh_AU32[n]\nObjectType=0x7\nDataType=0x0007\nAccessType=rw\n\n[3906sub2]\nParameterName=MOD_ConfigEntryVal_xxh_AU32[n]\nObjectType=0x7\nDataType=0x0007\nAccessType=rw\n\n[3906sub3]\nParameterName=MOD_ConfigEntryVal_xxh_AU32[n]\nObjectType=0x7\nDataType=0x0007\nAccessType=rw\n\n[3906sub4]\nParameterName=MOD_ConfigEntryVal_xxh_AU32[n]\nObjectType=0x7\nDataType=0x0007\nAccessType=rw\n\n[3906sub5]\nParameterName=MOD_ConfigEntryVal_xxh_AU32[n]\nObjectType=0x7\nDataType=0x0007\nAccessType=rw\n\n[3907]\nParameterName=MOD_ConfigEntryVal_xxh_AU32\nObjectType=0x8\nSubNumber=6\n\n[3907sub0]\nParameterName=Number of Entries\nObjectType=0x7\nDataType=0x0005\nAccessType=ro\nDefaultValue=0x5\nLowLimit=0x0\nHighLimit=0xFF\n\n[3907sub1]\nParameterName=MOD_ConfigEntryVal_xxh_AU32[n]\nObjectType=0x7\nDataType=0x0007\nAccessType=rw\n\n[3907sub2]\nParameterName=MOD_ConfigEntryVal_xxh_AU32[n]\nObjectType=0x7\nDataType=0x0007\nAccessType=rw\n\n[3907sub3]\nParameterName=MOD_ConfigEntryVal_xxh_AU32[n]\nObjectType=0x7\nDataType=0x0007\nAccessType=rw\n\n[3907sub4]\nParameterName=MOD_ConfigEntryVal_xxh_AU32[n]\nObjectType=0x7\nDataType=0x0007\nAccessType=rw\n\n[3907sub5]\nParameterName=MOD_ConfigEntryVal_xxh_AU32[n]\nObjectType=0x7\nDataType=0x0007\nAccessType=rw\n\n[3908]\nParameterName=MOD_ConfigEntryVal_xxh_AU32\nObjectType=0x8\nSubNumber=6\n\n[3908sub0]\nParameterName=Number of Entries\nObjectType=0x7\nDataType=0x0005\nAccessType=ro\nDefaultValue=0x5\nLowLimit=0x0\nHighLimit=0xFF\n\n[3908sub1]\nParameterName=MOD_ConfigEntryVal_xxh_AU32[n]\nObjectType=0x7\nDataType=0x0007\nAccessType=rw\n\n[3908sub2]\nParameterName=MOD_ConfigEntryVal_xxh_AU32[n]\nObjectType=0x7\nDataType=0x0007\nAccessType=rw\n\n[3908sub3]\nParameterName=MOD_ConfigEntryVal_xxh_AU32[n]\nObjectType=0x7\nDataType=0x0007\nAccessType=rw\n\n[3908sub4]\nParameterName=MOD_ConfigEntryVal_xxh_AU32[n]\nObjectType=0x7\nDataType=0x0007\nAccessType=rw\n\n[3908sub5]\nParameterName=MOD_ConfigEntryVal_xxh_AU32[n]\nObjectType=0x7\nDataType=0x0007\nAccessType=rw\n\n[3909]\nParameterName=MOD_ConfigEntryVal_xxh_AU32\nObjectType=0x8\nSubNumber=6\n\n[3909sub0]\nParameterName=Number of Entries\nObjectType=0x7\nDataType=0x0005\nAccessType=ro\nDefaultValue=0x5\nLowLimit=0x0\nHighLimit=0xFF\n\n[3909sub1]\nParameterName=MOD_ConfigEntryVal_xxh_AU32[n]\nObjectType=0x7\nDataType=0x0007\nAccessType=rw\n\n[3909sub2]\nParameterName=MOD_ConfigEntryVal_xxh_AU32[n]\nObjectType=0x7\nDataType=0x0007\nAccessType=rw\n\n[3909sub3]\nParameterName=MOD_ConfigEntryVal_xxh_AU32[n]\nObjectType=0x7\nDataType=0x0007\nAccessType=rw\n\n[3909sub4]\nParameterName=MOD_ConfigEntryVal_xxh_AU32[n]\nObjectType=0x7\nDataType=0x0007\nAccessType=rw\n\n[3909sub5]\nParameterName=MOD_ConfigEntryVal_xxh_AU32[n]\nObjectType=0x7\nDataType=0x0007\nAccessType=rw\n\n[390A]\nParameterName=MOD_ConfigEntryVal_xxh_AU32\nObjectType=0x8\nSubNumber=6\n\n[390Asub0]\nParameterName=Number of Entries\nObjectType=0x7\nDataType=0x0005\nAccessType=ro\nDefaultValue=0x5\nLowLimit=0x0\nHighLimit=0xFF\n\n[390Asub1]\nParameterName=MOD_ConfigEntryVal_xxh_AU32[n]\nObjectType=0x7\nDataType=0x0007\nAccessType=rw\n\n[390Asub2]\nParameterName=MOD_ConfigEntryVal_xxh_AU32[n]\nObjectType=0x7\nDataType=0x0007\nAccessType=rw\n\n[390Asub3]\nParameterName=MOD_ConfigEntryVal_xxh_AU32[n]\nObjectType=0x7\nDataType=0x0007\nAccessType=rw\n\n[390Asub4]\nParameterName=MOD_ConfigEntryVal_xxh_AU32[n]\nObjectType=0x7\nDataType=0x0007\nAccessType=rw\n\n[390Asub5]\nParameterName=MOD_ConfigEntryVal_xxh_AU32[n]\nObjectType=0x7\nDataType=0x0007\nAccessType=rw\n\n[390B]\nParameterName=MOD_ConfigEntryVal_xxh_AU32\nObjectType=0x8\nSubNumber=6\n\n[390Bsub0]\nParameterName=Number of Entries\nObjectType=0x7\nDataType=0x0005\nAccessType=ro\nDefaultValue=0x5\nLowLimit=0x0\nHighLimit=0xFF\n\n[390Bsub1]\nParameterName=MOD_ConfigEntryVal_xxh_AU32[n]\nObjectType=0x7\nDataType=0x0007\nAccessType=rw\n\n[390Bsub2]\nParameterName=MOD_ConfigEntryVal_xxh_AU32[n]\nObjectType=0x7\nDataType=0x0007\nAccessType=rw\n\n[390Bsub3]\nParameterName=MOD_ConfigEntryVal_xxh_AU32[n]\nObjectType=0x7\nDataType=0x0007\nAccessType=rw\n\n[390Bsub4]\nParameterName=MOD_ConfigEntryVal_xxh_AU32[n]\nObjectType=0x7\nDataType=0x0007\nAccessType=rw\n\n[390Bsub5]\nParameterName=MOD_ConfigEntryVal_xxh_AU32[n]\nObjectType=0x7\nDataType=0x0007\nAccessType=rw\n\n[390C]\nParameterName=MOD_ConfigEntryVal_xxh_AU32\nObjectType=0x8\nSubNumber=6\n\n[390Csub0]\nParameterName=Number of Entries\nObjectType=0x7\nDataType=0x0005\nAccessType=ro\nDefaultValue=0x5\nLowLimit=0x0\nHighLimit=0xFF\n\n[390Csub1]\nParameterName=MOD_ConfigEntryVal_xxh_AU32[n]\nObjectType=0x7\nDataType=0x0007\nAccessType=rw\n\n[390Csub2]\nParameterName=MOD_ConfigEntryVal_xxh_AU32[n]\nObjectType=0x7\nDataType=0x0007\nAccessType=rw\n\n[390Csub3]\nParameterName=MOD_ConfigEntryVal_xxh_AU32[n]\nObjectType=0x7\nDataType=0x0007\nAccessType=rw\n\n[390Csub4]\nParameterName=MOD_ConfigEntryVal_xxh_AU32[n]\nObjectType=0x7\nDataType=0x0007\nAccessType=rw\n\n[390Csub5]\nParameterName=MOD_ConfigEntryVal_xxh_AU32[n]\nObjectType=0x7\nDataType=0x0007\nAccessType=rw\n\n[390D]\nParameterName=MOD_ConfigEntryVal_xxh_AU32\nObjectType=0x8\nSubNumber=6\n\n[390Dsub0]\nParameterName=Number of Entries\nObjectType=0x7\nDataType=0x0005\nAccessType=ro\nDefaultValue=0x5\nLowLimit=0x0\nHighLimit=0xFF\n\n[390Dsub1]\nParameterName=MOD_ConfigEntryVal_xxh_AU32[n]\nObjectType=0x7\nDataType=0x0007\nAccessType=rw\n\n[390Dsub2]\nParameterName=MOD_ConfigEntryVal_xxh_AU32[n]\nObjectType=0x7\nDataType=0x0007\nAccessType=rw\n\n[390Dsub3]\nParameterName=MOD_ConfigEntryVal_xxh_AU32[n]\nObjectType=0x7\nDataType=0x0007\nAccessType=rw\n\n[390Dsub4]\nParameterName=MOD_ConfigEntryVal_xxh_AU32[n]\nObjectType=0x7\nDataType=0x0007\nAccessType=rw\n\n[390Dsub5]\nParameterName=MOD_ConfigEntryVal_xxh_AU32[n]\nObjectType=0x7\nDataType=0x0007\nAccessType=rw\n\n[390E]\nParameterName=MOD_ConfigEntryVal_xxh_AU32\nObjectType=0x8\nSubNumber=6\n\n[390Esub0]\nParameterName=Number of Entries\nObjectType=0x7\nDataType=0x0005\nAccessType=ro\nDefaultValue=0x5\nLowLimit=0x0\nHighLimit=0xFF\n\n[390Esub1]\nParameterName=MOD_ConfigEntryVal_xxh_AU32[n]\nObjectType=0x7\nDataType=0x0007\nAccessType=rw\n\n[390Esub2]\nParameterName=MOD_ConfigEntryVal_xxh_AU32[n]\nObjectType=0x7\nDataType=0x0007\nAccessType=rw\n\n[390Esub3]\nParameterName=MOD_ConfigEntryVal_xxh_AU32[n]\nObjectType=0x7\nDataType=0x0007\nAccessType=rw\n\n[390Esub4]\nParameterName=MOD_ConfigEntryVal_xxh_AU32[n]\nObjectType=0x7\nDataType=0x0007\nAccessType=rw\n\n[390Esub5]\nParameterName=MOD_ConfigEntryVal_xxh_AU32[n]\nObjectType=0x7\nDataType=0x0007\nAccessType=rw\n\n[390F]\nParameterName=MOD_ConfigEntryVal_xxh_AU32\nObjectType=0x8\nSubNumber=6\n\n[390Fsub0]\nParameterName=Number of Entries\nObjectType=0x7\nDataType=0x0005\nAccessType=ro\nDefaultValue=0x5\nLowLimit=0x0\nHighLimit=0xFF\n\n[390Fsub1]\nParameterName=MOD_ConfigEntryVal_xxh_AU32[n]\nObjectType=0x7\nDataType=0x0007\nAccessType=rw\n\n[390Fsub2]\nParameterName=MOD_ConfigEntryVal_xxh_AU32[n]\nObjectType=0x7\nDataType=0x0007\nAccessType=rw\n\n[390Fsub3]\nParameterName=MOD_ConfigEntryVal_xxh_AU32[n]\nObjectType=0x7\nDataType=0x0007\nAccessType=rw\n\n[390Fsub4]\nParameterName=MOD_ConfigEntryVal_xxh_AU32[n]\nObjectType=0x7\nDataType=0x0007\nAccessType=rw\n\n[390Fsub5]\nParameterName=MOD_ConfigEntryVal_xxh_AU32[n]\nObjectType=0x7\nDataType=0x0007\nAccessType=rw\n\n[3910]\nParameterName=MOD_ConfigEntryVal_xxh_AU32\nObjectType=0x8\nSubNumber=6\n\n[3910sub0]\nParameterName=Number of Entries\nObjectType=0x7\nDataType=0x0005\nAccessType=ro\nDefaultValue=0x5\nLowLimit=0x0\nHighLimit=0xFF\n\n[3910sub1]\nParameterName=MOD_ConfigEntryVal_xxh_AU32[n]\nObjectType=0x7\nDataType=0x0007\nAccessType=rw\n\n[3910sub2]\nParameterName=MOD_ConfigEntryVal_xxh_AU32[n]\nObjectType=0x7\nDataType=0x0007\nAccessType=rw\n\n[3910sub3]\nParameterName=MOD_ConfigEntryVal_xxh_AU32[n]\nObjectType=0x7\nDataType=0x0007\nAccessType=rw\n\n[3910sub4]\nParameterName=MOD_ConfigEntryVal_xxh_AU32[n]\nObjectType=0x7\nDataType=0x0007\nAccessType=rw\n\n[3910sub5]\nParameterName=MOD_ConfigEntryVal_xxh_AU32[n]\nObjectType=0x7\nDataType=0x0007\nAccessType=rw\n\n[3911]\nParameterName=MOD_ConfigEntryVal_xxh_AU32\nObjectType=0x8\nSubNumber=6\n\n[3911sub0]\nParameterName=Number of Entries\nObjectType=0x7\nDataType=0x0005\nAccessType=ro\nDefaultValue=0x5\nLowLimit=0x0\nHighLimit=0xFF\n\n[3911sub1]\nParameterName=MOD_ConfigEntryVal_xxh_AU32[n]\nObjectType=0x7\nDataType=0x0007\nAccessType=rw\n\n[3911sub2]\nParameterName=MOD_ConfigEntryVal_xxh_AU32[n]\nObjectType=0x7\nDataType=0x0007\nAccessType=rw\n\n[3911sub3]\nParameterName=MOD_ConfigEntryVal_xxh_AU32[n]\nObjectType=0x7\nDataType=0x0007\nAccessType=rw\n\n[3911sub4]\nParameterName=MOD_ConfigEntryVal_xxh_AU32[n]\nObjectType=0x7\nDataType=0x0007\nAccessType=rw\n\n[3911sub5]\nParameterName=MOD_ConfigEntryVal_xxh_AU32[n]\nObjectType=0x7\nDataType=0x0007\nAccessType=rw\n\n[3912]\nParameterName=MOD_ConfigEntryVal_xxh_AU32\nObjectType=0x8\nSubNumber=6\n\n[3912sub0]\nParameterName=Number of Entries\nObjectType=0x7\nDataType=0x0005\nAccessType=ro\nDefaultValue=0x5\nLowLimit=0x0\nHighLimit=0xFF\n\n[3912sub1]\nParameterName=MOD_ConfigEntryVal_xxh_AU32[n]\nObjectType=0x7\nDataType=0x0007\nAccessType=rw\n\n[3912sub2]\nParameterName=MOD_ConfigEntryVal_xxh_AU32[n]\nObjectType=0x7\nDataType=0x0007\nAccessType=rw\n\n[3912sub3]\nParameterName=MOD_ConfigEntryVal_xxh_AU32[n]\nObjectType=0x7\nDataType=0x0007\nAccessType=rw\n\n[3912sub4]\nParameterName=MOD_ConfigEntryVal_xxh_AU32[n]\nObjectType=0x7\nDataType=0x0007\nAccessType=rw\n\n[3912sub5]\nParameterName=MOD_ConfigEntryVal_xxh_AU32[n]\nObjectType=0x7\nDataType=0x0007\nAccessType=rw\n\n[3913]\nParameterName=MOD_ConfigEntryVal_xxh_AU32\nObjectType=0x8\nSubNumber=6\n\n[3913sub0]\nParameterName=Number of Entries\nObjectType=0x7\nDataType=0x0005\nAccessType=ro\nDefaultValue=0x5\nLowLimit=0x0\nHighLimit=0xFF\n\n[3913sub1]\nParameterName=MOD_ConfigEntryVal_xxh_AU32[n]\nObjectType=0x7\nDataType=0x0007\nAccessType=rw\n\n[3913sub2]\nParameterName=MOD_ConfigEntryVal_xxh_AU32[n]\nObjectType=0x7\nDataType=0x0007\nAccessType=rw\n\n[3913sub3]\nParameterName=MOD_ConfigEntryVal_xxh_AU32[n]\nObjectType=0x7\nDataType=0x0007\nAccessType=rw\n\n[3913sub4]\nParameterName=MOD_ConfigEntryVal_xxh_AU32[n]\nObjectType=0x7\nDataType=0x0007\nAccessType=rw\n\n[3913sub5]\nParameterName=MOD_ConfigEntryVal_xxh_AU32[n]\nObjectType=0x7\nDataType=0x0007\nAccessType=rw\n\n[3FFD]\nParameterName=Save_and_Reboot_Manufacturer\nObjectType=0x7\nDataType=0x0007\nAccessType=rw\nPDOMapping=0\n\n[3FFE]\nParameterName=Save_and_Reboot_Manufacturer_Communication\nObjectType=0x7\nDataType=0x0007\nAccessType=rw\nPDOMapping=0\n\n[3FFF]\nParameterName=Save_and_Reboot_All\nObjectType=0x7\nDataType=0x0007\nAccessType=rw\nPDOMapping=0\n") -> (error out=w12:errorcluster)  [unwired: 2 in, 2 out]
  n4 = call "Import.vi"("error in"=w12, "EDS File Path"=w4) -> ("error out"=w11:errorcluster, "Electronic Datasheet"=w10:refnum<class "Electronic Datasheet.lvclass">)  [unwired: 8 in]
  n5 = property class="EDS"(reference=w10, error in=w11) -> (error out=w5:errorcluster, "fields:Obj Dict"=w7:refnum<class "Object Dictionary.lvclass">)  [unwired: 1 out]
  n6 = call-dynamic "Create Generic IO Profile.vi"("error in"=w5, "Cia401Profile in"=w18) -> ("error out"=w17:errorcluster, "Cia401Profile out"=w16:refnum<class "CiA401 Generic IO Profile.lvclass">)  [unwired: 8 in]
  n7 = property class="Generic IO Profile"(reference=w16, error in=w17, "IO Capabilities"=T2 {"hasDigitialInputs"=TRUE, "hasDigitalOutputs"=FALSE, "hasAnalogInputs"=FALSE, "hasAnalogOutputs"=FALSE} ("Capabilities")) -> (reference out=w8:refnum<class "CiA401 Generic IO Profile.lvclass">, error out=w9:errorcluster)
  n8 = call-dynamic "Validate.vi"("error in"=w9, "Obj Dictionary"=w7, "CiA401 Generic IO Profile in"=w8) -> ("error out"=w6:errorcluster, "Missing Objects"=w2:T1[])  [unwired: 6 in, 1 out]
  n9 = call "Pass If Equal.vim"("error in (no error)"=w6, "Actual"=w2, "Expected"=T1[] [] ("Missing Objects"), "LUnit Test Case In"="Test Case In") -> ("error out"=→"error out":errorcluster, "LUnit Test Case Out"=→"Test Case Out":refnum<class "Test Profile Verification.lvclass">)  [unwired: 6 in]
